vi "WVDIAL+HSRL_v5.8.vi"() -> ()   [LabVIEW 2012]
uses:
  C:/Users/eol-lidar/Desktop/20171016_WVDIALLabviewSlimmed/DLLs/PowerMeterCommands.dll
  DLLs/PowerMeterCommands.dll
  <vilib>/DAQmx/write.llb/DAQmx Write (Digital 1D Bool NChan 1Samp 1Line).vi
  <vilib>/DAQmx/miscellaneous.llb/DAQmx Fill In Error Info.vi
  <vilib>/Analysis/baseanly.llb/Mean (DBL).vi
  WVD-MCSupdate/WVDMCSupdate/Subroutines/AMCS_Data.vi
  Shared Telescope WV DIAL Code/Libraries and VIs/Scalar_Data.vi
  <vilib>/Analysis/NI_AALBase.lvlib
  Shared Telescope WV DIAL Code/Libraries and VIs/Scalar_Data_2.vi
  Shared Telescope WV DIAL Code/Libraries and VIs/Scalar_Data_4.vi
  Shared Telescope WV DIAL Code/Libraries and VIs/Scalar_Data_3.vi
  DLLs/CLDevIFace.dll
panel:
  out "WV_averaged_energy":dbl
  out "HSRL Pulse Energy":dbl=375.0
  out "sigma_off_total":dbl[](array[numeric])=[5.0680831413375535e-25, 5.050268932514758e-25, 5.0324923656148135e-25, 5.014753469706972e-25, 4.99705227357782e-25, 4.979388805746344e-25, 4.961763094386931e-25, 4.944175167376033e-25, 4.926625052240752e-25, 4.909112776197929e-25, 4.891638366076327e-25, 4.874201848358338e-25, 4.856803249148664e-25, 4.839442594150606e-25, 4.822119908686877e-25, 4.8048352176943855e-25, 4.78758854565523e-25, 4.770379916627166e-25, 4.753209354281222e-25, 4.736076881793376e-25, 4.718982521901608e-25, 4.7019262968902895e-25, 4.684908228544634e-25, 4.667928338234015e-25, 4.650986646753398e-25, 4.634083174466291e-25, 4.617217941209719e-25, 4.6003909663091255e-25, 4.583602268570049e-25, 4.566851866270442e-25, 4.55013977714655e-25, 4.533466018427296e-25, 4.516830606754478e-25, 4.500233558239396e-25, 4.483674888410031e-25, 4.467154612270298e-25, 4.450672744202499e-25, 4.434229298043165e-25, 4.417824287033527e-25, 4.401457723829736e-25, 4.385129620513669e-25, 4.368839988513398e-25, 4.352588838702857e-25, 4.336376181349563e-25, 4.320202026083546e-25, 4.304066381932244e-25, 4.287969257308179e-25, 4.271910659984005e-25, 4.255890597128637e-25, 4.239909075259594e-25, 4.22396610028079e-25, 4.208061677439288e-25, 4.192195811375286e-25, 4.176368506057362e-25, 4.160579764835863e-25, 4.144829590406775e-25, 4.129117984793732e-25, 4.113444949423985e-25, 4.097810485038377e-25, 4.082214591740086e-25, 4.0666572689665333e-25, 4.0511385155395965e-25, 4.0356583295814885e-25, 4.0202167085949603e-25, 4.004813649400491e-25, 3.989449148200182e-25, 3.974123200508076e-25, 3.958835801202973e-25, 3.943586944503348e-25, 3.928376623976787e-25, 3.9132048325413214e-25, 3.898071562459315e-25, 3.8829768053453936e-25, 3.8679205521584474e-25, 3.8529027932308287e-25, 3.837923518222313e-25, 3.822982716166859e-25, 3.8080803754419415e-25, 3.7932164837935613e-25, 3.7783910283248477e-25, 3.7636039955186373e-25, 3.748855371190181e-25, 3.7341451405484317e-25, 3.719473288177287e-25, 3.7048397980204027e-25, 3.6902446533968063e-25, 3.675687837026237e-25, 3.6611693309848415e-25, 3.6466891167654896e-25, 3.6322471752135777e-25, 3.617843486608717e-25, 3.6034780305936944e-25, 3.5891507862467635e-25, 3.5748617320063354e-25, 3.560610845767059e-25, 3.5463981047924663e-25, 3.532223485800512e-25, 3.5180869649136043e-25, 3.5039885176765912e-25, 3.48992811906682e-25, 3.475905743508301e-25, 3.4619213648441316e-25, 3.4479749563841165e-25, 3.434066490863645e-25, 3.4201959404908824e-25, 3.4063632769091302e-25, 3.3925684712700433e-25, 3.378811494142299e-25, 3.365092315592867e-25, 3.3514109051791915e-25, 3.3377672319122537e-25, 3.324161264322276e-25, 3.3105929704212585e-25, 3.2970623177234063e-25, 3.283569273235881e-25, 3.270113803501489e-25, 3.256695874559878e-25, 3.243315451986542e-25, 3.2299725008719377e-25, 3.2166669858496116e-25, 3.20339887109077e-25, 3.190168120304605e-25, 3.176974696765837e-25, 3.1638185632881056e-25, 3.150699682259159e-25, 3.1376180156208974e-25, 3.124573524912379e-25, 3.1115661712294625e-25, 3.098595915273405e-25, 3.0856627173057447e-25, 3.0727665372159963e-25, 3.0599073344858437e-25, 3.0470850681967553e-25, 3.0342996970621855e-25, 3.0215511793910874e-25, 3.0088394731451073e-25, 2.9961645359090424e-25, 2.9835263248846283e-25, 2.9709247969417565e-25, 2.958359908598783e-25, 2.9458316159962206e-25, 2.9333398749913824e-25, 2.9208846410508e-25, 2.9084658693549316e-25, 2.896083514735401e-25, 2.8837375317201307e-25, 2.8714278745019077e-25, 2.8591544970149368e-25, 2.846917352851204e-25, 2.8347163953255015e-25, 2.8225515774470685e-25, 2.810422851965737e-25, 2.798330171330179e-25, 2.786273487738203e-25, 2.77425275308972e-25, 2.7622679190446606e-25, 2.7503189370035713e-25, 2.738405758092023e-25, 2.7265283332265874e-25, 2.714686613054595e-25, 2.702880547978048e-25, 2.6911100881787775e-25, 2.679375183623213e-25, 2.667675784031e-25, 2.656011838920782e-25, 2.6443832975917595e-25, 2.632790109126673e-25, 2.621232222411873e-25, 2.609709586132485e-25, 2.5982221487819162e-25, 2.5867698586571715e-25, 2.5753526638740077e-25, 2.563970512352378e-25, 2.5526233518470714e-25, 2.54131112993464e-25, 2.530033794027293e-25, 2.5187912913630233e-25, 2.507583569015988e-25, 2.4964105739108755e-25, 2.485272252816323e-25, 2.474168552342947e-25, 2.4630994189670276e-25, 2.452064799004571e-25, 2.441064638654035e-25, 2.430098883964197e-25, 2.4191674808444842e-25, 2.408270375096492e-25, 2.3974075123655827e-25, 2.386578838207447e-25, 2.3757842980299015e-25, 2.365023837158599e-25, 2.3542974007604364e-25, 2.3436049339301653e-25, 2.332946381641563e-25, 2.322321688765572e-25, 2.3117308000577395e-25, 2.301173660203864e-25, 2.290650213761381e-25, 2.2801604052267496e-25, 2.2697041789820395e-25, 2.2592814793185174e-25, 2.2488922504726313e-25, 2.238536436557817e-25, 2.228213981633397e-25, 2.217924829675797e-25, 2.2076689245697116e-25, 2.197446210150236e-25, 2.187256630164115e-25, 2.1771001282917803e-25, 2.166976648140285e-25, 2.156886133275938e-25, 2.1468285271631183e-25, 2.1368037732345433e-25, 2.126811814852733e-25, 2.1168525953198595e-25, 2.106926057899171e-25, 2.0970321457635677e-25, 2.0871708020784106e-25, 2.0773419699265684e-25, 2.0675455923466506e-25, 2.0577816123512618e-25, 2.0480499728835437e-25, 2.0383506168412001e-25, 2.0286834871066825e-25, 2.0190485264964055e-25, 2.0094456777942608e-25, 1.9998748837535606e-25, 1.9903360870818826e-25, 1.9808292304539481e-25, 1.9713542565212467e-25, 1.9619111078898567e-25, 1.9524997271395504e-25, 1.9431200568252154e-25, 1.933772039471289e-25, 1.9244556175785046e-25, 1.9151707336173428e-25, 1.9059173300424462e-25, 1.896695349278346e-25, 1.887504733733578e-25, 1.87834542579272e-25, 1.8692173678369714e-25, 1.860120502207169e-25, 1.8510547712471297e-25, 1.842020117276254e-25, 1.8330164826123113e-25, 1.824043809547516e-25, 1.8151020403721158e-25, 1.8061911173670722e-25, 1.797310982803557e-25, 1.788461578952029e-25, 1.7796428480706259e-25, 1.77085473241696e-25, 1.7620971742526653e-25, 1.7533701158247174e-25, 1.7446734993880605e-25, 1.7360072672028068e-25, 1.7273713615348505e-25, 1.7187657246371322e-25, 1.7101902987927655e-25, 1.7016450262655736e-25, 1.693129849355724e-25, 1.6846447103521253e-25, 1.6761895515616383e-25, 1.6677643153115813e-25, 1.6593689439330508e-25, 1.651003379777635e-25, 1.6426675652102032e-25, 1.634361442624433e-25, 1.626084954418816e-25, 1.6178380430220918e-25, 1.6096206508892247e-25, 1.6014327204907626e-25, 1.5932741943263567e-25, 1.5851450149297006e-25, 1.5770451248486239e-25, 1.5689744666725117e-25, 1.5609329830216526e-25, 1.5529206165353868e-25, 1.544937309909236e-25, 1.5369830058589343e-25, 1.5290576471379584e-25, 1.5211611765445334e-25, 1.5132935369148861e-25, 1.505454671121801e-25, 1.4976445220855464e-25, 1.489863032772808e-25, 1.4821101461853077e-25, 1.4743858053839818e-25, 1.466689953463803e-25, 1.4590225335824177e-25, 1.4513834889370796e-25, 1.443772762787685e-25, 1.4361902984353226e-25, 1.4286360392430281e-25, 1.421109928625391e-25, 1.4136119100589185e-25, 1.406141927068145e-25, 1.3986999232379715e-25, 1.3912858422279377e-25, 1.383899627734513e-25, 1.376541223531611e-25, 1.3692105734515838e-25, 1.3619076213860454e-25, 1.3546323112982237e-25, 1.3473845872110886e-25, 1.3401643932080463e-25, 1.3329716734486295e-25, 1.3258063721594936e-25, 1.3186684336191663e-25, 1.311557802194871e-25, 1.3044744223048489e-25, 1.297418238447701e-25, 1.2903891951836824e-25, 1.2833872371460614e-25, 1.2764123090352544e-25, 1.2694643556285982e-25, 1.2625433217621673e-25, 1.2556491523516578e-25, 1.2487817923731893e-25, 1.2419411868814273e-25, 1.2351272809923693e-25, 1.2283400199027554e-25, 1.2215793488683331e-25, 1.214845213215785e-25, 1.208137558343977e-25, 1.201456329712131e-25, 1.194801472852171e-25, 1.1881729333666788e-25, 1.1815706569168798e-25, 1.1749945892296885e-25, 1.1684446760950514e-25, 1.1619208633760922e-25, 1.1554230969912116e-25, 1.1489513229158033e-25, 1.1425054871903887e-25, 1.1360855359210408e-25, 1.1296914152607023e-25, 1.1233230714222248e-25, 1.1169804506797123e-25, 1.110663499354571e-25, 1.1043721638205043e-25, 1.0981063905075512e-25, 1.0918661258885507e-25, 1.0856513164910038e-25, 1.0794619088778648e-25, 1.0732978496687776e-25, 1.0671590855166174e-25, 1.061045563121081e-25, 1.05495722921555e-25, 1.0488940305679622e-25, 1.042855913990988e-25, 1.0368428263208767e-25, 1.0308547144263727e-25, 1.0248915252079669e-25, 1.0189532055871608e-25, 1.0130397025147169e-25, 1.0071509629616662e-25, 1.001286933916925e-25, 9.954475623889804e-26, 9.896327954044623e-26, 9.838425799963646e-26, 9.780768632115727e-26, 9.723355921058893e-26, 9.666187137403877e-26, 9.609261751836239e-26, 9.552579234978825e-26, 9.496139057499041e-26, 9.439940690018152e-26, 9.383983603146422e-26, 9.328267267294007e-26, 9.272791152923559e-26, 9.217554730238317e-26, 9.162557469354778e-26, 9.107798840261185e-26, 9.053278312649423e-26, 8.998995356083224e-26, 8.9449494398041e-26, 8.891140032926042e-26, 8.837566604108784e-26, 8.784228621835966e-26, 8.731125554230762e-26, 8.678256869058159e-26, 8.625622033744771e-26, 8.573220515301755e-26, 8.521051780403056e-26, 8.469115295177399e-26, 8.417410525424378e-26, 8.365936936435877e-26, 8.31469399303781e-26, 8.263681159579713e-26, 8.212897899851394e-26, 8.162343677202723e-26, 8.112017954374161e-26, 8.061920193554679e-26, 8.012049856393303e-26, 7.962406403953712e-26, 7.912989296683604e-26, 7.863797994472096e-26, 7.814831956537151e-26, 7.766090641487171e-26, 7.717573507309588e-26, 7.669280011340041e-26, 7.621209610219873e-26, 7.573361759993122e-26, 7.525735915967917e-26, 7.478331532870406e-26, 7.431148064613669e-26, 7.384184964520994e-26, 7.337441685187794e-26, 7.29091767855353e-26, 7.244612395792056e-26, 7.198525287435714e-26, 7.152655803274832e-26, 7.107003392446656e-26, 7.061567503355338e-26, 7.016347583682272e-26, 6.971343080435626e-26, 6.926553439985115e-26, 6.88197810788442e-26, 6.837616529090031e-26, 6.79346814786059e-26, 6.749532407732893e-26, 6.705808751605971e-26, 6.662296621685533e-26, 6.618995459569764e-26, 6.575904706131978e-26, 6.533023801627712e-26, 6.490352185687561e-26, 6.447889297329119e-26, 6.405634574897022e-26, 6.363587456183544e-26, 6.321747378368162e-26, 6.280113778015749e-26, 6.238686091168659e-26, 6.197463753295892e-26, 6.156446199285288e-26, 6.115632863532144e-26, 6.075023179890269e-26, 6.034616581717167e-26, 5.994412501882668e-26, 5.954410372776347e-26, 5.914609626304142e-26, 5.875009693971481e-26, 5.835610006837895e-26, 5.796409995518303e-26, 5.75740909026125e-26, 5.718606720923057e-26, 5.680002316993107e-26, 5.641595307612728e-26, 5.603385121584446e-26, 5.565371187391746e-26, 5.527552933235658e-26, 5.489929786980034e-26, 5.452501176287165e-26, 5.415266528483136e-26, 5.378225270744512e-26, 5.341376829930272e-26, 5.304720632755439e-26, 5.268256105689871e-26, 5.231982675042429e-26, 5.195899766910684e-26, 5.16000680729164e-26, 5.1243032219653016e-26, 5.088788436603722e-26, 5.0534618767497824e-26, 5.018322967764659e-26, 4.983371134955952e-26, 4.948605803457036e-26, 4.914026398329114e-26, 4.879632344485452e-26, 4.8454230667505313e-26, 4.8113979898186e-26, 4.7775565382652193e-26, 4.7438981365517906e-26, 4.710422208969762e-26, 4.6771281796924836e-26, 4.644015472735411e-26, 4.611083511920767e-26, 4.57833172085292e-26, 4.545759522944633e-26, 4.5133663413310994e-26, 4.481151598877351e-26, 4.4491147181409444e-26, 4.4172551212861777e-26, 4.3855722300946404e-26, 4.354065465910907e-26, 4.322734249520448e-26, 4.291578001182216e-26, 4.260596140510642e-26, 4.229788086386439e-26, 4.199153256902903e-26, 4.168691069302124e-26, 4.1384009398048773e-26, 4.108282283613907e-26, 4.0783345146637817e-26, 4.048557045636684e-26, 4.0189492877570055e-26, 3.9895106506522613e-26, 3.9602405422291465e-26, 3.931138368487194e-26, 3.9022035333512423e-26, 3.873435438487378e-26, 3.8448334831007303e-26, 3.816397063734802e-26, 3.788125574018162e-26, 3.7600184044335007e-26, 3.732074942091133e-26, 3.7042945704012646e-26, 3.676676668819464e-26, 3.649220612529393e-26, 3.621925772117007e-26, 3.5947915132405926e-26, 3.5678171962714004e-26, 3.54100217587998e-26, 3.514345800680216e-26, 3.487847412793427e-26, 3.46150634740613e-26, 3.435321932324773e-26, 3.4092934874888365e-26, 3.383420324498672e-26, 3.3577017460758364e-26, 3.3321370455455056e-26, 3.306725506289838e-26, 3.2814664011948384e-26, 3.256358992044371e-26, 3.2314025289844984e-26, 3.2065962498566274e-26, 3.181939379657207e-26, 3.157431129885823e-26, 3.133070697945638e-26, 3.108857266564713e-26, 3.084790003140973e-26, 3.0608680592056025e-26, 3.0370905698406435e-26, 3.013456653126369e-26, 2.989965409648841e-26, 2.966615922014565e-26, 2.943407254448675e-26, 2.9203384524140105e-26, 2.897408542324931e-26, 2.874616531322669e-26, 2.8519614071813997e-26, 2.8294421382236213e-26, 2.8070576734672486e-26, 2.7848069428088064e-26, 2.7626888573875596e-26, 2.7407023100768283e-26, 2.7188461762097713e-26, 2.697119314370084e-26, 2.675520567481005e-26, 2.6540487640552044e-26, 2.632702719645332e-26, 2.611481238544639e-26, 2.590383115739343e-26, 2.5694071390316248e-26, 2.5485520914860395e-26, 2.5278167540887466e-26]
  out "sigma_on_total":dbl[](array[numeric])=[3.516762235495058e-23, 3.5170357724616793e-23, 3.517243654951452e-23, 3.5173857348664984e-23, 3.5174618696032314e-23, 3.5174719220915503e-23, 3.517415760753968e-23, 3.5172932596204093e-23, 3.517104298364396e-23, 3.51684876225809e-23, 3.5165265424458705e-23, 3.516137535496363e-23, 3.515681644076201e-23, 3.5151587762548456e-23, 3.514568846261864e-23, 3.5139117739475565e-23, 3.5131874852176734e-23, 3.512395911649246e-23, 3.511536990843376e-23, 3.5106106663674556e-23, 3.509616887861969e-23, 3.508555610727384e-23, 3.5074267963931806e-23, 3.506230412591386e-23, 3.504966432699066e-23, 3.5036348365157345e-23, 3.502235609771152e-23, 3.5007687440506677e-23, 3.499234237494354e-23, 3.4976320939504184e-23, 3.495962323760679e-23, 3.494224942903625e-23, 3.49241997404422e-23, 3.4905474456712165e-23, 3.488607392449504e-23, 3.486599855312831e-23, 3.4845248812021826e-23, 3.482382523331685e-23, 3.480172841011926e-23, 3.4778958997372714e-23, 3.475551771273733e-23, 3.473140533296108e-23, 3.470662269831449e-23, 3.468117070802047e-23, 3.465505032651236e-23, 3.4628262576097196e-23, 3.460080854138148e-23, 3.45726893673351e-23, 3.454390626099514e-23, 3.4514460488569266e-23, 3.4484353379891165e-23, 3.445358631993262e-23, 3.442216075973032e-23, 3.439007820599526e-23, 3.4357340227405154e-23, 3.432394845253444e-23, 3.4289904566802195e-23, 3.4255210316914945e-23, 3.4219867507798155e-23, 3.418387800421652e-23, 3.414724372765394e-23, 3.410996665790666e-23, 3.4072048831825184e-23, 3.4033492345861695e-23, 3.399429935096494e-23, 3.395447205798206e-23, 3.391401272962522e-23, 3.387292368778739e-23, 3.3831207310294633e-23, 3.3788866028578776e-23, 3.374590232920535e-23, 3.3702318753465245e-23, 3.3658117896955215e-23, 3.361330240816889e-23, 3.356787498902605e-23, 3.3521838393438606e-23, 3.3475195429790614e-23, 3.3427948954567696e-23, 3.338010187875212e-23, 3.333165716240765e-23, 3.328261781614206e-23, 3.3232986899599464e-23, 3.3182767522919066e-23, 3.3131962843222246e-23, 3.3080576067047674e-23, 3.302861044880871e-23, 3.2976069289233546e-23, 3.292295593378607e-23, 3.28692737770923e-23, 3.281502625634601e-23, 3.2760216853713696e-23, 3.270484909673951e-23, 3.2648926555724865e-23, 3.259245284310476e-23, 3.2535431613827763e-23, 3.247786656472462e-23, 3.2419761433868873e-23, 3.236111999891676e-23, 3.230194607644908e-23, 3.224224352334098e-23, 3.218201623304901e-23, 3.212126813900501e-23, 3.206000320987107e-23, 3.1998225450888635e-23, 3.193593890217053e-23, 3.187314763902574e-23, 3.180985577228577e-23, 3.1746067445558867e-23, 3.1681786832471166e-23, 3.161701814312117e-23, 3.1551765614147503e-23, 3.1486033518257166e-23, 3.141982615325147e-23, 3.135314784744979e-23, 3.128600295896494e-23, 3.12183958718897e-23, 3.1150330997616086e-23, 3.1081812775128245e-23, 3.1012845666149164e-23, 3.094343416057281e-23, 3.0873582768518243e-23, 3.080329602576102e-23, 3.073257848990092e-23, 3.0661434740644925e-23, 3.0589869378030693e-23, 3.0517887022709475e-23, 3.0445492314167926e-23, 3.037268991101071e-23, 3.0299484491244396e-23, 3.0225880747406617e-23, 3.015188339097293e-23, 3.007749714748848e-23, 3.000272675788408e-23, 2.9927576977732326e-23, 2.985205257650438e-23, 2.9776158335799395e-23, 2.96998990486058e-23, 2.9623279520622924e-23, 2.95463045674669e-23, 2.9468979013938806e-23, 2.9391307693296044e-23, 2.931329545063522e-23, 2.9234947134973156e-23, 2.9156267603665074e-23, 2.9077261721683166e-23, 2.899793435577354e-23, 2.8918290379901955e-23, 2.8838334673516254e-23, 2.875807211674682e-23, 2.867750759380563e-23, 2.859664598922285e-23, 2.8515492191245574e-23, 2.843405108706446e-23, 2.8352327564177137e-23, 2.827032650869429e-23, 2.818805280670558e-23, 2.810551134056049e-23, 2.8022706991261984e-23, 2.793964463577744e-23, 2.7856329147406625e-23, 2.7772765392102393e-23, 2.7688958234922345e-23, 2.7604912531299645e-23, 2.7520633132488165e-23, 2.743612487989655e-23, 2.735139261052668e-23, 2.7266441149317645e-23, 2.7181275314589267e-23, 2.709589991342852e-23, 2.701031974511761e-23, 2.6924539595546e-23, 2.683856424064811e-23, 2.6752398443838836e-23, 2.666604695645691e-23, 2.657951451622079e-23, 2.64928058466925e-23, 2.6405925660708546e-23, 2.6318878650933588e-23, 2.623166950023963e-23, 2.6144302873272845e-23, 2.605678341793869e-23, 2.596911576589419e-23, 2.5881304533037822e-23, 2.579335431608461e-23, 2.5705269695038145e-23, 2.561705522881775e-23, 2.5528715460663286e-23, 2.544025491086251e-23, 2.5351678083127844e-23, 2.526298945833359e-23, 2.5174193497978176e-23, 2.5085294640868702e-23, 2.499629730657495e-23, 2.4907205891173368e-23, 2.4818024768787626e-23, 2.4728758289295365e-23, 2.4639410781783132e-23, 2.4549986550355716e-23, 2.446048987569473e-23, 2.4370925014707235e-23, 2.4281296198294717e-23, 2.4191607635749923e-23, 2.410186350688018e-23, 2.4012067968306574e-23, 2.3922225152197037e-23, 2.383233916222184e-23, 2.3742414075155433e-23, 2.3652453944316237e-23, 2.356246279369929e-23, 2.3472444620513065e-23, 2.3382403394918925e-23, 2.3292343058859766e-23, 2.320226752582726e-23, 2.31121806824655e-23, 2.3022086386507255e-23, 2.2931988466565566e-23, 2.2841890722839565e-23, 2.2751796926910086e-23, 2.2661710820640453e-23, 2.25716361151011e-23, 2.2481576495791282e-23, 2.239153561347598e-23, 2.2301517092117286e-23, 2.221152452512235e-23, 2.2121561475204396e-23, 2.2031631476018805e-23, 2.1941738027609358e-23, 2.1851884603355635e-23, 2.1762074643670217e-23, 2.1672311557668873e-23, 2.1582598724815263e-23, 2.1492939493072072e-23, 2.1403337179684793e-23, 2.1313795069370378e-23, 2.122431641770026e-23, 2.1134904445861343e-23, 2.1045562347470948e-23, 2.0956293282506624e-23, 2.0867100378140534e-23, 2.0777986732100067e-23, 2.0688955410071003e-23, 2.060000944651547e-23, 2.0511151842133093e-23, 2.0422385568881732e-23, 2.0333713564102114e-23, 2.0245138737186396e-23, 2.0156663962089972e-23, 2.0068292082336044e-23, 1.998002591100643e-23, 1.9891868229105785e-23, 1.980382178477887e-23, 1.9715889294982612e-23, 1.9628073446320595e-23, 1.9540376892646818e-23, 1.9452802256735596e-23, 1.9365352129525438e-23, 1.9278029072567576e-23, 1.9190835612499812e-23, 1.91037742482846e-23, 1.9016847444917354e-23, 1.893005763903771e-23, 1.8843407232709448e-23, 1.875689860134706e-23, 1.8670534085198197e-23, 1.8584315997233446e-23, 1.8498246617024378e-23, 1.84123281962543e-23, 1.8326562953430182e-23, 1.8240953077839484e-23, 1.8155500729638188e-23, 1.8070208036927798e-23, 1.7985077098912548e-23, 1.7900109983755774e-23, 1.7815308732448307e-23, 1.773067535295308e-23, 1.764621182557202e-23, 1.756192010157153e-23, 1.7477802101116256e-23, 1.7393859717820795e-23, 1.731009481375805e-23, 1.72265092239957e-23, 1.7143104753107387e-23, 1.7059883179662526e-23, 1.6976846252044663e-23, 1.689399569006683e-23, 1.6811333187260572e-23, 1.672886040677187e-23, 1.6646578986487505e-23, 1.6564490535655085e-23, 1.6482596635768948e-23, 1.6400898840747094e-23, 1.6319398679177246e-23, 1.6238097651022214e-23, 1.615699723056421e-23, 1.6076098864519727e-23, 1.5995403974270677e-23, 1.5914913954000554e-23, 1.5834630172910538e-23, 1.5754553974044207e-23, 1.567468667381523e-23, 1.5595029564861017e-23, 1.5515583912900006e-23, 1.5436350960233774e-23, 1.5357331922636956e-23, 1.527852799218216e-23, 1.519994033676169e-23, 1.512157009770021e-23, 1.5043418395760004e-23, 1.4965486324245265e-23, 1.4887774955618395e-23, 1.4810285336580102e-23, 1.473301849145713e-23, 1.4655975421750792e-23, 1.4579157105704486e-23, 1.4502564497889548e-23, 1.4426198531888076e-23, 1.4350060117390143e-23, 1.4274150143477282e-23, 1.4198469475750628e-23, 1.412301895898126e-23, 1.4047799416085326e-23, 1.397281164833039e-23, 1.3898056436731065e-23, 1.3823534540450451e-23, 1.374924669819906e-23, 1.367519362784015e-23, 1.3601376026596058e-23, 1.3527794572993132e-23, 1.345444992356258e-23, 1.338134271653312e-23, 1.3308473570279063e-23, 1.3235843082957725e-23, 1.3163451834423065e-23, 1.3091300385276409e-23, 1.3019389277070232e-23, 1.2947719033067269e-23, 1.287629015842858e-23, 1.2805103139300586e-23, 1.2734158443578285e-23, 1.266345652328421e-23, 1.2592997810378082e-23, 1.2522782721323675e-23, 1.2452811654015202e-23, 1.2383084990135959e-23, 1.231360309373691e-23, 1.224436631302927e-23, 1.2175374978978468e-23, 1.2106629407078185e-23, 1.2038129895959912e-23, 1.1969876728632002e-23, 1.1901870172145144e-23, 1.1834110478803927e-23, 1.17665978842996e-23, 1.1699332610450954e-23, 1.1632314863343385e-23, 1.1565544833530395e-23, 1.1499022698715565e-23, 1.1432748620427733e-23, 1.1366722747191667e-23, 1.1300945212717786e-23, 1.123541613658381e-23, 1.1170135625863034e-23, 1.1105103771905268e-23, 1.1040320654863601e-23, 1.0975786340483784e-23, 1.0911500881251414e-23, 1.0847464317505074e-23, 1.0783676676651296e-23, 1.072013797333755e-23, 1.0656848209624235e-23, 1.0593807375613547e-23, 1.053101544960556e-23, 1.0468472397800419e-23, 1.0406178174014872e-23, 1.0344132721652046e-23, 1.0282335972046119e-23, 1.022078784463896e-23, 1.0159488248914287e-23, 1.009843708277041e-23, 1.0037634233561993e-23, 9.977079577813222e-24, 9.916772981374685e-24, 9.856714300432864e-24, 9.796903379941135e-24, 9.737340056329804e-24, 9.678024153832417e-24, 9.618955489701952e-24, 9.56013386888505e-24, 9.501559088775499e-24, 9.443230936842041e-24, 9.385149190786067e-24, 9.327313620315594e-24, 9.269723984839043e-24, 9.212380036839242e-24, 9.155281518378968e-24, 9.098428164050549e-24, 9.041819699508081e-24, 8.985455842395154e-24, 8.929336302854748e-24, 8.873460781329201e-24, 8.817828972565724e-24, 8.762440561873945e-24, 8.707295227569992e-24, 8.652392640705569e-24, 8.597732464436974e-24, 8.543314355275043e-24, 8.489137962449134e-24, 8.435202927298483e-24, 8.381508885599682e-24, 8.328055465472504e-24, 8.274842288958961e-24, 8.221868971047883e-24, 8.169135120158045e-24, 8.116640338958178e-24, 8.064384224108965e-24, 8.012366364973562e-24, 7.960586345836796e-24, 7.909043745295739e-24, 7.857738134993387e-24, 7.806669082471879e-24, 7.755836148193789e-24, 7.705238888368371e-24, 7.654876853018416e-24, 7.604749586765955e-24, 7.55485663024675e-24, 7.505197517235484e-24, 7.455771778360625e-24, 7.406578937601527e-24, 7.357618515634297e-24, 7.308890027653686e-24, 7.260392983805177e-24, 7.212126891168683e-24, 7.164091250688767e-24, 7.116285560408834e-24, 7.068709312748114e-24, 7.021361997071622e-24, 6.974243098223998e-24, 6.927352096928226e-24, 6.880688469872392e-24, 6.834251690388735e-24, 6.788041227928738e-24, 6.74205654756112e-24, 6.696297111818915e-24, 6.650762379008484e-24, 6.605451803883469e-24, 6.560364838293893e-24, 6.515500930679167e-24, 6.470859525864765e-24, 6.426440065985254e-24, 6.3822419899864224e-24, 6.338264733424697e-24, 6.2945077296430576e-24, 6.250970408187265e-24, 6.207652196791993e-24, 6.1645525192732555e-24, 6.1216707982928335e-24, 6.079006452468766e-24, 6.036558898585921e-24, 5.994327550854651e-24, 5.952311820977106e-24, 5.91051111846898e-24, 5.8689248504600775e-24, 5.827552422010919e-24, 5.786393235413015e-24, 5.745446691515252e-24, 5.70471218876791e-24, 5.6641891240289495e-24, 5.623876891385928e-24, 5.583774883936359e-24, 5.543882492367527e-24, 5.504199105985904e-24, 5.4647241118077035e-24, 5.425456895808213e-24, 5.3863968417823294e-24, 5.3475433323432925e-24, 5.3088957487283714e-24, 5.270453469928564e-24, 5.2322158743535506e-24, 5.194182338497658e-24, 5.156352237900821e-24, 5.118724946515789e-24, 5.081299837205395e-24, 5.044076281345124e-24, 5.00705364996358e-24, 4.970231311817872e-24, 4.933608635831867e-24, 4.8971849887587276e-24, 4.860959737161173e-24, 4.824932246587322e-24, 4.789101881198934e-24, 4.753468004653525e-24, 4.718029979926282e-24, 4.682787168937907e-24, 4.64773893320707e-24, 4.61288463287618e-24, 4.57822362796343e-24, 4.543755277985405e-24, 4.5094789415972385e-24, 4.475393976637923e-24, 4.441499740944134e-24, 4.4077955914103135e-24, 4.37428088498634e-24, 4.340954977751444e-24, 4.307817225523096e-24, 4.2748669836991026e-24, 4.242103607475026e-24, 4.2095264516881575e-24, 4.1771348710310574e-24, 4.1449282197180875e-24, 4.112905851880118e-24, 4.081067121412209e-24, 4.0494113821795354e-24, 4.0179379878670075e-24, 3.986646291836567e-24, 3.955535648018798e-24, 3.924605409556693e-24, 3.893854929871518e-24, 3.86328356267722e-24, 3.832890661331585e-24, 3.802675579205614e-24, 3.772637670199129e-24, 3.742776287938411e-24, 3.7130907862965146e-24, 3.683580519412032e-24, 3.654244841233783e-24, 3.625083106498119e-24, 3.596094669639684e-24, 3.567278885604821e-24, 3.538635109403695e-24, 3.510162696594244e-24, 3.481861002991539e-24, 3.4537293843915806e-24, 3.425767197493094e-24, 3.397973798720516e-24, 3.370348545724783e-24, 3.342890795635657e-24, 3.315599906549671e-24, 3.288475236958258e-24, 3.261516145767498e-24, 3.2347219923174537e-24, 3.2080921364011063e-24, 3.1816259384203983e-24, 3.155322759262521e-24, 3.1291819603180443e-24, 3.1032029037663484e-24, 3.0773849519178782e-24, 3.0517274680380555e-24, 3.0262298159556292e-24, 3.0008913599497758e-24, 2.9757114650285268e-24, 2.9506894969391785e-24, 2.925824821926189e-24, 2.9011168071272163e-24, 2.8765648200814337e-24, 2.852168229246826e-24, 2.82792640363848e-24, 2.803838713331491e-24]
  out "FileHour":i32=15
  out "L_Count":i32=3898
  out "background start":u32=534
  in  "Tab Control 2":enum32{"WV ND ", "Aerosol Backscatter"}(tab)=enum."Aerosol Backscatter"
  out "Absolute Humdity":dbl[][](graph)=[[-0.43911902357191485, 0.7674663952390105, 1.089198047561827, 2.6300411493201166, 3.4291765661964013, 2.1826370931198134, 1.507099326727282, 0.5927930846768686, -0.22988822366265907, 0.7025005460279994, 1.7544006141816164, 2.9545622050750473, 3.1900074073183284, 2.3324285712319845, 1.7514031153891634, 1.2541824635986243, 1.3509003729591222, 1.6519070588508906, 1.8026972975487114, 1.6903947914155135, 2.265494301508439, 2.146123298209767, 1.6391161390239504, 2.2166010853185822, 1.7640203753873043, 1.4599096312591482, 2.0214743075836146, 1.3455446471069752, 0.6906002473766166, 1.7187612553894822, 1.3245046931560058, 1.5373155298336214, 3.1175191270510267, 2.058600944624954, 1.992682744164231, 1.1161600614949756, -0.5551456593299476, 0.4070166162409883, 1.3515152707512752, 1.7177316023216946, 1.11631731679326, 1.111671097114888, 1.266626742515687, 1.46631192511657, 1.8073710736908608, 1.7019847089304116, 1.7250702973731098, 1.4125937608474792, 1.011178543723195, 1.3382268587214503, 1.3506200724082702, 1.9761660656741449, 2.1939556560739777, 1.5780195903776568, 2.045873256124458, 2.5293112999377176, 2.703490702778044, 1.6452879060216548, 1.0576075048490583, 1.0512130764071408, 0.7180371257359376, 2.211620844870098, 2.026119244247009, 0.4793695199345807, 0.9672725601626276, 0.6068382536487752, -0.512186851471919, -0.4011462028908473, 2.2986667235702, 2.3928225226358535, -0.8623343544274511, -4.546067296288631, -3.6671571300297594, 2.963508385146911, 2.477818336507603, -0.7730631068296039, 0.27484877099214655, 5.07228764603499, 2.7054981267383957, 7.484869038819736, 10.095384979146317, 8.159899319104877, 10.23621613915989, -0.15535901324366141, -0.7556744625625325, 2.0359146362496325, 3.2936174110066916, 0.26188560568521835, -1.5732608903042629, -2.7031331554811366, -6.26203848006013, -4.739911514124669, 7.8784445633844795, 4.34136334767541, -5.63169780872005, -5.188286488951439, -4.94422805003286, 1.8684667149638774, 8.76467512313612, 3.7715591123153467, 0.32819189377123303, -2.4505936350968844, -12.140776491859997, -6.038820259767352, 3.895123514841929, 9.862640663802816, 15.889993648854608, 14.678346101469582, -9.170494635908195, -8.428014213255375, 5.815078267516897, 10.848521904702222, -0.8857627679520638, 3.797778088570643, 11.036538008467865, -5.791907427244432, -8.201948155169413, -13.325468076271626, -7.10041117393044, -2.597492332767941, 11.13207815656458, -6.368634026394772, -10.006438999059894, -9.135296902391824, -13.617167814473344, -3.4845237505167916, -4.1454508598096504, 2.3435932133564874, 12.563732204982063, 11.288485674970199, 36.16868444595382, 14.799324316628024, 1.5769093431448964, -1.8854602956657383, 19.635491464201746, 16.80188672151142, 46.017922690101315, -3.3344957560978647, -1.7333040932192738, 16.563254978689933, -50.40049266193685, -1.478822874325444, 21.59077656916447, 16.283956730069626, 33.162981555324286, -18.016429544035276, -33.98559536088698, -6.453658300443035, -3.9250086558074146, -36.04460860293349, -11.207138038790982, -12.502937335249557, -18.70334107161657, 6.451952145173226, -39.77788600536842, -2.415211697000792, -12.042267091263861, 25.672126305642212, 27.582743378613074, 27.79818105218298, 18.14096003224789, 12.977436187270932, 8.300952165461291, -13.136037670393218, 12.4790266665156, 2.1400405652821046, -17.785069539595643, -45.96350671485605, -30.286726600015847, -6.691937135949138, -21.73091558346501, 3.876662572037105, -10.942380645889088, -20.11025690738919, 39.7950001868943, 13.302011241048865, 50.466041624007254, 86.92474022598945, 4.268838653895308, -15.510332019261929, -3.120771120488032, 82.70959529873473, 7.212016118863077, 33.79567740393959, -66.17164582139678, -14.266624478596933, -50.23105378528014, -89.36923945110037, -8.007399405059925, 20.873265942894925, 12.052826928469846, -123.2577053187001, -12.979203007957627, -37.916432497523004, -17.357255927214595, 2.424193931176986, 12.105455024944154, 9.39671603326679, -11.857119440235177, -36.45203460133756, -17.94219433082227, 25.151678741839277, 31.544730307661215, 27.524918592037537, 3.702470697348131, -11.067479447355169, -14.282810702638022, -6.623679239266069, 56.09246608240582, 36.66472983037535, 23.437555702735036, 27.67568468068117, -26.765705144177016, -7.161524719274879, 28.949544518736197, -8.993806007055584, 7.983236679121731, 31.466085561873314, -18.458534240183422, -73.61556182865067, -35.017148615525684, -23.833019550156873, -15.21702273040866, -7.142592181613441, -35.661949148037905, 60.69356326442661, 19.713397670224253, -17.883026013671092, -28.915412589844596, 56.08818489430987, 34.759673717673294, -1.7848152395586112, 30.039478435158447, 13.060054194604119, 24.45014848207904, -30.063842093382007, 3.00030230715792, 18.101208239831223, 14.799726748045284, 8.119813104816837, 8.792474244182555, -2.6819367152462514, -6.864471659793929, -8.464719896121629, -0.13458922431711476, 61.44658645984669, 9.567574008232688, -3.666034565863264, -5.046946350464024, -6.7482129347076265, -8.962278664595518, 11.267851385961015, 13.988036631351386, 8.653118740817341, 10.366790037010064, -61.808747733220905, -21.31075537221845, -8.2771015265964, -1.1438620239312303, 2.238097790183826, 3.8974548205482114, -3.4893073046384457, -8.821705986619776, -1.7859123029040789, -8.71772126672572, -3.0147944073719932, 2.3677584647460512, 3.650385333500165, 4.074997484857947, -0.40734405003237933, -6.067790871931436, -7.141221408743356, 14.609765340960015, 14.106004595440186, -31.931186108876847, -41.520029873391806, -19.794851211645675, -35.062557681914896, -42.40576415703153, -34.729201194765906, -40.105169588126046, 19.713817404511346, -49.31390778183477, 36.961376894599375, -38.62004628086643, -6.32287021310135, -4.3565484205215945, 24.534496672067952, 15.66396458255203, 97.66677999232155, 35.72375476017369, -73.65705456601637, 2.067566234273238, -76.29797616803506, 51.03788136001346, 18.90222470349584, -49.702263464726336, -162.57102303962967, 52.42583530551217, -95.06770127971939, -26.617125438135137, 21.60588778069863, 164.09841416001998, 24.224920521878957, 30.815023506316063, 34.87086766844997, 28.58143198840871, 146.67395537343643, -47.708963980019256, 21.9428530634823, 38.564811172828534, 49.41056852669724, -238.79484851802914, -66.052687314641, -96.10355014728687, -95.5871559144477, 40.83988650250965, 43.475983086813336, 0.3146611232194053, -57.92113263479661, -86.50607349880221, -46.66601322083931, 74.78750739157985, 33.58731971916481, 82.0189273383918, 66.17828900981743, 15.828750282461364, 128.98898461026386, 32.36477982878135, 41.292715954558744, 11.222439832481294, 20.882373165908316, -12.53860620252582, -11.025901192035857, -52.71470018331551, -37.75416667552049, 17.16686782465116, -148.0695548469285, -92.02220639264362, -9.621725955363358, 40.634897061935966, -54.19561553704295, 0.19256922982608626, 2.705738476726222, -67.92841173623351, 11.43063895755972, -101.05699470920753, -41.75593532364788, 77.82217107887442, -107.16183355638805, -6.644346212831696, 48.015602752530455, -2.826280188189698, 17.00937550041266, 45.378570522943164, -3.216248303794063, -47.535905897947366, -2.1416471893549414, -53.43411749158754, 100.056988279913, 4.5077035827966165, -3.4681683299170314, 78.94144920688721, -41.418068759228824, 63.41035478067363, 10.941650303541369, 72.09514961017665, 22.954807000569623, 37.58505741948733, 19.211356099163343, 8.36806288848049, -4.510582190291753, -84.203219500812, -127.20566074919812, -32.03321683489874, 71.13707478376679, -68.28675654099125, -5.070014078593644, 6.317676349883395, -76.13930765337595, -1.8097801311160377, -42.35186884877382, 136.40210547776994, 110.23560823152658, -78.14634172643382, -143.35537453766815, 90.5051179112309, 85.84572610130117, 0.6397803161787242, 26.074645575502156, -5.384544475919519, 90.41174545451459, -105.78459325272166, -99.77025958659856, 174.52912947182614, 216.81653820734786, -44.03123136198067, -110.06205393662276, -28.756543280269884, 74.44691147035503, -19.08819748364667, -57.62782727684459, -54.37021241945169, 141.53433389120698, -212.94365238427417, -127.8710282378702, 55.46889078541576, 60.18912046585632, 16.17632050754951, -124.17338839226964, -79.48214539666493, 2.264184105225891, 23.018973586716612, 59.67973610015452, 129.1402429611125, -2.5194785856018735, -20.116715560990293, -68.91417729611277, -127.14292619191158, 110.85548368430678, 118.84309886244603, -204.4337907222643, -220.97502702027364, -109.39265468176163, -99.83525030447593, 75.611129386354, 51.732838425089476, -16.26448504005327, 112.50382875161316, -65.30459777341832, -151.24297614131643, -106.8769085451633, 182.41586779612493, 14.682396841276315, 142.99334145918363, -61.413290273766606, 111.94019358125149, 154.59289487396987, -214.62582260199017, 54.89746663534102, 104.09764700780897, 153.46679671587947, 53.714970372805254, 114.30594447544635, -100.04777091083065, -83.78446042659188, 17.56692204963583, -233.31334718675464, 95.68415472865925, 13.813357318156969, 211.43682506862646, 331.10247078633154, 29.01033724066947, -66.1634157435356, 41.232661494877675, 22.766038523094117, 62.17321466458547, 167.67677281858678, -82.57240976208081, 31.87427363452741, -90.0984447176088, -185.8896799406589, -14.382218279554221, 22.947883635054612, 33.01337226979676, 185.61670504107, -278.10548234534053, 1.1761348198131083, 150.65272327367498, -156.21450261097485, -71.41734227420827, 193.7646422618191, 17.37553262297968, 5.478139913091408, 17.210869439202813, -72.81060297613503, 107.15506731119036, 51.13928453681435, 56.63733078666798, 147.76720023140442, 64.93260676843603, -273.7729915132311, 73.03962942057125, -10.352386123561907, 10.298394140344827, -146.47617580111626, -78.41364215229515, -310.5646190363324, -12.806151946359822, -239.14725235333947, -163.08909725538328, 40.796579558951386, -204.83372895132018, -200.7697824288599, -363.4414283726354, 98.61279360943745, 22.90101095800704, 377.0943507429146, 84.092404608979, 330.50906328556124, -31.316994886248807, 32.35325342771979, 255.03731059068778, 181.028718688296, 443.1982102564722, -23.76667509199042, 70.74003481964324, -134.11477765047925, -155.30804016381632, -233.72967769023967, -48.82622532292061, 159.41319054519667, -8.50455165762419, 7.252393694404157, -225.65864380952655, -65.80824706764862, -82.88698883069048, 125.39304515066029, -43.705535627238916, 311.43147238329783, 255.82741934799517, -124.18879604047645, -173.38468188675336, 96.52036098897344, -92.86986701240156, 171.2539866441557, -186.71904382508953, -276.6141098954611, 153.89123446188006, -166.57151009940048, 74.85347774357571, 338.7713134374434, -230.72249941522534, -230.30704775473677, 260.9121593060359, 379.3522477359284, 571.3157427938677, 660.755208257923, 168.97402576404386, 115.47244743761077, -346.3258112748618, -399.0683231386004, 601.2013788930942, 69.59615947630618, -13.239411448226178, -598.4806793666385, -7.939917205044425, -218.31030496983257, -152.1980061733255, -200.42173760532737, 101.05361795449112, -25.499221737363577, -407.7546192096181, -12.045156501862934, -118.44000763650338, 46.25216161070102, 0.0, 0.0, 0.0, 0.0]] caption="Water Vapor Number Density"
  out "Backscatter coef":dbl[][](graph)=[[-6.101781934239638, -5.55819207458303, -5.801044305154781, -6.2328196973688375, -6.123462348382745, -6.20454511151235, -6.230233735481989, -6.042460288349948, -6.183551699078807, -6.227583324579191, -6.14179490584266, -6.143598041595478, -6.243649871297107, -6.359221334791356, -6.397559978334611, -6.414721891492175, -6.583486632063202, -6.608356113735066, -6.479085289096807, -6.446078734050416, -6.408947595036615, -6.423946914503367, -6.529676985434499, -6.548874850127348, -6.53383478430665, -6.544013862553407, -6.470849612037488, -6.425986542998685, -6.490064242513089, -6.61442850716864, -6.6006100849411204, -6.564486600217162, -6.5912766529253695, -6.522963646056062, -6.433782002723005, -6.442100188316377, -6.357969926848167, -6.4294395107842925, -6.671873946585843, -6.5693667651223, -6.442154657110836, -6.627316417136742, -6.784281614219408, -6.82826455056865, -6.758622256468138, -6.572146777693813, -6.579011918997984, -6.726887737468162, -6.798353125161297, -6.632550076611347, -6.645257413804344, -6.409688215270268, -6.352622654680023, -6.469966713669638, -6.478787055077587, -6.609133823509786, -6.925203395437127, -6.912773007626432, -6.474892328385615, -6.3877190812993145, -6.30618894148784, -6.238046623511279, -6.369164948867766, -6.85060756875214, -6.877440858198632, -7.102948389995496, -7.879972331400623, -6.824995156110393, -6.601052025852254, -6.658935015227749, -6.581660399356896, -7.826827712774719, nan, -6.862363028311067, nan, -7.043271548959624, -6.554980851353428, -6.746756361648549, -6.471710007291128, -6.603143750008058, -6.969517781176899, -6.6533956488580746, -6.684513348055012, -6.855467344081217, -7.04806322155278, -7.058685532384198, -6.507047325108888, -6.697349668656321, -7.197998562647096, -6.14065622548063, nan, -6.657747296539549, nan, -6.872844777945468, -6.412116102542699, -6.4853258272712795, -5.701488005658509, -6.699194461112069, -6.799536069351966, -7.28248281187773, -6.721987992077037, nan, -5.8696467366998295, -6.191891614634519, -6.470695050609423, nan, -6.362405236333286, -7.383808298262869, -7.392369450178678, nan, nan, nan, -5.429004703299054, -7.141344338654054, -6.97010241908043, nan, nan, -7.847255547863111, nan, nan, nan, nan, nan, nan, -6.943106635634607, nan, -6.424595664976583, -7.763936251747335, -6.363978335247913, -6.437076520870096, -6.322176859254257, -6.463605971636375, nan, nan, -7.725945931706045, nan, nan, nan, nan, nan, nan, -7.029497900228135, nan, nan, nan, nan, -6.0770508341926055, -4.908384834473849, nan, -7.410668426290945, nan, -7.009087873143682, nan, nan, -6.452525855289771, -7.861147672479182, nan, nan, nan, nan, nan, -7.941553533165616, nan, nan, nan, nan, -6.688407630174046, nan, nan, nan, nan, nan, nan, -7.8954766416019835, nan, nan, nan, nan, nan, nan, nan, nan, nan, nan, -8.069425302907483, -7.337791663490015, -6.465528758424902, nan, -6.22762689299916, -6.903106438246555, nan, nan, nan, nan, nan, nan, nan, nan, nan, nan, nan, nan, nan, nan, nan, nan, nan, nan, nan, nan, nan, nan, nan, -6.757597584090068, nan, nan, nan, nan, nan, nan, nan, nan, nan, -5.28555309056839, nan, -7.938591488517235, nan, -7.201304983514285, nan, nan, -6.64156670249622, nan, nan, nan, nan, nan, nan, -5.311562799522255, -5.910909859318399, -5.908041686445022, -5.736617534218841, -6.150419939924439, -6.169203730474008, -5.556859074573575, -3.979132016620454, nan, -6.1914994657126154, -6.216072161385436, -5.849790050608194, nan, nan, -5.945987764217738, -6.183812829268557, -6.779842649130457, -6.971420158827712, -6.602903925356085, -5.456517847326549, -6.259957035764601, -6.0328808435207195, -6.196006111282781, nan, nan, -6.425628362757092, -5.754590483375731, nan, -5.577331674269346, nan, nan, -5.572791298424621, -6.241637765518725, -5.736282455012595, nan, -5.896948827281867, -6.7139486493262295, -6.705125028560182, -6.517084347716156, nan, nan, nan, -9.013260579632778, -5.717066396683533, nan, nan, nan, -7.762131335150803, nan, nan, nan, nan, nan, nan, nan, -6.545201890198715, -7.456125538818139, -6.65702933291991, -8.742000127950279, nan, -6.026770854720809, nan, nan, nan, nan, -6.567466491229605, nan, -7.031176856609699, nan, -8.005636414719262, nan, nan, nan, nan, nan, nan, nan, nan, -7.29486811785902, nan, nan, nan, nan, nan, nan, nan, nan, nan, nan, nan, nan, nan, -6.795427727652744, nan, nan, nan, nan, nan, nan, nan, -8.154571244295028, nan, nan, nan, -8.845266775441495, nan, nan, nan, nan, nan, nan, nan, nan, nan, nan, nan, nan, nan, -6.951811125727428, nan, nan, -7.393493398624159, nan, nan, nan, nan, nan, nan, nan, nan, nan, nan, nan, -7.223989215860527, nan, nan, nan, nan, nan, nan, nan, nan, nan, nan, nan, nan, nan, nan, -9.08674961116814, nan, nan, nan, nan, nan, nan, nan, nan, nan, nan, nan, nan, nan, -6.94748724512486, -6.786214691202737, nan, -7.638798822160836, nan, nan, nan, nan, nan, -7.736976289245345, nan, nan, nan, nan, nan, nan, nan, -7.324850728779775, nan, nan, nan, nan, nan, nan, nan, nan, nan, nan, nan, nan, nan, nan, nan, nan, nan, nan, nan, nan, nan, nan, nan, nan, nan, nan, nan, nan, -7.593816159626079, nan, nan, nan, nan, -9.114231695044417, nan, nan, nan, nan, -8.338836457430537, -7.736593899877906, nan, nan, nan, nan, nan, nan, nan, nan, nan, nan, nan, -7.263561345691878, nan, nan, nan, nan, nan, nan, -7.5785139208201135, nan, nan, nan, nan, nan, nan, nan, nan, nan, nan, -7.285866728754617, nan, nan, nan, nan, nan, -6.731074121270791, nan, nan, nan, -7.1857771374160375, -7.327150171084961, nan, nan, nan, -7.90494470790998, nan, nan, nan, nan, nan, -7.748141873196549, nan, -7.33723191679826, nan, nan, nan, nan, nan, -7.313697050657414, nan, -8.717279917923955, -8.509338006032813, nan, nan, nan, nan, -7.432594030618594, nan, -7.531314180693064, nan, nan, nan, nan, nan, nan, nan, nan, -7.6749074871488805, nan, nan, -6.850350129336467, nan, nan, nan, nan, nan, -6.625563065934155, nan, -7.915879745599926, nan, nan, nan, nan, nan, -8.976686657189024, -8.291181880961823, nan, nan, nan, -7.997335199255455, 0.0, 0.0, 0.0]] caption="Water Vapor Number Density"
  out "CH3 RingBuffer short":dbl[][](array[numeric])=[[58.56, 44.56, 19.560000000000002, 45.56, 45.56, 62.56, 77.56, 66.56, 77.56, 101.56, 167.56, 177.56, 186.56, 142.56, 149.56, 168.56, 157.56, 178.56, 202.56, 196.56, 231.56, 198.56, 199.56, 240.56, 195.56, 222.56, 197.56, 175.56, 169.56, 155.56, 163.56, 125.56, 152.56, 156.56, 149.56, 114.56, 117.56, 104.56, 111.56, 85.56, 115.56, 114.56, 81.56, 96.56, 91.56, 102.56, 90.56, 81.56, 95.56, 64.56, 82.56, 75.56, 62.56, 85.56, 67.56, 91.56, 73.56, 67.56, 66.56, 42.56, 35.56, 59.56, 61.56, 48.56, 50.56, 48.56, 32.56, 34.56, 51.56, 23.560000000000002, 38.56, 35.56, 28.560000000000002, 29.560000000000002, 14.560000000000002, 26.560000000000002, 17.560000000000002, 9.560000000000002, 20.560000000000002, 23.560000000000002, 10.560000000000002, 7.560000000000002, 35.56, 33.56, 12.560000000000002, 15.560000000000002, 19.560000000000002, 21.560000000000002, 27.560000000000002, 4.560000000000002, 20.560000000000002, 17.560000000000002, 19.560000000000002, 6.560000000000002, 5.560000000000002, 23.560000000000002, 5.560000000000002, 13.560000000000002, 17.560000000000002, 25.560000000000002, 15.560000000000002, 14.560000000000002, 25.560000000000002, 23.560000000000002, 16.560000000000002, 9.560000000000002, 14.560000000000002, 6.560000000000002, 11.560000000000002, -5.439999999999998, -1.4399999999999977, -4.439999999999998, 20.560000000000002, 11.560000000000002, 23.560000000000002, 14.560000000000002, 6.560000000000002, 20.560000000000002, 2.5600000000000023, 9.560000000000002, 0.5600000000000023, -4.439999999999998, 4.560000000000002, 14.560000000000002, 11.560000000000002, -9.439999999999998, -2.4399999999999977, 9.560000000000002, -5.439999999999998, 13.560000000000002, 7.560000000000002, 12.560000000000002, 19.560000000000002, -5.439999999999998, 17.560000000000002, 9.560000000000002, 10.560000000000002, 7.560000000000002, 8.560000000000002, -1.4399999999999977, -0.4399999999999977, 6.560000000000002, 20.560000000000002, 10.560000000000002, 28.560000000000002, 9.560000000000002, 9.560000000000002, -13.439999999999998, 0.5600000000000023, 4.560000000000002, 13.560000000000002, -8.439999999999998, 3.5600000000000023, -12.439999999999998, 21.560000000000002, 22.560000000000002, 0.5600000000000023, 24.560000000000002, -7.439999999999998, 11.560000000000002, -6.439999999999998, -3.4399999999999977, 2.5600000000000023, -0.4399999999999977, 9.560000000000002, -1.4399999999999977, 3.5600000000000023, 6.560000000000002, 3.5600000000000023, 1.5600000000000023, 4.560000000000002, 10.560000000000002, 6.560000000000002, 15.560000000000002, -2.4399999999999977, 10.560000000000002, -11.439999999999998, -8.439999999999998, -19.439999999999998, -11.439999999999998, -6.439999999999998, 9.560000000000002, -11.439999999999998, -2.4399999999999977, 15.560000000000002, 8.560000000000002, 9.560000000000002, -7.439999999999998, 5.560000000000002, 2.5600000000000023, -3.4399999999999977, 7.560000000000002, -12.439999999999998, -9.439999999999998, 0.5600000000000023, 7.560000000000002, 10.560000000000002, 7.560000000000002, 14.560000000000002, 11.560000000000002, 11.560000000000002, 9.560000000000002, 5.560000000000002, -1.4399999999999977, 15.560000000000002, 7.560000000000002, 5.560000000000002, -4.439999999999998, 3.5600000000000023, -1.4399999999999977, -5.439999999999998, -0.4399999999999977, 2.5600000000000023, -14.439999999999998, -4.439999999999998, -7.439999999999998, -0.4399999999999977, -0.4399999999999977, -12.439999999999998, -7.439999999999998, -1.4399999999999977, 3.5600000000000023, 1.5600000000000023, 7.560000000000002, -9.439999999999998, -6.439999999999998, -11.439999999999998, -9.439999999999998, 4.560000000000002, -6.439999999999998, 2.5600000000000023, -0.4399999999999977, 5.560000000000002, 8.560000000000002, -1.4399999999999977, 16.560000000000002, -9.439999999999998, 8.560000000000002, 24.560000000000002, 18.560000000000002, 57.56, 88.56, 110.56, 126.56, 101.56, 103.56, 74.56, 33.56, 28.560000000000002, 34.56, 26.560000000000002, -15.439999999999998, 33.56, 17.560000000000002, 14.560000000000002, 24.560000000000002, 31.560000000000002, 16.560000000000002, 20.560000000000002, 25.560000000000002, 17.560000000000002, 22.560000000000002, 42.56, 69.56, 45.56, 77.56, 101.56, 113.56, 111.56, 83.56, 86.56, 72.56, 49.56, 54.56, 2.5600000000000023, 27.560000000000002, -2.4399999999999977, -14.439999999999998, 4.560000000000002, -9.439999999999998, -3.4399999999999977, 9.560000000000002, -7.439999999999998, -12.439999999999998, -9.439999999999998, -3.4399999999999977, 15.560000000000002, 8.560000000000002, 15.560000000000002, 8.560000000000002, -6.439999999999998, 1.5600000000000023, 13.560000000000002, 17.560000000000002, -1.4399999999999977, -5.439999999999998, -1.4399999999999977, 4.560000000000002, -1.4399999999999977, -5.439999999999998, 11.560000000000002, 22.560000000000002, -2.4399999999999977, -1.4399999999999977, -19.439999999999998, -27.439999999999998, -3.4399999999999977, 1.5600000000000023, 0.5600000000000023, -2.4399999999999977, -14.439999999999998, 1.5600000000000023, 4.560000000000002, 13.560000000000002, 2.5600000000000023, -1.4399999999999977, 8.560000000000002, 8.560000000000002, 23.560000000000002, -6.439999999999998, -13.439999999999998, -13.439999999999998, -19.439999999999998, -5.439999999999998, 1.5600000000000023, -9.439999999999998, 0.5600000000000023, -14.439999999999998, 11.560000000000002, -0.4399999999999977, -3.4399999999999977, 9.560000000000002, 5.560000000000002, 5.560000000000002, -12.439999999999998, -13.439999999999998, 10.560000000000002, -13.439999999999998, -4.439999999999998, 1.5600000000000023, -3.4399999999999977, 5.560000000000002, -6.439999999999998, -9.439999999999998, -3.4399999999999977, 7.560000000000002, -10.439999999999998, 17.560000000000002, 4.560000000000002, 8.560000000000002, 0.5600000000000023, -9.439999999999998, 4.560000000000002, -18.439999999999998, 9.560000000000002, 0.5600000000000023, -1.4399999999999977, -1.4399999999999977, 1.5600000000000023, -7.439999999999998, -0.4399999999999977, 1.5600000000000023, 4.560000000000002, -8.439999999999998, 8.560000000000002, -9.439999999999998, -5.439999999999998, -6.439999999999998, -4.439999999999998, -20.439999999999998, -2.4399999999999977, -0.4399999999999977, 1.5600000000000023, -19.439999999999998, -1.4399999999999977, 8.560000000000002, -2.4399999999999977, -7.439999999999998, -2.4399999999999977, -3.4399999999999977, 8.560000000000002, -4.439999999999998, -2.4399999999999977, 7.560000000000002, -5.439999999999998, 1.5600000000000023, -5.439999999999998, -1.4399999999999977, -4.439999999999998, -6.439999999999998, -0.4399999999999977, -2.4399999999999977, 4.560000000000002, -12.439999999999998, -11.439999999999998, 12.560000000000002, -7.439999999999998, 7.560000000000002, -1.4399999999999977, 3.5600000000000023, 25.560000000000002, -15.439999999999998, 1.5600000000000023, -6.439999999999998, -5.439999999999998, -9.439999999999998, -5.439999999999998, 0.5600000000000023, -11.439999999999998, -9.439999999999998, 0.5600000000000023, -17.439999999999998, -7.439999999999998, 4.560000000000002, -5.439999999999998, -2.4399999999999977, -5.439999999999998, 4.560000000000002, -8.439999999999998, 1.5600000000000023, -17.439999999999998, 0.5600000000000023, 4.560000000000002, -2.4399999999999977, -17.439999999999998, 4.560000000000002, -4.439999999999998, -5.439999999999998, 2.5600000000000023, 18.560000000000002, 20.560000000000002, 5.560000000000002, -14.439999999999998, -1.4399999999999977, 3.5600000000000023, -0.4399999999999977, -7.439999999999998, 3.5600000000000023, 2.5600000000000023, 1.5600000000000023, -20.439999999999998, -7.439999999999998, -3.4399999999999977, 1.5600000000000023, 11.560000000000002, -12.439999999999998, -3.4399999999999977, 9.560000000000002, -5.439999999999998, -17.439999999999998, 7.560000000000002, -2.4399999999999977, 2.5600000000000023, -7.439999999999998, -8.439999999999998, 6.560000000000002, 12.560000000000002, 0.5600000000000023, -16.439999999999998, -10.439999999999998, -0.4399999999999977, -9.439999999999998, -10.439999999999998, 2.5600000000000023, 2.5600000000000023, -9.439999999999998, -12.439999999999998, -10.439999999999998, 22.560000000000002, 5.560000000000002, 3.5600000000000023, -17.439999999999998, -5.439999999999998, 1.5600000000000023, -16.439999999999998, -10.439999999999998, -4.439999999999998, -6.439999999999998, -10.439999999999998, -3.4399999999999977, -6.439999999999998, -13.439999999999998, -4.439999999999998, -1.4399999999999977, -20.439999999999998, -7.439999999999998, -6.439999999999998, -6.439999999999998, 0.5600000000000023, 4.560000000000002, 3.5600000000000023, -2.4399999999999977, -4.439999999999998, 12.560000000000002, -20.439999999999998, -2.4399999999999977, 0.5600000000000023, -20.439999999999998, 5.560000000000002, -8.439999999999998, -4.439999999999998, 10.560000000000002, -2.4399999999999977, -16.439999999999998, 5.560000000000002, 9.560000000000002, 0.5600000000000023, -5.439999999999998, -18.439999999999998, -8.439999999999998, -5.439999999999998, -4.439999999999998, -4.439999999999998, 7.560000000000002, -13.439999999999998, -5.439999999999998, 5.560000000000002, -1.4399999999999977, -3.4399999999999977, -11.439999999999998, -0.4399999999999977, -9.439999999999998, -13.439999999999998, -1.4399999999999977, -15.439999999999998, 3.5600000000000023, 4.560000000000002, 3.5600000000000023, -1.4399999999999977, 19.560000000000002, -17.439999999999998, -2.4399999999999977, -11.439999999999998, 0.5600000000000023, -12.439999999999998, -7.439999999999998, -13.439999999999998, 5.560000000000002, 0.5600000000000023, -3.4399999999999977, -4.439999999999998, 4.560000000000002, 10.560000000000002, -26.439999999999998, 18.560000000000002, 8.560000000000002, -0.4399999999999977, -3.4399999999999977, -10.439999999999998, -5.439999999999998, -2.4399999999999977, 13.560000000000002, 0.5600000000000023, 2.5600000000000023, 9.560000000000002, 7.560000000000002, -11.439999999999998, 2.5600000000000023, 16.560000000000002], [121.76, 61.760000000000005, 55.760000000000005, 58.760000000000005, 27.760000000000005, 56.760000000000005, 69.76, 80.76, 95.76, 109.76, 129.76, 166.76, 167.76, 186.76, 206.76, 188.76, 167.76, 189.76, 204.76, 215.76, 243.76, 213.76, 221.76, 203.76, 180.76, 187.76, 183.76, 188.76, 160.76, 189.76, 168.76, 155.76, 147.76, 128.76, 143.76, 142.76, 149.76, 140.76, 110.76, 130.76, 126.76, 100.76, 108.76, 101.76, 117.76, 99.76, 113.76, 77.76, 67.76, 94.76, 98.76, 72.76, 58.760000000000005, 58.760000000000005, 89.76, 68.76, 43.760000000000005, 68.76, 58.760000000000005, 57.760000000000005, 64.76, 38.760000000000005, 62.760000000000005, 36.760000000000005, 47.760000000000005, 50.760000000000005, 39.760000000000005, 45.760000000000005, 59.760000000000005, 52.760000000000005, 47.760000000000005, 26.760000000000005, 17.760000000000005, 5.760000000000005, 30.760000000000005, 29.760000000000005, 45.760000000000005, 27.760000000000005, 31.760000000000005, 25.760000000000005, 23.760000000000005, 21.760000000000005, 28.760000000000005, 9.760000000000005, 10.760000000000005, 14.760000000000005, 27.760000000000005, 18.760000000000005, 9.760000000000005, 26.760000000000005, 27.760000000000005, 13.760000000000005, 23.760000000000005, 18.760000000000005, 18.760000000000005, 27.760000000000005, 15.760000000000005, 31.760000000000005, 30.760000000000005, 17.760000000000005, 24.760000000000005, 13.760000000000005, 2.760000000000005, 23.760000000000005, 31.760000000000005, 6.760000000000005, 23.760000000000005, 4.760000000000005, 15.760000000000005, 9.760000000000005, -6.239999999999995, 8.760000000000005, 22.760000000000005, 7.760000000000005, 23.760000000000005, 13.760000000000005, 3.760000000000005, 4.760000000000005, 1.7600000000000051, 16.760000000000005, 5.760000000000005, 1.7600000000000051, 12.760000000000005, -2.239999999999995, -0.23999999999999488, 10.760000000000005, 16.760000000000005, 12.760000000000005, 14.760000000000005, 10.760000000000005, 15.760000000000005, 19.760000000000005, 2.760000000000005, -2.239999999999995, 14.760000000000005, 10.760000000000005, 4.760000000000005, 23.760000000000005, 17.760000000000005, -2.239999999999995, 7.760000000000005, 13.760000000000005, -1.2399999999999949, 17.760000000000005, 8.760000000000005, 10.760000000000005, 7.760000000000005, 5.760000000000005, 22.760000000000005, 24.760000000000005, -0.23999999999999488, 4.760000000000005, 6.760000000000005, -1.2399999999999949, 20.760000000000005, -3.239999999999995, 10.760000000000005, 6.760000000000005, 12.760000000000005, 9.760000000000005, 5.760000000000005, 4.760000000000005, 10.760000000000005, -6.239999999999995, 2.760000000000005, 7.760000000000005, 9.760000000000005, -8.239999999999995, -6.239999999999995, 30.760000000000005, 3.760000000000005, -5.239999999999995, 7.760000000000005, 0.7600000000000051, 13.760000000000005, 16.760000000000005, 13.760000000000005, -4.239999999999995, -8.239999999999995, 2.760000000000005, -2.239999999999995, -1.2399999999999949, 12.760000000000005, -4.239999999999995, 1.7600000000000051, 4.760000000000005, 23.760000000000005, 0.7600000000000051, 7.760000000000005, 16.760000000000005, 0.7600000000000051, -11.239999999999995, -6.239999999999995, 13.760000000000005, -8.239999999999995, -14.239999999999995, -1.2399999999999949, 13.760000000000005, 14.760000000000005, -2.239999999999995, 2.760000000000005, -6.239999999999995, 0.7600000000000051, -5.239999999999995, -1.2399999999999949, 4.760000000000005, -2.239999999999995, 1.7600000000000051, 9.760000000000005, 0.7600000000000051, 5.760000000000005, -5.239999999999995, -2.239999999999995, -5.239999999999995, 19.760000000000005, -6.239999999999995, -0.23999999999999488, -17.239999999999995, -2.239999999999995, 15.760000000000005, 0.7600000000000051, -6.239999999999995, -1.2399999999999949, 17.760000000000005, -1.2399999999999949, -2.239999999999995, 2.760000000000005, -1.2399999999999949, 23.760000000000005, 17.760000000000005, 14.760000000000005, -0.23999999999999488, 10.760000000000005, 12.760000000000005, -1.2399999999999949, 2.760000000000005, -12.239999999999995, 9.760000000000005, 21.760000000000005, 9.760000000000005, 60.760000000000005, 80.76, 116.76, 135.76, 123.76, 87.76, 61.760000000000005, 38.760000000000005, 16.760000000000005, 34.760000000000005, 24.760000000000005, 28.760000000000005, 12.760000000000005, 31.760000000000005, 15.760000000000005, 34.760000000000005, 20.760000000000005, 27.760000000000005, 29.760000000000005, 33.760000000000005, 12.760000000000005, 29.760000000000005, 41.760000000000005, 44.760000000000005, 63.760000000000005, 66.76, 92.76, 114.76, 103.76, 108.76, 65.76, 54.760000000000005, 74.76, 49.760000000000005, 41.760000000000005, 25.760000000000005, 0.7600000000000051, 9.760000000000005, 5.760000000000005, -1.2399999999999949, 9.760000000000005, 12.760000000000005, -9.239999999999995, -6.239999999999995, -7.239999999999995, 4.760000000000005, -4.239999999999995, 8.760000000000005, -3.239999999999995, 1.7600000000000051, 10.760000000000005, 5.760000000000005, 3.760000000000005, 7.760000000000005, 6.760000000000005, -2.239999999999995, -4.239999999999995, -10.239999999999995, 7.760000000000005, 12.760000000000005, 11.760000000000005, -2.239999999999995, 16.760000000000005, -4.239999999999995, 2.760000000000005, 3.760000000000005, 19.760000000000005, 9.760000000000005, -5.239999999999995, -16.239999999999995, -12.239999999999995, 25.760000000000005, -0.23999999999999488, 3.760000000000005, -1.2399999999999949, 17.760000000000005, 4.760000000000005, -13.239999999999995, 2.760000000000005, 4.760000000000005, 1.7600000000000051, -16.239999999999995, -1.2399999999999949, 6.760000000000005, 11.760000000000005, 5.760000000000005, 6.760000000000005, 2.760000000000005, -2.239999999999995, 14.760000000000005, 26.760000000000005, -6.239999999999995, -13.239999999999995, 3.760000000000005, -7.239999999999995, 7.760000000000005, -9.239999999999995, 15.760000000000005, -13.239999999999995, 6.760000000000005, 3.760000000000005, 6.760000000000005, -1.2399999999999949, 14.760000000000005, 12.760000000000005, -12.239999999999995, 2.760000000000005, -4.239999999999995, 3.760000000000005, 3.760000000000005, -7.239999999999995, 6.760000000000005, 0.7600000000000051, 0.7600000000000051, -3.239999999999995, -2.239999999999995, 3.760000000000005, -3.239999999999995, -16.239999999999995, 17.760000000000005, 12.760000000000005, 8.760000000000005, -3.239999999999995, 3.760000000000005, -6.239999999999995, 5.760000000000005, 8.760000000000005, 10.760000000000005, -5.239999999999995, -1.2399999999999949, 18.760000000000005, 6.760000000000005, -1.2399999999999949, 9.760000000000005, -7.239999999999995, -15.239999999999995, -6.239999999999995, -1.2399999999999949, 5.760000000000005, -8.239999999999995, -5.239999999999995, -0.23999999999999488, 9.760000000000005, -19.239999999999995, 0.7600000000000051, -15.239999999999995, -3.239999999999995, 12.760000000000005, 10.760000000000005, -11.239999999999995, -10.239999999999995, 2.760000000000005, 10.760000000000005, -21.239999999999995, 7.760000000000005, -16.239999999999995, -15.239999999999995, 7.760000000000005, -6.239999999999995, 4.760000000000005, 8.760000000000005, 3.760000000000005, -2.239999999999995, 15.760000000000005, 8.760000000000005, 14.760000000000005, 14.760000000000005, 9.760000000000005, -5.239999999999995, 9.760000000000005, 16.760000000000005, 1.7600000000000051, -6.239999999999995, -9.239999999999995, -9.239999999999995, 10.760000000000005, -4.239999999999995, -4.239999999999995, 9.760000000000005, -0.23999999999999488, -0.23999999999999488, -11.239999999999995, -0.23999999999999488, -3.239999999999995, 21.760000000000005, 8.760000000000005, 0.7600000000000051, 12.760000000000005, -8.239999999999995, 6.760000000000005, -5.239999999999995, 11.760000000000005, -2.239999999999995, -0.23999999999999488, -6.239999999999995, -0.23999999999999488, 13.760000000000005, -2.239999999999995, 4.760000000000005, 2.760000000000005, 18.760000000000005, -2.239999999999995, 11.760000000000005, -9.239999999999995, -7.239999999999995, 15.760000000000005, 12.760000000000005, -5.239999999999995, -11.239999999999995, -1.2399999999999949, 6.760000000000005, 7.760000000000005, -0.23999999999999488, 0.7600000000000051, -4.239999999999995, 16.760000000000005, 2.760000000000005, 3.760000000000005, 7.760000000000005, 16.760000000000005, -3.239999999999995, 22.760000000000005, -12.239999999999995, 8.760000000000005, -17.239999999999995, -10.239999999999995, -1.2399999999999949, 6.760000000000005, 12.760000000000005, 10.760000000000005, 2.760000000000005, 3.760000000000005, 6.760000000000005, -2.239999999999995, 4.760000000000005, -1.2399999999999949, 11.760000000000005, -6.239999999999995, 0.7600000000000051, -12.239999999999995, -14.239999999999995, -3.239999999999995, 7.760000000000005, 0.7600000000000051, -9.239999999999995, 10.760000000000005, 12.760000000000005, 14.760000000000005, 7.760000000000005, -0.23999999999999488, -10.239999999999995, -9.239999999999995, 11.760000000000005, 5.760000000000005, 13.760000000000005, 16.760000000000005, -1.2399999999999949, 11.760000000000005, 8.760000000000005, -10.239999999999995, -0.23999999999999488, 5.760000000000005, 15.760000000000005, -0.23999999999999488, 1.7600000000000051, -14.239999999999995, -9.239999999999995, 19.760000000000005, 5.760000000000005, 0.7600000000000051, 6.760000000000005, 12.760000000000005, 1.7600000000000051, -1.2399999999999949, -2.239999999999995, 2.760000000000005, -8.239999999999995, -1.2399999999999949, -4.239999999999995, 14.760000000000005, -3.239999999999995, 2.760000000000005, -10.239999999999995, -0.23999999999999488, -13.239999999999995, 21.760000000000005, -8.239999999999995, -11.239999999999995, 10.760000000000005, 9.760000000000005, 0.7600000000000051, 12.760000000000005, 20.760000000000005, -3.239999999999995, 0.7600000000000051, -9.239999999999995, -13.239999999999995, 8.760000000000005, 4.760000000000005, 8.760000000000005, 0.7600000000000051, 7.760000000000005, -7.239999999999995, -6.239999999999995, -14.239999999999995, -7.239999999999995, 12.760000000000005, 7.760000000000005, 9.760000000000005, -18.239999999999995, -2.239999999999995, -1.2399999999999949, 14.760000000000005, 7.760000000000005, -7.239999999999995, -3.239999999999995, 3.760000000000005, -0.23999999999999488, 1.7600000000000051], [121.76, 61.760000000000005, 55.760000000000005, 58.760000000000005, 27.760000000000005, 56.760000000000005, 69.76, 80.76, 95.76, 109.76, 129.76, 166.76, 167.76, 186.76, 206.76, 188.76, 167.76, 189.76, 204.76, 215.76, 243.76, 213.76, 221.76, 203.76, 180.76, 187.76, 183.76, 188.76, 160.76, 189.76, 168.76, 155.76, 147.76, 128.76, 143.76, 142.76, 149.76, 140.76, 110.76, 130.76, 126.76, 100.76, 108.76, 101.76, 117.76, 99.76, 113.76, 77.76, 67.76, 94.76, 98.76, 72.76, 58.760000000000005, 58.760000000000005, 89.76, 68.76, 43.760000000000005, 68.76, 58.760000000000005, 57.760000000000005, 64.76, 38.760000000000005, 62.760000000000005, 36.760000000000005, 47.760000000000005, 50.760000000000005, 39.760000000000005, 45.760000000000005, 59.760000000000005, 52.760000000000005, 47.760000000000005, 26.760000000000005, 17.760000000000005, 5.760000000000005, 30.760000000000005, 29.760000000000005, 45.760000000000005, 27.760000000000005, 31.760000000000005, 25.760000000000005, 23.760000000000005, 21.760000000000005, 28.760000000000005, 9.760000000000005, 10.760000000000005, 14.760000000000005, 27.760000000000005, 18.760000000000005, 9.760000000000005, 26.760000000000005, 27.760000000000005, 13.760000000000005, 23.760000000000005, 18.760000000000005, 18.760000000000005, 27.760000000000005, 15.760000000000005, 31.760000000000005, 30.760000000000005, 17.760000000000005, 24.760000000000005, 13.760000000000005, 2.760000000000005, 23.760000000000005, 31.760000000000005, 6.760000000000005, 23.760000000000005, 4.760000000000005, 15.760000000000005, 9.760000000000005, -6.239999999999995, 8.760000000000005, 22.760000000000005, 7.760000000000005, 23.760000000000005, 13.760000000000005, 3.760000000000005, 4.760000000000005, 1.7600000000000051, 16.760000000000005, 5.760000000000005, 1.7600000000000051, 12.760000000000005, -2.239999999999995, -0.23999999999999488, 10.760000000000005, 16.760000000000005, 12.760000000000005, 14.760000000000005, 10.760000000000005, 15.760000000000005, 19.760000000000005, 2.760000000000005, -2.239999999999995, 14.760000000000005, 10.760000000000005, 4.760000000000005, 23.760000000000005, 17.760000000000005, -2.239999999999995, 7.760000000000005, 13.760000000000005, -1.2399999999999949, 17.760000000000005, 8.760000000000005, 10.760000000000005, 7.760000000000005, 5.760000000000005, 22.760000000000005, 24.760000000000005, -0.23999999999999488, 4.760000000000005, 6.760000000000005, -1.2399999999999949, 20.760000000000005, -3.239999999999995, 10.760000000000005, 6.760000000000005, 12.760000000000005, 9.760000000000005, 5.760000000000005, 4.760000000000005, 10.760000000000005, -6.239999999999995, 2.760000000000005, 7.760000000000005, 9.760000000000005, -8.239999999999995, -6.239999999999995, 30.760000000000005, 3.760000000000005, -5.239999999999995, 7.760000000000005, 0.7600000000000051, 13.760000000000005, 16.760000000000005, 13.760000000000005, -4.239999999999995, -8.239999999999995, 2.760000000000005, -2.239999999999995, -1.2399999999999949, 12.760000000000005, -4.239999999999995, 1.7600000000000051, 4.760000000000005, 23.760000000000005, 0.7600000000000051, 7.760000000000005, 16.760000000000005, 0.7600000000000051, -11.239999999999995, -6.239999999999995, 13.760000000000005, -8.239999999999995, -14.239999999999995, -1.2399999999999949, 13.760000000000005, 14.760000000000005, -2.239999999999995, 2.760000000000005, -6.239999999999995, 0.7600000000000051, -5.239999999999995, -1.2399999999999949, 4.760000000000005, -2.239999999999995, 1.7600000000000051, 9.760000000000005, 0.7600000000000051, 5.760000000000005, -5.239999999999995, -2.239999999999995, -5.239999999999995, 19.760000000000005, -6.239999999999995, -0.23999999999999488, -17.239999999999995, -2.239999999999995, 15.760000000000005, 0.7600000000000051, -6.239999999999995, -1.2399999999999949, 17.760000000000005, -1.2399999999999949, -2.239999999999995, 2.760000000000005, -1.2399999999999949, 23.760000000000005, 17.760000000000005, 14.760000000000005, -0.23999999999999488, 10.760000000000005, 12.760000000000005, -1.2399999999999949, 2.760000000000005, -12.239999999999995, 9.760000000000005, 21.760000000000005, 9.760000000000005, 60.760000000000005, 80.76, 116.76, 135.76, 123.76, 87.76, 61.760000000000005, 38.760000000000005, 16.760000000000005, 34.760000000000005, 24.760000000000005, 28.760000000000005, 12.760000000000005, 31.760000000000005, 15.760000000000005, 34.760000000000005, 20.760000000000005, 27.760000000000005, 29.760000000000005, 33.760000000000005, 12.760000000000005, 29.760000000000005, 41.760000000000005, 44.760000000000005, 63.760000000000005, 66.76, 92.76, 114.76, 103.76, 108.76, 65.76, 54.760000000000005, 74.76, 49.760000000000005, 41.760000000000005, 25.760000000000005, 0.7600000000000051, 9.760000000000005, 5.760000000000005, -1.2399999999999949, 9.760000000000005, 12.760000000000005, -9.239999999999995, -6.239999999999995, -7.239999999999995, 4.760000000000005, -4.239999999999995, 8.760000000000005, -3.239999999999995, 1.7600000000000051, 10.760000000000005, 5.760000000000005, 3.760000000000005, 7.760000000000005, 6.760000000000005, -2.239999999999995, -4.239999999999995, -10.239999999999995, 7.760000000000005, 12.760000000000005, 11.760000000000005, -2.239999999999995, 16.760000000000005, -4.239999999999995, 2.760000000000005, 3.760000000000005, 19.760000000000005, 9.760000000000005, -5.239999999999995, -16.239999999999995, -12.239999999999995, 25.760000000000005, -0.23999999999999488, 3.760000000000005, -1.2399999999999949, 17.760000000000005, 4.760000000000005, -13.239999999999995, 2.760000000000005, 4.760000000000005, 1.7600000000000051, -16.239999999999995, -1.2399999999999949, 6.760000000000005, 11.760000000000005, 5.760000000000005, 6.760000000000005, 2.760000000000005, -2.239999999999995, 14.760000000000005, 26.760000000000005, -6.239999999999995, -13.239999999999995, 3.760000000000005, -7.239999999999995, 7.760000000000005, -9.239999999999995, 15.760000000000005, -13.239999999999995, 6.760000000000005, 3.760000000000005, 6.760000000000005, -1.2399999999999949, 14.760000000000005, 12.760000000000005, -12.239999999999995, 2.760000000000005, -4.239999999999995, 3.760000000000005, 3.760000000000005, -7.239999999999995, 6.760000000000005, 0.7600000000000051, 0.7600000000000051, -3.239999999999995, -2.239999999999995, 3.760000000000005, -3.239999999999995, -16.239999999999995, 17.760000000000005, 12.760000000000005, 8.760000000000005, -3.239999999999995, 3.760000000000005, -6.239999999999995, 5.760000000000005, 8.760000000000005, 10.760000000000005, -5.239999999999995, -1.2399999999999949, 18.760000000000005, 6.760000000000005, -1.2399999999999949, 9.760000000000005, -7.239999999999995, -15.239999999999995, -6.239999999999995, -1.2399999999999949, 5.760000000000005, -8.239999999999995, -5.239999999999995, -0.23999999999999488, 9.760000000000005, -19.239999999999995, 0.7600000000000051, -15.239999999999995, -3.239999999999995, 12.760000000000005, 10.760000000000005, -11.239999999999995, -10.239999999999995, 2.760000000000005, 10.760000000000005, -21.239999999999995, 7.760000000000005, -16.239999999999995, -15.239999999999995, 7.760000000000005, -6.239999999999995, 4.760000000000005, 8.760000000000005, 3.760000000000005, -2.239999999999995, 15.760000000000005, 8.760000000000005, 14.760000000000005, 14.760000000000005, 9.760000000000005, -5.239999999999995, 9.760000000000005, 16.760000000000005, 1.7600000000000051, -6.239999999999995, -9.239999999999995, -9.239999999999995, 10.760000000000005, -4.239999999999995, -4.239999999999995, 9.760000000000005, -0.23999999999999488, -0.23999999999999488, -11.239999999999995, -0.23999999999999488, -3.239999999999995, 21.760000000000005, 8.760000000000005, 0.7600000000000051, 12.760000000000005, -8.239999999999995, 6.760000000000005, -5.239999999999995, 11.760000000000005, -2.239999999999995, -0.23999999999999488, -6.239999999999995, -0.23999999999999488, 13.760000000000005, -2.239999999999995, 4.760000000000005, 2.760000000000005, 18.760000000000005, -2.239999999999995, 11.760000000000005, -9.239999999999995, -7.239999999999995, 15.760000000000005, 12.760000000000005, -5.239999999999995, -11.239999999999995, -1.2399999999999949, 6.760000000000005, 7.760000000000005, -0.23999999999999488, 0.7600000000000051, -4.239999999999995, 16.760000000000005, 2.760000000000005, 3.760000000000005, 7.760000000000005, 16.760000000000005, -3.239999999999995, 22.760000000000005, -12.239999999999995, 8.760000000000005, -17.239999999999995, -10.239999999999995, -1.2399999999999949, 6.760000000000005, 12.760000000000005, 10.760000000000005, 2.760000000000005, 3.760000000000005, 6.760000000000005, -2.239999999999995, 4.760000000000005, -1.2399999999999949, 11.760000000000005, -6.239999999999995, 0.7600000000000051, -12.239999999999995, -14.239999999999995, -3.239999999999995, 7.760000000000005, 0.7600000000000051, -9.239999999999995, 10.760000000000005, 12.760000000000005, 14.760000000000005, 7.760000000000005, -0.23999999999999488, -10.239999999999995, -9.239999999999995, 11.760000000000005, 5.760000000000005, 13.760000000000005, 16.760000000000005, -1.2399999999999949, 11.760000000000005, 8.760000000000005, -10.239999999999995, -0.23999999999999488, 5.760000000000005, 15.760000000000005, -0.23999999999999488, 1.7600000000000051, -14.239999999999995, -9.239999999999995, 19.760000000000005, 5.760000000000005, 0.7600000000000051, 6.760000000000005, 12.760000000000005, 1.7600000000000051, -1.2399999999999949, -2.239999999999995, 2.760000000000005, -8.239999999999995, -1.2399999999999949, -4.239999999999995, 14.760000000000005, -3.239999999999995, 2.760000000000005, -10.239999999999995, -0.23999999999999488, -13.239999999999995, 21.760000000000005, -8.239999999999995, -11.239999999999995, 10.760000000000005, 9.760000000000005, 0.7600000000000051, 12.760000000000005, 20.760000000000005, -3.239999999999995, 0.7600000000000051, -9.239999999999995, -13.239999999999995, 8.760000000000005, 4.760000000000005, 8.760000000000005, 0.7600000000000051, 7.760000000000005, -7.239999999999995, -6.239999999999995, -14.239999999999995, -7.239999999999995, 12.760000000000005, 7.760000000000005, 9.760000000000005, -18.239999999999995, -2.239999999999995, -1.2399999999999949, 14.760000000000005, 7.760000000000005, -7.239999999999995, -3.239999999999995, 3.760000000000005, -0.23999999999999488, 1.7600000000000051], [114.44, 50.44, 47.44, 54.44, 50.44, 62.44, 69.44, 57.44, 99.44, 114.44, 153.44, 139.44, 157.44, 179.44, 176.44, 171.44, 158.44, 209.44, 226.44, 209.44, 226.44, 195.44, 205.44, 204.44, 203.44, 197.44, 178.44, 194.44, 187.44, 146.44, 150.44, 178.44, 145.44, 150.44, 160.44, 127.44, 107.44, 132.44, 144.44, 124.44, 155.44, 115.44, 112.44, 132.44, 91.44, 120.44, 100.44, 89.44, 71.44, 72.44, 77.44, 70.44, 86.44, 65.44, 67.44, 84.44, 77.44, 54.44, 76.44, 47.44, 47.44, 48.44, 51.44, 40.44, 62.44, 36.44, 48.44, 45.44, 53.44, 47.44, 44.44, 45.44, 21.439999999999998, 44.44, 29.439999999999998, 17.439999999999998, 44.44, 25.439999999999998, 30.439999999999998, 26.439999999999998, 28.439999999999998, 32.44, 18.439999999999998, 35.44, 22.439999999999998, 13.439999999999998, 10.439999999999998, 37.44, 17.439999999999998, 32.44, 23.439999999999998, 11.439999999999998, 15.439999999999998, 29.439999999999998, 21.439999999999998, 15.439999999999998, 14.439999999999998, 6.439999999999998, 11.439999999999998, -2.5600000000000023, 33.44, 23.439999999999998, -13.560000000000002, 35.44, 16.439999999999998, 21.439999999999998, 25.439999999999998, 19.439999999999998, 5.439999999999998, 3.4399999999999977, 17.439999999999998, 14.439999999999998, 10.439999999999998, 24.439999999999998, 11.439999999999998, 20.439999999999998, -0.5600000000000023, 7.439999999999998, 15.439999999999998, 6.439999999999998, 28.439999999999998, 13.439999999999998, 11.439999999999998, 7.439999999999998, 15.439999999999998, 31.439999999999998, 9.439999999999998, -4.560000000000002, 1.4399999999999977, 11.439999999999998, 1.4399999999999977, 6.439999999999998, 26.439999999999998, 8.439999999999998, 12.439999999999998, 0.4399999999999977, -5.560000000000002, 18.439999999999998, 26.439999999999998, -11.560000000000002, 10.439999999999998, -4.560000000000002, 14.439999999999998, 15.439999999999998, 1.4399999999999977, 7.439999999999998, -11.560000000000002, 5.439999999999998, 11.439999999999998, 19.439999999999998, 16.439999999999998, 22.439999999999998, 13.439999999999998, 6.439999999999998, 1.4399999999999977, 15.439999999999998, 5.439999999999998, 4.439999999999998, 14.439999999999998, -1.5600000000000023, 3.4399999999999977, 12.439999999999998, 7.439999999999998, -1.5600000000000023, 10.439999999999998, 8.439999999999998, 22.439999999999998, 12.439999999999998, 6.439999999999998, -5.560000000000002, -1.5600000000000023, 3.4399999999999977, 4.439999999999998, 6.439999999999998, -4.560000000000002, 11.439999999999998, 10.439999999999998, -0.5600000000000023, 5.439999999999998, 4.439999999999998, 4.439999999999998, 4.439999999999998, 17.439999999999998, 14.439999999999998, 19.439999999999998, 1.4399999999999977, 2.4399999999999977, 13.439999999999998, 0.4399999999999977, -10.560000000000002, 5.439999999999998, 2.4399999999999977, 8.439999999999998, 28.439999999999998, -6.560000000000002, 5.439999999999998, 2.4399999999999977, 14.439999999999998, -4.560000000000002, 4.439999999999998, -4.560000000000002, 21.439999999999998, 5.439999999999998, 20.439999999999998, 11.439999999999998, 5.439999999999998, 6.439999999999998, 7.439999999999998, 4.439999999999998, -8.560000000000002, 10.439999999999998, -0.5600000000000023, -14.560000000000002, 21.439999999999998, 13.439999999999998, 8.439999999999998, -6.560000000000002, -7.560000000000002, -5.560000000000002, 2.4399999999999977, 12.439999999999998, -6.560000000000002, -11.560000000000002, 12.439999999999998, 5.439999999999998, 6.439999999999998, -1.5600000000000023, 18.439999999999998, 7.439999999999998, 6.439999999999998, -5.560000000000002, 4.439999999999998, 6.439999999999998, -13.560000000000002, 6.439999999999998, 6.439999999999998, 4.439999999999998, 18.439999999999998, 24.439999999999998, 46.44, 45.44, 62.44, 112.44, 147.44, 128.44, 131.44, 78.44, 56.44, 52.44, 58.44, 26.439999999999998, 41.44, 25.439999999999998, 25.439999999999998, 29.439999999999998, 48.44, 21.439999999999998, 5.439999999999998, 25.439999999999998, 14.439999999999998, 37.44, 9.439999999999998, 28.439999999999998, 26.439999999999998, 35.44, 77.44, 109.44, 127.44, 107.44, 113.44, 95.44, 113.44, 109.44, 68.44, 71.44, 37.44, 18.439999999999998, 7.439999999999998, 1.4399999999999977, 12.439999999999998, 10.439999999999998, -4.560000000000002, 12.439999999999998, 1.4399999999999977, 0.4399999999999977, 0.4399999999999977, 1.4399999999999977, 12.439999999999998, 2.4399999999999977, 4.439999999999998, -17.560000000000002, 12.439999999999998, -13.560000000000002, -2.5600000000000023, 13.439999999999998, 10.439999999999998, -6.560000000000002, 3.4399999999999977, -3.5600000000000023, -0.5600000000000023, -0.5600000000000023, -5.560000000000002, -14.560000000000002, 32.44, 6.439999999999998, -6.560000000000002, -13.560000000000002, 5.439999999999998, -8.560000000000002, -7.560000000000002, 14.439999999999998, 8.439999999999998, 10.439999999999998, 4.439999999999998, 5.439999999999998, 4.439999999999998, 6.439999999999998, 18.439999999999998, 13.439999999999998, 6.439999999999998, 8.439999999999998, 7.439999999999998, -1.5600000000000023, 18.439999999999998, -12.560000000000002, 13.439999999999998, 2.4399999999999977, -11.560000000000002, 8.439999999999998, -4.560000000000002, 1.4399999999999977, -2.5600000000000023, 4.439999999999998, 5.439999999999998, -5.560000000000002, 13.439999999999998, -2.5600000000000023, -8.560000000000002, 3.4399999999999977, -0.5600000000000023, -14.560000000000002, 8.439999999999998, 26.439999999999998, -3.5600000000000023, -8.560000000000002, 3.4399999999999977, -5.560000000000002, 6.439999999999998, -6.560000000000002, 5.439999999999998, -4.560000000000002, -5.560000000000002, -2.5600000000000023, -4.560000000000002, -1.5600000000000023, 6.439999999999998, 7.439999999999998, 18.439999999999998, 6.439999999999998, -0.5600000000000023, -14.560000000000002, 0.4399999999999977, 12.439999999999998, -6.560000000000002, 1.4399999999999977, 12.439999999999998, -5.560000000000002, -6.560000000000002, 21.439999999999998, 3.4399999999999977, 1.4399999999999977, 9.439999999999998, 13.439999999999998, 8.439999999999998, 9.439999999999998, -15.560000000000002, -12.560000000000002, -18.560000000000002, 7.439999999999998, -0.5600000000000023, 16.439999999999998, -1.5600000000000023, 3.4399999999999977, 5.439999999999998, 19.439999999999998, 18.439999999999998, -15.560000000000002, -6.560000000000002, 7.439999999999998, 19.439999999999998, -6.560000000000002, 20.439999999999998, 1.4399999999999977, -8.560000000000002, 22.439999999999998, -3.5600000000000023, -1.5600000000000023, 6.439999999999998, 1.4399999999999977, 22.439999999999998, 0.4399999999999977, 10.439999999999998, -8.560000000000002, 4.439999999999998, 18.439999999999998, 13.439999999999998, 6.439999999999998, 1.4399999999999977, 6.439999999999998, 19.439999999999998, 14.439999999999998, 8.439999999999998, 8.439999999999998, -4.560000000000002, 10.439999999999998, -1.5600000000000023, 13.439999999999998, 1.4399999999999977, 2.4399999999999977, 3.4399999999999977, -5.560000000000002, -14.560000000000002, 1.4399999999999977, 14.439999999999998, 5.439999999999998, 11.439999999999998, -6.560000000000002, -3.5600000000000023, 8.439999999999998, -7.560000000000002, 13.439999999999998, 0.4399999999999977, -8.560000000000002, -6.560000000000002, -7.560000000000002, 12.439999999999998, -8.560000000000002, 0.4399999999999977, -5.560000000000002, -1.5600000000000023, 14.439999999999998, 7.439999999999998, -20.560000000000002, -12.560000000000002, -4.560000000000002, 1.4399999999999977, -1.5600000000000023, 14.439999999999998, -8.560000000000002, -2.5600000000000023, 1.4399999999999977, 4.439999999999998, 8.439999999999998, 6.439999999999998, 15.439999999999998, -8.560000000000002, 1.4399999999999977, 6.439999999999998, 8.439999999999998, -5.560000000000002, 7.439999999999998, -5.560000000000002, 15.439999999999998, 5.439999999999998, -4.560000000000002, 0.4399999999999977, 0.4399999999999977, 6.439999999999998, 8.439999999999998, -2.5600000000000023, 11.439999999999998, 11.439999999999998, 1.4399999999999977, 18.439999999999998, -0.5600000000000023, 15.439999999999998, 26.439999999999998, 5.439999999999998, 2.4399999999999977, -4.560000000000002, 13.439999999999998, 15.439999999999998, 6.439999999999998, 4.439999999999998, 6.439999999999998, 6.439999999999998, -2.5600000000000023, 5.439999999999998, -10.560000000000002, -4.560000000000002, -3.5600000000000023, -1.5600000000000023, 10.439999999999998, 1.4399999999999977, 3.4399999999999977, 9.439999999999998, 19.439999999999998, 24.439999999999998, 4.439999999999998, -11.560000000000002, 2.4399999999999977, 15.439999999999998, -3.5600000000000023, 3.4399999999999977, -1.5600000000000023, 8.439999999999998, 15.439999999999998, 13.439999999999998, 6.439999999999998, 8.439999999999998, 2.4399999999999977, -1.5600000000000023, 4.439999999999998, 8.439999999999998, -16.560000000000002, -8.560000000000002, 5.439999999999998, 5.439999999999998, 11.439999999999998, 3.4399999999999977, 1.4399999999999977, -0.5600000000000023, 12.439999999999998, 1.4399999999999977, 8.439999999999998, 2.4399999999999977, 19.439999999999998, 0.4399999999999977, 0.4399999999999977, 2.4399999999999977, -15.560000000000002, -8.560000000000002, 5.439999999999998, -5.560000000000002, 9.439999999999998, 1.4399999999999977, -4.560000000000002, -7.560000000000002, -13.560000000000002, 6.439999999999998, 11.439999999999998, -13.560000000000002, -3.5600000000000023, 4.439999999999998, 7.439999999999998, 13.439999999999998, 7.439999999999998, -3.5600000000000023, -1.5600000000000023, -17.560000000000002, -22.560000000000002, 4.439999999999998, 11.439999999999998, -3.5600000000000023, -2.5600000000000023, 4.439999999999998, -7.560000000000002, 12.439999999999998, 7.439999999999998], [94.48, 44.480000000000004, 38.480000000000004, 34.480000000000004, 68.48, 47.480000000000004, 60.480000000000004, 92.48, 105.48, 107.48, 123.48, 163.48000000000002, 163.48000000000002, 146.48000000000002, 180.48000000000002, 158.48000000000002, 179.48000000000002, 176.48000000000002, 184.48000000000002, 207.48000000000002, 225.48000000000002, 243.48000000000002, 198.48000000000002, 171.48000000000002, 182.48000000000002, 189.48000000000002, 210.48000000000002, 170.48000000000002, 199.48000000000002, 169.48000000000002, 132.48000000000002, 190.48000000000002, 143.48000000000002, 124.48, 171.48000000000002, 181.48000000000002, 130.48000000000002, 153.48000000000002, 138.48000000000002, 117.48, 122.48, 120.48, 128.48000000000002, 112.48, 87.48, 106.48, 94.48, 95.48, 87.48, 91.48, 89.48, 71.48, 65.48, 72.48, 74.48, 62.480000000000004, 76.48, 48.480000000000004, 61.480000000000004, 68.48, 74.48, 50.480000000000004, 49.480000000000004, 57.480000000000004, 39.480000000000004, 25.480000000000004, 29.480000000000004, 36.480000000000004, 20.480000000000004, 33.480000000000004, 34.480000000000004, 41.480000000000004, 34.480000000000004, 67.48, 37.480000000000004, 5.480000000000004, 21.480000000000004, 16.480000000000004, 28.480000000000004, 17.480000000000004, 29.480000000000004, 7.480000000000004, 41.480000000000004, 23.480000000000004, 20.480000000000004, 26.480000000000004, 9.480000000000004, 12.480000000000004, 29.480000000000004, 7.480000000000004, 14.480000000000004, 5.480000000000004, 8.480000000000004, 15.480000000000004, 15.480000000000004, 13.480000000000004, -4.519999999999996, 14.480000000000004, 7.480000000000004, 2.480000000000004, 2.480000000000004, 4.480000000000004, -2.519999999999996, 15.480000000000004, 24.480000000000004, 22.480000000000004, 20.480000000000004, 9.480000000000004, 13.480000000000004, 4.480000000000004, 8.480000000000004, 21.480000000000004, 9.480000000000004, 26.480000000000004, 17.480000000000004, 10.480000000000004, -1.519999999999996, 2.480000000000004, 1.480000000000004, 19.480000000000004, -0.519999999999996, 14.480000000000004, 2.480000000000004, 15.480000000000004, 23.480000000000004, 20.480000000000004, 1.480000000000004, 19.480000000000004, 19.480000000000004, -3.519999999999996, 7.480000000000004, -6.519999999999996, 8.480000000000004, 7.480000000000004, 0.480000000000004, 10.480000000000004, 4.480000000000004, -6.519999999999996, -6.519999999999996, 0.480000000000004, -1.519999999999996, 2.480000000000004, 8.480000000000004, 12.480000000000004, 26.480000000000004, 7.480000000000004, 3.480000000000004, 19.480000000000004, 3.480000000000004, 12.480000000000004, 10.480000000000004, 0.480000000000004, 14.480000000000004, 9.480000000000004, -6.519999999999996, 10.480000000000004, -1.519999999999996, 11.480000000000004, 14.480000000000004, -9.519999999999996, 13.480000000000004, 6.480000000000004, 3.480000000000004, 5.480000000000004, 12.480000000000004, 0.480000000000004, 7.480000000000004, 1.480000000000004, -2.519999999999996, 7.480000000000004, 8.480000000000004, -5.519999999999996, -9.519999999999996, 6.480000000000004, 17.480000000000004, 6.480000000000004, 6.480000000000004, 7.480000000000004, 6.480000000000004, 9.480000000000004, 21.480000000000004, 11.480000000000004, -4.519999999999996, -4.519999999999996, -6.519999999999996, 3.480000000000004, -9.519999999999996, -1.519999999999996, 20.480000000000004, 18.480000000000004, 6.480000000000004, -5.519999999999996, 3.480000000000004, 5.480000000000004, -0.519999999999996, 1.480000000000004, 1.480000000000004, 4.480000000000004, 2.480000000000004, -2.519999999999996, -3.519999999999996, -12.519999999999996, 9.480000000000004, 6.480000000000004, 0.480000000000004, -6.519999999999996, 6.480000000000004, 0.480000000000004, -11.519999999999996, 6.480000000000004, 3.480000000000004, 5.480000000000004, -5.519999999999996, 3.480000000000004, 23.480000000000004, 16.480000000000004, -4.519999999999996, 13.480000000000004, -2.519999999999996, -5.519999999999996, 2.480000000000004, -6.519999999999996, 2.480000000000004, 7.480000000000004, -6.519999999999996, -0.519999999999996, -2.519999999999996, 8.480000000000004, 4.480000000000004, 7.480000000000004, -9.519999999999996, 7.480000000000004, 1.480000000000004, -6.519999999999996, 1.480000000000004, 17.480000000000004, 9.480000000000004, 13.480000000000004, 23.480000000000004, 32.480000000000004, 47.480000000000004, 104.48, 93.48, 81.48, 119.48, 87.48, 49.480000000000004, 43.480000000000004, 47.480000000000004, 53.480000000000004, 51.480000000000004, 15.480000000000004, 45.480000000000004, 16.480000000000004, 23.480000000000004, 34.480000000000004, 27.480000000000004, 38.480000000000004, 27.480000000000004, 27.480000000000004, 28.480000000000004, 23.480000000000004, 30.480000000000004, 41.480000000000004, 35.480000000000004, 67.48, 108.48, 95.48, 119.48, 83.48, 94.48, 87.48, 46.480000000000004, 66.48, 26.480000000000004, 21.480000000000004, 15.480000000000004, 2.480000000000004, -1.519999999999996, -2.519999999999996, -0.519999999999996, -0.519999999999996, 9.480000000000004, 4.480000000000004, -0.519999999999996, -0.519999999999996, 4.480000000000004, -7.519999999999996, -1.519999999999996, 12.480000000000004, 6.480000000000004, 12.480000000000004, 6.480000000000004, -3.519999999999996, 4.480000000000004, 13.480000000000004, -0.519999999999996, 9.480000000000004, 23.480000000000004, -3.519999999999996, 4.480000000000004, 5.480000000000004, 8.480000000000004, -0.519999999999996, -3.519999999999996, -10.519999999999996, 3.480000000000004, 4.480000000000004, 16.480000000000004, -10.519999999999996, 0.480000000000004, -8.519999999999996, -4.519999999999996, -2.519999999999996, -18.519999999999996, 3.480000000000004, 3.480000000000004, -3.519999999999996, -6.519999999999996, 13.480000000000004, 2.480000000000004, 6.480000000000004, 5.480000000000004, 0.480000000000004, 8.480000000000004, -21.519999999999996, 6.480000000000004, -5.519999999999996, 0.480000000000004, -14.519999999999996, 14.480000000000004, 2.480000000000004, 12.480000000000004, -4.519999999999996, -0.519999999999996, 2.480000000000004, -6.519999999999996, -1.519999999999996, -1.519999999999996, 9.480000000000004, 1.480000000000004, -10.519999999999996, -7.519999999999996, 2.480000000000004, -7.519999999999996, 6.480000000000004, -9.519999999999996, 7.480000000000004, -2.519999999999996, 10.480000000000004, -2.519999999999996, -8.519999999999996, 10.480000000000004, -18.519999999999996, 18.480000000000004, -12.519999999999996, 3.480000000000004, 7.480000000000004, 12.480000000000004, 4.480000000000004, -1.519999999999996, 5.480000000000004, -9.519999999999996, -17.519999999999996, -8.519999999999996, 0.480000000000004, -4.519999999999996, 2.480000000000004, 2.480000000000004, 11.480000000000004, 13.480000000000004, -5.519999999999996, 10.480000000000004, -3.519999999999996, 10.480000000000004, 0.480000000000004, -8.519999999999996, -0.519999999999996, 2.480000000000004, 3.480000000000004, 2.480000000000004, 8.480000000000004, 5.480000000000004, 10.480000000000004, -1.519999999999996, -12.519999999999996, 5.480000000000004, -13.519999999999996, -11.519999999999996, 4.480000000000004, 7.480000000000004, -14.519999999999996, 2.480000000000004, 13.480000000000004, -7.519999999999996, 4.480000000000004, 1.480000000000004, -2.519999999999996, 5.480000000000004, 4.480000000000004, 3.480000000000004, 4.480000000000004, 20.480000000000004, 13.480000000000004, 1.480000000000004, 5.480000000000004, -10.519999999999996, -2.519999999999996, -5.519999999999996, 2.480000000000004, -5.519999999999996, 2.480000000000004, -22.519999999999996, -0.519999999999996, -4.519999999999996, -3.519999999999996, 6.480000000000004, 4.480000000000004, 4.480000000000004, 1.480000000000004, 0.480000000000004, 2.480000000000004, 13.480000000000004, 6.480000000000004, 10.480000000000004, 21.480000000000004, -5.519999999999996, -2.519999999999996, 20.480000000000004, -3.519999999999996, 4.480000000000004, -8.519999999999996, 1.480000000000004, 7.480000000000004, -4.519999999999996, -7.519999999999996, 3.480000000000004, -6.519999999999996, 12.480000000000004, -6.519999999999996, -3.519999999999996, 3.480000000000004, 2.480000000000004, 3.480000000000004, -7.519999999999996, 1.480000000000004, 5.480000000000004, 2.480000000000004, 9.480000000000004, -2.519999999999996, -9.519999999999996, -3.519999999999996, 0.480000000000004, -14.519999999999996, -4.519999999999996, 1.480000000000004, 9.480000000000004, 16.480000000000004, 11.480000000000004, 9.480000000000004, 3.480000000000004, -4.519999999999996, 8.480000000000004, 13.480000000000004, 2.480000000000004, -2.519999999999996, -0.519999999999996, -1.519999999999996, -13.519999999999996, -8.519999999999996, -0.519999999999996, 12.480000000000004, -4.519999999999996, -3.519999999999996, -10.519999999999996, 9.480000000000004, -4.519999999999996, 8.480000000000004, 4.480000000000004, -0.519999999999996, -9.519999999999996, 16.480000000000004, -7.519999999999996, 14.480000000000004, 2.480000000000004, 1.480000000000004, 1.480000000000004, -4.519999999999996, -8.519999999999996, 10.480000000000004, 4.480000000000004, 3.480000000000004, 5.480000000000004, 2.480000000000004, 6.480000000000004, 5.480000000000004, 17.480000000000004, -1.519999999999996, -4.519999999999996, -2.519999999999996, 14.480000000000004, -1.519999999999996, 16.480000000000004, -12.519999999999996, -8.519999999999996, -2.519999999999996, -9.519999999999996, -0.519999999999996, -16.519999999999996, 9.480000000000004, 5.480000000000004, 5.480000000000004, -13.519999999999996, 1.480000000000004, 20.480000000000004, 5.480000000000004, -13.519999999999996, 23.480000000000004, -4.519999999999996, 4.480000000000004, 5.480000000000004, -1.519999999999996, 4.480000000000004, 10.480000000000004, -6.519999999999996, 9.480000000000004, 3.480000000000004, 6.480000000000004, -0.519999999999996, -4.519999999999996, 10.480000000000004, 18.480000000000004, 7.480000000000004, 12.480000000000004, 4.480000000000004, -9.519999999999996, 9.480000000000004, -4.519999999999996, 12.480000000000004, 9.480000000000004, 4.480000000000004, -5.519999999999996, -2.519999999999996, -22.519999999999996, 0.480000000000004, -9.519999999999996, -6.519999999999996, 3.480000000000004, -7.519999999999996, -4.519999999999996, -1.519999999999996, -1.519999999999996, 13.480000000000004, -2.519999999999996, 1.480000000000004, -5.519999999999996, 19.480000000000004, 0.480000000000004, 4.480000000000004]]
  in  "?":T1(tab)=enum."Raw Counts combined"
  out "NRB WV Offline":dbl[][](graph)=[[8.417004443952767e-06, 3.777846374018435e-05, 0.00010495950595860812, 0.00023051318603964705, 0.00044311255965762743, 0.0007715798096324077, 0.0012664936261046194, 0.00194342800799893, 0.0028080258441383773, 0.00393639016463193, 0.005251684977648643, 0.006469469970496937, 0.007602102157360491, 0.008773828116546797, 0.010144850443098923, 0.011862644220783139, 0.013831515592834076, 0.016124460726861467, 0.018779564681224586, 0.021146579464015436, 0.023176578510579457, 0.025255732903990732, 0.026818020699673924, 0.028284386818955926, 0.02978277271959251, 0.031007947886778683, 0.03235641935567802, 0.033499995336881284, 0.03412386741170296, 0.03502064141409781, 0.03541512954841668, 0.03562593200238588, 0.036640155271657135, 0.037093809094988134, 0.03729784916702316, 0.037408577556670174, 0.03744840561340627, 0.037851639152133805, 0.038415738147179204, 0.03858655185308906, 0.03887759435899143, 0.03890195615209426, 0.038563023079122766, 0.0388240276853941, 0.03939906192425048, 0.040028441764994094, 0.04037612721820537, 0.03970846802266822, 0.038743507298406255, 0.03890259876638325, 0.03958207168229139, 0.04066058471091726, 0.040173960668825656, 0.03911917658545836, 0.039185947326161014, 0.03851741559329875, 0.038000738759134414, 0.03839483522450416, 0.038505908438785715, 0.037589779982924454, 0.03683522288024606, 0.036877849361392614, 0.03710303169891088, 0.036508773166941774, 0.03566829954710531, 0.03439779293683489, 0.03342202497800318, 0.03487796054696994, 0.03377822791274589, 0.030824665795632977, 0.030916522055162484, 0.030714649945591067, 0.029822620432927004, 0.028641930264031053, 0.029482878779960767, 0.02941391878542321, 0.02767986790416879, 0.02629110834172519, 0.024508779659559155, 0.026836521067004137, 0.02760504548271547, 0.026110972405088452, 0.026381997591239863, 0.025900980032971192, 0.02492291450890634, 0.027294849183595347, 0.026026658615171203, 0.02324438384188751, 0.024513045669805444, 0.024375050592058946, 0.025590857006541772, 0.02600806770297486, 0.02672809108194418, 0.026764058409616032, 0.02533006869809887, 0.027067234223134822, 0.02602655604677008, 0.02173820696568368, 0.022420245963781685, 0.023510656867348732, 0.022139902524148318, 0.022888122040569486, 0.023525003354831514, 0.027383593967650596, 0.026693242301129152, 0.026244301793987165, 0.024046068456391963, 0.020895466913336037, 0.022884589641448204, 0.02333291868960292, 0.02467661519731887, 0.024628696604455068, 0.024189483203616875, 0.021858459638980195, 0.023329844730351018, 0.028556048397219966, 0.025362657414347692, 0.019744456945177482, 0.02282540983495217, 0.02414105147275147, 0.023823567652962424, 0.02728332788387843, 0.030416482269541325, 0.026838106498144176, 0.02364515999601601, 0.02593745325609509, 0.027746180330489804, 0.022891876102645273, 0.015378475911787747, 0.017968190268610976, 0.021722353163242714, 0.023619895334405082, 0.0203954771022273, 0.018304406123161372, 0.021452562095269835, 0.02185257390986505, 0.02096245008521529, 0.021957796706134715, 0.024752692227707717, 0.024637923060094123, 0.019069340137890325, 0.019318705309746262, 0.02167433028265778, 0.01702830188619889, 0.02117969068365927, 0.028685784932340745, 0.024370985173724227, 0.02292867598538887, 0.017161644178891895, 0.011750492185372474, 0.01869910116842371, 0.0207692264419869, 0.01712133812897434, 0.017527671357886118, 0.01741402723555863, 0.01731965623385488, 0.019701792409329243, 0.020008244409837617, 0.020013155569406377, 0.02026568500363132, 0.018958614449192352, 0.012987312260112256, 0.01640672125329408, 0.016461385181502104, 0.015857798721756806, 0.017227434763329726, 0.017496699433834972, 0.020673935243190868, 0.01982612464396358, 0.03167610481222818, 0.0298403938553557, 0.02147575038570657, 0.021070712627150937, 0.014949465806679859, 0.024277153698263356, 0.02387698493058203, 0.01529787474847502, 0.02355532709600905, 0.023890910956699186, 0.01734646435630372, 0.019620489374965827, 0.021034885683519137, 0.01723272770096553, 0.024317379014202025, 0.02521955099360469, 0.015377773310666686, 0.026686824428998227, 0.028946912001445804, 0.01681661857797192, 0.013990678369410339, 0.017693738519428844, 0.021472245806385414, 0.012070205831947572, 0.008981012770316018, 0.02339767912661407, 0.030831874072932468, 0.026769962870599143, 0.018713915623162714, 0.0056772213155333465, 0.009895540819703548, 0.012737658120027376, 0.006564588898914189, 0.016467070514012108, 0.02688331827020619, 0.02696344710720438, 0.018119110292434213, 0.014870183943209252, 0.02283124988058921, 0.03209177529349085, 0.028053317313822004, 0.019691888111602412, 0.01677839848063801, 0.01574471692033561, 0.012081627815981, 0.014523235149612243, 0.02630726762864449, 0.03557532467785083, 0.034238627356240406, 0.038545010903432785, 0.022520596446559352, 0.004916066514773927, 0.007335218457959199, 0.006965813049054886, 0.02477554486444605, 0.016848069939622876, 0.003071638703181543, 0.01748748007834838, 0.009957111914174813, 0.01142283599332012, 0.013028925425540745, 0.015596618631394943, 0.04785434824101969, 0.06628137908079844, 0.08975756732778602, 0.13020048236839285, 0.18907552664033977, 0.2259926927451923, 0.22765566977104562, 0.23582896617213436, 0.24670184141392165, 0.26816447145128625, 0.27097181895471084, 0.24003780125309626, 0.23667052020643484, 0.25478714399183167, 0.25103856783487527, 0.23076579543218403, 0.22253394348904998, 0.1922134400581615, 0.1403022441095343, 0.1229362550535619, 0.1109824238242298, 0.1074488448991332, 0.12787083370046198, 0.12581759916737337, 0.1458256758838165, 0.17828793543320653, 0.19243552481529635, 0.23220663371788738, 0.25932404346771054, 0.27960199286818516, 0.31016804412683735, 0.3492841025592465, 0.43202711929699117, 0.5441565393533199, 0.6935342671473717, 0.8641130637222598, 1.0169857206026816, 1.1538475357164268, 1.2550424574293555, 1.3720590455319228, 1.5603775971679725, 1.7213116881943318, 1.809754338746903, 1.7527602242596538, 1.4557195023077085, 1.0036188298089705, 0.5676997248922993, 0.2683450081152654, 0.09709215380652389, 0.016248378679083707, -0.006102579840166127, 0.012797099743613134, 0.014654112871425332, 0.026853903116074985, 0.016473480377300915, -0.00469738497654194, 0.010346856223849675, 0.021393803612758357, 0.028817431526672547, 0.004258047178326554, -0.0024349777701002328, 0.01907588389717869, 0.011445014558171433, 0.006567683264719156, 0.03078975678147716, 0.026168533943751144, 0.014675849524508995, 0.0175156211030623, 0.006792203318870715, 0.018643626052148053, 0.03854233643154035, 0.006828193521364587, 9.310157824924474e-05, 0.03330176843835326, 0.04110812119969961, 0.03704255532083559, 0.011729938969007788, 0.018915936123218312, 0.03861192026796571, 0.02435131635817891, 0.021523509643420452, 0.006428109506754996, -0.024192548771537287, -0.01587201543071082, 0.014534101811432469, 0.04334644864749878, 0.040076832445805975, 0.0033339982441486704, -0.006736761400308365, 0.0025861100497806024, 0.004532364326174926, 0.01072966940096525, 0.03332681887219371, 0.031566580339381534, -0.00617714060962698, -0.003639134973681453, 0.012831538165906958, 0.023814393008452832, 0.04005806636380571, 0.02026568141213431, -0.006889400856808962, -0.006688115222464689, 0.03981347272117299, 0.05639678907967182, 0.015566711708443107, 0.006083715540361812, 0.026261037628781025, 0.04101441516897273, 0.04707974024612761, 0.020872034864120582, 0.017664576236715596, 0.04611059459141952, 0.02849747627936288, -0.009915846136059723, 0.02030877188291695, 0.05009309865042654, 0.030755417667643194, 0.029732040430369974, 0.010586348575603597, -0.0010900527871446576, 0.007994123244684244, -0.005605332362874124, -0.021280528677063256, -0.0271968640806867, -0.002647891373067867, -0.03266779707371711, -0.05628777453025922, 0.01720629694979472, 0.0287974764187627, 0.013688214784742461, 0.00386290982825141, 0.003307121778219752, 0.007968122829053589, -0.019268289977972617, -0.03272216667170967, -0.015202929643909973, 0.030684760174124023, 0.024589526111395404, -0.010955270604883065, 0.013552745395778143, 0.023930238563095816, 0.03000074169924868, 0.04272168642882764, 0.023855800778803147, 0.02150622770925634, 0.044810539613904854, 0.0409805305009384, 0.030659092709244124, 0.0006198339305055077, -0.016702856030091584, -0.005445627397475567, 0.00544848617225571, -0.028592477196475057, -0.06931821748693649, -0.011270627878797122, 0.02491499588422349, 0.02421967138511268, 0.019705053950862823, 0.017474744953750357, -0.0035289531654773697, -0.007753647713326499, 0.038716290465695136, 0.04231334779457208, 0.03330236450567607, 0.016814541868918276, 0.029670960421857344, -0.010074281042131436, -0.048825468782231936, -0.0014156414797213098, 0.02745456452058817, 0.07908780557856951, 0.014568777077058887, -0.027537791612550447, 0.0644665209869607, 0.07832297974851667, 0.01340830062649336, 0.00800580936178661, 0.017203939720143665, -0.021183034025484757, -0.00019976961048384867, 0.0511006288158511, 0.041823254790017715, 0.021568491647962217, 0.016015086126594292, -0.009869133466479413, -0.010678283584609562, -0.0047984593382851964, -0.030197362341271107, -0.026285316807730493, 0.05025219853060314, 0.03723066158089971, -0.0435120396782839, -0.029150654032817386, -0.005553882012494226, 0.061786527055640666, 0.06427317800245642, -0.0012195878196824847, -0.0004191793987496896, -0.022287737893836663, -0.0020503923998730954, 0.06272180683222722, 0.0601382132081228, 0.009883685214301361, -0.027989163092767864, -0.02541195096853322, -0.005244597086679473, 0.0004033402014085832, -0.0255518279678898, -0.030332243325829372, 0.07771439104650905, 0.10053016257790409, 0.045326260594520607, 0.0332265276801594, 0.0010668594866753156, -0.01417550320325517, -0.04115071126384698, -0.010127213339855017, 0.06709309131650192, 0.07182719083405392, 0.0224777908270675, 0.02817054163904619, 0.06649614401911809, 0.009461403000921041, -0.005232151925861605, 0.026394384885833677, 0.055554692647936846, 0.03880039791289731, 0.009670951530386045, 0.03566438021021902, 0.034190593995347095, -0.01801551699678214, -0.06551024768564083, -0.050705530965727066, 0.003532620238483738, 0.07750129515435333, 0.056818495050015363, 0.03451729024317206, 0.057306205217578295, 0.020783232516593444, -0.04641695993547782, -0.04490661675263582, -0.019618571473253715, -0.031018682180952453, -0.042514541577875806, 0.02305400092900598, 0.043830478584196836, 0.040511689138460524, 0.06480094082269071, 0.07945270638086656, 0.07395706927402887, -0.06972524191788461, -0.09811449791507533, 0.009470543750346908, 0.04608574819037628, 0.07472669881365222, 0.0625685122606428, 0.022666396749745903, -0.019920916142833294, -0.05838763267416668, -0.07736909859385267, -0.01990103058403915, 0.061990561696228436, 0.007728132960977308, -0.0067291413850605695, 0.005096907580987854, 0.031083639953508265, 0.01735874361302521, -0.032195709145069, -0.009055806470244468, -0.001121392380449164, -0.06900893147940347, -0.06374321983457303, 0.05393965183812454, 0.04884796217898643, -0.014601362889605222, 0.023621337291489915, 0.04180018565247476, -0.030094683860411052, -0.03847261894796629, 0.006839515088484497, 0.06599964304958028, 0.06712224337905011, 0.028328325576476455, 0.010432136779510848, -0.062124293425105934, -0.031926174840129384, 0.06696792533008394, 0.09790262305492584, 0.039652980887419684, -0.032719339435591764, 0.05756290594325096, 0.09192940404777669, 0.025532636308873594, -0.015718495236792644, -0.06607035421728576, -0.05050780854997524, 0.07690519575535266, 0.08118044775633655, -0.06707904733202577, -0.009596032286042095, 0.10038922893144334, 0.0021526956646553057, -0.005645504410892656, -0.029800090603445455, -0.10100918181022817, -0.14527744936701384, -0.10303215224956892, 0.003155813747558175, 0.018175031003382854, 0.07144443251862566, 0.056589782888370285, -0.05394411496953414, -0.059651880455095736, 0.05494121102800441, 0.04698186727542864, 0.014062318822590857, 0.009181188781742096, -0.03336035738054375, -0.016257409908556703, 0.010279337062240717, -0.02071338721927162, 0.06493776371947058, 0.1596128925861705, 0.055626712351279486, -0.00781280771768218, -0.019051963055981294, 0.0, 0.0, 0.0]] caption="Water Vapor Number Density"
  out "NRB HSRL Combined":dbl[][](graph)=[[3.0526048681727356e-05, 7.570043679600625e-05, 0.00016642077996791477, 0.0002977525803457301, 0.0004987689347039542, 0.0008986121856749108, 0.0014010112943981723, 0.0021507223773845063, 0.0032497139060569543, 0.004920500743995497, 0.0072497360904537995, 0.009419172516841354, 0.01124157056497073, 0.013634433307862617, 0.015954356992209477, 0.017251378017404326, 0.020252431938952827, 0.025166161394300023, 0.0294829488900197, 0.035011419874103146, 0.038949276237536024, 0.040371261022968, 0.04326635486521748, 0.04473984247875559, 0.04758138254385749, 0.05175823740835707, 0.05388378765575019, 0.055592070586187696, 0.057405197922313, 0.05808688583425708, 0.06031398749511843, 0.06236518481409098, 0.06128736782293099, 0.06652017049604439, 0.07145909934565435, 0.06976136617006387, 0.07168912698534612, 0.07339126801822282, 0.07231696186019938, 0.07803264751287756, 0.07952581030172191, 0.07599660401956698, 0.07914736492481837, 0.08027171703287062, 0.08268231892736376, 0.08698288518865252, 0.0814722145943729, 0.07378791883369316, 0.0765153334960119, 0.08529562588382966, 0.08309429875247386, 0.07411148622221483, 0.07455056179121475, 0.08394989993059328, 0.09126670888625463, 0.08545674163534979, 0.07981772493688463, 0.08357209274784853, 0.08180874003464668, 0.07963408840695574, 0.07673224215360953, 0.0794203225113666, 0.07949770345119792, 0.07557837525849832, 0.07662538881320807, 0.06903605104770574, 0.07043570932811788, 0.08258497089772611, 0.08540739423447115, 0.0817161552467189, 0.07730764780877092, 0.060488243257866794, 0.0573472074997017, 0.0638953742438423, 0.055874997447816696, 0.06466278224089704, 0.06590805875957421, 0.059954634804601774, 0.06445467558832121, 0.05928360813392631, 0.05353213487623129, 0.06467082131565363, 0.07196185716510328, 0.05256376312171658, 0.046132477518666955, 0.05247246025654599, 0.060861338831640695, 0.06196318897690433, 0.05994440673197211, 0.06768576037662911, 0.05744545459774019, 0.0510407379632796, 0.06136212936166391, 0.05885718368455689, 0.06687606059932355, 0.0563021428598936, 0.05377219033401227, 0.07419547997896661, 0.06142145147083539, 0.06385117995663246, 0.0687538186339989, 0.034852866622299, 0.05728457166194854, 0.10360085681025274, 0.08169624023352268, 0.07750139986096041, 0.06904128177476229, 0.04918814350015792, 0.03933245610507787, 0.01621289445845234, 0.02961994307687374, 0.0667438979572068, 0.08253830549013912, 0.09117816002585252, 0.09017801073298974, 0.04507691015663736, 0.028053008360580604, 0.03457115519322223, 0.051345706927613546, 0.061861298731281884, 0.03865953912286229, 0.041647692131857234, 0.04591098182087288, 0.05029673537363817, 0.07020324266880186, 0.06632475400061216, 0.05848138599219539, 0.0613433208600233, 0.05771419983201786, 0.06061080248036521, 0.06763454637539305, 0.07691256224279172, 0.04601059993768552, 0.04670508974396977, 0.07326467032187475, 0.04446477292020588, 0.06361496183431771, 0.09832623722014784, 0.035787353305666236, 0.005406774055472356, 0.043876545539470006, 0.058011404457538766, 0.09268355018755366, 0.12095791918476882, 0.0994379695717806, 0.05292435680111497, 0.03406384209936981, 0.07251393977995332, 0.128628447756633, 0.11173539348061423, 0.05751003693899362, 0.06282728552457002, 0.04243677434409648, 0.05514434462682587, 0.09468678845456666, 0.06521833222067604, 0.07771525478723534, 0.09937153267459368, 0.06675444358753377, 0.04237299155382973, 0.048012213914195655, 0.06205678270689621, 0.02722332841825998, 0.030738290495124627, 0.06544947246716075, 0.08253629130857941, 0.06264904045316583, -0.001112241436863234, 0.06753558035709736, 0.09567443661617292, 0.019589788853794414, 0.017487827676064955, 0.055436038356466245, 0.08113700798459846, 0.12069855968454125, 0.11597721600098154, 0.02839655681584141, -0.042450671972602536, -0.020202252621259218, 0.029367309548126705, 0.04906127335322257, 0.06527039691312218, 0.034313750814825864, 0.04136111683753395, 0.07418427749440712, 0.099531965315067, 0.07717513812030215, 0.06685894334575841, 0.12107145035343717, 0.0768256487649162, -0.011500959569596975, -0.045033028003552356, 0.05725029710885216, 0.04301257811847524, -0.055441534689112, -0.003027765216539939, 0.10094552394039444, 0.14832890901272766, 0.07959398568147207, 0.028374065020611863, 0.023882021563706744, 0.04502506376510203, 0.06008850778768674, 0.0656023348052836, 0.06790331851558086, 0.05017070021887288, 0.035460952741518025, 0.03921442223117759, 0.024099490989039685, 0.03128240668522458, 0.0245629321289127, -0.0495904560889453, -0.03933262565885625, 0.12994914421438275, 0.1402759689781115, -0.012870142273710286, -0.07607917948047452, -0.10112613034957327, -0.007560097168741431, 0.06866651893007791, -0.01347287848916075, -0.06214733005679232, 0.10387006898233568, 0.09887113378555785, -0.035909585620949494, -0.030191336629760923, 0.010153246448661672, 0.16185022903396568, 0.22114844249758073, 0.12508778407235216, 0.058881051553024435, 0.0975743065614357, 0.10483612141280815, 0.03884125760671558, 0.10882012044219211, 0.05706765401721584, 0.08854328968853264, 0.3929405060058441, 0.5246112671509436, 0.8833407089437023, 1.5781367526752912, 2.2339519351044332, 2.7422073940287985, 2.8753687508735433, 2.593108012045748, 1.9667519593470757, 1.2917873570633058, 0.9044012344843874, 0.9239355963326424, 0.9116525330266309, 0.6282939290094607, 0.5732191002400866, 0.6383464723094329, 0.5645486120602279, 0.7074482911708136, 0.7724435265966526, 0.6196284451647848, 0.653328880252162, 0.708656830855235, 0.6501706604607652, 0.6014657061609615, 0.8117829150177469, 1.1235055832367231, 1.2942609943105707, 1.661476571056178, 2.402897613450557, 3.0121423573707773, 3.151057718849362, 2.9802753234545043, 2.605222675465024, 2.2911438556960335, 2.1533150613481276, 1.892701868362403, 1.400091017759244, 0.9599469623270284, 0.5134193596964512, 0.14514542394682822, 0.09441613166564193, 0.042946097343875785, 0.07415135123658961, 0.174263664420406, 0.08148247841972624, -0.0725890826291684, -0.13666796593451183, -0.057614935151834516, 0.06124564048502901, 0.14282927817358315, 0.1340195800346541, 0.12836860223974986, 0.10937189920942665, 0.14016356631913496, 0.17473239132562968, 0.13871343227231653, 0.19416732262217512, 0.15090286312879936, -0.010358199792571366, -0.06952081359813872, 0.10848985762170263, 0.17616346921960013, 0.19507918113941972, 0.20352345778254066, 0.1545548587632463, 0.17005336781946645, 0.04006136689834487, -0.17595445196193457, -0.040589298215212496, 0.21171821914268799, 0.10841601686234019, -0.20693589993208722, -0.2915817905671659, 0.11053830290671283, 0.2416902133818604, 0.12740850884242952, 0.03885480706984042, 0.11340001763752008, 0.2754765816396892, 0.09900354566151075, 0.13151158068554178, 0.23661425424061505, 0.09685074447228031, -0.12587478945621847, -0.20428674602408303, 0.03700262756382799, 0.1985792337218293, 0.062437526983652014, 0.07119880989794658, -0.012641434733608743, -0.04239592762356885, 0.11090670673796073, 0.3261794935224379, 0.2720231495349483, -0.030405490440188667, 0.04369924440309479, -0.08352547162738486, -0.06633688529397212, 0.004448974973372547, -0.040279049737101974, -0.09454187184396115, -0.022643737252537068, 0.06833399402897204, 0.03665922716204027, 0.12445406668489324, 0.13445602091243744, 0.11658672670044021, -0.00469049521763912, -0.12737516552937406, 0.014235165243865254, 0.12408649044995887, 0.1680024506418345, 0.05310246542857563, -0.15050222664566118, 0.019531161770199094, -0.12767092610281205, -0.09876622880731394, 0.04966405392690004, 0.03496086309665025, 0.1757928451478326, 0.030304070184182838, 0.10158015159499918, 0.20940559380414706, 0.17461823295206344, 0.13427128793866763, -0.12462197863554235, -0.1879619816774497, 0.021000444108622594, 0.08974281849796126, 0.0690020974966942, 0.10673714860686347, 0.005365795788596408, 0.22659619311403476, 0.3634408595321281, 0.21814478805493964, 0.15352151986508383, 0.04961017102740371, -0.18287004562969705, -0.40667421477286975, -0.3640388602818237, -0.05630669730225693, 0.011321142941510775, 1.6425996602670817e-16, 0.10869087019471978, 0.16101944429121523, 0.06358814327552924, -0.005810894037489554, -0.052570350599916695, -0.2642091279488442, -0.10623491810101697, 0.10085582480782557, 0.04770608193416893, -0.14984384997996736, -0.06627079862915869, 0.2361757269976284, -0.12172703623687978, -0.1896361527549765, 1.774838033193708e-16, -0.35222527646954144, -0.06832029029861833, 0.12484929767191635, 0.20704061505398264, 0.5486045067987753, 0.3422061259569886, 0.10189673099277607, 0.3328264325249132, 0.4824349083877748, 0.45896685715720786, 0.3832759820757069, 0.25459621642954855, -0.01311989559053793, 0.07251455934169437, 0.49687106717469454, 0.26628248744817645, -0.2474915940636062, -0.35623211157401147, -0.24990025718803524, -0.02714784376652889, 0.1363975660836289, 0.054820962599049027, 0.13771223382255443, 0.166047007327129, -0.11817369219544674, -0.39810198083574383, -0.10526654382438609, 0.21859355135347092, 0.38258747458065306, 0.6905167750606441, 0.2860738492676771, -0.0071851569211251656, 0.20935317541860904, 0.2611044382316212, 0.3570557359543963, 0.358718391382502, -0.03677191132184263, -0.199484132529794, -0.16329511425421606, -0.12676540195965652, 0.14233643788989778, 0.06020567377222131, 0.09072267108608476, 0.13670695462093344, 0.20599763440199836, 0.20693505132301163, 0.007698851568682283, -0.18560464665624346, -0.3185020944607622, 0.05462634858851601, 0.3762820726167067, 0.3307228542726236, -0.08700109476041275, -0.4130984526084606, -0.09575949071322877, 0.21642626464359957, 0.20128392553243926, -0.02426036136360685, -0.16244773226761397, 0.22028233606443032, 0.5080778385129116, 0.49384609859596734, 0.41333714340309624, 0.38193096909686824, 0.2585069802345871, 0.2512566542844539, 0.12617198115501652, 0.23654489496767855, 0.042421808057813315, -0.5623427236453304, -0.4021883489105745, -0.06016024644914274, 0.4402159824221292, 0.5114524029541763, 0.31339739734822747, 0.2972466710378121, 0.16681193175481326, 0.14988556719915774, -0.0531234399556614, -0.05334782593599719, 0.47325433348230783, 0.32280215672813417, -0.06302772606452377, -0.31644939413869444, -0.58105144823879, -0.17322722794993897, 0.2014223329036116, 0.26661604146776946, -0.10154520315586761, -0.07415677242286256, 0.37233297461718495, 0.39256093882149384, 0.19708308547868256, 0.0659629193325819, -0.056770362358927115, -0.33250350368221304, 0.1526294540421979, 0.6034533681813754, 0.43278044922135794, 0.6083594729401951, 0.785354624799143, 0.5938148299225311, 0.47891428198828623, -0.19624700548413587, -0.30539976673416047, 0.4748093492170867, 0.7746724650067299, 0.15953064287858765, -0.2702673831994844, -0.1406971969892753, -0.252238132632945, 0.3545526057670537, 0.3051006593760772, -0.06125831841030068, 0.27675611935929634, 0.4219151084855917, 0.15495974507552635, 0.05185467823260385, 0.01041136437132523, -0.17767923759941814, -0.23083046964721357, 0.06319984251006557, 0.21148495586297875, 0.22291763381661264, 0.277059279773326, -0.06418077438179731, -0.24696729377475457, -0.07545347106450837, -0.32460206436564243, 0.20637720253662922, 0.7632767054733083, -0.010944646471747069, 0.0878905924883879, 0.6286267033401833, 0.17711685190880672, 0.13333883291686757, 0.8477192376005002, 0.4926152655374603, 0.044949541304097465, -0.34965219293394023, -0.7811394255593083, -0.27272814817713353, 0.22813110852851037, 0.4465197338548912, 0.4941471516091687, 0.16147668602282741, -0.10418806863642388, -0.7784401905857949, -0.6880249725191443, -0.04682008009727534, 0.28196051307713205, 0.44808078321004774, 0.14201320352909438, -0.7601106230495639, -1.1323668978915202, -0.20338804492193782, 0.828589214355894, 0.8074882179921723, 0.07256955154839627, -0.0728308657459747, 0.09745948906497609, 0.2812092104937272, 0.0, 0.0, 0.0]] caption="Water Vapor Number Density"
  out "CH 1 (WV off) counts display":dbl[][](graph)=[[15.879999999999995, 14.879999999999995, 30.879999999999995, 9.879999999999995, 66.88, 41.879999999999995, 63.879999999999995, 73.88, 59.879999999999995, 96.88, 126.88, 132.88, 165.88, 146.88, 167.88, 144.88, 157.88, 133.88, 131.88, 139.88, 162.88, 145.88, 152.88, 148.88, 156.88, 128.88, 135.88, 108.88, 110.88, 119.88, 122.88, 121.88, 84.88, 83.88, 78.88, 81.88, 74.88, 99.88, 67.88, 97.88, 57.879999999999995, 45.879999999999995, 59.879999999999995, 67.88, 60.879999999999995, 60.879999999999995, 56.879999999999995, 54.879999999999995, 15.879999999999995, 36.879999999999995, 54.879999999999995, 33.879999999999995, 51.879999999999995, 36.879999999999995, 35.879999999999995, 33.879999999999995, 36.879999999999995, 22.879999999999995, 26.879999999999995, 29.879999999999995, 16.879999999999995, 32.879999999999995, 45.879999999999995, 11.879999999999995, 18.879999999999995, 32.879999999999995, 12.879999999999995, 20.879999999999995, 21.879999999999995, 10.879999999999995, 15.879999999999995, 6.8799999999999955, 15.879999999999995, 19.879999999999995, 18.879999999999995, 21.879999999999995, 17.879999999999995, 10.879999999999995, 0.8799999999999955, 14.879999999999995, 14.879999999999995, -1.1200000000000045, -1.1200000000000045, 21.879999999999995, 2.8799999999999955, -0.12000000000000455, 20.879999999999995, -8.120000000000005, 9.879999999999995, -16.120000000000005, -9.120000000000005, -6.1200000000000045, 21.879999999999995, 21.879999999999995, 6.8799999999999955, 4.8799999999999955, 24.879999999999995, -2.1200000000000045, -25.120000000000005, 11.879999999999995, -11.120000000000005, 13.879999999999995, 5.8799999999999955, -0.12000000000000455, 11.879999999999995, 6.8799999999999955, 4.8799999999999955, -5.1200000000000045, 1.8799999999999955, 2.8799999999999955, -4.1200000000000045, -4.1200000000000045, 0.8799999999999955, -13.120000000000005, 3.8799999999999955, -11.120000000000005, 4.8799999999999955, 7.8799999999999955, 12.879999999999995, -9.120000000000005, -10.120000000000005, 8.879999999999995, 5.8799999999999955, -1.1200000000000045, -13.120000000000005, 10.879999999999995, 13.879999999999995, -0.12000000000000455, -5.1200000000000045, 0.8799999999999955, 4.8799999999999955, -12.120000000000005, 8.879999999999995, -1.1200000000000045, 3.8799999999999955, 4.8799999999999955, 13.879999999999995, 7.8799999999999955, -4.1200000000000045, 12.879999999999995, 14.879999999999995, -7.1200000000000045, -13.120000000000005, -3.1200000000000045, -2.1200000000000045, -5.1200000000000045, 6.8799999999999955, -8.120000000000005, -7.1200000000000045, -6.1200000000000045, -3.1200000000000045, 1.8799999999999955, -3.1200000000000045, -8.120000000000005, 13.879999999999995, -10.120000000000005, 16.879999999999995, -2.1200000000000045, 2.8799999999999955, -10.120000000000005, -4.1200000000000045, 8.879999999999995, 13.879999999999995, 2.8799999999999955, 6.8799999999999955, -5.1200000000000045, -2.1200000000000045, 3.8799999999999955, -5.1200000000000045, 9.879999999999995, -26.120000000000005, -1.1200000000000045, 14.879999999999995, 5.8799999999999955, 3.8799999999999955, -8.120000000000005, 0.8799999999999955, -4.1200000000000045, -10.120000000000005, -1.1200000000000045, -4.1200000000000045, -4.1200000000000045, -10.120000000000005, 3.8799999999999955, -2.1200000000000045, 13.879999999999995, -2.1200000000000045, 6.8799999999999955, -13.120000000000005, -4.1200000000000045, -4.1200000000000045, 3.8799999999999955, -2.1200000000000045, 0.8799999999999955, 6.8799999999999955, -5.1200000000000045, 17.879999999999995, -7.1200000000000045, -5.1200000000000045, -7.1200000000000045, 12.879999999999995, 0.8799999999999955, -11.120000000000005, 14.879999999999995, 6.8799999999999955, -10.120000000000005, 4.8799999999999955, 2.8799999999999955, -8.120000000000005, 16.879999999999995, -25.120000000000005, -9.120000000000005, -14.120000000000005, 7.8799999999999955, -15.120000000000005, -3.1200000000000045, 1.8799999999999955, 13.879999999999995, 8.879999999999995, 24.879999999999995, 8.879999999999995, 7.8799999999999955, 3.8799999999999955, 8.879999999999995, -9.120000000000005, 0.8799999999999955, -4.1200000000000045, 5.8799999999999955, -0.12000000000000455, 2.8799999999999955, 4.8799999999999955, -18.120000000000005, -9.120000000000005, -8.120000000000005, 7.8799999999999955, 0.8799999999999955, -2.1200000000000045, 6.8799999999999955, 16.879999999999995, 24.879999999999995, 56.879999999999995, 71.88, 126.88, 124.88, 123.88, 107.88, 61.879999999999995, 8.879999999999995, 21.879999999999995, 14.879999999999995, 13.879999999999995, 34.879999999999995, 32.879999999999995, 16.879999999999995, 15.879999999999995, 19.879999999999995, 37.879999999999995, 25.879999999999995, 16.879999999999995, 20.879999999999995, 28.879999999999995, 41.879999999999995, 15.879999999999995, 45.879999999999995, 65.88, 74.88, 115.88, 130.88, 106.88, 69.88, 81.88, 49.879999999999995, 65.88, 52.879999999999995, 35.879999999999995, 1.8799999999999955, 0.8799999999999955, 7.8799999999999955, 18.879999999999995, 3.8799999999999955, -2.1200000000000045, -6.1200000000000045, -23.120000000000005, 1.8799999999999955, 14.879999999999995, 15.879999999999995, -12.120000000000005, -8.120000000000005, 0.8799999999999955, -5.1200000000000045, -11.120000000000005, -2.1200000000000045, -7.1200000000000045, -10.120000000000005, 1.8799999999999955, -3.1200000000000045, 5.8799999999999955, -3.1200000000000045, 12.879999999999995, 1.8799999999999955, -1.1200000000000045, -12.120000000000005, -11.120000000000005, 4.8799999999999955, -3.1200000000000045, 11.879999999999995, -6.1200000000000045, 6.8799999999999955, -10.120000000000005, -12.120000000000005, -4.1200000000000045, -11.120000000000005, 2.8799999999999955, 13.879999999999995, -4.1200000000000045, -0.12000000000000455, 18.879999999999995, 5.8799999999999955, -2.1200000000000045, -10.120000000000005, -6.1200000000000045, 1.8799999999999955, -10.120000000000005, 1.8799999999999955, -4.1200000000000045, -1.1200000000000045, -11.120000000000005, 14.879999999999995, -1.1200000000000045, -2.1200000000000045, -0.12000000000000455, 14.879999999999995, -20.120000000000005, -1.1200000000000045, 1.8799999999999955, -1.1200000000000045, -17.120000000000005, -2.1200000000000045, -1.1200000000000045, -8.120000000000005, -7.1200000000000045, 5.8799999999999955, 17.879999999999995, 11.879999999999995, -3.1200000000000045, -14.120000000000005, 2.8799999999999955, 0.8799999999999955, 2.8799999999999955, 1.8799999999999955, 4.8799999999999955, 3.8799999999999955, -7.1200000000000045, -0.12000000000000455, 3.8799999999999955, 13.879999999999995, -7.1200000000000045, -1.1200000000000045, 6.8799999999999955, -22.120000000000005, -18.120000000000005, -2.1200000000000045, -4.1200000000000045, -6.1200000000000045, -8.120000000000005, -24.120000000000005, 1.8799999999999955, 4.8799999999999955, -7.1200000000000045, 21.879999999999995, -3.1200000000000045, -21.120000000000005, 2.8799999999999955, 2.8799999999999955, 7.8799999999999955, -5.1200000000000045, -2.1200000000000045, -3.1200000000000045, -2.1200000000000045, 12.879999999999995, -5.1200000000000045, 4.8799999999999955, -9.120000000000005, 12.879999999999995, -14.120000000000005, -3.1200000000000045, -0.12000000000000455, -6.1200000000000045, 1.8799999999999955, -3.1200000000000045, -5.1200000000000045, 4.8799999999999955, -8.120000000000005, -3.1200000000000045, -20.120000000000005, 13.879999999999995, -3.1200000000000045, 8.879999999999995, -0.12000000000000455, 11.879999999999995, -2.1200000000000045, 12.879999999999995, 27.879999999999995, -6.1200000000000045, -0.12000000000000455, -3.1200000000000045, -3.1200000000000045, 9.879999999999995, -14.120000000000005, 7.8799999999999955, 4.8799999999999955, -4.1200000000000045, 10.879999999999995, -11.120000000000005, -4.1200000000000045, 0.8799999999999955, 2.8799999999999955, 6.8799999999999955, -5.1200000000000045, -12.120000000000005, 17.879999999999995, -4.1200000000000045, -6.1200000000000045, 5.8799999999999955, -2.1200000000000045, 7.8799999999999955, 5.8799999999999955, -10.120000000000005, -2.1200000000000045, -12.120000000000005, -2.1200000000000045, -4.1200000000000045, 17.879999999999995, 16.879999999999995, -10.120000000000005, -14.120000000000005, 0.8799999999999955, 1.8799999999999955, -1.1200000000000045, -9.120000000000005, 3.8799999999999955, -4.1200000000000045, 4.8799999999999955, -5.1200000000000045, 10.879999999999995, -3.1200000000000045, 8.879999999999995, -8.120000000000005, 2.8799999999999955, -16.120000000000005, 12.879999999999995, -4.1200000000000045, -9.120000000000005, 18.879999999999995, -3.1200000000000045, 5.8799999999999955, -3.1200000000000045, 5.8799999999999955, 0.8799999999999955, -5.1200000000000045, 2.8799999999999955, -14.120000000000005, -1.1200000000000045, -11.120000000000005, -0.12000000000000455, 13.879999999999995, -4.1200000000000045, 6.8799999999999955, 37.879999999999995, -8.120000000000005, -0.12000000000000455, 1.8799999999999955, -17.120000000000005, 10.879999999999995, 9.879999999999995, 1.8799999999999955, 8.879999999999995, 6.8799999999999955, 5.8799999999999955, -23.120000000000005, -5.1200000000000045, 3.8799999999999955, 7.8799999999999955, -3.1200000000000045, -10.120000000000005, -2.1200000000000045, 6.8799999999999955, -14.120000000000005, 16.879999999999995, 8.879999999999995, 4.8799999999999955, 6.8799999999999955, -2.1200000000000045, -0.12000000000000455, 11.879999999999995, -0.12000000000000455, 10.879999999999995, -15.120000000000005, -7.1200000000000045, 4.8799999999999955, -17.120000000000005, 9.879999999999995, -9.120000000000005, -4.1200000000000045, 15.879999999999995, -12.120000000000005, 4.8799999999999955, -10.120000000000005, -7.1200000000000045, 10.879999999999995, -9.120000000000005, 5.8799999999999955, -14.120000000000005, -14.120000000000005, 4.8799999999999955, 3.8799999999999955, -6.1200000000000045, 6.8799999999999955, -2.1200000000000045, -3.1200000000000045, 7.8799999999999955, -4.1200000000000045, 5.8799999999999955, 7.8799999999999955, -15.120000000000005, -8.120000000000005, 11.879999999999995, 6.8799999999999955, 10.879999999999995, -1.1200000000000045, 10.879999999999995, 3.8799999999999955, 2.8799999999999955, -17.120000000000005, -16.120000000000005, -0.12000000000000455, -4.1200000000000045, -8.120000000000005, -9.120000000000005, 0.8799999999999955, -2.1200000000000045, -3.1200000000000045, -3.1200000000000045, 7.8799999999999955, -7.1200000000000045, 18.879999999999995, -0.12000000000000455, 23.879999999999995, 3.8799999999999955, -8.120000000000005, -6.1200000000000045, 1.8799999999999955, -0.12000000000000455, 4.8799999999999955, -8.120000000000005, -1.1200000000000045, -2.1200000000000045, 0.8799999999999955, 15.879999999999995, 0.0]] caption="Water Vapor Number Density"
  out "CH 3 (HSRL comb) counts display":dbl[][](graph)=[[121.76, 61.760000000000005, 55.760000000000005, 58.760000000000005, 27.760000000000005, 56.760000000000005, 69.76, 80.76, 95.76, 109.76, 129.76, 166.76, 167.76, 186.76, 206.76, 188.76, 167.76, 189.76, 204.76, 215.76, 243.76, 213.76, 221.76, 203.76, 180.76, 187.76, 183.76, 188.76, 160.76, 189.76, 168.76, 155.76, 147.76, 128.76, 143.76, 142.76, 149.76, 140.76, 110.76, 130.76, 126.76, 100.76, 108.76, 101.76, 117.76, 99.76, 113.76, 77.76, 67.76, 94.76, 98.76, 72.76, 58.760000000000005, 58.760000000000005, 89.76, 68.76, 43.760000000000005, 68.76, 58.760000000000005, 57.760000000000005, 64.76, 38.760000000000005, 62.760000000000005, 36.760000000000005, 47.760000000000005, 50.760000000000005, 39.760000000000005, 45.760000000000005, 59.760000000000005, 52.760000000000005, 47.760000000000005, 26.760000000000005, 17.760000000000005, 5.760000000000005, 30.760000000000005, 29.760000000000005, 45.760000000000005, 27.760000000000005, 31.760000000000005, 25.760000000000005, 23.760000000000005, 21.760000000000005, 28.760000000000005, 9.760000000000005, 10.760000000000005, 14.760000000000005, 27.760000000000005, 18.760000000000005, 9.760000000000005, 26.760000000000005, 27.760000000000005, 13.760000000000005, 23.760000000000005, 18.760000000000005, 18.760000000000005, 27.760000000000005, 15.760000000000005, 31.760000000000005, 30.760000000000005, 17.760000000000005, 24.760000000000005, 13.760000000000005, 2.760000000000005, 23.760000000000005, 31.760000000000005, 6.760000000000005, 23.760000000000005, 4.760000000000005, 15.760000000000005, 9.760000000000005, -6.239999999999995, 8.760000000000005, 22.760000000000005, 7.760000000000005, 23.760000000000005, 13.760000000000005, 3.760000000000005, 4.760000000000005, 1.7600000000000051, 16.760000000000005, 5.760000000000005, 1.7600000000000051, 12.760000000000005, -2.239999999999995, -0.23999999999999488, 10.760000000000005, 16.760000000000005, 12.760000000000005, 14.760000000000005, 10.760000000000005, 15.760000000000005, 19.760000000000005, 2.760000000000005, -2.239999999999995, 14.760000000000005, 10.760000000000005, 4.760000000000005, 23.760000000000005, 17.760000000000005, -2.239999999999995, 7.760000000000005, 13.760000000000005, -1.2399999999999949, 17.760000000000005, 8.760000000000005, 10.760000000000005, 7.760000000000005, 5.760000000000005, 22.760000000000005, 24.760000000000005, -0.23999999999999488, 4.760000000000005, 6.760000000000005, -1.2399999999999949, 20.760000000000005, -3.239999999999995, 10.760000000000005, 6.760000000000005, 12.760000000000005, 9.760000000000005, 5.760000000000005, 4.760000000000005, 10.760000000000005, -6.239999999999995, 2.760000000000005, 7.760000000000005, 9.760000000000005, -8.239999999999995, -6.239999999999995, 30.760000000000005, 3.760000000000005, -5.239999999999995, 7.760000000000005, 0.7600000000000051, 13.760000000000005, 16.760000000000005, 13.760000000000005, -4.239999999999995, -8.239999999999995, 2.760000000000005, -2.239999999999995, -1.2399999999999949, 12.760000000000005, -4.239999999999995, 1.7600000000000051, 4.760000000000005, 23.760000000000005, 0.7600000000000051, 7.760000000000005, 16.760000000000005, 0.7600000000000051, -11.239999999999995, -6.239999999999995, 13.760000000000005, -8.239999999999995, -14.239999999999995, -1.2399999999999949, 13.760000000000005, 14.760000000000005, -2.239999999999995, 2.760000000000005, -6.239999999999995, 0.7600000000000051, -5.239999999999995, -1.2399999999999949, 4.760000000000005, -2.239999999999995, 1.7600000000000051, 9.760000000000005, 0.7600000000000051, 5.760000000000005, -5.239999999999995, -2.239999999999995, -5.239999999999995, 19.760000000000005, -6.239999999999995, -0.23999999999999488, -17.239999999999995, -2.239999999999995, 15.760000000000005, 0.7600000000000051, -6.239999999999995, -1.2399999999999949, 17.760000000000005, -1.2399999999999949, -2.239999999999995, 2.760000000000005, -1.2399999999999949, 23.760000000000005, 17.760000000000005, 14.760000000000005, -0.23999999999999488, 10.760000000000005, 12.760000000000005, -1.2399999999999949, 2.760000000000005, -12.239999999999995, 9.760000000000005, 21.760000000000005, 9.760000000000005, 60.760000000000005, 80.76, 116.76, 135.76, 123.76, 87.76, 61.760000000000005, 38.760000000000005, 16.760000000000005, 34.760000000000005, 24.760000000000005, 28.760000000000005, 12.760000000000005, 31.760000000000005, 15.760000000000005, 34.760000000000005, 20.760000000000005, 27.760000000000005, 29.760000000000005, 33.760000000000005, 12.760000000000005, 29.760000000000005, 41.760000000000005, 44.760000000000005, 63.760000000000005, 66.76, 92.76, 114.76, 103.76, 108.76, 65.76, 54.760000000000005, 74.76, 49.760000000000005, 41.760000000000005, 25.760000000000005, 0.7600000000000051, 9.760000000000005, 5.760000000000005, -1.2399999999999949, 9.760000000000005, 12.760000000000005, -9.239999999999995, -6.239999999999995, -7.239999999999995, 4.760000000000005, -4.239999999999995, 8.760000000000005, -3.239999999999995, 1.7600000000000051, 10.760000000000005, 5.760000000000005, 3.760000000000005, 7.760000000000005, 6.760000000000005, -2.239999999999995, -4.239999999999995, -10.239999999999995, 7.760000000000005, 12.760000000000005, 11.760000000000005, -2.239999999999995, 16.760000000000005, -4.239999999999995, 2.760000000000005, 3.760000000000005, 19.760000000000005, 9.760000000000005, -5.239999999999995, -16.239999999999995, -12.239999999999995, 25.760000000000005, -0.23999999999999488, 3.760000000000005, -1.2399999999999949, 17.760000000000005, 4.760000000000005, -13.239999999999995, 2.760000000000005, 4.760000000000005, 1.7600000000000051, -16.239999999999995, -1.2399999999999949, 6.760000000000005, 11.760000000000005, 5.760000000000005, 6.760000000000005, 2.760000000000005, -2.239999999999995, 14.760000000000005, 26.760000000000005, -6.239999999999995, -13.239999999999995, 3.760000000000005, -7.239999999999995, 7.760000000000005, -9.239999999999995, 15.760000000000005, -13.239999999999995, 6.760000000000005, 3.760000000000005, 6.760000000000005, -1.2399999999999949, 14.760000000000005, 12.760000000000005, -12.239999999999995, 2.760000000000005, -4.239999999999995, 3.760000000000005, 3.760000000000005, -7.239999999999995, 6.760000000000005, 0.7600000000000051, 0.7600000000000051, -3.239999999999995, -2.239999999999995, 3.760000000000005, -3.239999999999995, -16.239999999999995, 17.760000000000005, 12.760000000000005, 8.760000000000005, -3.239999999999995, 3.760000000000005, -6.239999999999995, 5.760000000000005, 8.760000000000005, 10.760000000000005, -5.239999999999995, -1.2399999999999949, 18.760000000000005, 6.760000000000005, -1.2399999999999949, 9.760000000000005, -7.239999999999995, -15.239999999999995, -6.239999999999995, -1.2399999999999949, 5.760000000000005, -8.239999999999995, -5.239999999999995, -0.23999999999999488, 9.760000000000005, -19.239999999999995, 0.7600000000000051, -15.239999999999995, -3.239999999999995, 12.760000000000005, 10.760000000000005, -11.239999999999995, -10.239999999999995, 2.760000000000005, 10.760000000000005, -21.239999999999995, 7.760000000000005, -16.239999999999995, -15.239999999999995, 7.760000000000005, -6.239999999999995, 4.760000000000005, 8.760000000000005, 3.760000000000005, -2.239999999999995, 15.760000000000005, 8.760000000000005, 14.760000000000005, 14.760000000000005, 9.760000000000005, -5.239999999999995, 9.760000000000005, 16.760000000000005, 1.7600000000000051, -6.239999999999995, -9.239999999999995, -9.239999999999995, 10.760000000000005, -4.239999999999995, -4.239999999999995, 9.760000000000005, -0.23999999999999488, -0.23999999999999488, -11.239999999999995, -0.23999999999999488, -3.239999999999995, 21.760000000000005, 8.760000000000005, 0.7600000000000051, 12.760000000000005, -8.239999999999995, 6.760000000000005, -5.239999999999995, 11.760000000000005, -2.239999999999995, -0.23999999999999488, -6.239999999999995, -0.23999999999999488, 13.760000000000005, -2.239999999999995, 4.760000000000005, 2.760000000000005, 18.760000000000005, -2.239999999999995, 11.760000000000005, -9.239999999999995, -7.239999999999995, 15.760000000000005, 12.760000000000005, -5.239999999999995, -11.239999999999995, -1.2399999999999949, 6.760000000000005, 7.760000000000005, -0.23999999999999488, 0.7600000000000051, -4.239999999999995, 16.760000000000005, 2.760000000000005, 3.760000000000005, 7.760000000000005, 16.760000000000005, -3.239999999999995, 22.760000000000005, -12.239999999999995, 8.760000000000005, -17.239999999999995, -10.239999999999995, -1.2399999999999949, 6.760000000000005, 12.760000000000005, 10.760000000000005, 2.760000000000005, 3.760000000000005, 6.760000000000005, -2.239999999999995, 4.760000000000005, -1.2399999999999949, 11.760000000000005, -6.239999999999995, 0.7600000000000051, -12.239999999999995, -14.239999999999995, -3.239999999999995, 7.760000000000005, 0.7600000000000051, -9.239999999999995, 10.760000000000005, 12.760000000000005, 14.760000000000005, 7.760000000000005, -0.23999999999999488, -10.239999999999995, -9.239999999999995, 11.760000000000005, 5.760000000000005, 13.760000000000005, 16.760000000000005, -1.2399999999999949, 11.760000000000005, 8.760000000000005, -10.239999999999995, -0.23999999999999488, 5.760000000000005, 15.760000000000005, -0.23999999999999488, 1.7600000000000051, -14.239999999999995, -9.239999999999995, 19.760000000000005, 5.760000000000005, 0.7600000000000051, 6.760000000000005, 12.760000000000005, 1.7600000000000051, -1.2399999999999949, -2.239999999999995, 2.760000000000005, -8.239999999999995, -1.2399999999999949, -4.239999999999995, 14.760000000000005, -3.239999999999995, 2.760000000000005, -10.239999999999995, -0.23999999999999488, -13.239999999999995, 21.760000000000005, -8.239999999999995, -11.239999999999995, 10.760000000000005, 9.760000000000005, 0.7600000000000051, 12.760000000000005, 20.760000000000005, -3.239999999999995, 0.7600000000000051, -9.239999999999995, -13.239999999999995, 8.760000000000005, 4.760000000000005, 8.760000000000005, 0.7600000000000051, 7.760000000000005, -7.239999999999995, -6.239999999999995, -14.239999999999995, -7.239999999999995, 12.760000000000005, 7.760000000000005, 9.760000000000005, -18.239999999999995, -2.239999999999995, -1.2399999999999949, 14.760000000000005, 7.760000000000005, -7.239999999999995, -3.239999999999995, 3.760000000000005, -0.23999999999999488, 1.7600000000000051, 0.0]] caption="Water Vapor Number Density"
  out "CH3 (HSRL combined) smooth":dbl[](array[numeric])=[77.4, 48.0, 46.9, 47.2, 50.6, 63.300000000000004, 72.5, 85.19999999999999, 101.69999999999999, 124.7, 151.8, 165.7, 168.5, 176.2, 179.6, 170.7, 177.5, 196.7, 206.8, 221.6, 223.6, 211.2, 207.10000000000002, 196.7, 192.8, 193.9, 187.2, 179.6, 172.89999999999998, 163.5, 159.0, 154.3, 142.60000000000002, 145.8, 147.8, 136.4, 132.7, 128.8, 120.5, 123.6, 119.9, 109.2, 108.5, 105.1, 103.5, 104.19999999999999, 93.5, 81.2, 80.8, 86.5, 81.0, 69.5, 67.30000000000001, 73.0, 76.5, 69.1, 62.3, 63.0, 59.6, 56.099999999999994, 52.3, 52.400000000000006, 50.8, 46.8, 46.0, 40.2, 39.8, 45.3, 45.5, 42.3, 38.900000000000006, 29.6, 27.300000000000004, 29.6, 25.200000000000003, 28.400000000000002, 28.200000000000003, 25.0, 26.200000000000003, 23.500000000000004, 20.700000000000003, 24.400000000000002, 26.5, 18.900000000000002, 16.200000000000003, 18.000000000000004, 20.400000000000006, 20.300000000000004, 19.200000000000003, 21.200000000000003, 17.6, 15.300000000000002, 18.000000000000004, 16.900000000000006, 18.800000000000004, 15.500000000000002, 14.500000000000002, 19.6, 15.900000000000002, 16.200000000000003, 17.1, 8.500000000000004, 13.700000000000003, 24.300000000000004, 18.800000000000004, 17.5, 15.300000000000002, 10.700000000000003, 8.400000000000002, 3.400000000000003, 6.100000000000003, 13.500000000000004, 16.400000000000002, 17.800000000000004, 17.300000000000004, 8.500000000000004, 5.200000000000003, 6.300000000000003, 9.200000000000003, 10.900000000000002, 6.700000000000003, 7.100000000000003, 7.700000000000003, 8.300000000000004, 11.400000000000002, 10.600000000000001, 9.200000000000003, 9.500000000000004, 8.800000000000004, 9.100000000000003, 10.000000000000004, 11.200000000000003, 6.600000000000003, 6.600000000000003, 10.200000000000003, 6.100000000000002, 8.600000000000003, 13.100000000000001, 4.700000000000003, 0.7000000000000026, 5.600000000000003, 7.3000000000000025, 11.500000000000004, 14.800000000000002, 12.000000000000004, 6.3000000000000025, 4.0000000000000036, 8.400000000000002, 14.700000000000003, 12.600000000000003, 6.400000000000003, 6.900000000000003, 4.600000000000003, 5.900000000000003, 10.000000000000004, 6.8000000000000025, 8.000000000000004, 10.100000000000001, 6.700000000000003, 4.200000000000003, 4.700000000000003, 6.000000000000003, 2.6000000000000028, 2.900000000000003, 6.100000000000003, 7.600000000000003, 5.700000000000003, -0.09999999999999715, 6.0000000000000036, 8.400000000000004, 1.7000000000000028, 1.5000000000000029, 4.700000000000003, 6.8000000000000025, 10.000000000000004, 9.500000000000004, 2.300000000000003, -3.3999999999999972, -1.5999999999999972, 2.3000000000000025, 3.800000000000003, 5.0000000000000036, 2.6000000000000028, 3.1000000000000028, 5.5000000000000036, 7.300000000000003, 5.600000000000003, 4.8000000000000025, 8.600000000000001, 5.400000000000002, -0.7999999999999972, -3.099999999999997, 3.9000000000000026, 2.9000000000000026, -3.699999999999997, -0.19999999999999707, 6.600000000000003, 9.600000000000001, 5.100000000000002, 1.800000000000003, 1.5000000000000029, 2.800000000000003, 3.700000000000003, 4.000000000000003, 4.100000000000003, 3.0000000000000027, 2.1000000000000028, 2.300000000000003, 1.4000000000000028, 1.8000000000000027, 1.4000000000000028, -2.799999999999997, -2.199999999999997, 7.200000000000003, 7.700000000000003, -0.6999999999999972, -4.099999999999997, -5.399999999999997, -0.39999999999999725, 3.6000000000000028, -0.6999999999999971, -3.199999999999997, 5.300000000000003, 5.0000000000000036, -1.7999999999999972, -1.4999999999999971, 0.5000000000000028, 7.900000000000002, 10.700000000000003, 6.0000000000000036, 2.800000000000003, 4.600000000000003, 4.900000000000003, 1.800000000000003, 5.000000000000003, 2.6000000000000028, 4.0000000000000036, 17.6, 23.300000000000004, 38.9, 68.9, 96.7, 117.7, 122.4, 109.5, 82.4, 53.7, 37.3, 37.8, 37.0, 25.300000000000004, 22.900000000000002, 25.3, 22.200000000000003, 27.6, 29.9, 23.800000000000004, 24.900000000000002, 26.8, 24.400000000000002, 22.400000000000006, 30.0, 41.2, 47.099999999999994, 60.0, 86.1, 107.1, 111.2, 104.4, 90.6, 79.1, 73.8, 64.4, 47.3, 32.2, 17.1, 4.8000000000000025, 3.1000000000000028, 1.4000000000000028, 2.400000000000003, 5.600000000000003, 2.6000000000000028, -2.299999999999997, -4.299999999999997, -1.7999999999999972, 1.9000000000000028, 4.400000000000003, 4.100000000000003, 3.9000000000000026, 3.3000000000000025, 4.200000000000003, 5.200000000000003, 4.100000000000003, 5.700000000000003, 4.400000000000003, -0.29999999999999716, -1.9999999999999973, 3.1000000000000028, 5.000000000000003, 5.500000000000003, 5.700000000000003, 4.3000000000000025, 4.700000000000003, 1.100000000000003, -4.799999999999997, -1.099999999999997, 5.700000000000003, 2.900000000000003, -5.499999999999997, -7.6999999999999975, 2.900000000000003, 6.3000000000000025, 3.300000000000003, 1.000000000000003, 2.9000000000000026, 7.000000000000003, 2.500000000000003, 3.300000000000003, 5.900000000000003, 2.400000000000003, -3.099999999999997, -4.9999999999999964, 0.900000000000003, 4.8000000000000025, 1.5000000000000029, 1.700000000000003, -0.29999999999999716, -0.9999999999999973, 2.6000000000000028, 7.600000000000003, 6.3000000000000025, -0.6999999999999972, 1.0000000000000029, -1.899999999999997, -1.4999999999999971, 0.10000000000000275, -0.8999999999999972, -2.099999999999997, -0.49999999999999734, 1.5000000000000027, 0.8000000000000029, 2.700000000000003, 2.900000000000003, 2.5000000000000027, -0.0999999999999972, -2.6999999999999975, 0.30000000000000293, 2.600000000000003, 3.500000000000003, 1.1000000000000028, -3.0999999999999974, 0.4000000000000029, -2.599999999999997, -1.9999999999999973, 1.0000000000000027, 0.700000000000003, 3.5000000000000027, 0.6000000000000028, 2.0000000000000027, 4.100000000000003, 3.400000000000003, 2.6000000000000028, -2.3999999999999972, -3.599999999999997, 0.4000000000000028, 1.7000000000000028, 1.300000000000003, 2.0000000000000027, 0.10000000000000286, 4.200000000000003, 6.700000000000003, 4.0000000000000036, 2.800000000000003, 0.9000000000000028, -3.299999999999997, -7.299999999999997, -6.499999999999997, -0.9999999999999971, 0.20000000000000284, 2.886579864025407e-15, 1.900000000000003, 2.800000000000003, 1.1000000000000028, -0.0999999999999972, -0.899999999999997, -4.4999999999999964, -1.799999999999997, 1.7000000000000028, 0.8000000000000028, -2.4999999999999973, -1.0999999999999972, 3.900000000000003, -1.999999999999997, -3.099999999999997, 2.886579864025407e-15, -5.6999999999999975, -1.099999999999997, 2.0000000000000027, 3.3000000000000034, 8.700000000000003, 5.400000000000002, 1.6000000000000028, 5.200000000000003, 7.5000000000000036, 7.100000000000003, 5.900000000000002, 3.900000000000003, -0.1999999999999973, 1.1000000000000028, 7.5000000000000036, 4.000000000000003, -3.699999999999997, -5.299999999999997, -3.699999999999997, -0.399999999999997, 2.0000000000000027, 0.8000000000000028, 2.0000000000000027, 2.400000000000003, -1.699999999999997, -5.6999999999999975, -1.4999999999999971, 3.100000000000003, 5.400000000000002, 9.700000000000003, 4.0000000000000036, -0.0999999999999972, 2.900000000000003, 3.6000000000000028, 4.900000000000003, 4.900000000000003, -0.49999999999999734, -2.6999999999999975, -2.1999999999999975, -1.6999999999999973, 1.9000000000000028, 0.8000000000000027, 1.2000000000000028, 1.800000000000003, 2.700000000000003, 2.700000000000003, 0.10000000000000285, -2.3999999999999972, -4.099999999999998, 0.7000000000000028, 4.8000000000000025, 4.200000000000003, -1.099999999999997, -5.1999999999999975, -1.1999999999999973, 2.700000000000003, 2.5000000000000027, -0.29999999999999716, -1.9999999999999971, 2.700000000000003, 6.200000000000003, 6.000000000000003, 5.000000000000003, 4.600000000000003, 3.1000000000000028, 3.0000000000000027, 1.5000000000000029, 2.8000000000000025, 0.5000000000000027, -6.599999999999997, -4.6999999999999975, -0.6999999999999973, 5.100000000000003, 5.900000000000003, 3.6000000000000028, 3.400000000000003, 1.900000000000003, 1.7000000000000028, -0.599999999999997, -0.599999999999997, 5.3000000000000025, 3.6000000000000028, -0.6999999999999971, -3.499999999999997, -6.399999999999997, -1.8999999999999972, 2.200000000000003, 2.900000000000003, -1.0999999999999972, -0.7999999999999972, 4.000000000000003, 4.200000000000003, 2.1000000000000028, 0.7000000000000027, -0.5999999999999972, -3.4999999999999973, 1.6000000000000028, 6.3000000000000025, 4.5000000000000036, 6.3000000000000025, 8.100000000000003, 6.100000000000003, 4.900000000000003, -1.9999999999999973, -3.0999999999999974, 4.8000000000000025, 7.8000000000000025, 1.6000000000000023, -2.6999999999999975, -1.399999999999997, -2.4999999999999973, 3.5000000000000027, 3.0000000000000027, -0.5999999999999972, 2.700000000000003, 4.100000000000003, 1.5000000000000027, 0.5000000000000028, 0.10000000000000275, -1.699999999999997, -2.199999999999997, 0.6000000000000028, 2.0000000000000027, 2.1000000000000028, 2.6000000000000028, -0.5999999999999971, -2.299999999999997, -0.6999999999999973, -2.9999999999999973, 1.9000000000000026, 7.000000000000003, -0.0999999999999972, 0.8000000000000027, 5.700000000000003, 1.6000000000000028, 1.2000000000000028, 7.600000000000003, 4.400000000000003, 0.40000000000000285, -3.099999999999997, -6.899999999999997, -2.3999999999999972, 2.0000000000000027, 3.900000000000003, 4.3000000000000025, 1.4000000000000028, -0.8999999999999971, -6.699999999999997, -5.899999999999997, -0.39999999999999714, 2.400000000000003, 3.800000000000003, 1.2000000000000028, -6.399999999999997, -9.499999999999996, -1.6999999999999973, 6.900000000000003, 6.700000000000003, 0.600000000000003, -0.5999999999999971, 0.8000000000000028, 2.3000000000000025]
  out "CH3 Bin Readings":dbl[](array[numeric])=[197.0, 137.0, 131.0, 134.0, 103.0, 132.0, 145.0, 156.0, 171.0, 185.0, 205.0, 242.0, 243.0, 262.0, 282.0, 264.0, 243.0, 265.0, 280.0, 291.0, 319.0, 289.0, 297.0, 279.0, 256.0, 263.0, 259.0, 264.0, 236.0, 265.0, 244.0, 231.0, 223.0, 204.0, 219.0, 218.0, 225.0, 216.0, 186.0, 206.0, 202.0, 176.0, 184.0, 177.0, 193.0, 175.0, 189.0, 153.0, 143.0, 170.0, 174.0, 148.0, 134.0, 134.0, 165.0, 144.0, 119.0, 144.0, 134.0, 133.0, 140.0, 114.0, 138.0, 112.0, 123.0, 126.0, 115.0, 121.0, 135.0, 128.0, 123.0, 102.0, 93.0, 81.0, 106.0, 105.0, 121.0, 103.0, 107.0, 101.0, 99.0, 97.0, 104.0, 85.0, 86.0, 90.0, 103.0, 94.0, 85.0, 102.0, 103.0, 89.0, 99.0, 94.0, 94.0, 103.0, 91.0, 107.0, 106.0, 93.0, 100.0, 89.0, 78.0, 99.0, 107.0, 82.0, 99.0, 80.0, 91.0, 85.0, 69.0, 84.0, 98.0, 83.0, 99.0, 89.0, 79.0, 80.0, 77.0, 92.0, 81.0, 77.0, 88.0, 73.0, 75.0, 86.0, 92.0, 88.0, 90.0, 86.0, 91.0, 95.0, 78.0, 73.0, 90.0, 86.0, 80.0, 99.0, 93.0, 73.0, 83.0, 89.0, 74.0, 93.0, 84.0, 86.0, 83.0, 81.0, 98.0, 100.0, 75.0, 80.0, 82.0, 74.0, 96.0, 72.0, 86.0, 82.0, 88.0, 85.0, 81.0, 80.0, 86.0, 69.0, 78.0, 83.0, 85.0, 67.0, 69.0, 106.0, 79.0, 70.0, 83.0, 76.0, 89.0, 92.0, 89.0, 71.0, 67.0, 78.0, 73.0, 74.0, 88.0, 71.0, 77.0, 80.0, 99.0, 76.0, 83.0, 92.0, 76.0, 64.0, 69.0, 89.0, 67.0, 61.0, 74.0, 89.0, 90.0, 73.0, 78.0, 69.0, 76.0, 70.0, 74.0, 80.0, 73.0, 77.0, 85.0, 76.0, 81.0, 70.0, 73.0, 70.0, 95.0, 69.0, 75.0, 58.0, 73.0, 91.0, 76.0, 69.0, 74.0, 93.0, 74.0, 73.0, 78.0, 74.0, 99.0, 93.0, 90.0, 75.0, 86.0, 88.0, 74.0, 78.0, 63.0, 85.0, 97.0, 85.0, 136.0, 156.0, 192.0, 211.0, 199.0, 163.0, 137.0, 114.0, 92.0, 110.0, 100.0, 104.0, 88.0, 107.0, 91.0, 110.0, 96.0, 103.0, 105.0, 109.0, 88.0, 105.0, 117.0, 120.0, 139.0, 142.0, 168.0, 190.0, 179.0, 184.0, 141.0, 130.0, 150.0, 125.0, 117.0, 101.0, 76.0, 85.0, 81.0, 74.0, 85.0, 88.0, 66.0, 69.0, 68.0, 80.0, 71.0, 84.0, 72.0, 77.0, 86.0, 81.0, 79.0, 83.0, 82.0, 73.0, 71.0, 65.0, 83.0, 88.0, 87.0, 73.0, 92.0, 71.0, 78.0, 79.0, 95.0, 85.0, 70.0, 59.0, 63.0, 101.0, 75.0, 79.0, 74.0, 93.0, 80.0, 62.0, 78.0, 80.0, 77.0, 59.0, 74.0, 82.0, 87.0, 81.0, 82.0, 78.0, 73.0, 90.0, 102.0, 69.0, 62.0, 79.0, 68.0, 83.0, 66.0, 91.0, 62.0, 82.0, 79.0, 82.0, 74.0, 90.0, 88.0, 63.0, 78.0, 71.0, 79.0, 79.0, 68.0, 82.0, 76.0, 76.0, 72.0, 73.0, 79.0, 72.0, 59.0, 93.0, 88.0, 84.0, 72.0, 79.0, 69.0, 81.0, 84.0, 86.0, 70.0, 74.0, 94.0, 82.0, 74.0, 85.0, 68.0, 60.0, 69.0, 74.0, 81.0, 67.0, 70.0, 75.0, 85.0, 56.0, 76.0, 60.0, 72.0, 88.0, 86.0, 64.0, 65.0, 78.0, 86.0, 54.0, 83.0, 59.0, 60.0, 83.0, 69.0, 80.0, 84.0, 79.0, 73.0, 91.0, 84.0, 90.0, 90.0, 85.0, 70.0, 85.0, 92.0, 77.0, 69.0, 66.0, 66.0, 86.0, 71.0, 71.0, 85.0, 75.0, 75.0, 64.0, 75.0, 72.0, 97.0, 84.0, 76.0, 88.0, 67.0, 82.0, 70.0, 87.0, 73.0, 75.0, 69.0, 75.0, 89.0, 73.0, 80.0, 78.0, 94.0, 73.0, 87.0, 66.0, 68.0, 91.0, 88.0, 70.0, 64.0, 74.0, 82.0, 83.0, 75.0, 76.0, 71.0, 92.0, 78.0, 79.0, 83.0, 92.0, 72.0, 98.0, 63.0, 84.0, 58.0, 65.0, 74.0, 82.0, 88.0, 86.0, 78.0, 79.0, 82.0, 73.0, 80.0, 74.0, 87.0, 69.0, 76.0, 63.0, 61.0, 72.0, 83.0, 76.0, 66.0, 86.0, 88.0, 90.0, 83.0, 75.0, 65.0, 66.0, 87.0, 81.0, 89.0, 92.0, 74.0, 87.0, 84.0, 65.0, 75.0, 81.0, 91.0, 75.0, 77.0, 61.0, 66.0, 95.0, 81.0, 76.0, 82.0, 88.0, 77.0, 74.0, 73.0, 78.0, 67.0, 74.0, 71.0, 90.0, 72.0, 78.0, 65.0, 75.0, 62.0, 97.0, 67.0, 64.0, 86.0, 85.0, 76.0, 88.0, 96.0, 72.0, 76.0, 66.0, 62.0, 84.0, 80.0, 84.0, 76.0, 83.0, 68.0, 69.0, 61.0, 68.0, 88.0, 83.0, 85.0, 57.0, 73.0, 74.0, 90.0, 83.0, 68.0, 72.0, 79.0, 75.0, 77.0]
  out "CH2 (molecular) smoothed":dbl[](array[numeric])=[15.479999999999997, 3.3799999999999955, 5.3799999999999955, 11.579999999999995, 10.379999999999995, 14.779999999999996, 17.58, 15.079999999999997, 22.779999999999994, 29.879999999999995, 31.58, 34.48, 41.08, 50.879999999999995, 54.58, 52.98, 67.78, 77.07999999999998, 69.38, 71.08, 68.08, 65.47999999999999, 73.38, 71.18, 68.38, 69.47999999999999, 61.07999999999999, 55.08, 57.58, 63.07999999999999, 60.279999999999994, 55.98, 53.279999999999994, 50.08, 45.08, 41.97999999999999, 36.17999999999999, 38.779999999999994, 48.67999999999999, 44.379999999999995, 36.48, 41.779999999999994, 48.67999999999999, 48.98, 45.17999999999999, 37.08, 33.48, 34.17999999999999, 36.379999999999995, 32.78, 31.08, 19.679999999999996, 17.479999999999997, 22.379999999999995, 23.679999999999993, 25.179999999999993, 30.879999999999995, 30.879999999999995, 18.179999999999996, 15.079999999999995, 12.379999999999995, 11.079999999999995, 13.179999999999996, 21.579999999999995, 21.679999999999996, 22.279999999999994, 28.179999999999993, 20.279999999999994, 15.979999999999997, 15.879999999999995, 13.279999999999996, 20.779999999999994, 21.179999999999993, 13.579999999999995, 19.379999999999995, 14.979999999999997, 9.179999999999996, 10.179999999999996, 7.579999999999996, 8.079999999999995, 10.279999999999996, 8.879999999999995, 9.979999999999995, 8.479999999999995, 8.479999999999995, 9.479999999999995, 6.079999999999995, 7.679999999999996, 10.979999999999997, 3.4799999999999955, -5.020000000000005, 5.479999999999996, 15.179999999999996, 7.579999999999996, 4.779999999999995, 4.3799999999999955, 0.9799999999999954, 7.279999999999996, 6.579999999999996, 9.579999999999995, 6.479999999999995, -0.4200000000000046, 1.2799999999999954, 4.179999999999995, 5.079999999999996, -2.6200000000000045, 3.479999999999995, 6.579999999999995, 5.179999999999995, 10.079999999999995, 5.679999999999995, -4.1200000000000045, 0.5799999999999956, 9.579999999999995, 8.179999999999996, 9.079999999999995, 6.079999999999995, 4.3799999999999955, 7.279999999999996, 14.679999999999996, 13.779999999999996, 10.379999999999995, 8.779999999999996, 8.679999999999996, 5.179999999999995, -5.020000000000005, 2.1799999999999957, 6.479999999999995, 1.8799999999999955, 2.1799999999999953, 1.9799999999999955, 2.7799999999999954, 6.8799999999999955, 8.279999999999996, 6.8799999999999955, 7.579999999999995, 12.079999999999995, 13.479999999999995, -1.7200000000000042, -2.720000000000004, 7.179999999999995, 3.479999999999995, -0.7200000000000044, -0.7200000000000044, -0.7200000000000044, -4.020000000000005, 0.47999999999999554, 0.07999999999999563, -2.0200000000000045, 7.579999999999996, 6.479999999999996, 3.1799999999999953, 12.379999999999995, 10.479999999999995, 2.2799999999999954, 4.679999999999996, 8.379999999999995, 7.679999999999995, 10.179999999999996, 5.579999999999995, 3.7799999999999954, 4.179999999999995, 6.679999999999995, 7.479999999999995, 4.979999999999995, 7.3799999999999955, 1.7799999999999956, 7.079999999999996, 7.3799999999999955, -0.5200000000000046, -0.8200000000000046, -0.4200000000000046, 3.5799999999999956, 4.679999999999996, -2.1200000000000045, -1.9200000000000046, 4.3799999999999955, 6.679999999999995, 2.1799999999999953, -2.1200000000000045, -2.2200000000000046, -3.6200000000000045, -0.5200000000000047, 3.1799999999999953, 3.8799999999999955, 4.079999999999995, 1.1799999999999953, -4.6200000000000045, 1.1799999999999953, 2.079999999999995, -5.720000000000004, -3.5200000000000045, 4.779999999999995, 5.3799999999999955, -4.820000000000005, -4.420000000000005, 7.979999999999995, 7.779999999999996, 4.779999999999996, 4.579999999999996, 3.779999999999996, 3.779999999999996, 4.979999999999996, 4.8799999999999955, 4.179999999999995, 4.279999999999996, 3.8799999999999955, 2.979999999999995, -5.220000000000005, -2.420000000000005, 5.179999999999996, 2.6799999999999957, 1.0799999999999956, 2.1799999999999953, -4.720000000000004, -3.0200000000000045, 2.579999999999995, 4.479999999999995, 3.579999999999995, 3.7799999999999954, 5.279999999999996, 1.3799999999999955, -1.1200000000000045, 0.07999999999999541, -3.8200000000000047, -1.020000000000005, 7.479999999999995, 3.7799999999999954, -0.6200000000000044, -1.2200000000000044, 0.6799999999999955, 3.9799999999999955, 9.179999999999996, 4.8799999999999955, -7.720000000000005, -2.8200000000000047, 3.779999999999996, 0.2799999999999954, 1.3799999999999955, 2.279999999999996, 2.779999999999996, 9.279999999999996, 11.679999999999996, 3.279999999999996, 0.07999999999999546, -0.02000000000000457, 5.479999999999995, 3.9799999999999955, 1.8799999999999955, -0.5200000000000045, -3.4200000000000044, 1.3799999999999955, 2.4799999999999955, 6.179999999999996, 9.879999999999995, 6.279999999999995, 0.47999999999999543, 2.7799999999999954, 1.8799999999999955, 2.3799999999999955, -1.120000000000005, -1.720000000000005, 6.179999999999995, 1.7799999999999954, -1.5200000000000047, 2.1799999999999957, -1.8200000000000043, -6.020000000000005, 2.579999999999995, 9.279999999999994, 2.779999999999995, -5.020000000000005, 3.1799999999999953, 11.179999999999996, 7.479999999999995, 2.8799999999999955, -0.9200000000000046, 4.479999999999995, 4.8799999999999955, 1.7799999999999954, 0.17999999999999527, -1.8200000000000047, 5.079999999999996, 6.279999999999996, -1.1200000000000048, -0.3200000000000047, 8.479999999999995, 7.179999999999995, 6.979999999999996, 2.779999999999996, -4.320000000000005, -1.4200000000000046, 0.6799999999999955, 2.9799999999999955, 0.8799999999999957, -0.22000000000000441, 3.9799999999999955, 0.17999999999999527, -4.820000000000005, -4.520000000000005, -2.8200000000000043, -1.1200000000000045, 0.7799999999999956, -2.7200000000000046, -1.6200000000000045, 4.8799999999999955, 3.7799999999999954, 5.079999999999996, 3.1799999999999957, 1.2799999999999954, -1.6200000000000048, -7.520000000000005, -4.920000000000004, -2.7200000000000046, -2.3200000000000047, 3.079999999999995, 4.779999999999996, 9.879999999999995, 7.079999999999996, 1.8799999999999952, 6.3799999999999955, 0.17999999999999572, 2.6799999999999957, 3.779999999999996, -1.8200000000000045, -4.220000000000005, 1.979999999999995, 8.179999999999996, 3.8799999999999955, 1.6799999999999955, -0.32000000000000456, 0.07999999999999546, 3.4799999999999955, 0.5799999999999952, 0.07999999999999519, -0.22000000000000464, -3.2200000000000046, -1.4200000000000046, -9.120000000000005, -11.420000000000005, -3.6200000000000045, 1.9799999999999955, 3.9799999999999955, 4.8799999999999955, -0.5200000000000045, -4.420000000000004, 3.879999999999996, 5.579999999999996, 6.279999999999995, 10.579999999999995, 9.479999999999995, 7.979999999999995, 5.479999999999995, 3.5799999999999956, -0.12000000000000455, 0.1799999999999955, 5.779999999999996, 2.7799999999999954, 0.8799999999999955, -0.6200000000000045, -1.8200000000000045, -2.520000000000005, 0.4799999999999951, 4.979999999999995, -0.12000000000000455, -2.7200000000000046, -2.6200000000000045, -3.220000000000004, -3.720000000000004, -3.8200000000000047, 2.3799999999999955, 11.979999999999995, 10.479999999999995, 6.979999999999995, 5.8799999999999955, 3.9799999999999955, 6.779999999999996, 1.5799999999999956, 1.0799999999999956, 5.579999999999996, 5.579999999999996, 8.079999999999995, -0.12000000000000455, -1.2200000000000046, 2.0799999999999956, -3.3200000000000047, 3.3799999999999955, 6.3799999999999955, 4.8799999999999955, 9.679999999999996, 10.579999999999995, 11.479999999999997, 9.079999999999995, 5.779999999999996, 0.9799999999999953, 7.379999999999996, 5.779999999999996, -10.920000000000005, -7.320000000000005, 1.8799999999999955, 0.8799999999999955, -3.8200000000000047, 2.579999999999995, 12.479999999999995, 8.579999999999995, 6.579999999999996, 15.579999999999995, 9.879999999999995, 0.5799999999999954, -2.8200000000000043, -1.4200000000000044, 4.979999999999995, 8.879999999999995, 3.8799999999999955, -4.1200000000000045, -1.8200000000000047, 0.2799999999999955, -1.6200000000000043, -4.1200000000000045, 0.4799999999999953, 8.179999999999996, 14.679999999999996, 11.179999999999996, 5.179999999999995, -0.9200000000000048, -1.2200000000000046, 4.8799999999999955, 3.3799999999999955, -1.3200000000000047, -4.520000000000005, -4.220000000000004, -6.020000000000005, 2.779999999999996, 4.679999999999996, -3.6200000000000045, -1.4200000000000044, -0.02000000000000455, 1.6799999999999955, -2.020000000000005, 4.379999999999995, 12.579999999999995, -0.8200000000000047, -6.1200000000000045, 4.179999999999995, 5.779999999999995, 2.0799999999999956, -1.5200000000000045, -3.1200000000000045, 3.6799999999999953, 6.079999999999996, 1.9799999999999955, -0.5200000000000046, 1.2799999999999954, 4.679999999999995, 3.4799999999999955, 4.079999999999996, 2.8799999999999955, -4.020000000000005, -9.720000000000006, -1.020000000000005, 11.279999999999996, 7.979999999999996, 7.779999999999996, 10.079999999999995, 7.279999999999996, 7.579999999999995, 3.1799999999999953, 4.079999999999996, 1.5799999999999956, -0.9200000000000044, 5.079999999999996, 6.079999999999996, 7.979999999999995, 5.779999999999996, 4.979999999999995, 2.0799999999999956, -2.8200000000000047, -0.9200000000000046, 0.9799999999999954, 3.4799999999999955, 7.779999999999996, 4.079999999999996, -0.8200000000000045, -2.9200000000000044, -0.6200000000000043, 4.979999999999995, 1.0799999999999952, 1.6799999999999953, 1.7799999999999954, 6.479999999999995, 12.679999999999996, 5.979999999999995, 0.5799999999999954, -1.7200000000000046, 6.079999999999995, 7.479999999999995, 1.2799999999999954, 1.2799999999999954, 2.3799999999999955, 3.1799999999999953, 3.779999999999996, 3.8799999999999955, 5.079999999999995, 6.8799999999999955, 2.5799999999999956, -2.4200000000000044, 3.3799999999999955, 1.2799999999999954, -1.5200000000000045, 0.6799999999999955, -6.520000000000005, -8.720000000000004, -3.1200000000000045, -0.22000000000000453, -4.520000000000005, -0.5200000000000045, 6.579999999999996, 1.3799999999999957, 1.3799999999999957, -0.7200000000000042, -1.5200000000000045, 0.5799999999999954, -1.0200000000000045, -0.8200000000000045, -0.5200000000000045, 2.1799999999999953, 2.8799999999999955, 1.2799999999999954, -2.3200000000000047, -5.420000000000004, 2.979999999999995, 12.779999999999994, 8.779999999999996, -2.120000000000004, -1.120000000000004, 9.479999999999995, 8.679999999999996, 0.17999999999999527, -3.9200000000000044, -4.720000000000004, -7.320000000000004, -5.520000000000005, 1.7799999999999954, -0.3200000000000047, -1.9200000000000046, 1.0799999999999956, -3.6200000000000045, -2.1200000000000045, 3.8799999999999955, 5.3799999999999955, 4.279999999999996, 4.8799999999999955, 3.8799999999999955, 3.8799999999999955, 3.7799999999999954, 1.4799999999999955, 1.0799999999999954]
  out "CH 2 Bin Readings":dbl[](array[numeric])=[163.0, 137.0, 127.0, 150.0, 154.0, 152.0, 171.0, 154.0, 150.0, 168.0, 162.0, 168.0, 175.0, 169.0, 207.0, 196.0, 188.0, 228.0, 204.0, 194.0, 214.0, 206.0, 207.0, 241.0, 201.0, 208.0, 230.0, 202.0, 196.0, 189.0, 211.0, 195.0, 200.0, 186.0, 196.0, 168.0, 180.0, 171.0, 200.0, 187.0, 201.0, 163.0, 195.0, 192.0, 188.0, 186.0, 167.0, 169.0, 202.0, 188.0, 180.0, 168.0, 148.0, 161.0, 168.0, 175.0, 156.0, 181.0, 165.0, 150.0, 150.0, 148.0, 154.0, 154.0, 172.0, 149.0, 168.0, 168.0, 143.0, 148.0, 158.0, 167.0, 192.0, 155.0, 140.0, 185.0, 150.0, 164.0, 157.0, 139.0, 146.0, 156.0, 137.0, 167.0, 159.0, 156.0, 158.0, 144.0, 149.0, 157.0, 135.0, 142.0, 147.0, 150.0, 127.0, 143.0, 152.0, 143.0, 162.0, 138.0, 161.0, 121.0, 127.0, 129.0, 155.0, 148.0, 136.0, 150.0, 139.0, 142.0, 163.0, 139.0, 130.0, 155.0, 153.0, 153.0, 147.0, 151.0, 156.0, 153.0, 177.0, 151.0, 171.0, 146.0, 148.0, 124.0, 128.0, 158.0, 134.0, 140.0, 145.0, 148.0, 137.0, 163.0, 157.0, 161.0, 150.0, 165.0, 155.0, 115.0, 174.0, 137.0, 143.0, 135.0, 155.0, 131.0, 134.0, 149.0, 136.0, 146.0, 150.0, 155.0, 150.0, 173.0, 140.0, 134.0, 145.0, 143.0, 155.0, 143.0, 149.0, 162.0, 137.0, 164.0, 129.0, 153.0, 152.0, 132.0, 161.0, 127.0, 132.0, 137.0, 138.0, 157.0, 131.0, 131.0, 165.0, 134.0, 161.0, 139.0, 143.0, 141.0, 128.0, 162.0, 137.0, 142.0, 141.0, 156.0, 122.0, 168.0, 134.0, 131.0, 136.0, 157.0, 138.0, 131.0, 149.0, 168.0, 146.0, 157.0, 134.0, 155.0, 140.0, 170.0, 135.0, 150.0, 141.0, 157.0, 140.0, 136.0, 150.0, 145.0, 127.0, 147.0, 142.0, 108.0, 131.0, 147.0, 140.0, 130.0, 147.0, 152.0, 130.0, 129.0, 159.0, 119.0, 158.0, 162.0, 135.0, 116.0, 138.0, 135.0, 160.0, 165.0, 143.0, 113.0, 157.0, 130.0, 146.0, 148.0, 140.0, 137.0, 174.0, 150.0, 146.0, 152.0, 148.0, 158.0, 128.0, 142.0, 126.0, 156.0, 141.0, 153.0, 149.0, 162.0, 148.0, 133.0, 141.0, 141.0, 165.0, 120.0, 152.0, 151.0, 138.0, 141.0, 145.0, 127.0, 127.0, 160.0, 155.0, 141.0, 134.0, 166.0, 167.0, 142.0, 137.0, 136.0, 162.0, 143.0, 137.0, 135.0, 127.0, 172.0, 146.0, 142.0, 157.0, 150.0, 158.0, 144.0, 135.0, 133.0, 135.0, 147.0, 140.0, 142.0, 154.0, 160.0, 130.0, 143.0, 135.0, 122.0, 133.0, 145.0, 127.0, 160.0, 141.0, 158.0, 152.0, 121.0, 155.0, 138.0, 134.0, 129.0, 144.0, 140.0, 150.0, 135.0, 173.0, 147.0, 153.0, 155.0, 145.0, 165.0, 143.0, 149.0, 130.0, 158.0, 147.0, 149.0, 131.0, 146.0, 129.0, 144.0, 126.0, 149.0, 122.0, 128.0, 139.0, 121.0, 126.0, 129.0, 149.0, 134.0, 144.0, 130.0, 140.0, 164.0, 139.0, 167.0, 150.0, 157.0, 139.0, 143.0, 163.0, 125.0, 129.0, 146.0, 135.0, 136.0, 138.0, 120.0, 147.0, 150.0, 150.0, 146.0, 134.0, 130.0, 152.0, 145.0, 132.0, 155.0, 167.0, 142.0, 146.0, 148.0, 142.0, 151.0, 128.0, 147.0, 139.0, 158.0, 159.0, 127.0, 152.0, 137.0, 139.0, 176.0, 124.0, 161.0, 164.0, 154.0, 151.0, 147.0, 155.0, 122.0, 160.0, 114.0, 115.0, 135.0, 149.0, 156.0, 132.0, 157.0, 172.0, 153.0, 163.0, 169.0, 136.0, 138.0, 141.0, 156.0, 154.0, 154.0, 135.0, 143.0, 143.0, 140.0, 129.0, 149.0, 135.0, 154.0, 161.0, 159.0, 161.0, 130.0, 142.0, 137.0, 142.0, 132.0, 143.0, 141.0, 126.0, 166.0, 139.0, 143.0, 151.0, 140.0, 141.0, 134.0, 149.0, 150.0, 143.0, 147.0, 155.0, 149.0, 145.0, 132.0, 146.0, 154.0, 144.0, 140.0, 143.0, 140.0, 147.0, 143.0, 171.0, 137.0, 136.0, 132.0, 139.0, 159.0, 140.0, 163.0, 153.0, 163.0, 158.0, 164.0, 148.0, 146.0, 144.0, 160.0, 145.0, 152.0, 161.0, 159.0, 143.0, 138.0, 160.0, 135.0, 148.0, 163.0, 130.0, 120.0, 130.0, 148.0, 155.0, 135.0, 141.0, 117.0, 148.0, 167.0, 148.0, 131.0, 145.0, 152.0, 142.0, 142.0, 149.0, 145.0, 156.0, 143.0, 155.0, 151.0, 138.0, 141.0, 135.0, 156.0, 132.0, 166.0, 143.0, 121.0, 141.0, 140.0, 148.0, 124.0, 149.0, 148.0, 135.0, 135.0, 110.0, 145.0, 123.0, 145.0, 149.0, 139.0, 141.0, 146.0, 143.0, 131.0, 140.0, 181.0, 165.0, 154.0, 131.0, 154.0, 150.0, 154.0, 128.0, 131.0, 144.0, 142.0, 147.0, 153.0, 129.0, 145.0, 138.0, 131.0, 133.0, 144.0, 136.0, 132.0, 161.0, 155.0, 152.0, 138.0, 140.0, 141.0, 104.0]
  in  "stop":bool
  in  "Reset Average":bool=TRUE
  in  "Save Data?":bool=TRUE
  in  "Collect Data?":bool=TRUE
  in  "ILX Address":i32=6 min=0 step=1
  in  "Lambda On DBR Current":dbl=171.13999999999868
  in  "Lambda Off DBR Current":dbl=172.9499999999997
  in  "Tab Control":T2(tab)=enum."OD"
  out "Water Vapor Number Density":cluster{"Y":dbl[], "Y":dbl[]}[](graph)
  out "Absolute Humidity":cluster{"Y":dbl[], "Y":dbl[]}[](graph)
  out "NRB plot":cluster{"Y":dbl[], "Y":dbl[]}[](graph)
  in  "background length":i32=25
  out "Correction":cluster{"Y":dbl[], "Y":dbl[]}[](graph)
  in  "dead time":dbl=3.7e-08
  out "Optical Depth":cluster{"Y":dbl[], "Y":dbl[]}[](graph) caption="XY Graph"
  out "aerosol profile":cluster{"Y":dbl[], "Y":dbl[]}[](graph)
  out "CH1 RingBuffer long":dbl[][](array[numeric])
  in  "Weather":T3(tab)=enum."Pulse Energy (Micro Joule)"
  out "Temperature (C)":dbl(graph)=16.758852258852258
  out "Pressure (mb)":dbl(graph)=847.1703296703296
  out "Relative Humdity (%)":dbl(graph)=22.21001221001221
  out "Pulse Energy (Micro Joule)":T4(graph)={"WV Online Pulse Energy"=1272.0, "WV_averaged_energy"=1341.0, "HSRL"=374.0, "WV_averaged_energy"=0.0}
  out "?":cluster{"mean":dbl, "mean":dbl}(graph)={"mean"=29995.09975498775, "mean"=21068.253412670634}
  out "Index":i32=837
  out "CH1  Bin Readings":dbl[](array[numeric])=[123.0, 122.0, 138.0, 117.0, 174.0, 149.0, 171.0, 181.0, 167.0, 204.0, 234.0, 240.0, 273.0, 254.0, 275.0, 252.0, 265.0, 241.0, 239.0, 247.0, 270.0, 253.0, 260.0, 256.0, 264.0, 236.0, 243.0, 216.0, 218.0, 227.0, 230.0, 229.0, 192.0, 191.0, 186.0, 189.0, 182.0, 207.0, 175.0, 205.0, 165.0, 153.0, 167.0, 175.0, 168.0, 168.0, 164.0, 162.0, 123.0, 144.0, 162.0, 141.0, 159.0, 144.0, 143.0, 141.0, 144.0, 130.0, 134.0, 137.0, 124.0, 140.0, 153.0, 119.0, 126.0, 140.0, 120.0, 128.0, 129.0, 118.0, 123.0, 114.0, 123.0, 127.0, 126.0, 129.0, 125.0, 118.0, 108.0, 122.0, 122.0, 106.0, 106.0, 129.0, 110.0, 107.0, 128.0, 99.0, 117.0, 91.0, 98.0, 101.0, 129.0, 129.0, 114.0, 112.0, 132.0, 105.0, 82.0, 119.0, 96.0, 121.0, 113.0, 107.0, 119.0, 114.0, 112.0, 102.0, 109.0, 110.0, 103.0, 103.0, 108.0, 94.0, 111.0, 96.0, 112.0, 115.0, 120.0, 98.0, 97.0, 116.0, 113.0, 106.0, 94.0, 118.0, 121.0, 107.0, 102.0, 108.0, 112.0, 95.0, 116.0, 106.0, 111.0, 112.0, 121.0, 115.0, 103.0, 120.0, 122.0, 100.0, 94.0, 104.0, 105.0, 102.0, 114.0, 99.0, 100.0, 101.0, 104.0, 109.0, 104.0, 99.0, 121.0, 97.0, 124.0, 105.0, 110.0, 97.0, 103.0, 116.0, 121.0, 110.0, 114.0, 102.0, 105.0, 111.0, 102.0, 117.0, 81.0, 106.0, 122.0, 113.0, 111.0, 99.0, 108.0, 103.0, 97.0, 106.0, 103.0, 103.0, 97.0, 111.0, 105.0, 121.0, 105.0, 114.0, 94.0, 103.0, 103.0, 111.0, 105.0, 108.0, 114.0, 102.0, 125.0, 100.0, 102.0, 100.0, 120.0, 108.0, 96.0, 122.0, 114.0, 97.0, 112.0, 110.0, 99.0, 124.0, 82.0, 98.0, 93.0, 115.0, 92.0, 104.0, 109.0, 121.0, 116.0, 132.0, 116.0, 115.0, 111.0, 116.0, 98.0, 108.0, 103.0, 113.0, 107.0, 110.0, 112.0, 89.0, 98.0, 99.0, 115.0, 108.0, 105.0, 114.0, 124.0, 132.0, 164.0, 179.0, 234.0, 232.0, 231.0, 215.0, 169.0, 116.0, 129.0, 122.0, 121.0, 142.0, 140.0, 124.0, 123.0, 127.0, 145.0, 133.0, 124.0, 128.0, 136.0, 149.0, 123.0, 153.0, 173.0, 182.0, 223.0, 238.0, 214.0, 177.0, 189.0, 157.0, 173.0, 160.0, 143.0, 109.0, 108.0, 115.0, 126.0, 111.0, 105.0, 101.0, 84.0, 109.0, 122.0, 123.0, 95.0, 99.0, 108.0, 102.0, 96.0, 105.0, 100.0, 97.0, 109.0, 104.0, 113.0, 104.0, 120.0, 109.0, 106.0, 95.0, 96.0, 112.0, 104.0, 119.0, 101.0, 114.0, 97.0, 95.0, 103.0, 96.0, 110.0, 121.0, 103.0, 107.0, 126.0, 113.0, 105.0, 97.0, 101.0, 109.0, 97.0, 109.0, 103.0, 106.0, 96.0, 122.0, 106.0, 105.0, 107.0, 122.0, 87.0, 106.0, 109.0, 106.0, 90.0, 105.0, 106.0, 99.0, 100.0, 113.0, 125.0, 119.0, 104.0, 93.0, 110.0, 108.0, 110.0, 109.0, 112.0, 111.0, 100.0, 107.0, 111.0, 121.0, 100.0, 106.0, 114.0, 85.0, 89.0, 105.0, 103.0, 101.0, 99.0, 83.0, 109.0, 112.0, 100.0, 129.0, 104.0, 86.0, 110.0, 110.0, 115.0, 102.0, 105.0, 104.0, 105.0, 120.0, 102.0, 112.0, 98.0, 120.0, 93.0, 104.0, 107.0, 101.0, 109.0, 104.0, 102.0, 112.0, 99.0, 104.0, 87.0, 121.0, 104.0, 116.0, 107.0, 119.0, 105.0, 120.0, 135.0, 101.0, 107.0, 104.0, 104.0, 117.0, 93.0, 115.0, 112.0, 103.0, 118.0, 96.0, 103.0, 108.0, 110.0, 114.0, 102.0, 95.0, 125.0, 103.0, 101.0, 113.0, 105.0, 115.0, 113.0, 97.0, 105.0, 95.0, 105.0, 103.0, 125.0, 124.0, 97.0, 93.0, 108.0, 109.0, 106.0, 98.0, 111.0, 103.0, 112.0, 102.0, 118.0, 104.0, 116.0, 99.0, 110.0, 91.0, 120.0, 103.0, 98.0, 126.0, 104.0, 113.0, 104.0, 113.0, 108.0, 102.0, 110.0, 93.0, 106.0, 96.0, 107.0, 121.0, 103.0, 114.0, 145.0, 99.0, 107.0, 109.0, 90.0, 118.0, 117.0, 109.0, 116.0, 114.0, 113.0, 84.0, 102.0, 111.0, 115.0, 104.0, 97.0, 105.0, 114.0, 93.0, 124.0, 116.0, 112.0, 114.0, 105.0, 107.0, 119.0, 107.0, 118.0, 92.0, 100.0, 112.0, 90.0, 117.0, 98.0, 103.0, 123.0, 95.0, 112.0, 97.0, 100.0, 118.0, 98.0, 113.0, 93.0, 93.0, 112.0, 111.0, 101.0, 114.0, 105.0, 104.0, 115.0, 103.0, 113.0, 115.0, 92.0, 99.0, 119.0, 114.0, 118.0, 106.0, 118.0, 111.0, 110.0, 90.0, 91.0, 107.0, 103.0, 99.0, 98.0, 108.0, 105.0, 104.0, 104.0, 115.0, 100.0, 126.0, 107.0, 131.0, 111.0, 99.0, 101.0, 109.0, 107.0, 112.0, 99.0, 106.0, 105.0, 108.0, 123.0]
  out "CH1 (WV off) smooth":dbl[](array[numeric])=[21.34699999999998, 23.952555555555556, 29.574777777777797, 36.53311111111114, 44.94144444444446, 54.338666666666654, 65.52199999999996, 76.96922222222216, 87.86088888888884, 99.75255555555553, 109.97477777777779, 113.83311111111112, 113.9747777777778, 113.42200000000003, 114.24144444444445, 117.40533333333335, 121.25533333333335, 126.08033333333336, 131.7831111111111, 133.92200000000003, 133.13311111111113, 132.18866666666668, 128.43033333333332, 124.40533333333332, 120.73033333333333, 116.21922222222223, 112.46088888888892, 108.27200000000002, 102.81922222222224, 98.6081111111111, 93.39422222222217, 88.1747777777777, 85.2747777777777, 81.33033333333327, 77.17477777777773, 73.16644444444441, 69.34144444444439, 66.44977777777774, 64.02755555555552, 61.13866666666663, 58.63311111111108, 55.91088888888886, 52.87755555555553, 50.84422222222221, 49.33033333333332, 47.96366666666667, 46.34422222222225, 43.69977777777781, 40.91644444444447, 39.45811111111114, 38.58866666666669, 38.130333333333354, 36.266444444444474, 34.01922222222225, 32.8497777777778, 31.147000000000027, 29.660888888888913, 28.944222222222244, 28.05255555555558, 26.48033333333335, 25.105333333333345, 24.330333333333336, 23.7081111111111, 22.60533333333332, 21.41088888888887, 20.027555555555537, 18.8831111111111, 19.13033333333332, 17.994222222222206, 15.955333333333318, 15.55533333333332, 15.027555555555546, 14.194222222222216, 13.266444444444438, 13.294222222222214, 12.91644444444444, 11.841444444444452, 10.9608888888889, 9.9608888888889, 10.6358888888889, 10.672000000000011, 9.849777777777788, 9.713666666666676, 9.310888888888897, 8.749777777777787, 9.360888888888901, 8.722000000000008, 7.613666666666673, 7.849777777777785, 7.63311111111112, 7.8386666666666756, 7.794222222222231, 7.838666666666675, 7.683111111111117, 7.119222222222227, 7.4497777777777845, 7.016444444444451, 5.741444444444445, 5.802555555555557, 5.963666666666667, 5.505333333333329, 5.58033333333333, 5.6247777777777745, 6.422000000000002, 6.1414444444444465, 5.924777777777778, 5.3275555555555565, 4.544222222222218, 4.885888888888884, 4.89144444444444, 5.08033333333333, 4.98033333333333, 4.80533333333333, 4.266444444444441, 4.474777777777775, 5.383111111111107, 4.699777777777774, 3.5969999999999964, 4.088666666666663, 4.252555555555551, 4.127555555555551, 4.649777777777773, 5.099777777777773, 4.427555555555551, 3.8386666666666622, 4.1442222222222185, 4.363666666666663, 3.5442222222222215, 2.344222222222224, 2.697, 3.2108888888888876, 3.4386666666666645, 2.924777777777776, 2.58588888888889, 2.985888888888888, 2.996999999999999, 2.833111111111112, 2.924777777777778, 3.2497777777777754, 3.1886666666666637, 2.433111111111111, 2.430333333333335, 2.688666666666668, 2.083111111111112, 2.555333333333332, 3.413666666666664, 2.860888888888889, 2.655333333333335, 1.9608888888888898, 1.3247777777777785, 2.0803333333333347, 2.2803333333333344, 1.855333333333335, 1.8747777777777799, 1.8386666666666684, 1.8053333333333348, 2.027555555555556, 2.0331111111111113, 2.008111111111112, 2.0081111111111123, 1.8553333333333346, 1.255333333333334, 1.5664444444444454, 1.5525555555555564, 1.4775555555555564, 1.5858888888888898, 1.5914444444444453, 1.8581111111111122, 1.76088888888889, 2.780333333333332, 2.5886666666666653, 1.8414444444444455, 1.78588888888889, 1.2525555555555559, 2.0108888888888896, 1.9553333333333343, 1.238666666666667, 1.88588888888889, 1.8914444444444456, 1.3581111111111115, 1.519222222222223, 1.6108888888888897, 1.305333333333334, 1.822000000000001, 1.869222222222223, 1.127555555555556, 1.9358888888888899, 2.077555555555557, 1.1942222222222227, 0.9831111111111113, 1.2303333333333337, 1.4775555555555562, 0.8220000000000005, 0.6053333333333335, 1.5608888888888899, 2.0358888888888904, 1.749777777777779, 1.2108888888888896, 0.3636666666666669, 0.6275555555555561, 0.7997777777777784, 0.4081111111111113, 1.013666666666667, 1.6386666666666674, 1.6275555555555563, 1.0831111111111116, 0.8803333333333341, 1.3386666666666678, 1.8636666666666681, 1.613666666666668, 1.1220000000000003, 0.9470000000000004, 0.8803333333333339, 0.6692222222222225, 0.7970000000000003, 1.430333333333334, 1.9164444444444455, 1.8275555555555565, 2.0386666666666677, 1.1803333333333341, 0.25533333333333363, 0.3775555555555558, 0.3553333333333336, 1.2525555555555559, 0.8442222222222229, 0.15255555555555617, 0.8608888888888895, 0.48588888888888937, 0.5525555555555561, 0.6247777777777783, 0.7414444444444448, 2.2553333333333345, 3.0969999999999986, 4.158111111111108, 5.980333333333334, 8.610888888888896, 10.205333333333343, 10.19422222222223, 10.472000000000007, 10.863666666666674, 11.710888888888888, 11.73588888888889, 10.310888888888897, 10.08311111111112, 10.766444444444453, 10.52200000000001, 9.594222222222232, 9.177555555555564, 7.863666666666675, 5.6942222222222245, 4.949777777777774, 4.433111111111108, 4.258111111111108, 5.027555555555551, 4.908111111111107, 5.644222222222226, 6.847000000000009, 7.333111111111121, 8.780333333333344, 9.730333333333343, 10.410888888888898, 11.460888888888897, 12.808111111111106, 15.721999999999984, 19.652555555555537, 24.858111111111114, 30.738666666666692, 35.90533333333336, 40.43311111111114, 43.652555555555594, 47.36922222222225, 53.471999999999994, 58.55255555555552, 61.110888888888844, 58.75811111111106, 48.45255555555555, 33.169222222222245, 18.63033333333334, 8.744222222222216, 3.1414444444444443, 0.5220000000000005, -0.19466666666666643, 0.4053333333333335, 0.46088888888888907, 0.8386666666666677, 0.5108888888888898, -0.14466666666666633, 0.31644444444444464, 0.6497777777777782, 0.8692222222222228, 0.12755555555555576, -0.07244444444444417, 0.5636666666666669, 0.33588888888888907, 0.1914444444444447, 0.8914444444444449, 0.7525555555555562, 0.41922222222222266, 0.49700000000000033, 0.19144444444444467, 0.5220000000000004, 1.0720000000000005, 0.18866666666666704, 0.0025555555555559217, 0.9081111111111114, 1.113666666666667, 0.9970000000000006, 0.313666666666667, 0.5025555555555559, 1.0192222222222225, 0.6386666666666669, 0.5608888888888892, 0.16644444444444476, -0.6224444444444439, -0.405777777777777, 0.3692222222222226, 1.0942222222222229, 1.0053333333333343, 0.08311111111111186, -0.1668888888888884, 0.0636666666666669, 0.11088888888888913, 0.26088888888888917, 0.8053333333333339, 0.7581111111111116, -0.14744444444444416, -0.08633333333333304, 0.302555555555556, 0.5581111111111117, 0.9331111111111118, 0.46922222222222276, -0.15855555555555534, -0.15299999999999975, 0.9053333333333341, 1.2747777777777787, 0.3497777777777782, 0.13588888888888928, 0.5831111111111116, 0.9053333333333342, 1.033111111111112, 0.4553333333333338, 0.3831111111111114, 0.9942222222222228, 0.6108888888888893, -0.21133333333333332, 0.4303333333333336, 1.0553333333333337, 0.6442222222222225, 0.6192222222222223, 0.21922222222222246, -0.02244444444444421, 0.1636666666666669, -0.11411111111111086, -0.43077777777777726, -0.5474444444444437, -0.0529999999999996, -0.6502222222222216, -1.1141111111111104, 0.338666666666667, 0.5636666666666671, 0.26644444444444493, 0.07477777777777828, 0.06366666666666712, 0.1525555555555559, -0.36688888888888865, -0.6196666666666663, -0.28633333333333294, 0.5747777777777783, 0.45811111111111164, -0.20299999999999974, 0.24977777777777788, 0.43866666666666687, 0.5470000000000007, 0.7747777777777782, 0.43033333333333373, 0.3858888888888893, 0.7997777777777781, 0.727555555555556, 0.5414444444444446, 0.010888888888889225, -0.2918888888888885, -0.09466666666666634, 0.09422222222222254, -0.49188888888888876, -1.1863333333333332, -0.19188888888888858, 0.42200000000000015, 0.4081111111111113, 0.3303333333333338, 0.29144444444444484, -0.05855555555555539, -0.12799999999999967, 0.6358888888888895, 0.6914444444444449, 0.5414444444444448, 0.27200000000000035, 0.47755555555555596, -0.16133333333333288, -0.7779999999999997, -0.022444444444444194, 0.4331111111111115, 1.2414444444444457, 0.22755555555555673, -0.4279999999999996, 0.9970000000000007, 1.205333333333334, 0.20533333333333356, 0.12200000000000036, 0.2608888888888892, -0.3196666666666663, -0.0029999999999995586, 0.7636666666666669, 0.6220000000000001, 0.3192222222222223, 0.23588888888888898, -0.1446666666666665, -0.15577777777777757, -0.06966666666666649, -0.43633333333333324, -0.3779999999999999, 0.7192222222222227, 0.5303333333333338, -0.6168888888888884, -0.4113333333333328, -0.07799999999999957, 0.8636666666666676, 0.894222222222223, -0.01688888888888853, -0.005777777777777349, -0.30577777777777754, -0.02799999999999986, 0.8525555555555562, 0.8136666666666672, 0.13311111111111149, -0.3752222222222218, -0.3391111111111107, -0.0696666666666664, 0.005333333333333575, -0.3363333333333331, -0.3974444444444442, 1.0136666666666676, 1.3053333333333341, 0.5858888888888891, 0.4275555555555558, 0.013666666666666924, -0.1807777777777775, -0.522444444444444, -0.12799999999999961, 0.8442222222222224, 0.899777777777778, 0.28033333333333366, 0.3497777777777781, 0.8220000000000004, 0.1164444444444448, -0.0641111111111109, 0.3220000000000003, 0.6747777777777781, 0.46922222222222265, 0.11644444444444504, 0.42755555555555613, 0.40811111111111137, -0.2141111111111107, -0.7752222222222216, -0.5974444444444438, 0.04144444444444495, 0.9053333333333338, 0.6608888888888891, 0.39977777777777795, 0.6608888888888893, 0.23866666666666717, -0.5307777777777771, -0.5113333333333329, -0.22244444444444436, -0.350222222222222, -0.47799999999999965, 0.25811111111111146, 0.48866666666666697, 0.44977777777777833, 0.716444444444445, 0.8747777777777784, 0.8108888888888895, -0.7613333333333326, -1.066888888888888, 0.1025555555555559, 0.49700000000000033, 0.8025555555555559, 0.6692222222222226, 0.2414444444444448, -0.211333333333333, -0.6168888888888887, -0.8141111111111108, -0.20855555555555533, 0.6470000000000001, 0.08033333333333378, -0.06966666666666607, 0.052555555555555925, 0.3192222222222226, 0.1775555555555559, -0.32799999999999985, -0.09188888888888869, -0.011333333333333091, -0.694666666666666, -0.6391111111111104, 0.5386666666666668, 0.48588888888888915, -0.14466666666666633, 0.23311111111111124, 0.41088888888888897, -0.29466666666666624, -0.3752222222222218, 0.06644444444444467, 0.638666666666667, 0.6470000000000005, 0.27200000000000024, 0.09977777777777777, -0.5918888888888889, -0.3029999999999996, 0.6331111111111116, 0.9220000000000006, 0.37200000000000044, -0.3057777777777775, 0.5358888888888893, 0.8525555555555561, 0.23588888888888904, -0.14466666666666644, -0.6057777777777774, -0.46133333333333304, 0.6997777777777783, 0.7358888888888893, -0.6057777777777773, -0.08633333333333293, 0.899777777777778, 0.019222222222222585, -0.050222222222221835, -0.2641111111111105, -0.8918888888888884, -1.2779999999999994, -0.9029999999999994, 0.027555555555555736, 0.15811111111111148, 0.6192222222222228, 0.4886666666666671, -0.46411111111111103, -0.5113333333333333, 0.4692222222222225, 0.399777777777778, 0.11922222222222248, 0.07755555555555575, -0.28077777777777757, -0.136333333333333, 0.08588888888888926, -0.1724444444444441, 0.5386666666666671, 1.3192222222222227, 0.45811111111111147, -0.0641111111111109, -0.15577777777777752]
  out "CH0 (WV on) smoothed":dbl[](array[numeric])=[14.809111111111108, 16.411888888888882, 20.817444444444437, 25.73411111111111, 30.35633333333334, 35.84800000000001, 42.0896666666667, 48.12300000000005, 55.00911111111117, 62.44800000000005, 69.2035555555556, 71.74244444444449, 69.63688888888893, 66.8035555555556, 64.87022222222227, 66.22577777777782, 68.31466666666671, 69.87300000000005, 71.6396666666667, 72.07855555555558, 70.82300000000004, 68.81188888888894, 65.83688888888894, 61.89244444444449, 59.61466666666672, 57.15355555555562, 53.38411111111117, 50.670222222222264, 48.2646666666667, 45.21188888888892, 42.3146666666667, 40.289666666666704, 37.71744444444447, 35.62022222222224, 33.15633333333334, 30.017444444444443, 28.564666666666664, 27.167444444444442, 26.467444444444446, 25.56744444444444, 23.817444444444433, 21.82022222222221, 20.603555555555545, 20.2591111111111, 19.322999999999993, 18.109111111111105, 17.345222222222215, 16.23966666666666, 15.170222222222218, 14.547999999999995, 13.425777777777773, 12.864666666666665, 12.192444444444446, 12.00911111111111, 11.797999999999996, 10.489666666666666, 9.892444444444445, 9.089666666666666, 8.628555555555554, 8.53411111111111, 7.342444444444447, 6.625777777777781, 6.33966666666667, 6.936888888888891, 7.023000000000002, 6.167444444444445, 5.923000000000002, 4.986888888888889, 4.667444444444443, 4.93411111111111, 4.19522222222222, 3.8924444444444424, 3.964666666666665, 4.2063333333333315, 3.5952222222222217, 3.256333333333333, 3.9841111111111096, 4.17022222222222, 3.5063333333333317, 2.5729999999999995, 2.3480000000000008, 2.723, 2.653555555555556, 1.9424444444444462, 1.895222222222223, 1.2785555555555557, 1.2785555555555552, 1.475777777777778, 1.1896666666666673, 1.8646666666666676, 1.8313333333333341, 1.8174444444444449, 1.631333333333334, 1.5674444444444446, 1.7480000000000007, 1.2730000000000008, 1.7118888888888892, 1.6313333333333335, 0.4702222222222219, 1.025777777777778, 2.0118888888888895, 1.9646666666666674, 1.7368888888888891, 1.131333333333333, 0.7507777777777778, 0.7535555555555556, 1.261888888888889, 1.5563333333333342, 1.048000000000001, 1.359111111111112, 1.356333333333334, 0.8035555555555558, 0.42577777777777776, 0.23966666666666636, 1.1230000000000004, 1.3257777777777786, 0.7063333333333335, 0.5257777777777777, 0.9341111111111116, 0.8730000000000006, 0.46744444444444444, 1.167444444444445, 0.8563333333333336, 0.7035555555555558, 1.642444444444445, 1.236888888888889, 0.2841111111111107, 0.8424444444444449, 1.1341111111111115, 1.100777777777778, 1.0257777777777781, 1.1202222222222225, 0.675777777777778, -0.3492222222222223, -0.4964444444444448, -0.3853333333333335, -0.013111111111111186, 0.23133333333333303, 1.3591111111111112, 1.4563333333333337, 0.18133333333333335, -0.22700000000000026, -0.021444444444444696, 0.3535555555555553, 0.47299999999999975, 0.13133333333333297, -0.5353333333333332, -0.2353333333333331, -0.16866666666666677, 0.18133333333333368, 0.014666666666667383, -0.7575555555555554, -0.17422222222222264, -0.4936666666666663, -0.44088888888888855, 0.8952222222222221, 0.823, 0.436888888888889, 0.6452222222222224, -0.17700000000000046, -0.2242222222222227, 0.48688888888888904, 0.3452222222222224, 0.07022222222222185, 0.053555555555555225, 0.11466666666666636, -0.18255555555555597, -0.1631111111111115, -0.313111111111111, -0.5964444444444442, -0.13533333333333356, 0.5952222222222227, 1.2591111111111117, 1.2368888888888891, 0.5674444444444443, -0.22700000000000034, -0.6047777777777779, -0.13255555555555576, -0.6936666666666665, -1.085333333333333, 0.006333333333333219, 0.21744444444444416, 0.03411111111111075, 0.006333333333332983, -0.38533333333333336, 0.3480000000000003, 1.089666666666667, 0.0007777777777776551, -0.2603333333333336, -0.08533333333333365, -0.35200000000000037, -0.4742222222222227, -0.5075555555555559, -0.604777777777778, -0.5242222222222224, 0.17022222222222233, -0.449222222222222, -1.0520000000000003, -0.17700000000000035, -0.5714444444444441, -0.6631111111111108, 0.1146666666666664, -0.29922222222222195, -0.9047777777777775, -1.1158888888888887, -0.8381111111111109, -0.6714444444444445, -0.2603333333333335, 0.14244444444444404, -0.28533333333333355, -0.727, -0.5103333333333334, -0.5992222222222221, -0.5353333333333331, -0.02144444444444458, 0.13133333333333314, -0.3686666666666664, -0.07422222222222163, 0.7313333333333334, 0.31466666666666643, 0.031333333333333095, 0.32299999999999973, 0.14799999999999952, -0.1658888888888894, 0.0674444444444441, -0.8214444444444443, -1.1408888888888884, 0.07855555555555532, 0.45355555555555493, -0.24922222222222268, -0.6520000000000001, 0.07299999999999979, 0.4479999999999997, 1.478555555555555, 2.348, 2.173000000000001, 2.0563333333333347, 1.8452222222222232, 1.717444444444445, 2.150777777777777, 2.7479999999999993, 1.9146666666666672, 1.3007777777777785, 1.3952222222222226, 1.9368888888888893, 1.7368888888888896, 1.2341111111111118, 1.8924444444444455, 1.8174444444444453, 1.7063333333333341, 1.1563333333333339, -0.03533333333333376, 0.3368888888888887, 0.8285555555555555, 1.1118888888888885, 1.2785555555555557, 1.359111111111112, 0.8674444444444449, 1.0174444444444444, 1.8618888888888891, 1.4480000000000004, 1.8813333333333344, 2.8313333333333333, 3.8174444444444444, 4.645222222222223, 5.025777777777778, 5.075777777777778, 5.070222222222223, 7.136888888888889, 9.042444444444442, 9.892444444444441, 10.125777777777776, 11.58133333333333, 12.486888888888886, 11.484111111111108, 9.939666666666666, 7.189666666666669, 3.645222222222224, 0.8229999999999997, -0.3519999999999999, -0.42699999999999966, -0.218666666666667, -0.18811111111111162, -0.42144444444444473, -1.0019999999999998, -0.4631111111111109, 0.1729999999999997, 0.028555555555555195, -0.5075555555555559, 0.023000000000000076, 0.4952222222222223, -0.10200000000000033, -0.3158888888888893, 0.11188888888888852, 0.11744444444444394, -0.01588888888888955, -0.20477777777777828, -0.7381111111111113, -0.34644444444444455, 0.11466666666666632, -0.2520000000000004, -0.685333333333333, -0.7075555555555553, -0.4436666666666671, -0.07700000000000039, 0.8841111111111115, 0.7952222222222227, -0.2408888888888891, 0.0007777777777776274, 0.2479999999999998, -0.09922222222222249, 0.09799999999999953, -0.19644444444444462, -0.3797777777777777, 0.20355555555555532, 0.12577777777777752, 0.20633333333333298, -0.12422222222222204, -0.7825555555555548, -0.4297777777777775, -0.30755555555555586, -0.5881111111111116, -0.07422222222222255, 0.11188888888888852, -0.38533333333333386, -0.37977777777777816, -0.3353333333333336, -0.20477777777777806, 0.3868888888888892, 0.7507777777777781, 0.13688888888888856, -0.08533333333333362, -0.027000000000000274, -0.001999999999999974, 0.22299999999999967, -0.2131111111111117, -0.32144444444444475, -0.19366666666666701, -0.8908888888888886, -1.1158888888888887, -0.6992222222222226, -0.6575555555555559, -0.10755555555555546, -0.1742222222222224, -0.671444444444445, -0.3575555555555559, -0.6853333333333329, -1.1519999999999988, -0.6019999999999996, -0.21588888888888919, -0.2520000000000003, 0.19522222222222219, 0.27299999999999996, -0.45477777777777806, -0.17422222222222256, 0.9980000000000001, 0.5396666666666668, -0.504777777777778, -0.36588888888888915, -0.3520000000000002, -0.7464444444444449, 0.09799999999999981, 0.5507777777777777, -0.17422222222222242, -0.5519999999999999, -0.665888888888889, -0.21588888888888913, 0.3035555555555553, -0.06033333333333374, -0.39366666666666705, -0.12422222222222248, -0.4242222222222225, -0.6325555555555559, -0.4770000000000003, -0.23533333333333353, -0.24644444444444474, -0.48255555555555585, -0.4353333333333338, -0.6547777777777781, -0.4881111111111112, -0.33811111111111136, -0.01588888888888934, 0.581333333333333, 0.35633333333333317, -0.5825555555555558, -0.8020000000000003, -0.279777777777778, -0.7075555555555553, -0.015888888888888175, 0.7785555555555557, 0.4174444444444441, 0.6785555555555557, 0.4424444444444443, -0.071444444444445, 0.2729999999999997, 0.5757777777777775, 0.3646666666666661, -0.03533333333333381, -0.4686666666666669, -0.5158888888888888, 0.05911111111111106, 0.05077777777777717, -0.4047777777777784, -0.5297777777777779, -0.9519999999999995, -0.48811111111111094, -0.23255555555555577, -0.0964444444444445, 0.4979999999999999, 0.31466666666666643, 0.03688888888888846, -0.5270000000000001, -0.34922222222222216, -0.11588888888888929, -0.16311111111111154, 0.7452222222222223, 0.8646666666666667, -0.054777777777778175, -0.5214444444444448, -0.11866666666666717, 0.6257777777777775, 0.39244444444444415, -0.527, -0.5908888888888887, -0.615888888888889, -0.5131111111111113, -0.49088888888888893, -0.5936666666666666, -0.40755555555555595, -0.802, -0.16033333333333327, -0.17699999999999988, -0.29644444444444434, 0.2646666666666663, -0.3769999999999998, -0.6881111111111113, -0.5881111111111119, -1.0214444444444444, -0.8492222222222221, -0.8131111111111109, 0.48688888888888915, 0.8868888888888886, 0.036888888888888416, 0.0646666666666662, -0.48811111111111144, -0.1492222222222226, -0.7325555555555552, -1.4908888888888878, -0.8575555555555552, -0.28533333333333355, -0.6881111111111108, -0.9186666666666659, 0.04800000000000043, 0.7591111111111113, 0.4285555555555555, -0.22422222222222238, -0.03811111111111137, 0.031333333333332936, -0.0742222222222225, -0.37977777777777777, -0.49922222222222223, -0.3658888888888888, -0.021444444444444377, -0.2908888888888887, -0.7547777777777777, -0.3908888888888893, -0.15477777777777804, -0.4214444444444444, -0.5186666666666667, -0.15200000000000036, -0.39644444444444493, 0.06466666666666634, 0.32855555555555527, 0.17299999999999974, -0.9297777777777776, -0.9103333333333332, -0.318666666666667, 0.036888888888888804, 0.4424444444444443, -0.5186666666666665, -0.4797777777777776, -0.27144444444444477, -0.38533333333333364, -0.02700000000000026, 0.4368888888888887, 0.39799999999999974, -0.19088888888888939, -0.6186666666666673, 0.053555555555555745, 0.4091111111111115, -0.42144444444444434, -0.4297777777777776, -0.6075555555555552, -0.838111111111111, -0.07144444444444498, -0.424222222222222, -0.6492222222222219, -0.27700000000000036, -0.9381111111111109, -0.6131111111111108, 0.3618888888888886, 0.506333333333333, 0.5118888888888884, -0.08811111111111175, -0.2131111111111116, 0.03133333333333299, -0.6381111111111109, -0.45199999999999974, 0.056333333333332986, 0.33688888888888846, 0.01744444444444404, -0.5770000000000003, -0.2464444444444448, 0.1841111111111107, -0.20755555555555577, -1.385333333333333, -1.2214444444444439, -0.1464444444444442, 0.2118888888888888, -0.3075555555555557, -0.7325555555555558, -0.8992222222222219, -0.7547777777777775, -0.052000000000000365, 0.42299999999999977, 0.07855555555555516, -0.16311111111111165, -0.5270000000000001, -0.8520000000000001, -0.21311111111111156, 0.42299999999999965, 0.32299999999999973, -0.08255555555555609, 0.12855555555555506, -0.19366666666666646, -0.5408888888888888, -0.2631111111111114, 0.0424444444444441, -0.20200000000000046, -0.38533333333333364, -0.3297777777777779, 0.009111111111111181, -0.01866666666666683, 0.006333333333332969, 0.08411111111111089, -0.09088888888888917, 0.34244444444444394, -0.08533333333333348, 0.017444444444444485, 0.16188888888888855, -0.04644444444444473, 0.3118888888888886, -0.027000000000000385, -0.1020000000000003, -0.2575555555555557, -0.06311111111111128, 0.18966666666666643]
  out "CH 0 Bin Readings":dbl[](array[numeric])=[117.0, 123.0, 123.0, 136.0, 156.0, 123.0, 134.0, 149.0, 155.0, 137.0, 188.0, 188.0, 209.0, 207.0, 200.0, 179.0, 160.0, 162.0, 180.0, 203.0, 192.0, 161.0, 179.0, 182.0, 172.0, 186.0, 162.0, 138.0, 178.0, 163.0, 148.0, 140.0, 147.0, 140.0, 141.0, 154.0, 134.0, 123.0, 130.0, 135.0, 123.0, 132.0, 133.0, 129.0, 126.0, 127.0, 148.0, 138.0, 87.0, 118.0, 97.0, 117.0, 112.0, 138.0, 130.0, 117.0, 102.0, 119.0, 114.0, 121.0, 100.0, 112.0, 123.0, 119.0, 118.0, 127.0, 115.0, 129.0, 103.0, 107.0, 100.0, 121.0, 111.0, 122.0, 96.0, 116.0, 103.0, 105.0, 93.0, 90.0, 127.0, 103.0, 106.0, 96.0, 104.0, 115.0, 87.0, 112.0, 107.0, 92.0, 128.0, 116.0, 124.0, 108.0, 103.0, 105.0, 123.0, 101.0, 93.0, 127.0, 122.0, 85.0, 109.0, 110.0, 104.0, 108.0, 102.0, 125.0, 97.0, 112.0, 93.0, 108.0, 99.0, 125.0, 103.0, 102.0, 106.0, 99.0, 106.0, 122.0, 99.0, 113.0, 103.0, 89.0, 127.0, 119.0, 110.0, 90.0, 105.0, 128.0, 102.0, 102.0, 121.0, 114.0, 111.0, 108.0, 124.0, 108.0, 127.0, 124.0, 116.0, 116.0, 98.0, 120.0, 115.0, 87.0, 107.0, 94.0, 109.0, 115.0, 109.0, 102.0, 103.0, 106.0, 105.0, 106.0, 126.0, 88.0, 110.0, 118.0, 108.0, 102.0, 109.0, 111.0, 101.0, 100.0, 79.0, 106.0, 107.0, 107.0, 87.0, 116.0, 107.0, 93.0, 108.0, 102.0, 101.0, 103.0, 90.0, 103.0, 109.0, 104.0, 106.0, 79.0, 99.0, 109.0, 105.0, 117.0, 111.0, 101.0, 108.0, 104.0, 119.0, 113.0, 103.0, 85.0, 124.0, 98.0, 108.0, 103.0, 94.0, 101.0, 111.0, 96.0, 106.0, 113.0, 100.0, 103.0, 110.0, 102.0, 103.0, 103.0, 99.0, 98.0, 101.0, 98.0, 105.0, 98.0, 122.0, 101.0, 110.0, 107.0, 115.0, 100.0, 105.0, 83.0, 97.0, 96.0, 93.0, 109.0, 109.0, 76.0, 128.0, 118.0, 120.0, 111.0, 89.0, 113.0, 114.0, 98.0, 93.0, 114.0, 110.0, 126.0, 137.0, 127.0, 108.0, 102.0, 116.0, 114.0, 125.0, 114.0, 106.0, 107.0, 102.0, 116.0, 123.0, 116.0, 119.0, 129.0, 111.0, 118.0, 104.0, 103.0, 125.0, 124.0, 128.0, 147.0, 117.0, 142.0, 120.0, 139.0, 123.0, 116.0, 115.0, 114.0, 104.0, 95.0, 109.0, 110.0, 96.0, 116.0, 96.0, 99.0, 105.0, 104.0, 102.0, 100.0, 81.0, 116.0, 119.0, 102.0, 98.0, 110.0, 115.0, 99.0, 106.0, 105.0, 104.0, 91.0, 111.0, 127.0, 111.0, 98.0, 120.0, 99.0, 112.0, 109.0, 121.0, 110.0, 112.0, 104.0, 100.0, 108.0, 100.0, 97.0, 87.0, 106.0, 97.0, 95.0, 101.0, 127.0, 107.0, 103.0, 100.0, 95.0, 94.0, 92.0, 111.0, 109.0, 105.0, 111.0, 118.0, 97.0, 106.0, 105.0, 121.0, 124.0, 91.0, 131.0, 109.0, 102.0, 94.0, 104.0, 93.0, 89.0, 113.0, 112.0, 81.0, 115.0, 113.0, 108.0, 106.0, 118.0, 105.0, 112.0, 129.0, 113.0, 115.0, 94.0, 101.0, 88.0, 123.0, 103.0, 128.0, 93.0, 99.0, 100.0, 102.0, 109.0, 111.0, 110.0, 107.0, 112.0, 117.0, 102.0, 121.0, 105.0, 91.0, 108.0, 96.0, 118.0, 125.0, 90.0, 102.0, 106.0, 101.0, 100.0, 116.0, 123.0, 116.0, 102.0, 104.0, 115.0, 100.0, 124.0, 110.0, 112.0, 128.0, 96.0, 98.0, 112.0, 105.0, 104.0, 125.0, 113.0, 108.0, 112.0, 105.0, 108.0, 101.0, 99.0, 120.0, 103.0, 117.0, 103.0, 83.0, 121.0, 121.0, 93.0, 137.0, 100.0, 116.0, 102.0, 119.0, 115.0, 110.0, 111.0, 94.0, 101.0, 98.0, 106.0, 100.0, 98.0, 101.0, 94.0, 107.0, 84.0, 113.0, 108.0, 105.0, 101.0, 114.0, 94.0, 107.0, 102.0, 95.0, 93.0, 116.0, 107.0, 107.0, 112.0, 109.0, 118.0, 112.0, 109.0, 93.0, 110.0, 90.0, 107.0, 94.0, 85.0, 90.0, 106.0, 84.0, 114.0, 97.0, 95.0, 83.0, 108.0, 101.0, 109.0, 109.0, 112.0, 128.0, 95.0, 103.0, 108.0, 107.0, 94.0, 110.0, 109.0, 110.0, 99.0, 98.0, 93.0, 106.0, 89.0, 113.0, 120.0, 113.0, 102.0, 119.0, 97.0, 93.0, 109.0, 97.0, 106.0, 99.0, 93.0, 96.0, 103.0, 103.0, 103.0, 118.0, 110.0, 103.0, 110.0, 115.0, 108.0, 95.0, 98.0, 112.0, 97.0, 117.0, 117.0, 113.0, 108.0, 119.0, 104.0, 101.0, 100.0, 117.0, 99.0, 107.0, 106.0, 116.0, 125.0, 106.0, 128.0, 119.0, 123.0, 101.0, 99.0, 122.0, 90.0, 94.0, 111.0, 99.0, 90.0, 109.0, 111.0, 128.0, 124.0, 106.0, 98.0, 110.0, 101.0, 100.0, 106.0, 90.0, 109.0, 137.0, 91.0, 125.0, 102.0, 107.0, 97.0, 104.0]
  out "Range Corrected Altitude Array":dbl[](array[numeric])=[1406.25, 5625.0, 12656.25, 22500.0, 35156.25, 50625.0, 68906.25, 90000.0, 113906.25, 140625.0, 170156.25, 202500.0, 237656.25, 275625.0, 316406.25, 360000.0, 406406.25, 455625.0, 507656.25, 562500.0, 620156.25, 680625.0, 743906.25, 810000.0, 878906.25, 950625.0, 1025156.25, 1102500.0, 1182656.25, 1265625.0, 1351406.25, 1440000.0, 1531406.25, 1625625.0, 1722656.25, 1822500.0, 1925156.25, 2030625.0, 2138906.25, 2250000.0, 2363906.25, 2480625.0, 2600156.25, 2722500.0, 2847656.25, 2975625.0, 3106406.25, 3240000.0, 3376406.25, 3515625.0, 3657656.25, 3802500.0, 3950156.25, 4100625.0, 4253906.25, 4410000.0, 4568906.25, 4730625.0, 4895156.25, 5062500.0, 5232656.25, 5405625.0, 5581406.25, 5760000.0, 5941406.25, 6125625.0, 6312656.25, 6502500.0, 6695156.25, 6890625.0, 7088906.25, 7290000.0, 7493906.25, 7700625.0, 7910156.25, 8122500.0, 8337656.25, 8555625.0, 8776406.25, 9000000.0, 9226406.25, 9455625.0, 9687656.25, 9922500.0, 10160156.25, 10400625.0, 10643906.25, 10890000.0, 11138906.25, 11390625.0, 11645156.25, 11902500.0, 12162656.25, 12425625.0, 12691406.25, 12960000.0, 13231406.25, 13505625.0, 13782656.25, 14062500.0, 14345156.25, 14630625.0, 14918906.25, 15210000.0, 15503906.25, 15800625.0, 16100156.25, 16402500.0, 16707656.25, 17015625.0, 17326406.25, 17640000.0, 17956406.25, 18275625.0, 18597656.25, 18922500.0, 19250156.25, 19580625.0, 19913906.25, 20250000.0, 20588906.25, 20930625.0, 21275156.25, 21622500.0, 21972656.25, 22325625.0, 22681406.25, 23040000.0, 23401406.25, 23765625.0, 24132656.25, 24502500.0, 24875156.25, 25250625.0, 25628906.25, 26010000.0, 26393906.25, 26780625.0, 27170156.25, 27562500.0, 27957656.25, 28355625.0, 28756406.25, 29160000.0, 29566406.25, 29975625.0, 30387656.25, 30802500.0, 31220156.25, 31640625.0, 32063906.25, 32490000.0, 32918906.25, 33350625.0, 33785156.25, 34222500.0, 34662656.25, 35105625.0, 35551406.25, 36000000.0, 36451406.25, 36905625.0, 37362656.25, 37822500.0, 38285156.25, 38750625.0, 39218906.25, 39690000.0, 40163906.25, 40640625.0, 41120156.25, 41602500.0, 42087656.25, 42575625.0, 43066406.25, 43560000.0, 44056406.25, 44555625.0, 45057656.25, 45562500.0, 46070156.25, 46580625.0, 47093906.25, 47610000.0, 48128906.25, 48650625.0, 49175156.25, 49702500.0, 50232656.25, 50765625.0, 51301406.25, 51840000.0, 52381406.25, 52925625.0, 53472656.25, 54022500.0, 54575156.25, 55130625.0, 55688906.25, 56250000.0, 56813906.25, 57380625.0, 57950156.25, 58522500.0, 59097656.25, 59675625.0, 60256406.25, 60840000.0, 61426406.25, 62015625.0, 62607656.25, 63202500.0, 63800156.25, 64400625.0, 65003906.25, 65610000.0, 66218906.25, 66830625.0, 67445156.25, 68062500.0, 68682656.25, 69305625.0, 69931406.25, 70560000.0, 71191406.25, 71825625.0, 72462656.25, 73102500.0, 73745156.25, 74390625.0, 75038906.25, 75690000.0, 76343906.25, 77000625.0, 77660156.25, 78322500.0, 78987656.25, 79655625.0, 80326406.25, 81000000.0, 81676406.25, 82355625.0, 83037656.25, 83722500.0, 84410156.25, 85100625.0, 85793906.25, 86490000.0, 87188906.25, 87890625.0, 88595156.25, 89302500.0, 90012656.25, 90725625.0, 91441406.25, 92160000.0, 92881406.25, 93605625.0, 94332656.25, 95062500.0, 95795156.25, 96530625.0, 97268906.25, 98010000.0, 98753906.25, 99500625.0, 100250156.25, 101002500.0, 101757656.25, 102515625.0, 103276406.25, 104040000.0, 104806406.25, 105575625.0, 106347656.25, 107122500.0, 107900156.25, 108680625.0, 109463906.25, 110250000.0, 111038906.25, 111830625.0, 112625156.25, 113422500.0, 114222656.25, 115025625.0, 115831406.25, 116640000.0, 117451406.25, 118265625.0, 119082656.25, 119902500.0, 120725156.25, 121550625.0, 122378906.25, 123210000.0, 124043906.25, 124880625.0, 125720156.25, 126562500.0, 127407656.25, 128255625.0, 129106406.25, 129960000.0, 130816406.25, 131675625.0, 132537656.25, 133402500.0, 134270156.25, 135140625.0, 136013906.25, 136890000.0, 137768906.25, 138650625.0, 139535156.25, 140422500.0, 141312656.25, 142205625.0, 143101406.25, 144000000.0, 144901406.25, 145805625.0, 146712656.25, 147622500.0, 148535156.25, 149450625.0, 150368906.25, 151290000.0, 152213906.25, 153140625.0, 154070156.25, 155002500.0, 155937656.25, 156875625.0, 157816406.25, 158760000.0, 159706406.25, 160655625.0, 161607656.25, 162562500.0, 163520156.25, 164480625.0, 165443906.25, 166410000.0, 167378906.25, 168350625.0, 169325156.25, 170302500.0, 171282656.25, 172265625.0, 173251406.25, 174240000.0, 175231406.25, 176225625.0, 177222656.25, 178222500.0, 179225156.25, 180230625.0, 181238906.25, 182250000.0, 183263906.25, 184280625.0, 185300156.25, 186322500.0, 187347656.25, 188375625.0, 189406406.25, 190440000.0, 191476406.25, 192515625.0, 193557656.25, 194602500.0, 195650156.25, 196700625.0, 197753906.25, 198810000.0, 199868906.25, 200930625.0, 201995156.25, 203062500.0, 204132656.25, 205205625.0, 206281406.25, 207360000.0, 208441406.25, 209525625.0, 210612656.25, 211702500.0, 212795156.25, 213890625.0, 214988906.25, 216090000.0, 217193906.25, 218300625.0, 219410156.25, 220522500.0, 221637656.25, 222755625.0, 223876406.25, 225000000.0, 226126406.25, 227255625.0, 228387656.25, 229522500.0, 230660156.25, 231800625.0, 232943906.25, 234090000.0, 235238906.25, 236390625.0, 237545156.25, 238702500.0, 239862656.25, 241025625.0, 242191406.25, 243360000.0, 244531406.25, 245705625.0, 246882656.25, 248062500.0, 249245156.25, 250430625.0, 251618906.25, 252810000.0, 254003906.25, 255200625.0, 256400156.25, 257602500.0, 258807656.25, 260015625.0, 261226406.25, 262440000.0, 263656406.25, 264875625.0, 266097656.25, 267322500.0, 268550156.25, 269780625.0, 271013906.25, 272250000.0, 273488906.25, 274730625.0, 275975156.25, 277222500.0, 278472656.25, 279725625.0, 280981406.25, 282240000.0, 283501406.25, 284765625.0, 286032656.25, 287302500.0, 288575156.25, 289850625.0, 291128906.25, 292410000.0, 293693906.25, 294980625.0, 296270156.25, 297562500.0, 298857656.25, 300155625.0, 301456406.25, 302760000.0, 304066406.25, 305375625.0, 306687656.25, 308002500.0, 309320156.25, 310640625.0, 311963906.25, 313290000.0, 314618906.25, 315950625.0, 317285156.25, 318622500.0, 319962656.25, 321305625.0, 322651406.25, 324000000.0, 325351406.25, 326705625.0, 328062656.25, 329422500.0, 330785156.25, 332150625.0, 333518906.25, 334890000.0, 336263906.25, 337640625.0, 339020156.25, 340402500.0, 341787656.25, 343175625.0, 344566406.25, 345960000.0, 347356406.25, 348755625.0, 350157656.25, 351562500.0, 352970156.25, 354380625.0, 355793906.25, 357210000.0, 358628906.25, 360050625.0, 361475156.25, 362902500.0, 364332656.25, 365765625.0, 367201406.25, 368640000.0, 370081406.25, 371525625.0, 372972656.25, 374422500.0, 375875156.25, 377330625.0, 378788906.25, 380250000.0, 381713906.25, 383180625.0, 384650156.25, 386122500.0, 387597656.25, 389075625.0, 390556406.25, 392040000.0, 393526406.25, 395015625.0, 396507656.25, 398002500.0, 399500156.25, 401000625.0, 402503906.25, 404010000.0, 405518906.25, 407030625.0, 408545156.25, 410062500.0, 411582656.25, 413105625.0, 414631406.25, 416160000.0, 417691406.25, 419225625.0, 420762656.25, 422302500.0, 423845156.25, 425390625.0, 426938906.25, 428490000.0, 430043906.25, 431600625.0, 433160156.25, 434722500.0, 436287656.25, 437855625.0, 439426406.25, 441000000.0]
  out "Altitude Array (km)":dbl[](array[numeric])=[0.0375, 0.075, 0.11249999999999999, 0.15, 0.1875, 0.225, 0.26249999999999996, 0.3, 0.33749999999999997, 0.37499999999999994, 0.4125, 0.44999999999999996, 0.48749999999999993, 0.525, 0.5625, 0.6, 0.6375, 0.6749999999999999, 0.7124999999999999, 0.75, 0.7875, 0.825, 0.8624999999999999, 0.8999999999999999, 0.9374999999999999, 0.975, 1.0125, 1.05, 1.0875000000000001, 1.125, 1.1625, 1.2, 1.2375, 1.2750000000000001, 1.3125, 1.35, 1.3875, 1.425, 1.4625000000000001, 1.5, 1.5375, 1.575, 1.6125, 1.6500000000000001, 1.6875, 1.725, 1.7625, 1.8, 1.8375, 1.875, 1.9125, 1.95, 1.9875, 2.025, 2.0625, 2.1, 2.1375, 2.175, 2.2125, 2.25, 2.2875, 2.325, 2.3625, 2.4, 2.4375, 2.475, 2.5125, 2.55, 2.5875, 2.625, 2.6625, 2.7, 2.7375, 2.775, 2.8125, 2.85, 2.8875, 2.925, 2.9625, 3.0, 3.0375, 3.075, 3.1125, 3.15, 3.1875, 3.225, 3.2625, 3.3, 3.3375, 3.375, 3.4125, 3.45, 3.4875, 3.525, 3.5625, 3.6, 3.6374999999999997, 3.675, 3.7125, 3.75, 3.7875, 3.8249999999999997, 3.8625, 3.9, 3.9375, 3.975, 4.012499999999999, 4.05, 4.0874999999999995, 4.124999999999999, 4.1625, 4.199999999999999, 4.2375, 4.2749999999999995, 4.312499999999999, 4.35, 4.387499999999999, 4.425, 4.4624999999999995, 4.499999999999999, 4.5375, 4.574999999999999, 4.6125, 4.6499999999999995, 4.687499999999999, 4.725, 4.762499999999999, 4.8, 4.8374999999999995, 4.874999999999999, 4.9125, 4.949999999999999, 4.9875, 5.0249999999999995, 5.062499999999999, 5.1, 5.137499999999999, 5.175, 5.2124999999999995, 5.249999999999999, 5.2875, 5.324999999999999, 5.3625, 5.3999999999999995, 5.437499999999999, 5.475, 5.512499999999999, 5.55, 5.5874999999999995, 5.624999999999999, 5.6625, 5.699999999999999, 5.7375, 5.7749999999999995, 5.812499999999999, 5.85, 5.887499999999999, 5.925, 5.9624999999999995, 5.999999999999999, 6.0375, 6.074999999999999, 6.1125, 6.1499999999999995, 6.187499999999999, 6.225, 6.262499999999999, 6.3, 6.3374999999999995, 6.374999999999999, 6.4125, 6.449999999999999, 6.4875, 6.5249999999999995, 6.562499999999999, 6.6, 6.637499999999999, 6.675, 6.7124999999999995, 6.749999999999999, 6.7875, 6.824999999999999, 6.8625, 6.8999999999999995, 6.937499999999999, 6.975, 7.012499999999999, 7.05, 7.0874999999999995, 7.124999999999999, 7.1625, 7.199999999999999, 7.237499999999999, 7.2749999999999995, 7.312499999999999, 7.35, 7.387499999999999, 7.424999999999999, 7.4624999999999995, 7.499999999999999, 7.5375, 7.574999999999999, 7.612499999999999, 7.6499999999999995, 7.687499999999999, 7.725, 7.762499999999999, 7.799999999999999, 7.8374999999999995, 7.874999999999999, 7.9125, 7.949999999999999, 7.987499999999999, 8.025, 8.0625, 8.1, 8.1375, 8.174999999999999, 8.212499999999999, 8.25, 8.2875, 8.325, 8.362499999999999, 8.399999999999999, 8.4375, 8.475, 8.5125, 8.549999999999999, 8.587499999999999, 8.625, 8.6625, 8.7, 8.737499999999999, 8.774999999999999, 8.8125, 8.85, 8.8875, 8.924999999999999, 8.962499999999999, 9.0, 9.0375, 9.075, 9.112499999999999, 9.149999999999999, 9.1875, 9.225, 9.2625, 9.299999999999999, 9.337499999999999, 9.375, 9.4125, 9.45, 9.487499999999999, 9.524999999999999, 9.5625, 9.6, 9.6375, 9.674999999999999, 9.712499999999999, 9.75, 9.7875, 9.825, 9.862499999999999, 9.899999999999999, 9.9375, 9.975, 10.0125, 10.049999999999999, 10.087499999999999, 10.125, 10.1625, 10.2, 10.237499999999999, 10.274999999999999, 10.3125, 10.35, 10.3875, 10.424999999999999, 10.462499999999999, 10.5, 10.5375, 10.575, 10.612499999999999, 10.649999999999999, 10.6875, 10.725, 10.7625, 10.799999999999999, 10.837499999999999, 10.875, 10.9125, 10.95, 10.987499999999999, 11.024999999999999, 11.0625, 11.1, 11.1375, 11.174999999999999, 11.212499999999999, 11.25, 11.2875, 11.325, 11.362499999999999, 11.399999999999999, 11.4375, 11.475, 11.5125, 11.549999999999999, 11.587499999999999, 11.625, 11.6625, 11.7, 11.737499999999999, 11.774999999999999, 11.8125, 11.85, 11.8875, 11.924999999999999, 11.962499999999999, 12.0, 12.0375, 12.075, 12.112499999999999, 12.149999999999999, 12.1875, 12.225, 12.2625, 12.299999999999999, 12.337499999999999, 12.375, 12.4125, 12.45, 12.487499999999999, 12.524999999999999, 12.5625, 12.6, 12.6375, 12.674999999999999, 12.712499999999999, 12.75, 12.7875, 12.825, 12.862499999999999, 12.899999999999999, 12.9375, 12.975, 13.0125, 13.049999999999999, 13.087499999999999, 13.125, 13.1625, 13.2, 13.237499999999999, 13.274999999999999, 13.3125, 13.35, 13.3875, 13.424999999999999, 13.462499999999999, 13.5, 13.5375, 13.575, 13.612499999999999, 13.649999999999999, 13.6875, 13.725, 13.7625, 13.799999999999999, 13.837499999999999, 13.875, 13.9125, 13.95, 13.987499999999999, 14.024999999999999, 14.0625, 14.1, 14.1375, 14.174999999999999, 14.212499999999999, 14.25, 14.2875, 14.325, 14.362499999999999, 14.399999999999999, 14.437499999999998, 14.475, 14.5125, 14.549999999999999, 14.587499999999999, 14.624999999999998, 14.6625, 14.7, 14.737499999999999, 14.774999999999999, 14.812499999999998, 14.85, 14.8875, 14.924999999999999, 14.962499999999999, 14.999999999999998, 15.0375, 15.075, 15.112499999999999, 15.149999999999999, 15.187499999999998, 15.225, 15.2625, 15.299999999999999, 15.337499999999999, 15.374999999999998, 15.4125, 15.45, 15.487499999999999, 15.524999999999999, 15.562499999999998, 15.6, 15.6375, 15.674999999999999, 15.712499999999999, 15.749999999999998, 15.7875, 15.825, 15.862499999999999, 15.899999999999999, 15.937499999999998, 15.975, 16.0125, 16.05, 16.087500000000002, 16.125, 16.1625, 16.2, 16.2375, 16.275000000000002, 16.3125, 16.35, 16.3875, 16.425, 16.462500000000002, 16.5, 16.5375, 16.575, 16.6125, 16.650000000000002, 16.6875, 16.725, 16.7625, 16.8, 16.837500000000002, 16.875, 16.9125, 16.95, 16.9875, 17.025000000000002, 17.0625, 17.1, 17.1375, 17.175, 17.212500000000002, 17.25, 17.2875, 17.325, 17.3625, 17.400000000000002, 17.4375, 17.475, 17.5125, 17.55, 17.587500000000002, 17.625, 17.6625, 17.7, 17.7375, 17.775000000000002, 17.8125, 17.85, 17.8875, 17.925, 17.962500000000002, 18.0, 18.0375, 18.075, 18.1125, 18.150000000000002, 18.1875, 18.225, 18.2625, 18.3, 18.337500000000002, 18.375, 18.4125, 18.45, 18.4875, 18.525000000000002, 18.5625, 18.6, 18.6375, 18.675, 18.712500000000002, 18.75, 18.7875, 18.825, 18.8625, 18.900000000000002, 18.9375, 18.975, 19.0125, 19.05, 19.087500000000002, 19.125, 19.1625, 19.2, 19.2375, 19.275000000000002, 19.3125, 19.35, 19.3875, 19.425, 19.462500000000002, 19.5, 19.5375, 19.575, 19.6125, 19.650000000000002, 19.6875, 19.725, 19.7625, 19.8, 19.837500000000002, 19.875, 19.9125, 19.95, 19.9875, 20.025000000000002, 20.0625, 20.1, 20.1375, 20.175, 20.212500000000002, 20.25, 20.2875, 20.325, 20.3625, 20.400000000000002, 20.4375, 20.475, 20.5125, 20.55, 20.587500000000002, 20.625, 20.6625, 20.7, 20.7375, 20.775000000000002, 20.8125, 20.85, 20.8875, 20.925, 20.962500000000002, 21.0]
  out "WV Offline Pulse Energy":dbl=1323.0
  out "WV Online Pulse Energy":dbl=1272.0
  in  "Instrument Control":T5(tab)=enum."Wavemeter"
  in  "Device In":refnum<visa-resource-name>="GPIB0::10::INSTR"
  in  "Settings":T6={"Module"=enum."WV Online TEC", "WV Online TEC"=23.122500000001626, "WV Online LD"=0.175, "WV Offline TEC"=29.534450000000476, "WV Offline LD"=0.17, "WV Etalon TEC"=27.3, "HSRL Etalon TEC"=26.0, "HSRL TEC"=18.63300000000109, "HSRL LD"=0.16} {"HSRL LD" min=0.0 max=0.18 step=0.001 format="%.3p"; "HSRL TEC" min=14.0 max=28.0 step=0.1 format="%.3g"; "WV Offline LD" min=0.0 max=0.18 step=0.001 format="%.3p"; "WV Online LD" min=0.0 max=0.18 step=0.001 format="%.3p"; "HSRL Etalon TEC" format="%.2g"; "WV Etalon TEC" format="%.2g"; "WV Offline TEC" min=16.0 max=30.0 step=0.1 format="%.3g"; "WV Online TEC" min=14.0 max=28.0 step=0.1 format="%.3g"}
  out "Readings":T7={"Pro8000"=TRUE, "WV OnLine TEC"=23.1282902, "WV Online TEC"=TRUE, "WV Online LD"=0.175111338, "WV Online LD"=TRUE, "WV Offline TEC"=29.5466862, "WV Offline TEC"=TRUE, "WV Offline LD"=0.170369148, "WV Offline LD"=TRUE, "WV EtalonTEC"=26.9207764, "WV Etalon TEC"=TRUE, "HSRL Etalon TEC"=25.9994164, "HSRL Etalon TEC"=TRUE, "HSRL TEC"=18.6453495, "HSRL TEC "=TRUE, "HSRL LD"=0.1602754, "HSRL LD"=TRUE} {"HSRL LD" format="%.3p"; "HSRL TEC" format="%.3g"; "WV Offline LD" format="%.3p"; "WV Online LD" format="%.3p"; "HSRL Etalon TEC" format="%.3g"; "WV EtalonTEC" format="%.3g"; "WV Offline TEC" format="%.3g"; "WV OnLine TEC" format="%.3g"}
  in  "Pulse B Polarity":enum32{"Low", "High"}(ring)=enum."High"
  in  "Pulse A Delay(ns)":u32=1040 min=80 max=327600
  in  "Pulse B Delay(ns)":u32=170000 min=80 max=327600 step=1
  in  "Accumulation Delay(ns)":u32=10 min=10 max=1270 step=1
  in  "Sync Pulse Polarity":enum32{"Low", "High"}(ring)=enum."High"
  in  "Pulse A Polarity":enum32{"Low", "High"}(ring)=enum."High"
  in  "Number of Bins":u32=560 min=2 max=4095 step=1
  in  "Number of Accumulates":u32=14285 min=1 max=32767 step=1
  in  "Time Resolution Per Bin(ns)":u32=250 min=5 max=1063 step=1
  out "AMCS_Profile":i32=247
  in  "WV Online Set (nm)":dbl=828.195 format="%.5f"
  out "WV Online Read (nm)":dbl=828.1949970058118 format="%.5f"
  out "WV Offline Read (nm)":dbl=828.2946901675556 format="%.5f"
  in  "WV Offline Set (nm)":dbl=828.29465 format="%.5f"
  in  "Bristol In":i32=3
  out "Bristol Out":i32
  out "Online_Diff":dbl=-2.9941882075945614e-06 format="%#_3e"
  out "Oflline_Diff":dbl=4.0167555539483146e-05 format="%#_3e"
  out "WV Online Locked":bool=TRUE
  out "WV Oflline Locked":bool=TRUE
  in  "calculate absorption cross sections":bool
  in  "Online_Tol":dbl=5e-05 format="%#_15g"
  in  "Cancel online":bool
  in  "Offline_Tol":dbl=5e-05 format="%#_15g"
  in  "Cancel Offline":bool
  in  "temp step size":dbl=0.0005 format="%#_6p"
  in  "HSRL_Tol":dbl=7.5e-05 format="%#_15g"
  out "HSRL_Diff":dbl=-7.440016486270906e-05 format="%#_3e"
  in  "Cancel HSRL":bool
  out "HSRL Locked":bool=TRUE
  out "HSRL Read (nm)":dbl=780.2460455998352 format="%.5f"
  in  "HSRL Set (nm)":dbl=780.24612 format="%#.5f"
  in  "Smoothing Range":dbl=75.0
  in  "Total DIAL Integration Time (Minutes)":i32=3
  in  "Data Reads (number of loops)":i32=1
  in  "Total Aerosol Integration Time (Minutes)":dbl=0.08
  in  "Scalar Wait Time":u32
  out "Smoothed Bins":dbl=2.0
  out "gate size":dbl=37.5
  in  "Receiver Scale Factor":dbl=0.75
  in  "NewportIn":string
  in  "logging":bool
  out "Newport Device Key":string
  in  "SampleSize":i32=2
  out "NewportRef":refnum<k24>
  in  "Switch Comm Port":refnum<visa-resource-name>="COM3"
  out "FF_On_Ref":refnum<file>
  out "FF_On_Ptr":i64=5986016 format="%.2p"
  out "FF_Off_Ref":refnum<file>
  out "FF_Off_Ptr":i64=5986016 format="%.2p"
  out "NF_On_Ref":refnum<file>
  out "NF_On_Ptr":i64=5986016 format="%.2p"
  out "NF_Off_Ref":refnum<file>
  out "NF_Off_Ptr":i64=5986016 format="%.2p"
  out "DataOpen":bool=TRUE
  out "File Path_Far Field (out)":string="C:\\SharedTeleWVData\\171024FF\\15"
  out "File Path_Near Field (out)":string="C:\\SharedTeleWVData\\171024NF\\15"
  in  "Data File DIR (in)":string="C:\\SharedTeleWVData\\"
  out "TRHP":T8={"Temp C"=16.758852258852258, "RelH %"=22.21001221001221, "Press hPa"=847.1703296703296, "AbH g/m^3"=3.0677655677655675}
  in  "WS visa":refnum<visa-resource-name>="COM2"
  in  "WS_On/Off":bool=TRUE
  out "NetCDFFilePath":string="C:\\SharedTeleWVData\\171024NF\\15"
  in  "OfflineIndex":i32=1
  in  "WVDialNumber":dbl=2.0
  out "NetCDFFileName":string="TestingNCARWVDIAL002_20171024_150001.cdf"
  out "NetCDFEntry":i32=1323
  out "H2ODIAL":T9(array[cluster])=[{"DIALCounts"=array[559 elements], "DIALEnergy"=1272.0, "DIALTEC"=23.1282902, "DIALWavelength"=828.1949970058118}, {"DIALCounts"=array[559 elements], "DIALEnergy"=1323.0, "DIALTEC"=29.5466862, "DIALWavelength"=828.2946901675556}]
  in  "OnlinIndex":i32
  out "HSRL":T10={"HSRLCombinedCounts"=array[559 elements], "HSRLMolecularCounts"=[197.0, 137.0, 131.0, 134.0, 103.0, 132.0, 145.0, 156.0, 171.0, 185.0, 205.0, 242.0, 243.0, 262.0, 282.0, 264.0, 243.0, 265.0, 280.0, 291.0, 319.0, 289.0, 297.0, 279.0, 256.0, 263.0, 259.0, 264.0, 236.0, 265.0, 244.0, 231.0, 223.0, 204.0, 219.0, 218.0, 225.0, 216.0, 186.0, 206.0, 202.0, 176.0, 184.0, 177.0, 193.0, 175.0, 189.0, 153.0, 143.0, 170.0, 174.0, 148.0, 134.0, 134.0, 165.0, 144.0, 119.0, 144.0, 134.0, 133.0, 140.0, 114.0, 138.0, 112.0, 123.0, 126.0, 115.0, 121.0, 135.0, 128.0, 123.0, 102.0, 93.0, 81.0, 106.0, 105.0, 121.0, 103.0, 107.0, 101.0, 99.0, 97.0, 104.0, 85.0, 86.0, 90.0, 103.0, 94.0, 85.0, 102.0, 103.0, 89.0, 99.0, 94.0, 94.0, 103.0, 91.0, 107.0, 106.0, 93.0, 100.0, 89.0, 78.0, 99.0, 107.0, 82.0, 99.0, 80.0, 91.0, 85.0, 69.0, 84.0, 98.0, 83.0, 99.0, 89.0, 79.0, 80.0, 77.0, 92.0, 81.0, 77.0, 88.0, 73.0, 75.0, 86.0, 92.0, 88.0, 90.0, 86.0, 91.0, 95.0, 78.0, 73.0, 90.0, 86.0, 80.0, 99.0, 93.0, 73.0, 83.0, 89.0, 74.0, 93.0, 84.0, 86.0, 83.0, 81.0, 98.0, 100.0, 75.0, 80.0, 82.0, 74.0, 96.0, 72.0, 86.0, 82.0, 88.0, 85.0, 81.0, 80.0, 86.0, 69.0, 78.0, 83.0, 85.0, 67.0, 69.0, 106.0, 79.0, 70.0, 83.0, 76.0, 89.0, 92.0, 89.0, 71.0, 67.0, 78.0, 73.0, 74.0, 88.0, 71.0, 77.0, 80.0, 99.0, 76.0, 83.0, 92.0, 76.0, 64.0, 69.0, 89.0, 67.0, 61.0, 74.0, 89.0, 90.0, 73.0, 78.0, 69.0, 76.0, 70.0, 74.0, 80.0, 73.0, 77.0, 85.0, 76.0, 81.0, 70.0, 73.0, 70.0, 95.0, 69.0, 75.0, 58.0, 73.0, 91.0, 76.0, 69.0, 74.0, 93.0, 74.0, 73.0, 78.0, 74.0, 99.0, 93.0, 90.0, 75.0, 86.0, 88.0, 74.0, 78.0, 63.0, 85.0, 97.0, 85.0, 136.0, 156.0, 192.0, 211.0, 199.0, 163.0, 137.0, 114.0, 92.0, 110.0, 100.0, 104.0, 88.0, 107.0, 91.0, 110.0, 96.0, 103.0, 105.0, 109.0, 88.0, 105.0, 117.0, 120.0, 139.0, 142.0, 168.0, 190.0, 179.0, 184.0, 141.0, 130.0, 150.0, 125.0, 117.0, 101.0, 76.0, 85.0, 81.0, 74.0, 85.0, 88.0, 66.0, 69.0, 68.0, 80.0, 71.0, 84.0, 72.0, 77.0, 86.0, 81.0, 79.0, 83.0, 82.0, 73.0, 71.0, 65.0, 83.0, 88.0, 87.0, 73.0, 92.0, 71.0, 78.0, 79.0, 95.0, 85.0, 70.0, 59.0, 63.0, 101.0, 75.0, 79.0, 74.0, 93.0, 80.0, 62.0, 78.0, 80.0, 77.0, 59.0, 74.0, 82.0, 87.0, 81.0, 82.0, 78.0, 73.0, 90.0, 102.0, 69.0, 62.0, 79.0, 68.0, 83.0, 66.0, 91.0, 62.0, 82.0, 79.0, 82.0, 74.0, 90.0, 88.0, 63.0, 78.0, 71.0, 79.0, 79.0, 68.0, 82.0, 76.0, 76.0, 72.0, 73.0, 79.0, 72.0, 59.0, 93.0, 88.0, 84.0, 72.0, 79.0, 69.0, 81.0, 84.0, 86.0, 70.0, 74.0, 94.0, 82.0, 74.0, 85.0, 68.0, 60.0, 69.0, 74.0, 81.0, 67.0, 70.0, 75.0, 85.0, 56.0, 76.0, 60.0, 72.0, 88.0, 86.0, 64.0, 65.0, 78.0, 86.0, 54.0, 83.0, 59.0, 60.0, 83.0, 69.0, 80.0, 84.0, 79.0, 73.0, 91.0, 84.0, 90.0, 90.0, 85.0, 70.0, 85.0, 92.0, 77.0, 69.0, 66.0, 66.0, 86.0, 71.0, 71.0, 85.0, 75.0, 75.0, 64.0, 75.0, 72.0, 97.0, 84.0, 76.0, 88.0, 67.0, 82.0, 70.0, 87.0, 73.0, 75.0, 69.0, 75.0, 89.0, 73.0, 80.0, 78.0, 94.0, 73.0, 87.0, 66.0, 68.0, 91.0, 88.0, 70.0, 64.0, 74.0, 82.0, 83.0, 75.0, 76.0, 71.0, 92.0, 78.0, 79.0, 83.0, 92.0, 72.0, 98.0, 63.0, 84.0, 58.0, 65.0, 74.0, 82.0, 88.0, 86.0, 78.0, 79.0, 82.0, 73.0, 80.0, 74.0, 87.0, 69.0, 76.0, 63.0, 61.0, 72.0, 83.0, 76.0, 66.0, 86.0, 88.0, 90.0, 83.0, 75.0, 65.0, 66.0, 87.0, 81.0, 89.0, 92.0, 74.0, 87.0, 84.0, 65.0, 75.0, 81.0, 91.0, 75.0, 77.0, 61.0, 66.0, 95.0, 81.0, 76.0, 82.0, 88.0, 77.0, 74.0, 73.0, 78.0, 67.0, 74.0, 71.0, 90.0, 72.0, 78.0, 65.0, 75.0, 62.0, 97.0, 67.0, 64.0, 86.0, 85.0, 76.0, 88.0, 96.0, 72.0, 76.0, 66.0, 62.0, 84.0, 80.0, 84.0, 76.0, 83.0, 68.0, 69.0, 61.0, 68.0, 88.0, 83.0, 85.0, 57.0, 73.0, 74.0, 90.0, 83.0, 68.0, 72.0, 79.0, 75.0, 77.0], "HSRLLaserEnergy"=0.0, "HSRLTEC"=18.6453495, "HSRLWavelength"=780.2460455998352}
  out "WeatherStation":T11={"Pressure"=847.1703296703296, "RelativeHumidity"=22.21001221001221, "Temperature"=16.758852258852258, "AbsoluteHumidity"=16.758852258852258}
  out "size(s)":i32=559
  in  "bins":u32=560 min=2 max=4095 step=1
  out "y offset":u32=10
  in  "ns scale":u32=250
  # "NetCDFStuff"
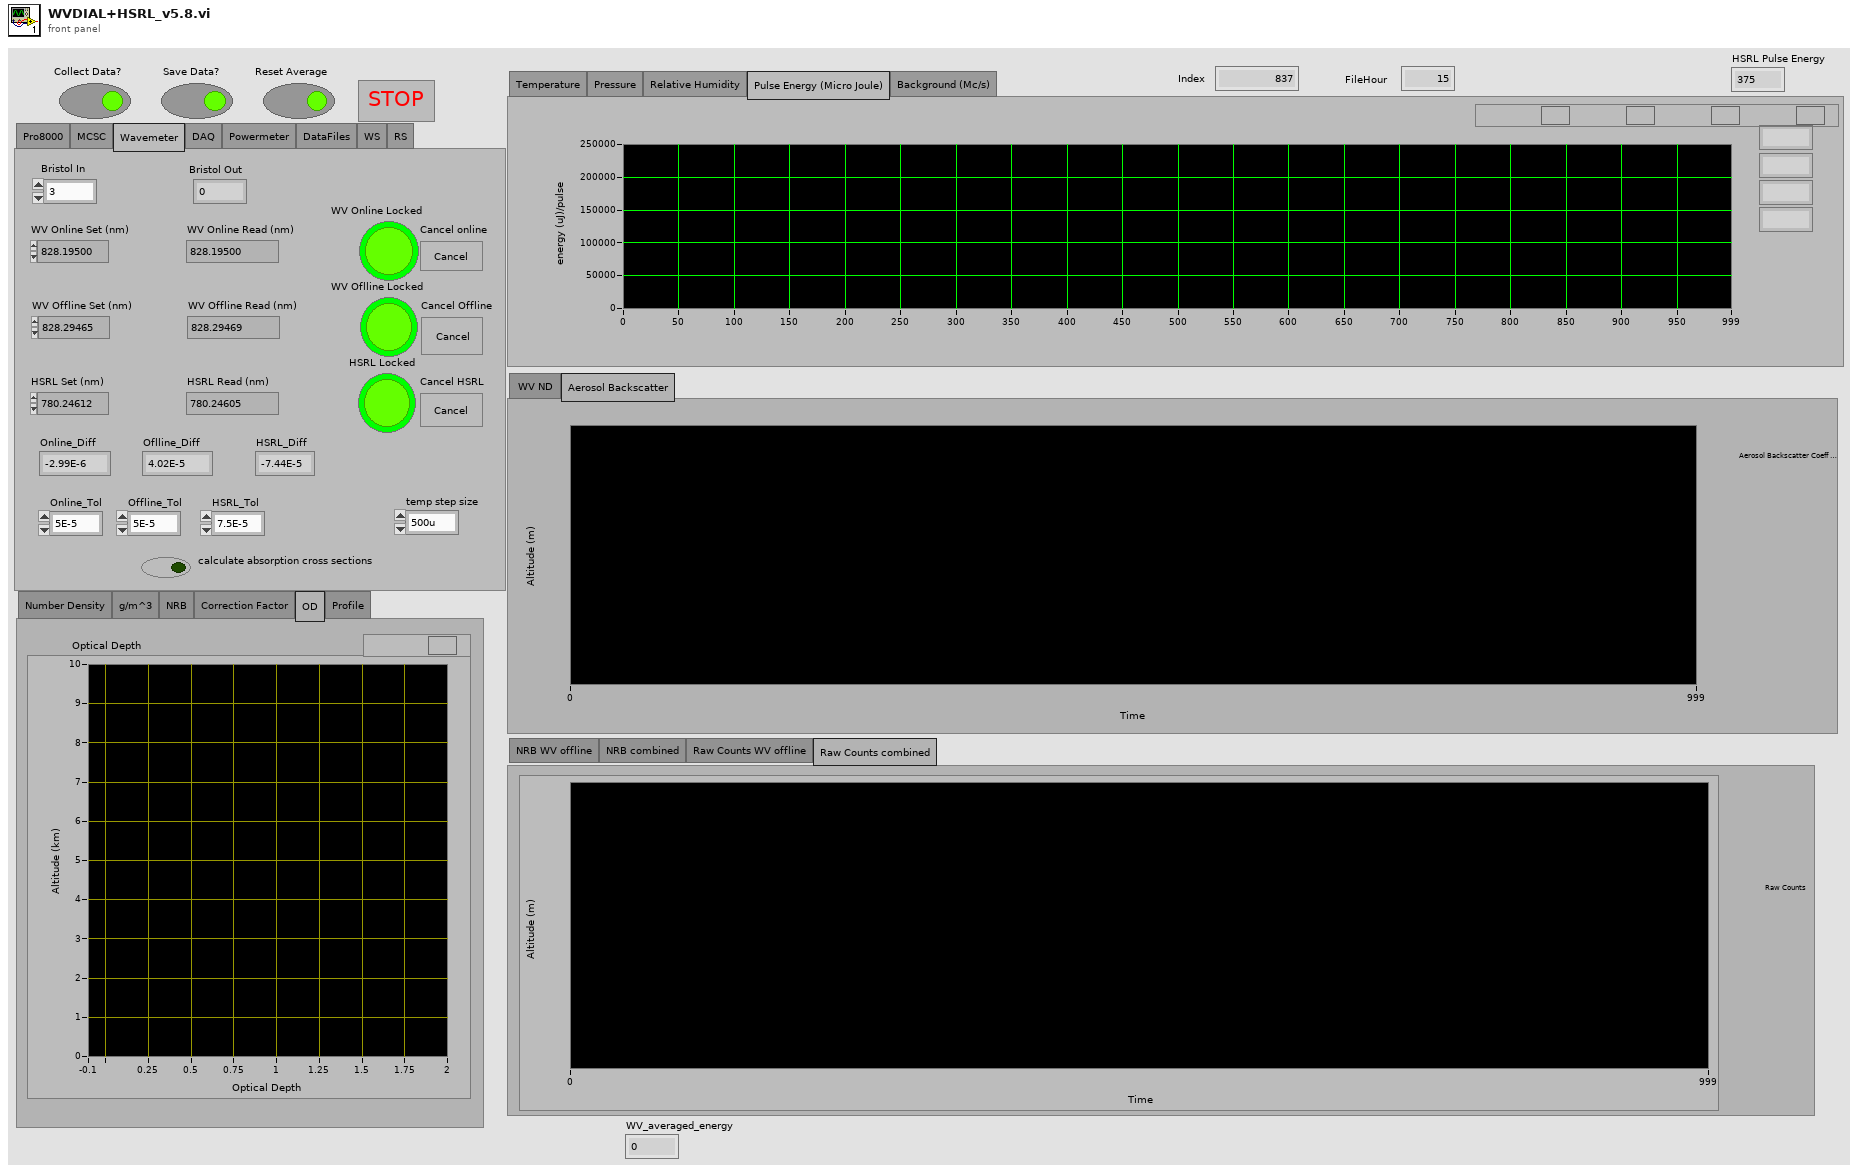
[diagram p1: front panel]
types:
  T1 = enum32{"NRB WV offline", "NRB combined", "Raw Counts WV offline", "Raw Counts combined"}
  T2 = enum32{"Number Density", "g/m^3", "NRB", "Correction Factor", "OD", "Profile"}
  T3 = enum32{"Temperature", "Pressure", "Relative Humidity", "Pulse Energy (Micro Joule)", "Background (Mc/s)"}
  T4 = cluster{"WV Online Pulse Energy":dbl, "WV_averaged_energy":dbl, "HSRL":dbl, "WV_averaged_energy":dbl}
  T5 = enum32{"Pro8000", "MCSC", "Wavemeter", "DAQ", "Powermeter", "DataFiles", "WS", "RS"}
  T6 = cluster{"Module":enum16{"WV Online TEC", "WV Online LD", "WV Offline TEC", "WV Offline LD", "WV Etalon TEC", "HSRL Etalon TEC", "HSRL TEC", "HSRL LD"}, "WV Online TEC":dbl, "WV Online LD":dbl, "WV Offline TEC":dbl, "WV Offline LD":dbl, "WV Etalon TEC":dbl, "HSRL Etalon TEC":dbl, "HSRL TEC":dbl, "HSRL LD":dbl}
  T7 = cluster{"Pro8000":bool, "WV OnLine TEC":dbl, "WV Online TEC":bool, "WV Online LD":dbl, "WV Online LD":bool, "WV Offline TEC":dbl, "WV Offline TEC":bool, "WV Offline LD":dbl, "WV Offline LD":bool, "WV EtalonTEC":dbl, "WV Etalon TEC":bool, "HSRL Etalon TEC":dbl, "HSRL Etalon TEC":bool, "HSRL TEC":dbl, "HSRL TEC ":bool, "HSRL LD":dbl, "HSRL LD":bool}
  T8 = cluster{"Temp C":dbl, "RelH %":dbl, "Press hPa":dbl, "AbH g/m^3":dbl}
  T9 = cluster{"DIALCounts":dbl[], "DIALEnergy":dbl, "DIALTEC":dbl, "DIALWavelength":dbl}[]
  T10 = cluster{"HSRLCombinedCounts":dbl[], "HSRLMolecularCounts":dbl[], "HSRLLaserEnergy":dbl, "HSRLTEC":dbl, "HSRLWavelength":dbl}
  T11 = cluster{"Pressure":dbl, "RelativeHumidity":dbl, "Temperature":dbl, "AbsoluteHumidity":dbl}
  T12 = enum16{"Open_TL", "Close_TL", "Verify_ID", "TEC_Sensor", "SET", "READ", "ON", "OFF", "Set_Limits", "Read_Limits", "Enable_Status", "Read_Status"}
  T13 = enum16{"Initialize ILX", "Set ON T", "Set Off T", "Set ON I", "Set Off I", "Set On Lim", "Set Off Lim", "Read ILX", "TEC ON/OFF", "LASER ON/OFF", "Status?", "ILX OFF"}
  T14 = enum16{"open", "replace", "create", "open or create", "replace or create", "replace or create with confirmation"}
  T15 = enum16{"WV Online TEC", "WV Online LD", "WV Offline TEC", "WV Offline LD", "WV Etalon TEC", "HSRL Etalon TEC", "HSRL TEC", "HSRL LD"}
  T16 = cluster{"Temp":dbl, "RelH":dbl, "Press":dbl, "AbH":dbl}
  T17 = typedef "LVDateTimeRec.ctl" = cluster{"fractional second":dbl, "second":i32, "minute":i32, "hour":i32, "day of month":i32, "month":i32, "year":i32, "day of week":i32, "day of year":i32, "DST":i32}
  T18 = cluster{"WV Online Pulse Energy":dbl, "WV Offline Pulse Energy":dbl, "HSRL Pulse Energy":dbl, "WV_averaged_energy":dbl}
  T19 = cluster{"DIALCounts":dbl[], "DIALEnergy":dbl, "DIALTEC":dbl, "DIALWavelength":dbl}
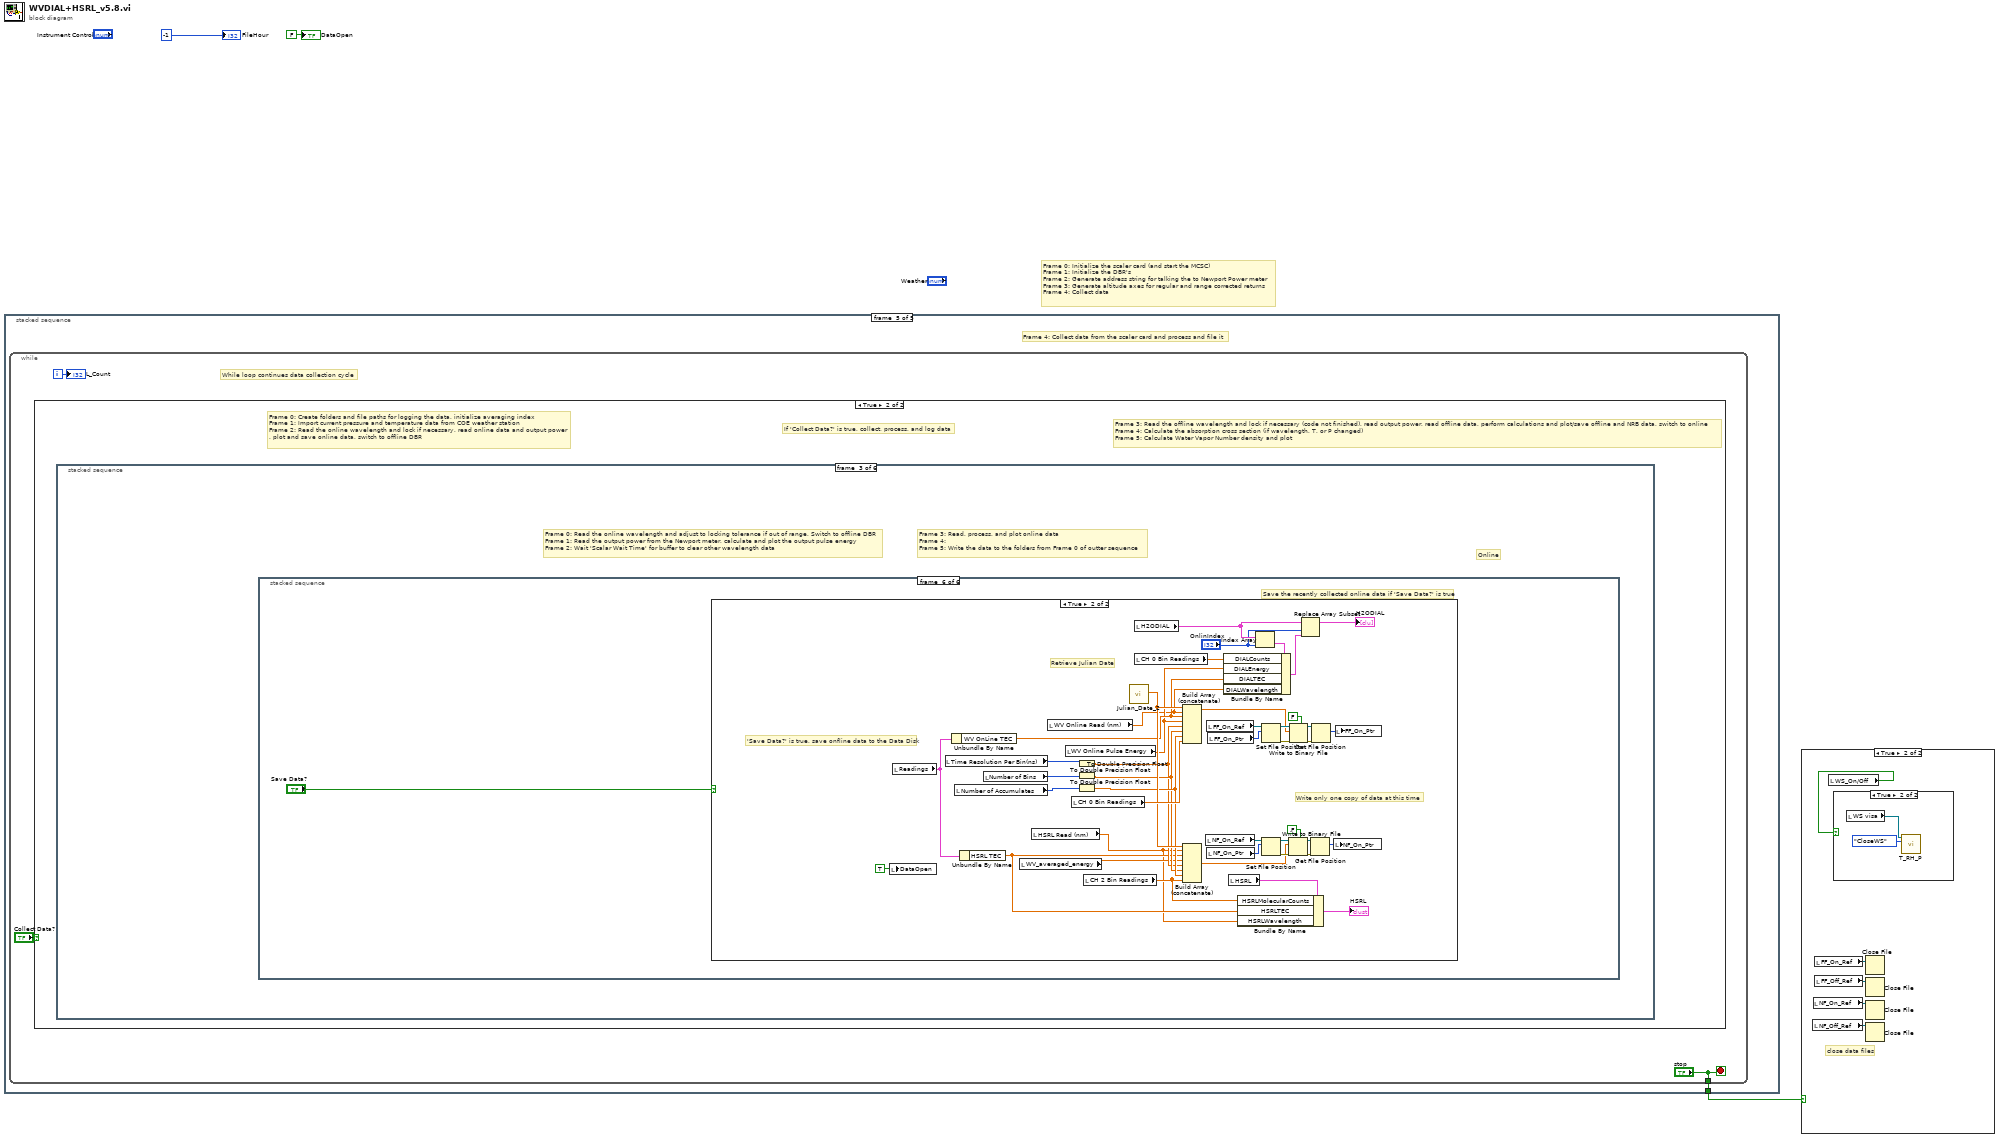
[diagram p0: block diagram]
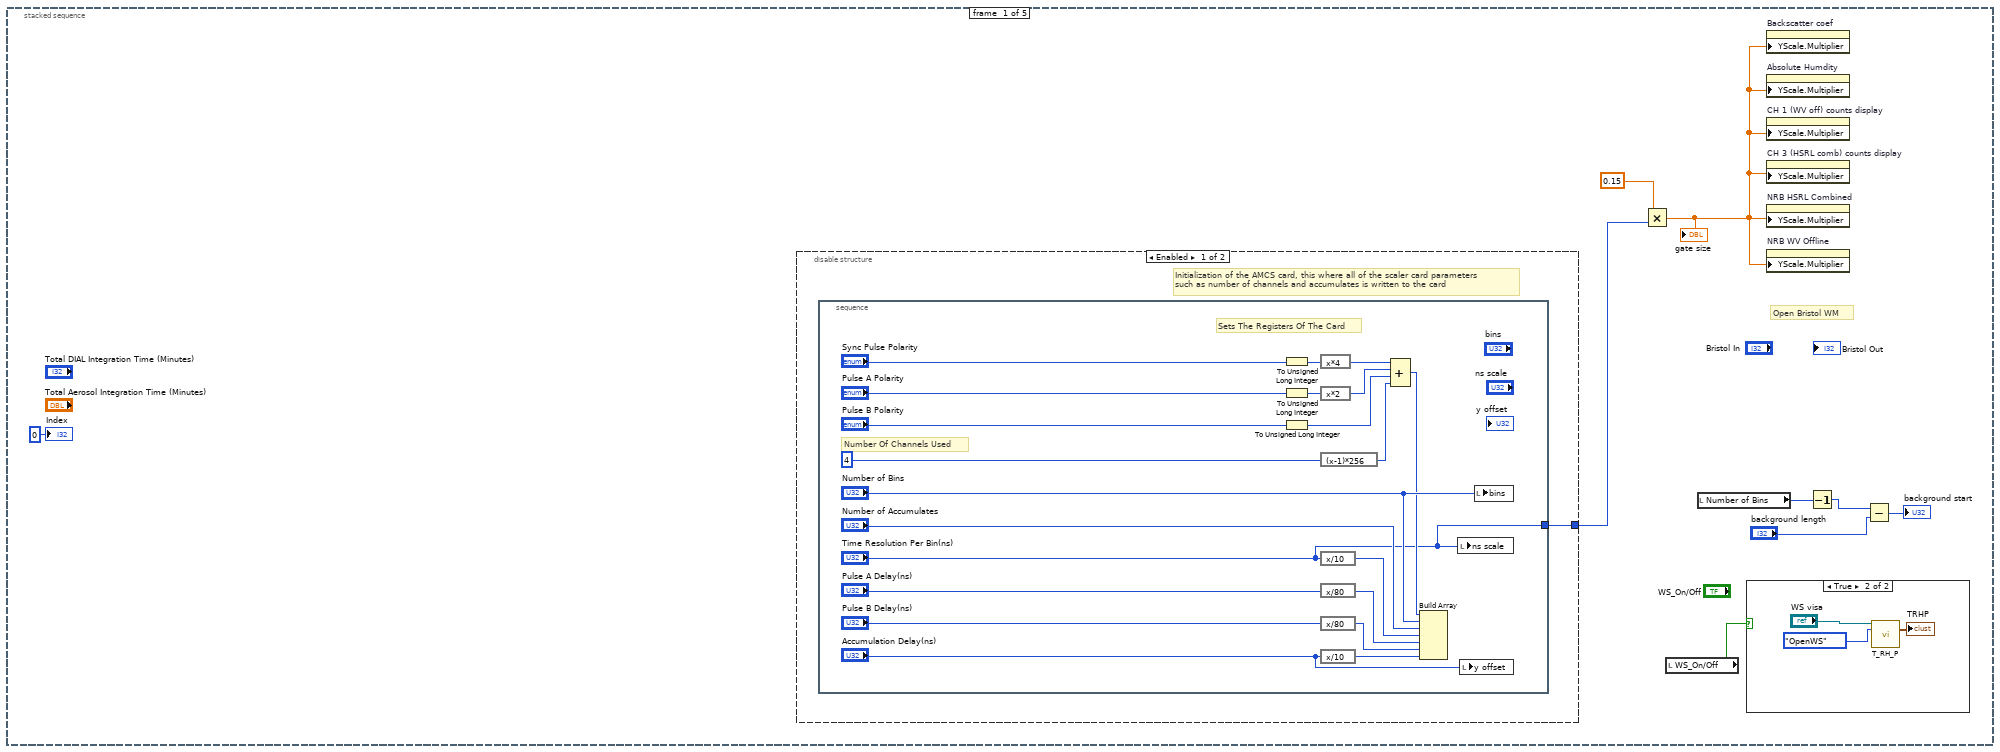
[diagram p4: hidden frame]
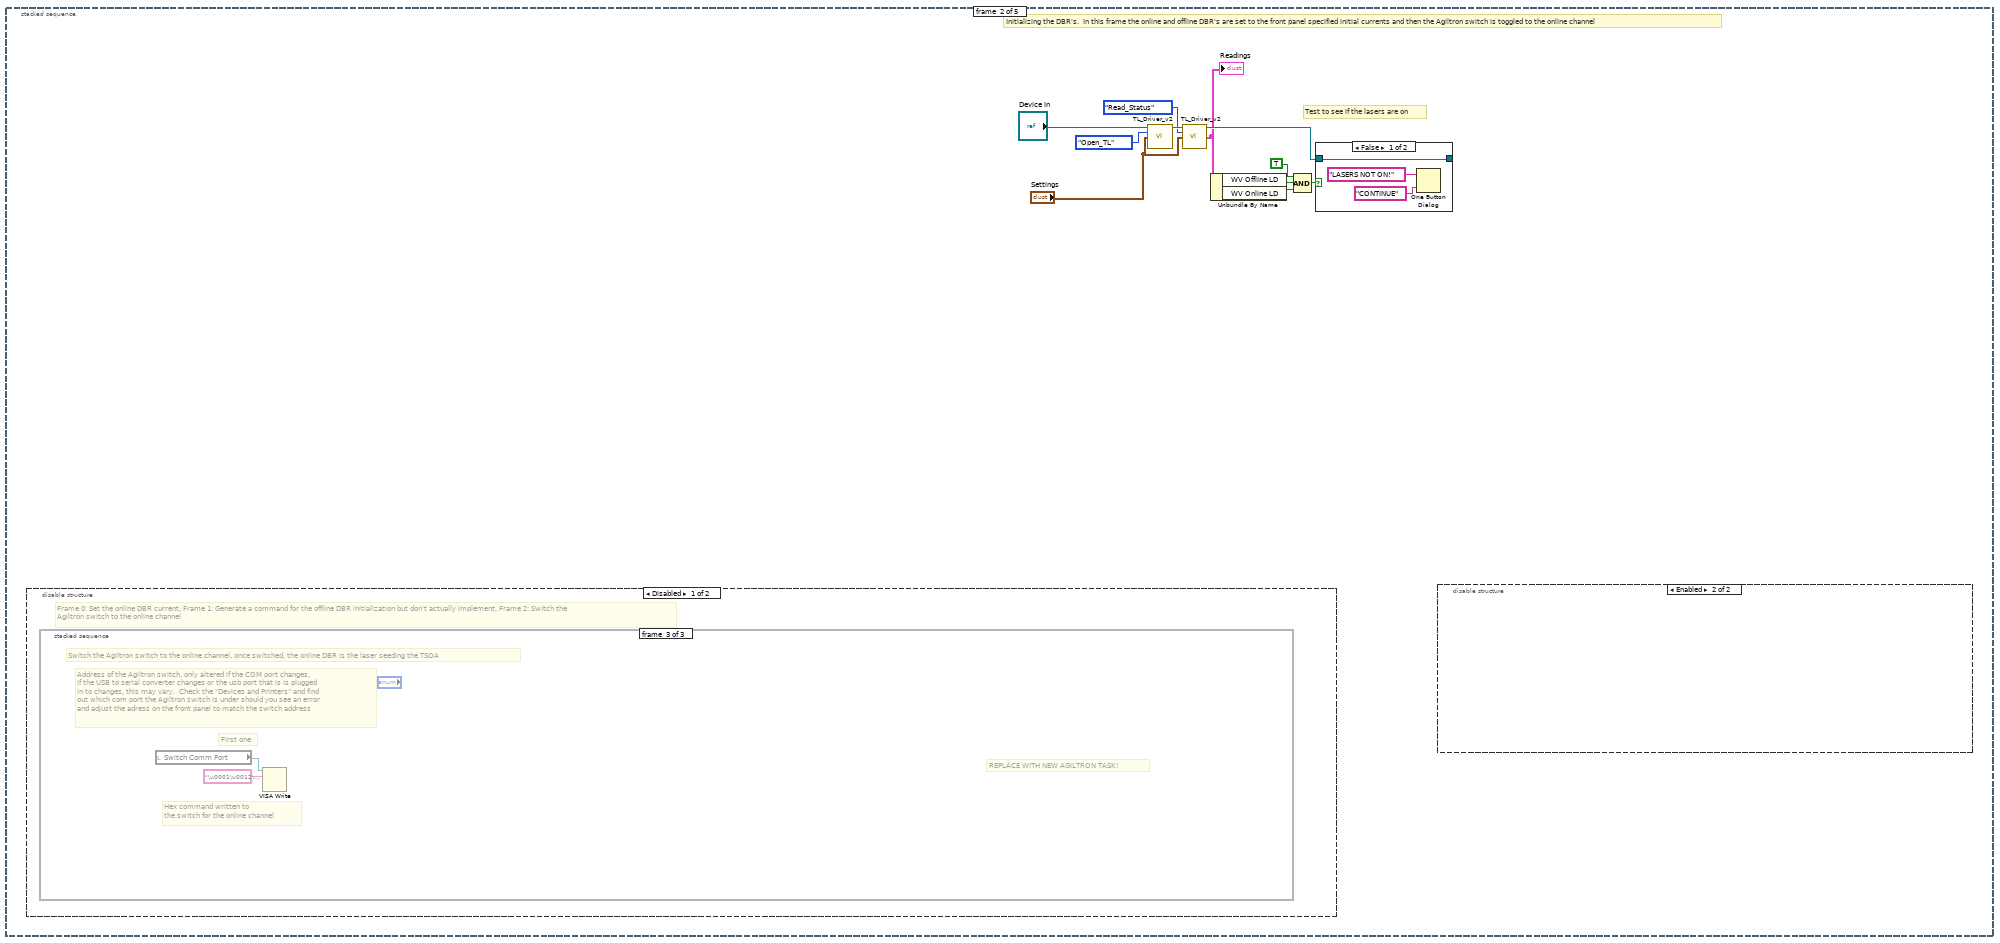
[diagram p7: hidden frame]
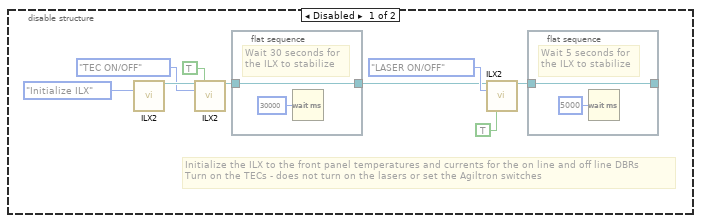
[diagram p9: hidden frame]
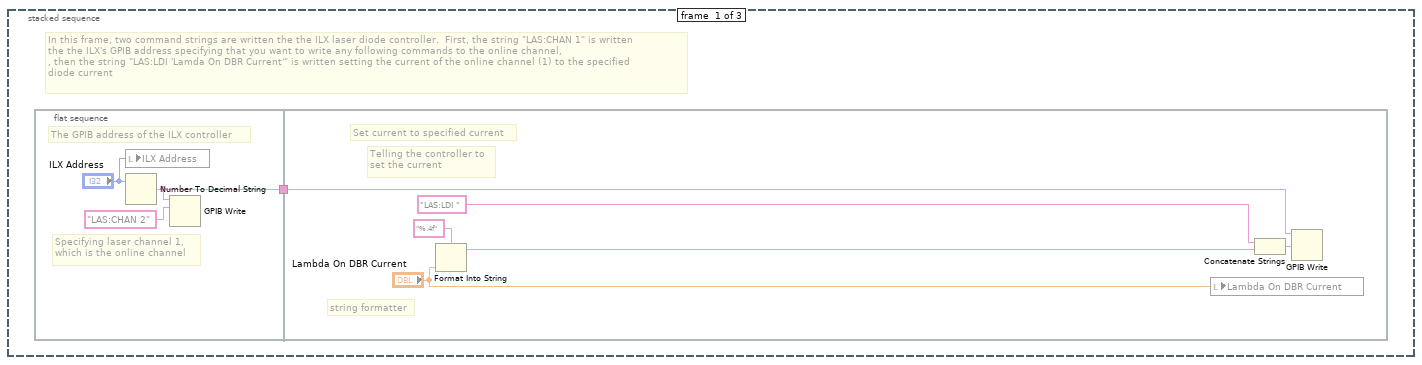
[diagram p10: hidden frame]
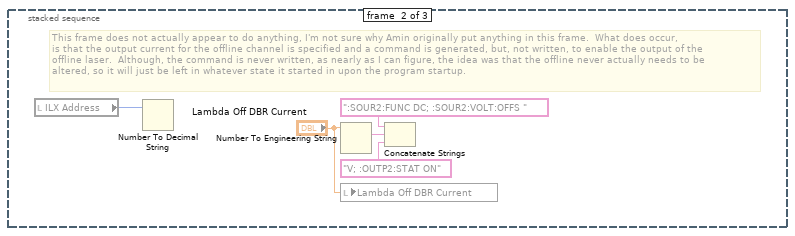
[diagram p11: hidden frame]
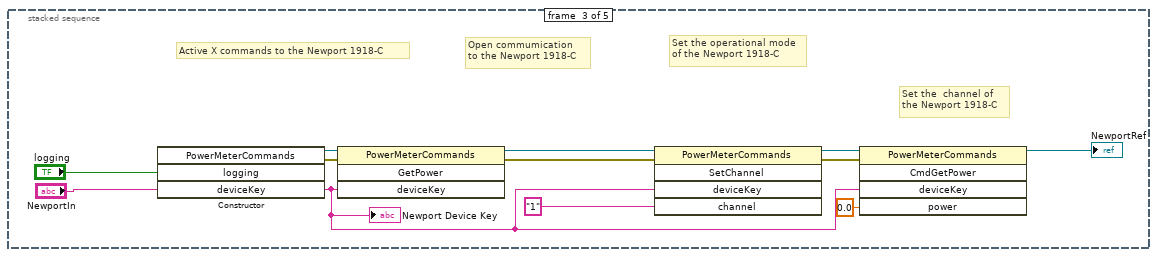
[diagram p13: hidden frame]
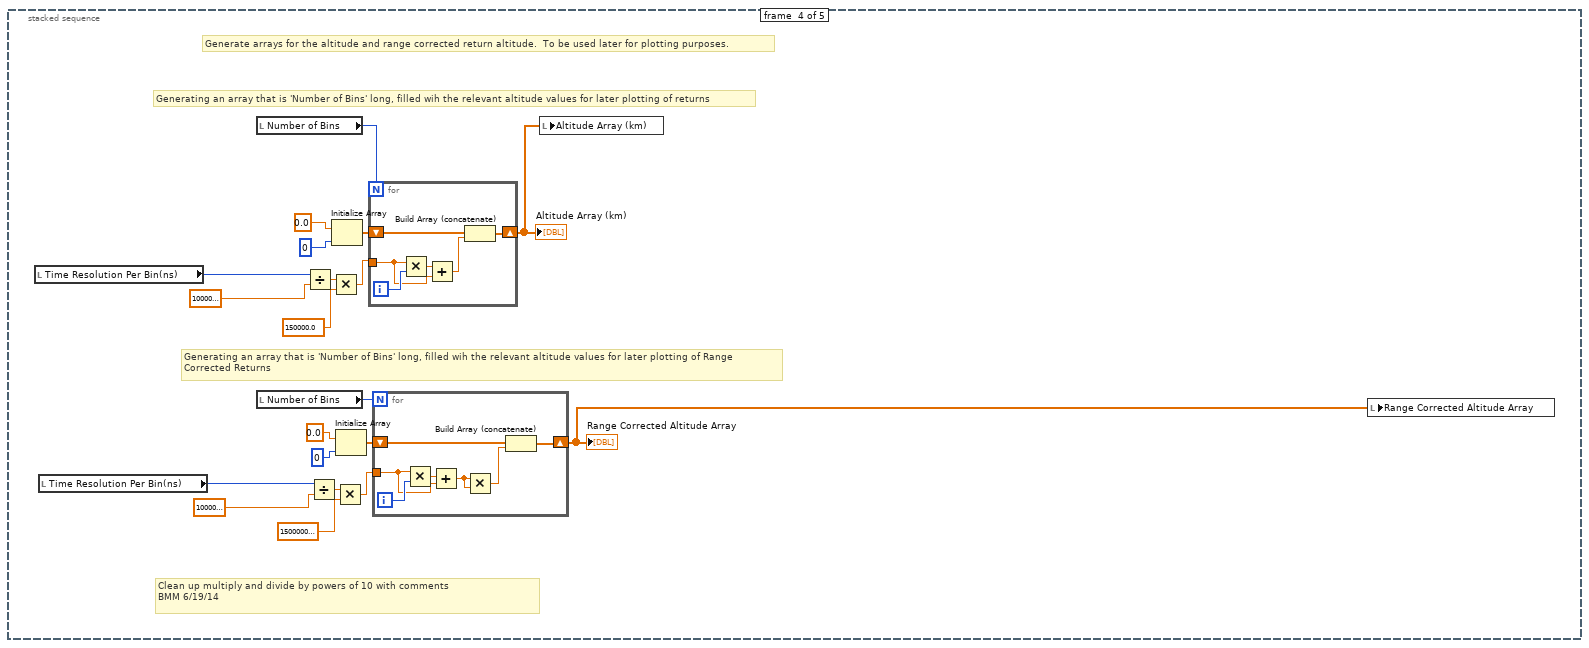
[diagram p14: hidden frame]
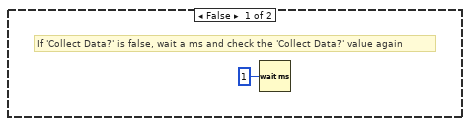
[diagram p15: hidden frame]
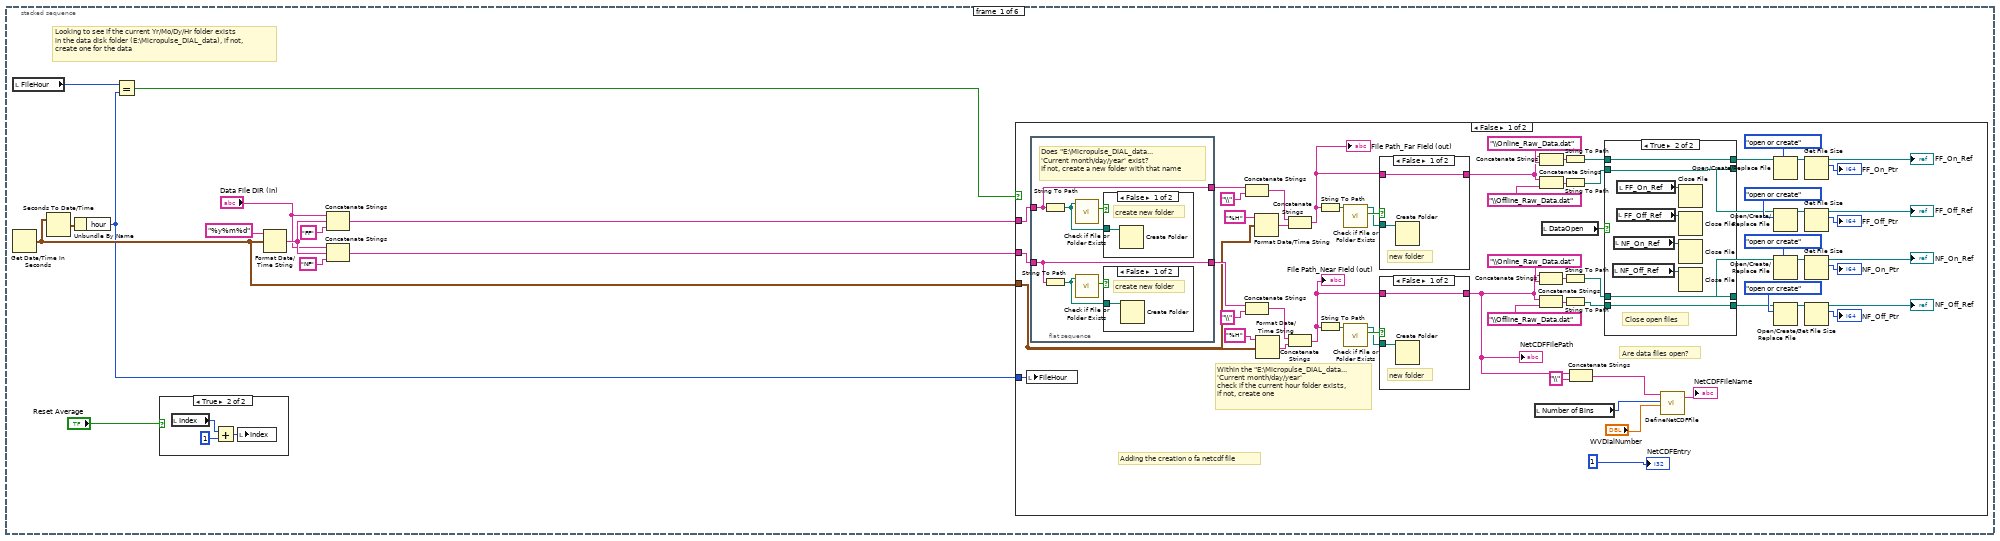
[diagram p16: hidden frame]
diagram:
  # "Frame 0: Initialize the scaler card (and start the MCSC)\nFrame 1: Initialize the DBR's\nFrame 2: Generate address string for talking the to Newport Power meter\nFrame 3: Generate altitude axes for regular and range corrected returns\nFrame 4: Collect data"
  n1 = stacked-sequence {
    tunnel: [_ _ _ _ w128] -> w3
    frame #0 {
      # "Open Bristol WM"
      n2 = disable-structure shown="Enabled" {
        disable-tunnel: [w16 _] -> w5
        frame Enabled {
          # "Initialization of the AMCS card, this where all of the scaler card parameters\nsuch as number of channels and accumulates is written to the card"
          n3 = stacked-sequence {
            tunnel: ["Time Resolution Per Bin(ns)"] -> w16
            frame #0 {
              # "Sets The Registers Of The Card"
              # "Number Of Channels Used"
              n4 = To Unsigned Long Integer(number="Sync Pulse Polarity") -> (unsigned 32bit integer=w18:u32)
              n5 = To Unsigned Long Integer(number="Pulse A Polarity") -> (unsigned 32bit integer=w22:u32)
              n6 = To Unsigned Long Integer(number="Pulse B Polarity") -> (unsigned 32bit integer=w20:u32)
              n7 = expression code="x*4"(w18) -> (w27:u32)
              n8 = expression code="x*2"(w22) -> (w26:u32)
              n9 = expression code="(x-1)*256"(u32 4 ("Number of Channels Used")) -> (w25:u32)
              n10 = expression code="x/10"("Time Resolution Per Bin(ns)") -> (w28:u32)
              n11 = expression code="x/80"("Pulse A Delay(ns)") -> (w35:u32)
              n12 = expression code="x/80"("Pulse B Delay(ns)") -> (w37:u32)
              n13 = expression code="x/10"("Accumulation Delay(ns)") -> (w36:u32)
              n14 = Compound Arithmetic op=ADD(w27, w26, w20, w25) -> (w24:u32)
              n15 = Build Array(w24, "Number of Bins", "Number of Accumulates", w28, w35, w37, w36) -> ()  [unwired: 1 out]
              n16 = local write "ns scale"("Time Resolution Per Bin(ns)") -> ()
              n17 = local write "y offset"("Accumulation Delay(ns)") -> ()
              n18 = local write "bins"("Number of Bins") -> ()
            }
          }
        }
        frame Disabled {
        }
      }
      n19 = Multiply(x=0.15, y=w5) -> (x*y=w4:dbl)
      "gate size" <- w4
      n20 = local read "WS_On/Off"() -> (w7:bool)
      n21 = local read "Number of Bins"() -> (w11:u32)
      n22 = case shown="True" w7 {
        frame False {
        }
        frame True {
          n23 = call "T_RH_P.vi"("VISA in"="WS visa", "WS_Commands"=enum16{"OpenWS", "ReadTRHP", "CloseWS"}."OpenWS") -> ("TRHP"=→"TRHP":T16)  [unwired: 11 in, 2 out]
        }
      }
      n24 = property on="Backscatter coef" class="IntChart (strict)"("YScale.Multiplier"=w4) -> ()  [unwired: 2 in, 2 out]
      n25 = property on="Absolute Humdity" class="IntChart (strict)"("YScale.Multiplier"=w4) -> ()  [unwired: 2 in, 2 out]
      n26 = property on="CH 1 (WV off) counts display" class="IntChart (strict)"("YScale.Multiplier"=w4) -> ()  [unwired: 2 in, 2 out]
      n27 = property on="CH 3 (HSRL comb) counts display" class="IntChart (strict)"("YScale.Multiplier"=w4) -> ()  [unwired: 2 in, 2 out]
      n28 = property on="NRB HSRL Combined" class="IntChart (strict)"("YScale.Multiplier"=w4) -> ()  [unwired: 2 in, 2 out]
      n29 = property on="NRB WV Offline" class="IntChart (strict)"("YScale.Multiplier"=w4) -> ()  [unwired: 2 in, 2 out]
      n30 = Decrement(x=w11) -> (x-1=w10:u32)
      n31 = Subtract(x=w10, y="background length") -> (x-y=→"background start":u32)
      "Index" <- 0 ("Index")
    }
    frame #1 {
      # "Test to see if the lasers are on"
      # "Initializing the DBR's.  In this frame the online and offline DBR's are set to the front panel specified initial currents and then the Agiltron switch is toggled to the online channel"
      n32 = disable-structure shown="Disabled" {
        frame Disabled {
          # "Frame 0: Set the online DBR current, Frame 1: Generate a command for the offline DBR initialization but don't actually implement, Frame 2: Switch the \nAgiltron switch to the online channel"
          n33 = stacked-sequence {
            frame #0 {
              # "In this frame, two command strings are written the the ILX laser diode controller.  First, the string \"LAS:CHAN 1\" is written\nthe the ILX's GPIB address specifying that you want to write any following commands to the online channel,\n, then the string \"LAS:LDI 'Lamda On DBR Current'\" is written setting the current of the online channel (1) to the specified \ndiode current"
              n34 = flat-sequence {
                tunnel: [w68] -> w66
                tunnel: w66 -> [w70]
                frame #0 {
                  # "The GPIB address of the ILX controller"
                  # "Specifying laser channel 1,\nwhich is the online channel"
                  n35 = local write "ILX Address"("ILX Address") -> ()
                  n36 = Number To Decimal String(number="ILX Address") -> (decimal integer string=w68:string)  [unwired: 1 in]
                  n37 = GPIB Write(0:w68, 1:"LAS:CHAN 2") -> ()  [unwired: 3 in, 2 out]
                }
                frame #1 {
                  # "Telling the controller to\nset the current"
                  # "string formatter"
                  # "Set current to specified current"
                  n38 = Format Into String(format string="%.4f" ("Format String"), "Lambda On DBR Current") -> (resulting string=w73:string)  [unwired: 2 in, 1 out]
                  n39 = local write "Lambda On DBR Current"("Lambda On DBR Current") -> ()
                  n40 = Concatenate Strings("LAS:LDI ", w73) -> (w74:string)
                  n41 = GPIB Write(0:w70, 1:w74) -> ()  [unwired: 3 in, 2 out]
                }
              }
            }
            frame #1 {
              # "This frame does not actually appear to do anything, I'm not sure why Amin originally put anything in this frame.  What does occur, \nis that the output current for the offline channel is specified and a command is generated, but, not written, to enable the output of the\noffline laser.  Although, the command is never written, as nearly as I can figure, the idea was that the offline never actually needs to be \naltered, so it will just be left in whatever state it started in upon the program startup."
              n42 = local read "ILX Address"() -> (w76:i32)
              n43 = Number To Decimal String(number=w76) -> ()  [unwired: 1 in, 1 out]
              n44 = Number To Engineering String(4:"Lambda Off DBR Current") -> (0:w80:string)  [unwired: 3 in]
              n45 = local write "Lambda Off DBR Current"("Lambda Off DBR Current") -> ()
              n46 = Concatenate Strings(":SOUR2:FUNC DC; :SOUR2:VOLT:OFFS ", w80, "V; :OUTP2:STAT ON") -> ()  [unwired: 1 out]
            }
            frame #2 {
              # "REPLACE WITH NEW AGILTRON TASK!"
              # "First one"
              # "Address of the Agiltron switch, only altered if the COM port changes,\nif the USB to serial converter changes or the usb port that is is plugged\nin to changes, this may vary.  Check the \"Devices and Printers\" and find \nout which com port the Agiltron switch is under should you see an error \nand adjust the adress on the front panel to match the switch address"
              # "Hex command written to \nthe switch for the online channel"
              # "Switch the Agiltron switch to the online channel, once switched, the online DBR is the laser seeding the TSOA"
              n47 = local read "Switch Comm Port"() -> (w81:refnum<visa-resource-name>)
              n48 = VISA Write(VISA resource name=w81, write buffer="\u0001\u0012\u0000\u0002") -> ()  [unwired: 1 in, 3 out]
            }
          }
        }
        frame Enabled {
        }
      }
      n49 = call "TL_Driver_v2.vi"("Device In"="Device In", "Commands"=T12."Open_TL", "Settings"="Settings") -> ("Device Out"=w46:refnum<visa-resource-name>)  [unwired: 9 in, 3 out]
      n50 = call "TL_Driver_v2.vi"("Device In"=w46, "Commands"=T12."Read_Status", "Settings"="Settings") -> ("Device Out"=w44:refnum<visa-resource-name>, "Readings"=w38:T7)  [unwired: 9 in, 2 out]
      "Readings" <- w38
      n51 = Unbundle By Name(w38) -> ("WV Offline LD"=w41:bool, "WV Online LD"=w42:bool)
      n52 = Compound Arithmetic op=AND(TRUE, w41, w42) -> (w40:bool)
      n53 = case shown="False" w40 {
        tunnel: w44 -> [w49 w52]
        tunnel: [w49 w52] -> _
        frame False {
          n54 = One Button Dialog(message="LASERS NOT ON!", button name ("OK")="CONTINUE") -> ()  [unwired: 1 out]
        }
        frame True {
        }
      }
      n55 = disable-structure shown="Enabled" {
        frame Disabled {
          # "Initialize the ILX to the front panel temperatures and currents for the on line and off line DBRs\nTurn on the TECs - does not turn on the lasers or set the Agiltron switches"
          n56 = call "ILX2.vi"("ILX Command"=T13."Initialize ILX") -> ("Device Out"=w60:refnum<visa-resource-name>)  [unwired: 10 in, 4 out]
          n57 = call "ILX2.vi"("Device In"=w60, "TEC Control"=TRUE, "ILX Command"=T13."TEC ON/OFF") -> ("Device Out"=w57:refnum<visa-resource-name>)  [unwired: 8 in, 4 out]
          n58 = flat-sequence {
            tunnel: w57 -> [w64]
            tunnel: [w64] -> w54
            frame #0 {
              # "Wait 30 seconds for\nthe ILX to stabilize"
              n59 = Wait (ms)(milliseconds to wait=u32 30000) -> ()  [unwired: 1 out]
            }
          }
          n60 = call "ILX2.vi"("Device In"=w54, "ILX Command"=T13."LASER ON/OFF", "Laser Control"=TRUE ("TEC Control")) -> ("Device Out"=w53:refnum<visa-resource-name>)  [unwired: 8 in, 4 out]
          n61 = flat-sequence {
            tunnel: w53 -> [w62]
            tunnel: [w62] -> _
            frame #0 {
              # "Wait 5 seconds for\nthe ILX to stabilize"
              n62 = Wait (ms)(milliseconds to wait=u32 5000) -> ()  [unwired: 1 out]
            }
          }
        }
        frame Enabled {
        }
      }
    }
    frame #2 {
      # "Active X commands to the Newport 1918-C"
      # "Set the  channel of\nthe Newport 1918-C"
      # "Set the operational mode\nof the Newport 1918-C"
      # "Open commumication\nto the Newport 1918-C"
      n63 = constructor class="PowerMeterCommands"("logging"="logging", "deviceKey"="NewportIn") -> (reference out=w94:refnum<k24>, error out=w91:errorcluster, "deviceKey"=w86:string)  [unwired: 3 in, 2 out]
      "Newport Device Key" <- w86
      n64 = invoke class="PowerMeterCommands" method="GetPower"(reference=w94, error in=w91, "deviceKey"=w86) -> (reference out=w93:refnum<k24>, error out=w90:errorcluster)  [unwired: 1 in, 2 out]
      n65 = invoke class="PowerMeterCommands" method="SetChannel"(reference=w93, error in=w90, "deviceKey"=w86, "channel"="1") -> (reference out=w87:refnum<k24>, error out=w89:errorcluster)  [unwired: 1 in, 3 out]
      n66 = invoke class="PowerMeterCommands" method="CmdGetPower"(reference=w87, error in=w89, "deviceKey"=w86, "power"=sgl 0.0) -> (reference out=→"NewportRef":refnum<k24>)  [unwired: 1 in, 4 out]
    }
    frame #3 {
      # "Clean up multiply and divide by powers of 10 with comments\nBMM 6/19/14"
      # "Generating an array that is 'Number of Bins' long, filled wih the relevant altitude values for later plotting of Range \nCorrected Returns"
      # "Generating an array that is 'Number of Bins' long, filled wih the relevant altitude values for later plotting of returns"
      # "Generate arrays for the altitude and range corrected return altitude.  To be used later for plotting purposes."
      n67 = local read "Time Resolution Per Bin(ns)"() -> (w107:u32)
      n68 = local read "Time Resolution Per Bin(ns)"() -> (w97:u32)
      n69 = local read "Number of Bins"() -> (w110:u32)
      n70 = local read "Number of Bins"() -> (w100:u32)
      n71 = Divide(x=w107, y=1000000000.0) -> (x/y=w105:dbl)
      n72 = Divide(x=w97, y=1000000000.0) -> (x/y=w95:dbl)
      n73 = Multiply(x=w105, y=150000.0) -> (x*y=w108:dbl)
      n74 = Initialize Array(0.0, 0) -> (w113:dbl[])
      n75 = Multiply(x=w95, y=150000000.0) -> (x*y=w98:dbl)
      n76 = Initialize Array(0.0, 0) -> (w103:dbl[])
      n77 = for {
        N: w110 -> [_]
        shift-right: [w126] -> w111
        shift-left: w113 -> [w127]
        tunnel: w108 -> [w123]
        i -> [w125]
        n78 = Multiply(x=w123, y=w125) -> (x*y=w124:dbl)
        n79 = Add(x=w124, y=w123) -> (x+y=w122:dbl)
        n80 = Build Array (concatenate)(w127, w122) -> (w126:dbl[])
      }
      "Altitude Array (km)" <- w111
      n81 = for {
        N: w100 -> [_]
        shift-right: [w120] -> w101
        shift-left: w103 -> [w121]
        tunnel: w98 -> [w116]
        i -> [w119]
        n82 = Multiply(x=w116, y=w119) -> (x*y=w117:dbl)
        n83 = Add(x=w117, y=w116) -> (x+y=w115:dbl)
        n84 = Multiply(x=w115, y=w115) -> (x*y=w118:dbl)
        n85 = Build Array (concatenate)(w121, w118) -> (w120:dbl[])
      }
      "Range Corrected Altitude Array" <- w101
      n86 = local write "Altitude Array (km)"(w111) -> ()
      n87 = local write "Range Corrected Altitude Array"(w101) -> ()
    }
    frame #4 {
      # "Frame 4: Collect data from the scaler card and process and file it"
      n88 = while {
        tunnel: ["stop"] -> w128
        i -> [w129]
        stop <- "stop" stop-if-true
        # "While loop continues data collection cycle"
        n89 = case shown="True" "Collect Data?" {
          frame False {
            # "If 'Collect Data?' is false, wait a ms and check the 'Collect Data?' value again"
            n90 = Wait (ms)(milliseconds to wait=u32 1) -> ()  [unwired: 1 out]
          }
          frame True {
            # "Frame 3: Read the offline wavelength and lock if necessary (code not finished), read output power, read offline data, perform calculations and plot/save offline and NRB data, switch to online\nFrame 4: Calculate the absorption cross section (if wavelength, T, or P changed)\nFrame 5: Calculate Water Vapor Number density and plot"
            # "Frame 0: Create folders and file paths for logging the data, initialize averaging index\nFrame 1: Import current pressure and temperature data from COE weather station\nFrame 2: Read the online wavelength and lock if necessary, read online data and output power\n, plot and save online data, switch to offline DBR"
            # "If 'Collect Data?' is true, collect, process, and log data"
            n91 = stacked-sequence {
              frame #0 {
                # "Looking to see if the current Yr/Mo/Dy/Hr folder exists\nin the data disk folder (E:\\Micropulse_DIAL_data), if not,\ncreate one for the data"
                n92 = local read "FileHour"() -> (w142:i32)
                n93 = Get Date/Time In Seconds() -> (seconds since 1Jan1904=w134:timestamp)
                n94 = Seconds To Date/Time(time stamp (now)=w134) -> (date time rec=w144:T17)  [unwired: 1 in]
                n95 = Unbundle By Name(w144) -> ("hour"=w133:i32)
                n96 = Equal?(x=w142, y=w133) -> (x = y?=w143:bool)
                n97 = case shown="True" "Reset Average" {
                  frame False {
                    n98 = local write "Index"(0 ("Index")) -> ()
                  }
                  frame True {
                    n99 = local read "Index"() -> (w238:i32)
                    n100 = Add(x=w238, y=1) -> (x+y=w237:i32)
                    n101 = local write "Index"(w237) -> ()
                  }
                }
                n102 = Format Date/Time String(time format string (%c)="%y%m%d", seconds (now)=w134) -> (date/time string=w138:string)  [unwired: 1 in]
                n103 = Concatenate Strings("Data File DIR (in)", w138, "FF" ("string")) -> (w140:string)
                n104 = Concatenate Strings("Data File DIR (in)", w138, "NF" ("string")) -> (w135:string)
                n105 = case shown="False" w143 {
                  tunnel: w140 -> [w208 _]
                  tunnel: w135 -> [w207 _]
                  tunnel: w134 -> [w194 _]
                  tunnel: w133 -> [w170 _]
                  frame False {
                    # "Adding the creation o fa netcdf file"
                    # "Are data files open?"
                    # "Within the \"E:\\Micropulse_DIAL_data...\n'Current month/day/year' \ncheck if the current hour folder exists,\nif not, create one"
                    n106 = local write "FileHour"(w170) -> ()
                    n107 = flat-sequence {
                      tunnel: [w228] -> w195
                      tunnel: w208 -> [w227]
                      tunnel: w207 -> [w228]
                      tunnel: [w227] -> w196
                      frame #0 {
                        # "Does \"E:\\Micropulse_DIAL_data...\n'Current month/day/year' exist?\nIf not, create a new folder with that name"
                        n108 = String To Path(string=w227) -> (path=w232:path)
                        n109 = String To Path(string=w228) -> (path=w230:path)
                        n110 = call <vilib>:"Check if File or Folder Exists.vi"("path"=w232) -> ("file or folder exists?"=w231:bool)  [unwired: 8 in, 2 out]
                        n111 = call <vilib>:"Check if File or Folder Exists.vi"("path"=w230) -> ("file or folder exists?"=w229:bool)  [unwired: 8 in, 2 out]
                        n112 = case shown="False" w231 {
                          tunnel: w232 -> [w234 _]
                          frame False {
                            # "create new folder"
                            n113 = Create Folder(path (use dialog)=w234) -> ()  [unwired: 2 in, 3 out]
                          }
                          frame True {
                            # "Folder exists\ndo nothing"
                          }
                        }
                        n114 = case shown="False" w229 {
                          tunnel: w230 -> [w233 _]
                          frame False {
                            # "create new folder"
                            n115 = Create Folder(path (use dialog)=w233) -> ()  [unwired: 2 in, 3 out]
                          }
                          frame True {
                            # "Folder exists\ndo nothing"
                          }
                        }
                      }
                    }
                    n116 = Concatenate Strings(w196, "\\" ("string")) -> (w203:string)
                    n117 = Concatenate Strings(w195, "\\" ("string")) -> (w198:string)
                    n118 = Format Date/Time String(time format string (%c)="%H", seconds (now)=w194) -> (date/time string=w206:string)  [unwired: 1 in]
                    n119 = Format Date/Time String(time format string (%c)="%H", seconds (now)=w194) -> (date/time string=w201:string)  [unwired: 1 in]
                    n120 = Concatenate Strings(w203, w206) -> (w166:string)
                    "File Path_Far Field (out)" <- w166
                    n121 = Concatenate Strings(w198, w201) -> (w167:string)
                    "File Path_Near Field (out)" <- w167
                    n122 = String To Path(string=w166) -> (path=w204:path)
                    n123 = String To Path(string=w167) -> (path=w199:path)
                    n124 = call <vilib>:"Check if File or Folder Exists.vi"("path"=w204) -> ("file or folder exists?"=w193:bool, "dup path"=w191:path)  [unwired: 8 in, 1 out]
                    n125 = call <vilib>:"Check if File or Folder Exists.vi"("path"=w199) -> ("file or folder exists?"=w192:bool, "dup path"=w190:path)  [unwired: 8 in, 1 out]
                    n126 = case shown="False" w193 {
                      tunnel: w191 -> [w225 _]
                      tunnel: w166 -> [w224 w226]
                      tunnel: [w224 w226] -> w165
                      frame False {
                        # "new folder"
                        n127 = Create Folder(path (use dialog)=w225) -> ()  [unwired: 2 in, 3 out]
                      }
                      frame True {
                        # "Folder exists\ndo nothing"
                      }
                    }
                    n128 = case shown="False" w192 {
                      tunnel: w190 -> [w222 _]
                      tunnel: w167 -> [w221 w223]
                      tunnel: [w221 w223] -> w147
                      frame False {
                        # "new folder"
                        n129 = Create Folder(path (use dialog)=w222) -> ()  [unwired: 2 in, 3 out]
                      }
                      frame True {
                        # "Folder exists\ndo nothing"
                      }
                    }
                    "NetCDFFilePath" <- w147
                    n130 = local read "Number of Bins"() -> (w151:u32)
                    n131 = Concatenate Strings(w147, "\\Online_Raw_Data.dat" ("string")) -> (w184:string)
                    n132 = Concatenate Strings(w147, "\\Offline_Raw_Data.dat" ("string")) -> (w183:string)
                    n133 = Concatenate Strings(w165, "\\Online_Raw_Data.dat" ("string")) -> (w189:string)
                    n134 = Concatenate Strings(w165, "\\Offline_Raw_Data.dat" ("string")) -> (w188:string)
                    n135 = local read "DataOpen"() -> (w181:bool)
                    n136 = String To Path(string=w189) -> (path=w180:path)
                    n137 = String To Path(string=w188) -> (path=w179:path)
                    n138 = String To Path(string=w184) -> (path=w178:path)
                    n139 = String To Path(string=w183) -> (path=w177:path)
                    n140 = Concatenate Strings(w147, "\\" ("string")) -> (w149:string)
                    n141 = case shown="True" w181 {
                      tunnel: w180 -> [w212 w216]
                      tunnel: [w212 w216] -> w174
                      tunnel: w179 -> [w211 w215]
                      tunnel: [w211 w215] -> w173
                      tunnel: w178 -> [w210 w214]
                      tunnel: [w210 w214] -> w172
                      tunnel: [w209 w213] -> w171
                      tunnel: w177 -> [w209 w213]
                      frame False {
                        # "No files open\ndo nothing"
                      }
                      frame True {
                        # "Close open files"
                        n142 = local read "NF_Off_Ref"() -> (w218:refnum<file>)
                        n143 = local read "NF_On_Ref"() -> (w217:refnum<file>)
                        n144 = local read "FF_Off_Ref"() -> (w220:refnum<file>)
                        n145 = local read "FF_On_Ref"() -> (w219:refnum<file>)
                        n146 = Close File(refnum=w219) -> ()  [unwired: 1 in, 2 out]
                        n147 = Close File(refnum=w220) -> ()  [unwired: 1 in, 2 out]
                        n148 = Close File(refnum=w217) -> ()  [unwired: 1 in, 2 out]
                        n149 = Close File(refnum=w218) -> ()  [unwired: 1 in, 2 out]
                      }
                    }
                    n150 = call "DefineNetCDFFile.vi"("BaseFilePath"=w149, "AltitudeBins"=w151, "WVDialNumber"="WVDialNumber") -> ("BaseName"=→"NetCDFFileName":string)  [unwired: 14 in, 2 out]
                    n151 = Open/Create/Replace File(file path (use dialog)=w174, operation (0:open)=T14."open or create") -> (refnum out=w161:refnum<file>)  [unwired: 4 in, 2 out]
                    n152 = Open/Create/Replace File(file path (use dialog)=w173, operation (0:open)=T14."open or create") -> (refnum out=w162:refnum<file>)  [unwired: 4 in, 2 out]
                    n153 = Open/Create/Replace File(file path (use dialog)=w172, operation (0:open)=T14."open or create") -> (refnum out=w163:refnum<file>)  [unwired: 4 in, 2 out]
                    n154 = Open/Create/Replace File(file path (use dialog)=w171, operation (0:open)=T14."open or create") -> (refnum out=w164:refnum<file>)  [unwired: 4 in, 2 out]
                    n155 = Get File Size(file=w161) -> (refnum out=→"FF_On_Ref":refnum<file>, size (in bytes)=→"FF_On_Ptr":i64)  [unwired: 1 in, 1 out]
                    n156 = Get File Size(file=w162) -> (refnum out=→"FF_Off_Ref":refnum<file>, size (in bytes)=→"FF_Off_Ptr":i64)  [unwired: 1 in, 1 out]
                    n157 = Get File Size(file=w163) -> (refnum out=→"NF_On_Ref":refnum<file>, size (in bytes)=→"NF_On_Ptr":i64)  [unwired: 1 in, 1 out]
                    n158 = Get File Size(file=w164) -> (refnum out=→"NF_Off_Ref":refnum<file>, size (in bytes)=→"NF_Off_Ptr":i64)  [unwired: 1 in, 1 out]
                    "NetCDFEntry" <- 1
                  }
                  frame True {
                    # "Don't need to do anything!"
                  }
                }
              }
              frame #1 {
                # "Writing and plotting retrieved\nweather parameters"
                # "Matlab script goes online and retrieves most recent press, temp, and relative humidity data \nfrom the weather station on the roof of Cobleigh"
                # "Importing the current weather conditions from the COE weather station"
                n159 = disable-structure shown="Disabled" {
                  frame Disabled {
                    n160 = script code="%try\n%s=urlread('http://www.coe.montana.edu/ee/weather/mostCurrentCSV.php');\n%amin=textscan(s,'%s %s %s %s %s %s %s %s %s %s %s %s %s');\n%data=amin{1}{2};\n%[test remain]=strtok(data,',');\n%remain=str2num(remain);\n%press=remain(3)./1000;\n%temp=remain(5);\n%RH=remain(7);\n%catch\npress=.850;\ntemp=20;\nRH=40;\n%end"() -> ()  [unwired: 1 in, 4 out]
                  }
                  frame Enabled {
                  }
                }
                n161 = local read "WS_On/Off"() -> (w239:bool)
                n162 = case shown="True" w239 {
                  frame False {
                  }
                  frame True {
                    n163 = local read "WS visa"() -> (w247:refnum<visa-resource-name>)
                    n164 = local read "WeatherStation"() -> (w244:T11)
                    n165 = call "T_RH_P.vi"("VISA in"=w247, "WS_Commands"=enum16{"OpenWS", "ReadTRHP", "CloseWS"}."ReadTRHP") -> ("TRHP"=w246:T16)  [unwired: 11 in, 2 out]
                    n166 = local write "TRHP"(w246) -> ()
                    n167 = Unbundle By Name(w246) -> ("Temp"=w241:dbl, "RelH"=w242:dbl, "Press"=w243:dbl, "AbH"=w240:dbl)
                    "Temperature (C)" <- w241
                    "Pressure (mb)" <- w243
                    "Relative Humdity (%)" <- w242
                    n168 = Bundle By Name(cluster=w244, "Pressure"=w243, "RelativeHumidity"=w242, "Temperature"=w241, "AbsoluteHumidity"=w240) -> (→"WeatherStation":T11)
                  }
                }
              }
              frame #2 {
                # "Frame 3: Read, process, and plot online data\nFrame 4:\nFrame 5: Write the data to the folders from Frame 0 of outter sequence"
                # "Frame 0: Read the online wavelength and adjust to locking tolerance if out of range, Switch to offline DBR\nFrame 1: Read the output power from the Newport meter, calculate and plot the output pulse energy\nFrame 2: Wait 'Scalar Wait Time' for buffer to clear other wavelength data"
                # "Online"
                n169 = stacked-sequence {
                  frame #0 {
                    # "Read the online wavelength and continue adjusting the online DBR if outside the wavelength tolerance\nuntil it is within tolerance"
                    n170 = while {
                      i -> [w250]
                      stop <- w249 stop-if-true
                      # "Frame 2: Decrement DBR current if above tolerance\nFrame 3: Increment DBR current if below tolerance"
                      # "Frame 0: Read the current wavelength from the wavemeter\nFrame 1: Calculate the difference between desired and actual wavelength"
                      # "Continue reading and adjusting online DBR current until within locking tolerance"
                      n171 = stacked-sequence {
                        tunnel: w250 -> [w252 _ _ _ _]
                        tunnel: [_ _ w268 _ _] -> w249
                        frame #0 {
                          n172 = Equal To 0?(x=w252) -> (x = 0?=w251:bool)
                          n173 = case shown="True" w251 {
                            frame False {
                            }
                            frame True {
                              # "Set the wavemeter switch to WV Online"
                              n174 = flat-sequence {
                                frame #0 {
                                n175 = Build Array(FALSE ("Boolean")) -> (w255:bool[])
                                n176 = call-poly <vilib>:"DAQmx Write.vi"("task/channels in"=refnum<k21> "BristolWM", "data"=w255) -> ()  [unwired: 11 in, 3 out]
                                }
                                frame #1 {
                                n177 = Build Array(FALSE ("Boolean")) -> (w258:bool[])
                                n178 = call-poly <vilib>:"DAQmx Write.vi"("task/channels in"=refnum<k21> "HSRL_WV_switch", "data"=w258) -> ()  [unwired: 11 in, 3 out]
                                }
                              }
                            }
                          }
                        }
                        frame #1 {
                          # "Reading the wavelength from the wavemeter"
                          n179 = flat-sequence {
                            tunnel: [w261] -> w260
                            tunnel: w260 -> [w264]
                            tunnel: [w263] -> w259
                            tunnel: w259 -> [w267]
                            frame #0 {
                              n180 = local read "Bristol In"() -> (w262:i32)
                              n181 = dll-call lib="C:/Users/eol-lidar/Desktop/20171016_WVDIALLabviewSlimmed/DLLs/CLDevIface.dll" fn="CLOpenUSBSerialDevice"("commPort"=w262) -> ("return type"=w261:i32)  [unwired: 4 in, 2 out]
                            }
                            frame #1 {
                              n182 = dll-call lib="C:/Users/eol-lidar/Desktop/20171016_WVDIALLabviewSlimmed/DLLs/CLDevIface.dll" fn="CLGetLambdaReading"("devHandle"=w264) -> ("return type"=→"WV Online Read (nm)":dbl, "devHandle"=w263:i32)  [unwired: 3 in, 2 out]
                            }
                            frame #2 {
                              n183 = dll-call lib="C:/Users/eol-lidar/Desktop/20171016_WVDIALLabviewSlimmed/DLLs/CLDevIface.dll" fn="CLCloseDevice"("commPort"=w267) -> ("return type"=w266:i32)  [unwired: 4 in, 2 out]
                              n184 = local write "Bristol Out"(w266) -> ()
                            }
                          }
                        }
                        frame #2 {
                          # "If WL difference is within tolerance, stop looping, and illuminate 'Wavelength Lock Online' indicator"
                          # "Calculating the difference between the actual and desired online wavelength"
                          n185 = local read "WV Online Read (nm)"() -> (w271:dbl)
                          n186 = local read "Online_Tol"() -> (w276:dbl)
                          n187 = Multiply(x=-1.0, y=w276) -> (x*y=w277:dbl)
                          n188 = Subtract(x=w271, y="WV Online Set (nm)") -> (x-y=w272:dbl)
                          "Online_Diff" <- w272
                          n189 = Greater?(x=w272, y=w277) -> (0:w273:bool)
                          n190 = Less?(x=w272, y=w276) -> (x < y?=w274:bool)
                          n191 = And(x=w273, y=w274) -> (x .and. y?=w270:bool)
                          "WV Online Locked" <- w270
                          n192 = Or(x=w270, y="Cancel online") -> (x .or. y?=w268:bool)
                        }
                        frame #3 {
                          # "If the wavelength difference is greater that 0.0002 nm, decrement the \nDBR current by 0.01 mA"
                          n193 = local read "Online_Diff"() -> (w281:dbl)
                          n194 = Greater Or Equal?(x=w281, y="Online_Tol") -> (x >= y?=w280:bool)
                          n195 = case shown="True" w280 {
                            frame False {
                              # "Wavelength difference is not greater than 0.0002 nm, do nothing"
                            }
                            frame True {
                              # "Generating a command string\nto decrement the current"
                              # "WL difference is greater than 0.0002 nm,\ndecrement the DBR current by 0.01 mA"
                              n196 = local read "Settings"() -> (w288:T6)
                              n197 = local read "temp step size"() -> (w283:dbl)
                              n198 = Unbundle By Name(w288) -> ("WV Online TEC"=w287:dbl)
                              n199 = local read "Device In"() -> (w284:refnum<visa-resource-name>)
                              n200 = Subtract(x=w287, y=w283) -> (x-y=w286:dbl)
                              n201 = Bundle By Name(cluster=w288, "WV Online TEC"=w286, "Module"=T15."WV Online TEC") -> (w290:T6)
                              n202 = call "TL_Driver_v2.vi"("Device In"=w284, "Commands"=T12."SET", "Settings"=w290) -> ("Readings"=w289:T7)  [unwired: 9 in, 3 out]
                              n203 = local write "Settings"(w290) -> ()
                              n204 = local write "Readings"(w289) -> ()
                            }
                          }
                        }
                        frame #4 {
                          # "If WL difference is < 0.0002 nm, increment the DBR current"
                          n205 = local read "Online_Tol"() -> (w292:dbl)
                          n206 = local read "Online_Diff"() -> (w295:dbl)
                          n207 = Multiply(x=-1.0, y=w292) -> (x*y=w291:dbl)
                          n208 = Less Or Equal?(x=w295, y=w291) -> (x <= y?=w294:bool)
                          n209 = case shown="True" w294 {
                            frame False {
                              # "WL difference is no <= to -0.0002 nm, do nothing"
                            }
                            frame True {
                              # "WL difference is < -0.0002,\nincrement the DBR current by 0.01 mA"
                              # "Generating a command string\nto decrement the current"
                              n210 = local read "Settings"() -> (w304:T6)
                              n211 = local read "temp step size"() -> (w297:dbl)
                              n212 = Unbundle By Name(w304) -> ("WV Online TEC"=w301:dbl)
                              n213 = local read "Device In"() -> (w298:refnum<visa-resource-name>)
                              n214 = Add(x=w301, y=w297) -> (x+y=w300:dbl)
                              n215 = Bundle By Name(cluster=w304, "WV Online TEC"=w300, "Module"=T15."WV Online TEC") -> (w303:T6)
                              n216 = call "TL_Driver_v2.vi"("Device In"=w298, "Commands"=T12."SET", "Settings"=w303) -> ("Readings"=w302:T7)  [unwired: 9 in, 3 out]
                              n217 = local write "Settings"(w303) -> ()
                              n218 = local write "Readings"(w302) -> ()
                            }
                          }
                        }
                      }
                    }
                  }
                  frame #1 {
                    # "Converting to pulse energy, assumes 5 percent pickoff"
                    # "Reading the Newport Power meter"
                    # "Reading the output power of the laser transmitter from the Newport power meter, once read, convert to corresponding pulse energy and plot"
                    n219 = local read "Newport Device Key"() -> (w313:string)
                    n220 = local read "NewportRef"() -> (w309:refnum<k24>)
                    n221 = disable-structure shown="Enabled" {
                      frame Enabled {
                        # "Plotting the online and offling pulse energies"
                        n222 = local read "WV Online Pulse Energy"() -> (w325:dbl)
                        n223 = local read "WV Offline Pulse Energy"() -> (w321:dbl)
                        n224 = local read "HSRL Pulse Energy"() -> (w324:dbl)
                        n225 = local read "WV_averaged_energy"() -> (w322:dbl)
                        n226 = Bundle("WV Online Pulse Energy"=w325, "WV Offline Pulse Energy"=w321, "HSRL Pulse Energy"=w324, "WV_averaged_energy"=w322) -> (→"Pulse Energy (Micro Joule)":T18)  [unwired: 1 in]
                      }
                      frame Disabled {
                      }
                    }
                    n227 = Number To Decimal String(number="SampleSize") -> (decimal integer string=w311:string)  [unwired: 1 in]
                    n228 = invoke class="PowerMeterCommands" method="PerformDAQ"(reference=w309, "deviceKey"=w313, "interval"="1", "sampleSize"=w311) -> ("PerformDAQ"=w314:dbl[])  [unwired: 2 in, 5 out]
                    n229 = call-poly <vilib>:"Mean.vi"("X"=w314) -> ("mean"=w312:dbl)  [unwired: 1 out]
                    n230 = Multiply(x=w312, y=1000.0) -> (x*y=w319:dbl)
                    n231 = Divide(x=w319, y=0.05) -> (x/y=w317:dbl)
                    n232 = global read "AMCS_Data.vi" "AMCS_PowerMon"() -> (w307:u32[])
                    n233 = Divide(x=w317, y=7.0) -> (x/y=→"WV_averaged_energy":dbl)
                    n234 = Index Array(array=w307, index=1) -> (element=→"WV Online Pulse Energy":u32)
                  }
                  frame #2 {
                    # "Wait 'Scalar Wait Time' for the next available batch of scalar card data"
                    n235 = local read "AMCS_Profile"() -> (w326:i32)
                    n236 = disable-structure shown="Disabled" {
                      frame Disabled {
                        # "Waiting 'Scalar Wait Time'"
                        n237 = Wait (ms)(milliseconds to wait="Scalar Wait Time") -> ()  [unwired: 1 out]
                      }
                      frame Enabled {
                      }
                    }
                    n238 = while {
                      tunnel: [w333] -> w327
                      tunnel: [w329] -> _
                      tunnel: w326 -> [w329]
                      stop <- w331 stop-if-true
                      n239 = global read "AMCS_Data.vi" "AMCS_Profile"() -> (w333:i32)
                      n240 = Wait (ms)(milliseconds to wait=u32 10) -> ()  [unwired: 1 out]
                      n241 = Equal?(x=w333, y=w329) -> (x = y?=w332:bool)
                      n242 = case shown="False" w332 {
                        tunnel: [TRUE FALSE] -> w331
                        frame False {
                        }
                        frame True {
                        }
                      }
                    }
                    "AMCS_Profile" <- w327
                  }
                  frame #3 {
                    # "convert time per range bin to meters\nand calculate smoothed bins using\nsmoothing range"
                    # "Plotting online cross section and smoothed online data"
                    # "Calculate the bin by bin mean of the data"
                    # "Collect 'Integration Period (Seconds)' number\nof scalar data"
                    # "Reading, processing, and plotting the online data"
                    n243 = local read "Data Reads (number of loops)"() -> (w337:i32)
                    n244 = local read "bins"() -> (w336:u32)
                    n245 = for {
                      N: w337 -> [_]
                      tunnel: [w391] -> w377 mode=indexing
                      tunnel: [w386] -> w342 mode=indexing
                      tunnel: w336 -> [w385]
                      # "Scalar Data is retrieved from Global \nVariable that scaler.vi is writing to,"
                      n246 = global read "AMCS_Data.vi" "AMCS_Data"() -> (w394:u16[][])
                      n247 = disable-structure shown="Disabled" {
                        frame Disabled {
                          n248 = global read "Scalar_Data_3.vi" "Scalar Data 3"() -> ()  [unwired: 1 out]
                          n249 = global read "Scalar_Data.vi" "Scalar Data"() -> ()  [unwired: 1 out]
                        }
                        frame Enabled {
                        }
                      }
                      n250 = Index Array(array=w394, index (row) #1=0 ("index (row)"), index (row) #2=2 ("index (row)")) -> (element #1=w390:u16[], element #2=w388:u16[])  [unwired: 2 in]
                      n251 = Array Subset(array=w390, index=0, length=w385) -> (w391:u16[])
                      n252 = Array Subset(array=w388, index=0, length=w385) -> (w386:u16[])
                    }
                    n253 = Transpose 2D Array(2D array=w377) -> (transposed array=w381:u16[][])
                    n254 = Transpose 2D Array(2D array=w342) -> (transposed array=w364:u16[][])
                    n255 = for {
                      tunnel: w364 -> [w384] mode=indexing
                      tunnel: [w383] -> w365 mode=indexing
                      n256 = call-poly <vilib>:"Mean.vi"("X"=w384) -> ("mean"=w383:dbl)  [unwired: 1 out]
                    }
                    n257 = for {
                      tunnel: w381 -> [w396] mode=indexing
                      tunnel: [w395] -> w382 mode=indexing
                      n258 = call-poly <vilib>:"Mean.vi"("X"=w396) -> ("mean"=w395:dbl)  [unwired: 1 out]
                    }
                    n259 = Array Subset(array=w382, index=1 ("dimension size"), length=w336) -> (w369:dbl[])
                    n260 = Array Subset(array=w365, index=1 ("dimension size"), length=w336) -> (w362:dbl[])
                    n261 = local read "background length"() -> (w349:i32)
                    n262 = local read "background start"() -> (w350:u32)
                    n263 = Array Size(array=w369) -> (size(s)=w366:i32)
                    n264 = Array Size(array=w362) -> (size(s)=w359:i32)
                    n265 = Initialize Array(1.0 ("element"), w366) -> (w368:dbl[])
                    n266 = Initialize Array(1.0 ("element"), w359) -> (w361:dbl[])
                    n267 = Multiply(x=w369, y=w368) -> (x*y=w370:dbl[])
                    "CH 0 Bin Readings" <- w370
                    n268 = Multiply(x=w362, y=w361) -> (x*y=w353:dbl[])
                    "CH 2 Bin Readings" <- w353
                    n269 = local read "Total DIAL Integration Time (Minutes)"() -> (w373:i32)
                    n270 = local read "Total Aerosol Integration Time (Minutes)"() -> (w339:dbl)
                    n271 = local read "Time Resolution Per Bin(ns)"() -> (w345:u32)
                    n272 = Array Subset(array=w370, index=w350, length=w349) -> (w379:dbl[])
                    n273 = Array Subset(array=w353, index=w350, length=w349) -> (w355:dbl[])
                    n274 = Divide(x=w339, y=w337) -> (x/y=w340:dbl)
                    n275 = call-poly <vilib>:"Mean.vi"("X"=w379) -> ("mean"=w378:dbl)  [unwired: 1 out]
                    n276 = Multiply(x=w340, y=60.0) -> (x*y=w338:dbl)
                    n277 = call-poly <vilib>:"Mean.vi"("X"=w355) -> ("mean"=w356:dbl)  [unwired: 1 out]
                    n278 = Divide(x=w373, y=w337) -> (x/y=w371:dbl)
                    n279 = local read "Index"() -> (w354:i32)
                    n280 = Subtract(x=w370, y=w378) -> (x-y=w375:dbl[])
                    n281 = Subtract(x=w353, y=w356) -> (x-y=w357:dbl[])
                    n282 = Multiply(x=w371, y=60.0) -> (x*y=w351:dbl)
                    n283 = To Double Precision Float(number=w345) -> (double precision float=w346:dbl)
                    n284 = Multiply(x=w346, y=0.15) -> (x*y=w348:dbl)
                    n285 = call "Ring Buffer CH2 rev2.vi"("Index"=w354, "Profiles to Average"=w338, "Input Array"=w357) -> ("AvgArray"=w358:dbl[])  [unwired: 7 in, 1 out]
                    n286 = call "Ring Buffer CH0 rev2.vi"("Index"=w354, "Profiles to Average"=w351, "Input Array"=w375) -> ("AvgArray"=w374:dbl[])  [unwired: 7 in, 1 out]
                    n287 = Divide(x="Smoothing Range", y=w348) -> (x/y=w343:dbl)
                    "Smoothed Bins" <- w343
                    n288 = call "Smooth Arrray.vi"("smooth size"=w343, "Raw Array"=w374) -> ("Smoothed Array"=→"CH0 (WV on) smoothed":dbl[])  [unwired: 9 in]
                    n289 = call "Smooth Arrray.vi"("smooth size"=w343, "Raw Array"=w358) -> ("Smoothed Array"=→"CH2 (molecular) smoothed":dbl[])  [unwired: 9 in]
                    n290 = disable-structure shown="Disabled" {
                      frame Disabled {
                        n291 = script code="format long;\ncounts=sum(Online);\nif counts >=0.5e6\ntime=time;\nelse\ntime=time\nend"() -> ()  [unwired: 3 in, 2 out]
                      }
                      frame Enabled {
                      }
                    }
                  }
                  frame #4 {
                    # "Toggling the Agiltron switch to the offline DBR seed laser"
                    n292 = disable-structure shown="Disabled" {
                      frame Disabled {
                        n293 = flat-sequence {
                          frame #0 {
                            # "Second one"
                            # "Command the switch to switch to position 2\ncorresponding to the offline DBR"
                            # "Hex string command \ncorrespond to offline"
                            n294 = VISA Write(VISA resource name="Switch Comm Port", write buffer="\u0001\u0012\u0000\u0001") -> ()  [unwired: 1 in, 3 out]
                          }
                        }
                      }
                      frame Enabled {
                      }
                    }
                  }
                  frame #5 {
                    # "Save the recently collected online data if 'Save Data?' is true"
                    n295 = case shown="True" "Save Data?" {
                      frame False {
                        # "'Save Data?' is false, do nothing"
                      }
                      frame True {
                        # "'Save Data?' is true, save onfline data to the Data Disk"
                        # "Write only one copy of data at this time"
                        # "Retrieve Julian Date"
                        n296 = local write "DataOpen"(TRUE ("DataOpen")) -> ()
                        n297 = local read "Readings"() -> (w415:T7)
                        n298 = local read "Time Resolution Per Bin(ns)"() -> (w421:u32)
                        n299 = Unbundle By Name(w415) -> ("WV OnLine TEC"=w408:dbl)
                        n300 = local read "Number of Accumulates"() -> (w419:u32)
                        n301 = Unbundle By Name(w415) -> ("HSRL TEC"=w401:dbl)
                        n302 = local read "Number of Bins"() -> (w420:u32)
                        n303 = local read "WV_averaged_energy"() -> (w403:dbl)
                        n304 = local read "HSRL Read (nm)"() -> (w400:dbl)
                        n305 = local read "WV Online Read (nm)"() -> (w406:dbl)
                        n306 = local read "WV Online Pulse Energy"() -> (w407:dbl)
                        n307 = local read "CH 0 Bin Readings"() -> (w442:dbl[])
                        n308 = To Double Precision Float(number=w421) -> (double precision float=w416:dbl)
                        n309 = To Double Precision Float(number=w420) -> (double precision float=w417:dbl)
                        n310 = To Double Precision Float(number=w419) -> (double precision float=w418:dbl)
                        n311 = local read "CH 2 Bin Readings"() -> (w404:dbl[])
                        n312 = call "Julian_Date_2.vi"() -> ("Julian Date"=w441:dbl)  [unwired: 11 in]
                        n313 = local read "H2ODIAL"() -> (w413:T9)
                        n314 = local read "CH 0 Bin Readings"() -> (w409:dbl[])
                        n315 = Build Array (concatenate)(w441, w406, w408, w407, w416, w417, w418, w442) -> (w436:dbl[])
                        n316 = Build Array (concatenate)(w441, w400, w401, w403, w416, w417, w418, w404) -> (w426:dbl[])
                        n317 = local read "NF_On_Ref"() -> (w424:refnum<file>)
                        n318 = local read "FF_On_Ref"() -> (w440:refnum<file>)
                        n319 = local read "NF_On_Ptr"() -> (w425:i64)
                        n320 = local read "FF_On_Ptr"() -> (w439:i64)
                        n321 = local read "HSRL"() -> (w405:T10)
                        n322 = Bundle By Name(cluster=w405, "HSRLMolecularCounts"=w404, "HSRLTEC"=w401, "HSRLWavelength"=w400) -> (→"HSRL":T10)
                        n323 = Index Array(array=w413, index="OnlinIndex") -> (element=w414:T19)
                        n324 = Bundle By Name(cluster=w414, "DIALCounts"=w409, "DIALEnergy"=w407, "DIALTEC"=w408, "DIALWavelength"=w406) -> (w410:T19)
                        n325 = Set File Position(offset (in bytes) (0)=w439, refnum=w440) -> (refnum out=w437:refnum<file>, error out=w434:errorcluster)  [unwired: 2 in]
                        n326 = Set File Position(offset (in bytes) (0)=w425, refnum=w424) -> (refnum out=w430:refnum<file>, error out=w428:errorcluster)  [unwired: 2 in]
                        n327 = Write to Binary File(file (use dialog)=w430, data=w426, error in=w428, 5:FALSE ("prepend array or string size? (T)")) -> (refnum out=w429:refnum<file>, error out=w427:errorcluster)  [unwired: 2 in, 1 out]
                        n328 = Write to Binary File(file (use dialog)=w437, data=w436, error in=w434, 5:FALSE ("prepend array or string size? (T)")) -> (refnum out=w435:refnum<file>, error out=w433:errorcluster)  [unwired: 2 in, 1 out]
                        n329 = Replace Array Subset(array=w413, new element=w410, index="OnlinIndex") -> (→"H2ODIAL":T9)
                        n330 = Get File Position(4:w427, 7:w429) -> (2:w423:i64)  [unwired: 2 out]
                        n331 = Get File Position(4:w433, 7:w435) -> (2:w432:i64)  [unwired: 2 out]
                        n332 = local write "NF_On_Ptr"(w423) -> ()
                        n333 = local write "FF_On_Ptr"(w432) -> ()
                      }
                    }
                  }
                }
              }
              frame #3 {
                # "Frame 3: Read offline data, calculate aerosol data, and plot offline and normalized relative backscatter\nFrame 4:\nFrame 5: Save the offline data and related information"
                # "Frame 0: Read the offline wavelength and lock if necessary, Switch to online DBR\nFrame 1: Read the output power from the Newport power meter\nFrame 2: Wait 'Scalar Wait Time' for buffers to clear of online contiminated data"
                # "offline"
                n334 = stacked-sequence {
                  frame #0 {
                    # "Following Locking the Offline wavelength, check and lock the HSRL 780 nm wavelength"
                    # "Every 60 data collection cycles, read the offline DBR wavelength, and if outside of wavelength tolerance, adjust DBR current until within tolerance"
                    n335 = local read "L_Count"() -> (w444:i32)
                    n336 = Quotient & Remainder(x=w444, y=60.0) -> (x-y*floor(x/y)=w445:dbl)  [unwired: 1 out]
                    n337 = Equal To 0?(x=w445) -> (x = 0?=w443:bool)
                    n338 = case shown="True" w443 {
                      frame False {
                      }
                      frame True {
                        n339 = flat-sequence {
                          frame #0 {
                            n340 = while {
                              i -> [w450]
                              stop <- w448 stop-if-true
                              # "If WL difference is within tolerance, stop looping, and illuminate 'Wavelength Lock Offline' indicator"
                              # "Frame 2: Decrement DBR if above tolerance\nFrame 3: Increment DBR if below tolerance"
                              # "Frame 0: Read the wavelength from the wavemeter\nFrame 1: Calculate the difference between desired and actual wavelength"
                              # "Continue reading and adjusting offline DBR until within locking tolerance"
                              n341 = stacked-sequence {
                                tunnel: w450 -> [w452 _ _ _ _]
                                tunnel: [_ _ w466 _ _] -> w447
                                frame #0 {
                                n342 = Equal To 0?(x=w452) -> (x = 0?=w451:bool)
                                n343 = case shown="True" w451 {
                                frame False {
                                }
                                frame True {
                                # "Set the TSOA switch to\namplify the offline wavelength"
                                n344 = Build Array(TRUE ("Boolean")) -> (w454:bool[])
                                n345 = call-poly <vilib>:"DAQmx Write.vi"("task/channels in"=refnum<k21> "BristolWM", "data"=w454) -> ()  [unwired: 11 in, 3 out]
                                n346 = Wait (ms)(milliseconds to wait=u32 3200) -> ()  [unwired: 1 out]
                                }
                                }
                                }
                                frame #1 {
                                # "Reading the wavelength from the wavemeter"
                                n347 = flat-sequence {
                                tunnel: [w459] -> w458
                                tunnel: w458 -> [w462]
                                tunnel: [w461] -> w457
                                tunnel: w457 -> [w465]
                                frame #0 {
                                n348 = local read "Bristol In"() -> (w460:i32)
                                n349 = dll-call lib="C:/Users/eol-lidar/Desktop/20171016_WVDIALLabviewSlimmed/DLLs/CLDevIface.dll" fn="CLOpenUSBSerialDevice"("commPort"=w460) -> ("return type"=w459:i32)  [unwired: 4 in, 2 out]
                                }
                                frame #1 {
                                n350 = dll-call lib="C:/Users/eol-lidar/Desktop/20171016_WVDIALLabviewSlimmed/DLLs/CLDevIface.dll" fn="CLGetLambdaReading"("devHandle"=w462) -> ("return type"=→"WV Offline Read (nm)":dbl, "devHandle"=w461:i32)  [unwired: 3 in, 2 out]
                                }
                                frame #2 {
                                n351 = dll-call lib="C:/Users/eol-lidar/Desktop/20171016_WVDIALLabviewSlimmed/DLLs/CLDevIface.dll" fn="CLCloseDevice"("commPort"=w465) -> ("return type"=w464:i32)  [unwired: 4 in, 2 out]
                                n352 = local write "Bristol Out"(w464) -> ()
                                }
                                }
                                }
                                frame #2 {
                                # "Calculating the difference between the actual and desired online wavelength"
                                n353 = local read "Offline_Tol"() -> (w468:dbl)
                                n354 = local read "WV Offline Read (nm)"() -> (w474:dbl)
                                n355 = Multiply(x=-1.0, y=w468) -> (x*y=w467:dbl)
                                n356 = Subtract(x=w474, y="WV Offline Set (nm)") -> (x-y=w470:dbl)
                                "Oflline_Diff" <- w470
                                n357 = Greater?(x=w470, y=w467) -> (0:w471:bool)
                                n358 = Less?(x=w470, y=w468) -> (x < y?=w472:bool)
                                n359 = And(x=w471, y=w472) -> (x .and. y?=w466:bool)
                                "WV Oflline Locked" <- w466
                                n360 = case shown="True" w466 {
                                frame False {
                                }
                                frame True {
                                # "Set the Wavemeter switch to\nthe HSRL wavelength"
                                n361 = Build Array(TRUE ("Boolean")) -> (w476:bool[])
                                n362 = call-poly <vilib>:"DAQmx Write.vi"("task/channels in"=refnum<k21> "HSRL_WV_switch", "data"=w476) -> ()  [unwired: 11 in, 3 out]
                                n363 = Wait (ms)(milliseconds to wait=u32 3200) -> ()  [unwired: 1 out]
                                }
                                }
                                }
                                frame #3 {
                                # "If the wavelength difference is greater that 0.0002 nm, decrement the \nDBR current by 0.01 mA"
                                n364 = local read "Oflline_Diff"() -> (w481:dbl)
                                n365 = Greater Or Equal?(x=w481, y="Offline_Tol") -> (x >= y?=w480:bool)
                                n366 = case shown="True" w480 {
                                frame False {
                                # "Wavelength difference is not greater than 0.0002 nm, do nothing"
                                }
                                frame True {
                                # "Generating a command string\nto decrement the current"
                                n367 = local read "Settings"() -> (w488:T6)
                                n368 = Unbundle By Name(w488) -> ("WV Offline TEC"=w486:dbl)
                                n369 = Subtract(x=w486, y="temp step size") -> (x-y=w485:dbl)
                                n370 = local read "Device In"() -> (w483:refnum<visa-resource-name>)
                                n371 = Bundle By Name(cluster=w488, "WV Offline TEC"=w485, "Module"=T15."WV Offline TEC") -> (w489:T6)
                                n372 = call "TL_Driver_v2.vi"("Device In"=w483, "Commands"=T12."SET", "Settings"=w489) -> ("Readings"=w490:T7)  [unwired: 9 in, 3 out]
                                n373 = local write "Settings"(w489) -> ()
                                n374 = local write "Readings"(w490) -> ()
                                }
                                }
                                }
                                frame #4 {
                                # "If WL difference is < 0.0002 nm, increment the DBR temperature"
                                n375 = local read "Oflline_Diff"() -> (w493:dbl)
                                n376 = Less Or Equal?(x=w493, y=-0.0001) -> (x <= y?=w491:bool)
                                n377 = case shown="True" w491 {
                                frame False {
                                # "WL difference is no <= to -0.0002 nm, do nothing"
                                }
                                frame True {
                                # "Generating a command string\nto decrement the current"
                                # "WL difference is less than 0.0002 nm,\nincrement the DBR current by 0.01 mA"
                                n378 = local read "Settings"() -> (w501:T6)
                                n379 = Unbundle By Name(w501) -> ("WV Offline TEC"=w499:dbl)
                                n380 = local read "temp step size"() -> (w495:dbl)
                                n381 = Add(x=w499, y=w495) -> (x+y=w498:dbl)
                                n382 = local read "Device In"() -> (w496:refnum<visa-resource-name>)
                                n383 = Bundle By Name(cluster=w501, "WV Offline TEC"=w498, "Module"=T15."WV Offline TEC") -> (w502:T6)
                                n384 = call "TL_Driver_v2.vi"("Device In"=w496, "Commands"=T12."SET", "Settings"=w502) -> ("Readings"=w500:T7)  [unwired: 9 in, 3 out]
                                n385 = local write "Settings"(w502) -> ()
                                n386 = local write "Readings"(w500) -> ()
                                }
                                }
                                }
                              }
                              n387 = Or(x=w447, y="Cancel Offline") -> (x .or. y?=w448:bool)
                            }
                          }
                          frame #1 {
                            n388 = while {
                              i -> [w506]
                              stop <- w504 stop-if-true
                              # "If WL difference is within tolerance, stop looping, and illuminate 'Wavelength Lock Offline' indicator"
                              # "Frame 2: Decrement DBR if above tolerance\nFrame 3: Increment DBR if below tolerance"
                              # "Frame 0: Read the wavelength from the wavemeter\nFrame 1: Calculate the difference between desired and actual wavelength"
                              # "Continue reading and adjusting offline DBR until within locking tolerance"
                              n389 = stacked-sequence {
                                tunnel: w506 -> [w508 _ _ _ _]
                                tunnel: [_ _ w521 _ _] -> w503
                                frame #0 {
                                n390 = Equal To 0?(x=w508) -> (x = 0?=w507:bool)
                                n391 = case shown="True" w507 {
                                frame False {
                                }
                                frame True {
                                # "Set the Wavemeter to\nthe non HSRL wavelength"
                                n392 = Build Array(TRUE ("Boolean")) -> (w509:bool[])
                                n393 = call-poly <vilib>:"DAQmx Write.vi"("task/channels in"=refnum<k21> "HSRL_WV_switch", "data"=w509) -> ()  [unwired: 11 in, 3 out]
                                }
                                }
                                }
                                frame #1 {
                                # "Reading the wavelength from the wavemeter"
                                n394 = flat-sequence {
                                tunnel: [w514] -> w513
                                tunnel: w513 -> [w517]
                                tunnel: [w516] -> w512
                                tunnel: w512 -> [w520]
                                frame #0 {
                                n395 = local read "Bristol In"() -> (w515:i32)
                                n396 = dll-call lib="C:/Users/eol-lidar/Desktop/20171016_WVDIALLabviewSlimmed/DLLs/CLDevIface.dll" fn="CLOpenUSBSerialDevice"("commPort"=w515) -> ("return type"=w514:i32)  [unwired: 4 in, 2 out]
                                }
                                frame #1 {
                                n397 = dll-call lib="C:/Users/eol-lidar/Desktop/20171016_WVDIALLabviewSlimmed/DLLs/CLDevIface.dll" fn="CLGetLambdaReading"("devHandle"=w517) -> ("return type"=→"HSRL Read (nm)":dbl, "devHandle"=w516:i32)  [unwired: 3 in, 2 out]
                                }
                                frame #2 {
                                n398 = dll-call lib="C:/Users/eol-lidar/Desktop/20171016_WVDIALLabviewSlimmed/DLLs/CLDevIface.dll" fn="CLCloseDevice"("commPort"=w520) -> ("return type"=w519:i32)  [unwired: 4 in, 2 out]
                                n399 = local write "Bristol Out"(w519) -> ()
                                }
                                }
                                }
                                frame #2 {
                                # "Calculating the difference between the actual and desired online wavelength"
                                n400 = local read "HSRL_Tol"() -> (w523:dbl)
                                n401 = local read "HSRL Read (nm)"() -> (w529:dbl)
                                n402 = Multiply(x=-1.0, y=w523) -> (x*y=w522:dbl)
                                n403 = Subtract(x=w529, y="HSRL Set (nm)") -> (x-y=w525:dbl)
                                "HSRL_Diff" <- w525
                                n404 = Greater?(x=w525, y=w522) -> (0:w526:bool)
                                n405 = Less?(x=w525, y=w523) -> (x < y?=w527:bool)
                                n406 = And(x=w526, y=w527) -> (x .and. y?=w521:bool)
                                "HSRL Locked" <- w521
                                n407 = case shown="True" w521 {
                                frame False {
                                }
                                frame True {
                                # "Set the Wavementer switch to WV Online"
                                n408 = Build Array(FALSE ("Boolean")) -> (w531:bool[])
                                n409 = Build Array(FALSE ("Boolean")) -> (w535:bool[])
                                n410 = call-poly <vilib>:"DAQmx Write.vi"("task/channels in"=refnum<k21> "BristolWM", "data"=w535) -> ("error out"=w530:errorcluster)  [unwired: 11 in, 2 out]
                                n411 = call-poly <vilib>:"DAQmx Write.vi"("task/channels in"=refnum<k21> "HSRL_WV_switch", "data"=w531, "error in"=w530) -> ()  [unwired: 10 in, 3 out]
                                n412 = Wait (ms)(milliseconds to wait=u32 3200) -> ()  [unwired: 1 out]
                                }
                                }
                                }
                                frame #3 {
                                # "If the wavelength difference is greater that 0.0002 nm, decrement the \nDBR current by 0.01 mA"
                                n413 = local read "HSRL_Diff"() -> (w540:dbl)
                                n414 = Greater Or Equal?(x=w540, y="HSRL_Tol") -> (x >= y?=w539:bool)
                                n415 = case shown="True" w539 {
                                frame False {
                                # "Wavelength difference is not greater than 0.0002 nm, do nothing"
                                }
                                frame True {
                                # "Generating a command string\nto decrement the current"
                                n416 = local read "Settings"() -> (w547:T6)
                                n417 = local read "temp step size"() -> (w541:dbl)
                                n418 = Unbundle By Name(w547) -> ("HSRL TEC"=w546:dbl)
                                n419 = Subtract(x=w546, y=w541) -> (x-y=w545:dbl)
                                n420 = local read "Device In"() -> (w543:refnum<visa-resource-name>)
                                n421 = Bundle By Name(cluster=w547, "HSRL TEC"=w545, "Module"=T15."HSRL TEC") -> (w548:T6)
                                n422 = call "TL_Driver_v2.vi"("Device In"=w543, "Commands"=T12."SET", "Settings"=w548) -> ("Readings"=w549:T7)  [unwired: 9 in, 3 out]
                                n423 = local write "Settings"(w548) -> ()
                                n424 = local write "Readings"(w549) -> ()
                                }
                                }
                                }
                                frame #4 {
                                # "If WL difference is < 0.0002 nm, increment the DBR temperature"
                                n425 = local read "HSRL_Diff"() -> (w552:dbl)
                                n426 = Less Or Equal?(x=w552, y=-0.0001) -> (x <= y?=w550:bool)
                                n427 = case shown="True" w550 {
                                frame False {
                                # "WL difference is no <= to -0.0002 nm, do nothing"
                                }
                                frame True {
                                # "Generating a command string\nto decrement the current"
                                # "WL difference is less than 0.0002 nm,\nincrement the DBR current by 0.01 mA"
                                n428 = local read "Settings"() -> (w560:T6)
                                n429 = local read "temp step size"() -> (w553:dbl)
                                n430 = Unbundle By Name(w560) -> ("HSRL TEC"=w558:dbl)
                                n431 = Add(x=w558, y=w553) -> (x+y=w557:dbl)
                                n432 = local read "Device In"() -> (w555:refnum<visa-resource-name>)
                                n433 = Bundle By Name(cluster=w560, "HSRL TEC"=w557, "Module"=T15."HSRL TEC") -> (w561:T6)
                                n434 = call "TL_Driver_v2.vi"("Device In"=w555, "Commands"=T12."SET", "Settings"=w561) -> ("Readings"=w559:T7)  [unwired: 9 in, 3 out]
                                n435 = local write "Settings"(w561) -> ()
                                n436 = local write "Readings"(w559) -> ()
                                }
                                }
                                }
                              }
                              n437 = Or(x=w503, y="Cancel HSRL") -> (x .or. y?=w504:bool)
                            }
                          }
                        }
                      }
                    }
                  }
                  frame #1 {
                    # "Reading the power meter"
                    # "Updating the pulse energy plot"
                    # "Converting to pulse energy"
                    # "Reading the offline output power, converting to pulse energy,  and updating the Pulse energy plot"
                    n438 = local read "SampleSize"() -> (w573:i32)
                    n439 = local read "Newport Device Key"() -> (w574:string)
                    n440 = local read "WV Online Pulse Energy"() -> (w579:dbl)
                    n441 = local read "WV Offline Pulse Energy"() -> (w578:dbl)
                    n442 = local read "HSRL Pulse Energy"() -> (w563:dbl)
                    n443 = local read "WV_averaged_energy"() -> (w562:dbl)
                    n444 = local read "NewportRef"() -> (w571:refnum<k24>)
                    n445 = Number To Decimal String(number=w573) -> (decimal integer string=w575:string)  [unwired: 1 in]
                    n446 = invoke class="PowerMeterCommands" method="PerformDAQ"(reference=w571, "deviceKey"=w574, "interval"="1", "sampleSize"=w575) -> ("PerformDAQ"=w576:dbl[])  [unwired: 2 in, 5 out]
                    n447 = Bundle("WV Online Pulse Energy"=w579, "WV Offline Pulse Energy"=w578, "HSRL Pulse Energy"=w563, "WV_averaged_energy"=w562) -> (w564:T18)  [unwired: 1 in]
                    n448 = local write "Pulse Energy (Micro Joule)"(w564) -> ()
                    n449 = call-poly <vilib>:"Mean.vi"("X"=w576) -> ("mean"=w572:dbl)  [unwired: 1 out]
                    n450 = Multiply(x=w572, y=1000.0) -> (x*y=w583:dbl)
                    n451 = Divide(x=w583, y=0.05) -> (x/y=w581:dbl)
                    n452 = Divide(x=w581, y=7.0) -> ()  [unwired: 1 out]
                    n453 = global read "AMCS_Data.vi" "AMCS_PowerMon"() -> (w567:u32[])
                    n454 = global read "AMCS_Data.vi" "AMCS_PowerMon"() -> (w570:u32[])
                    n455 = Index Array(array=w567, index=0) -> (element=→"HSRL Pulse Energy":u32)
                    n456 = Index Array(array=w570, index=2) -> (element=→"WV Offline Pulse Energy":u32)
                  }
                  frame #2 {
                    # "Added in the ability to interactively control the ThorLab  setting (just etalon temp for now)"
                    # "Wait 'Scalar Wait Time' for buffers to clear of online contiminated offline data"
                    n457 = disable-structure shown="Disabled" {
                      frame Disabled {
                        # "Wait 'Scalar Wait Time'"
                        n458 = local read "Scalar Wait Time"() -> (w600:u32)
                        n459 = Wait (ms)(milliseconds to wait=w600) -> ()  [unwired: 1 out]
                      }
                      frame Enabled {
                      }
                    }
                    n460 = event shown="[2] \"Settings.HSRL Etalon TEC\": Value Change" {
                      selector: _ -> [_ _ _]
                      dyn-events: _ -> [_ _ _]
                      timeout: 1 -> [_ _ _]
                      event Timeout {
                        n461 = event-data() -> ()  [unwired: 1 in, 2 out]
                      }
                      event "Settings.WV Etalon TEC": Value Change {
                        # "Generating a command string\nto update the etalon"
                        n462 = event-data() -> ()  [unwired: 1 in, 5 out]
                        n463 = local read "Settings"() -> (w590:T6)
                        n464 = Unbundle By Name(w590) -> ("WV Etalon TEC"=w592:dbl)
                        n465 = local read "Device In"() -> (w586:refnum<visa-resource-name>)
                        n466 = Bundle By Name(cluster=w590, "WV Etalon TEC"=w592, "Module"=T15."WV Etalon TEC") -> (w588:T6)
                        n467 = call "TL_Driver_v2.vi"("Device In"=w586, "Commands"=T12."SET", "Settings"=w588) -> ("Readings"=w589:T7)  [unwired: 9 in, 3 out]
                        n468 = local write "Readings"(w589) -> ()
                        n469 = local write "Settings"(w588) -> ()
                      }
                      event "Settings.HSRL Etalon TEC": Value Change {
                        # "Generating a command string\nto update the etalon"
                        n470 = event-data() -> ()  [unwired: 1 in, 5 out]
                        n471 = local read "Settings"() -> (w597:T6)
                        n472 = Unbundle By Name(w597) -> ("HSRL Etalon TEC"=w599:dbl)
                        n473 = local read "Device In"() -> (w593:refnum<visa-resource-name>)
                        n474 = Bundle By Name(cluster=w597, "HSRL Etalon TEC"=w599, "Module"=T15."HSRL Etalon TEC") -> (w595:T6)
                        n475 = call "TL_Driver_v2.vi"("Device In"=w593, "Commands"=T12."SET", "Settings"=w595) -> ("Readings"=w596:T7)  [unwired: 9 in, 3 out]
                        n476 = local write "Readings"(w596) -> ()
                        n477 = local write "Settings"(w595) -> ()
                      }
                    }
                  }
                  frame #3 {
                    w617 = 1
                    w646 = 1 ("dimension size")
                    # "Plotting the normalized relative \nbackscatter"
                    # "Calculating the normalized relative backscatter"
                    # "File path in MATLAB script is of old dial is:\nF:\\Micropulse DIAL\\Micropulse DIAL Matlab\\\nFinal Overlap Function.mat')];"
                    # "Read in latest scalar card data from \n'Scalar Data' global variable that \nscaler.vi is writing to, then wait 1 sec\nfor next batch of data"
                    # "Calculating/Plotting smoothed data,\ncross sections etc."
                    # "Pick off data with\nout header"
                    # "Calculate mean bin by bin mean"
                    # "Reading in 'Integration Period (Seconds)' of data"
                    # "Read the offline data from the scalar card, perform smoothing, calculate normalized relative backscatter, and plot"
                    # "Collects Data From Card,\nSends It To The Chart,\nAnd Saves A Copy As A\nFile If Option Selected On\nFront Panel"
                    n478 = local read "Total DIAL Integration Time (Minutes)"() -> (w662:i32)
                    n479 = local read "bins"() -> (w601:u32)
                    n480 = for {
                      N: "Data Reads (number of loops)" -> [_]
                      tunnel: [w674] -> w637 mode=indexing
                      tunnel: [w670] -> w636 mode=indexing
                      tunnel: w601 -> [w671]
                      n481 = global read "AMCS_Data.vi" "AMCS_Data"() -> (w677:u16[][])
                      n482 = disable-structure shown="Disabled" {
                        frame Disabled {
                          n483 = global read "Scalar_Data_4.vi" "Scalar Data 4"() -> ()  [unwired: 1 out]
                          n484 = global read "Scalar_Data_2.vi" "Scalar Data 2"() -> ()  [unwired: 1 out]
                        }
                        frame Enabled {
                        }
                      }
                      n485 = Index Array(array=w677, index (row) #1=1 ("index (row)"), index (row) #2=3 ("index (row)")) -> (element #1=w676:u16[], element #2=w673:u16[])  [unwired: 2 in]
                      n486 = Array Subset(array=w673, index=0, length=w671) -> (w670:u16[])
                      n487 = Array Subset(array=w676, index=0, length=w671) -> (w674:u16[])
                    }
                    n488 = Divide(x=w662, y="Data Reads (number of loops)") -> (x/y=w660:dbl)
                    n489 = local read "Total Aerosol Integration Time (Minutes)"() -> (w663:dbl)
                    n490 = Multiply(x=w660, y=60.0) -> (x*y=w650:dbl)
                    n491 = local read "background length"() -> (w641:i32)
                    n492 = local read "background start"() -> (w642:u32)
                    n493 = Transpose 2D Array(2D array=w637) -> (transposed array=w668:u16[][])
                    n494 = Transpose 2D Array(2D array=w636) -> (transposed array=w655:u16[][])
                    n495 = Divide(x=w663, y="Data Reads (number of loops)") -> (x/y=w664:dbl)
                    n496 = for {
                      N: w601 -> [_]
                      tunnel: w668 -> [w683] mode=indexing
                      tunnel: [w682] -> w669 mode=indexing
                      tunnel: w655 -> [w681] mode=indexing
                      tunnel: [w680] -> _ mode=indexing
                      tunnel: [w680] -> w652 mode=indexing
                      n497 = call-poly <vilib>:"Mean.vi"("X"=w683) -> ("mean"=w682:dbl)  [unwired: 1 out]
                      n498 = call-poly <vilib>:"Mean.vi"("X"=w681) -> ("mean"=w680:dbl)  [unwired: 1 out]
                    }
                    n499 = Multiply(x=w664, y=60.0) -> (x*y=w633:dbl)
                    n500 = Array Subset(array=w652, index=w646, length=w601) -> (w653:dbl[])
                    "CH3 Bin Readings" <- w653
                    n501 = Array Subset(array=w669, index=w646, length=w601) -> (w651:dbl[])
                    "CH1  Bin Readings" <- w651
                    n502 = Array Subset(array=w653, index=w642, length=w641) -> (w654:dbl[])
                    n503 = Array Subset(array=w651, index=w642, length=w641) -> (w667:dbl[])
                    n504 = local read "Smoothed Bins"() -> (w638:dbl)
                    n505 = call-poly <vilib>:"Mean.vi"("X"=w654) -> ("mean"=w623:dbl)  [unwired: 1 out]
                    n506 = call-poly <vilib>:"Mean.vi"("X"=w667) -> ("mean"=w628:dbl)  [unwired: 1 out]
                    n507 = local read "Index"() -> (w634:i32)
                    n508 = Subtract(x=w653, y=w623) -> (x-y=w635:dbl[])
                    n509 = Subtract(x=w651, y=w628) -> (x-y=w649:dbl[])
                    n510 = call "Ring Buffer CH1 short rev2.vi"("Index"=w634, "Profiles to Average"=w650, "Input Array"=w649) -> ("AvgArray"=w666:dbl[], "RingBufferOut"=→"CH1 RingBuffer long":dbl[][])  [unwired: 7 in]
                    n511 = call "Ring Buffer CH3 short rev2.vi"("Index"=w634, "Profiles to Average"=w633, "Input Array"=w635) -> ("AvgArray"=w644:dbl[], "RingBufferOut"=→"CH3 RingBuffer short":dbl[][])  [unwired: 7 in]
                    n512 = Reshape Array(w649, w646, w601) -> (→"CH 1 (WV off) counts display":dbl[][])
                    n513 = Reshape Array(w635, w646, w601) -> (→"CH 3 (HSRL comb) counts display":dbl[][])
                    n514 = local read "Time Resolution Per Bin(ns)"() -> (w624:u32)
                    n515 = local read "Number of Accumulates"() -> (w622:u32)
                    n516 = call "Smooth Arrray.vi"("smooth size"=w638, "Raw Array"=w666) -> ("Smoothed Array"=w602:dbl[])  [unwired: 9 in]
                    "CH1 (WV off) smooth" <- w602
                    n517 = call "Smooth Arrray.vi"("smooth size"=w638, "Raw Array"=w644) -> ("Smoothed Array"=w640:dbl[])  [unwired: 9 in]
                    "CH3 (HSRL combined) smooth" <- w640
                    n518 = local read "Temperature (C)"() -> (w659:dbl)
                    n519 = local read "Pressure (mb)"() -> (w658:dbl)
                    n520 = To Double Precision Float(number=w622) -> (double precision float=w621:dbl)
                    n521 = To Double Precision Float(number=w624) -> (double precision float=w620:dbl)
                    n522 = Reciprocal(x=w620) -> (1/x=w631:dbl)
                    n523 = script code="%accum_num=10000;     % scaler card setting number of accumulations\nt_bin = t_bin_in/1e9                 % scaler card setting time per bin\n%t_d = 37.3e-9;                % APD dead time from spec sheet\n\n% conversion from accumulated counts to count rate  (c/s)\nc_convert = 1./t_bin./accum_num;\nCR_WV = p_raw_WV.*c_convert;\nCR_HSRL = p_raw_HSRL.*c_convert;\nCR_total_WV = (p_raw_WV+b_WV).*c_convert;\nCR_total_HSRL = (p_raw_HSRL+b_HSRL).*c_convert;\nb_CR_WV =b_WV.*c_convert;\nb_CR_HSRL =b_HSRL.*c_convert;\n \n% create a range array\nsize_p =  size(p_raw_WV,2);\ngate = t_bin*3e8/2;\nr = (gate:gate:size_p*gate)./1e3; \n   \n%APD correction factor\n D_WV = 1./(1-(t_d*CR_total_WV));\n D_HSRL = 1./(1-(t_d*CR_total_HSRL));\n\n %Calculating normalize relative backscatter profile\n nrb_WV = CR_WV.*D_WV.*r.^2.*1e-6;\n nrb_HSRL = CR_HSRL.*D_HSRL.*r.^2.*1e-6;"("E"=6.0 ("Real"), "temp"=w659, "press"=w658, "p_raw_WV"=w602, "b_WV"=w628, "b_HSRL"=w623, "p_raw_HSRL"=w640, "accum_num"=w621, "t_d"="dead time", "t_bin_in"=w620) -> ("nrb_WV"=w610:cdb[], "D_WV"=w607:dbl[], "nrb_HSRL"=w609:cdb[], "D_HSRL"=w606:dbl[])  [unwired: 1 in, 1 out]
                    n524 = Divide(x=w631, y=w621) -> (x/y=w629:dbl)
                    n525 = Multiply(x=1000000000.0, y=w629) -> (x*y=w626:dbl)
                    n526 = Multiply(x=w626, y=w628) -> (x*y=w627:dbl)
                    n527 = Multiply(x=w626, y=w623) -> (x*y=w625:dbl)
                    n528 = Bundle(w627, w625) -> (→"?":cluster{dbl, dbl})  [unwired: 1 in]
                    n529 = local read "bins"() -> (w616:u32)
                    n530 = local read "Altitude Array (km)"() -> (w612:dbl[])
                    n531 = Build Array(w610, w609) -> (w614:cdb[][])
                    n532 = Build Array(w607, w606) -> (w605:dbl[][])
                    n533 = Reshape Array(w609, w617, w616) -> (→"NRB HSRL Combined":cdb[][])
                    n534 = Reshape Array(w610, w617, w616) -> (→"NRB WV Offline":cdb[][])
                    n535 = Build Array(w612, w612) -> (w611:dbl[][])
                    n536 = call "Convert to Dynamic Data7"("2D Array"=w605) -> ("Dynamic Data Type"=w604:dynamicdata)  [unwired: 3 in]
                    n537 = call "Convert to Dynamic Data3"("2D Array"=w614) -> ("Dynamic Data Type"=w613:dynamicdata)  [unwired: 3 in]
                    n538 = call "Convert to Dynamic Data4"("2D Array"=w611) -> ("Dynamic Data Type"=w608:dynamicdata)  [unwired: 3 in]
                    n539 = call "Build XY Graph2"("Y Input"=w608, "X Input"=w613) -> ("XY Graph"=→"NRB plot":cluster{"Y":dbl[], "Y":dbl[]}[])  [unwired: 3 in, 6 out]
                    n540 = call "Build XY Graph4"("Y Input"=w608, "X Input"=w604) -> ("XY Graph"=→"Correction":cluster{"Y":dbl[], "Y":dbl[]}[])  [unwired: 3 in, 6 out]
                  }
                  frame #4 {
                    # "REPLACE WITH NEW AGILTRON TASK!"
                    # "Toggle Agiltron switch to online DBR"
                    n541 = disable-structure shown="Disabled" {
                      frame Disabled {
                        # "ABSORBING"
                        n542 = flat-sequence {
                          frame #0 {
                            # "Third one"
                            # "Command the switch to switch to position 1\ncorresponding to the online DBR"
                            # "Hex string command \ncorrespond to online"
                            n543 = local read "Switch Comm Port"() -> (w687:refnum<visa-resource-name>)
                            n544 = VISA Write(VISA resource name=w687, write buffer="\u0001\u0012\u0000\u0002") -> ()  [unwired: 1 in, 3 out]
                          }
                        }
                        n545 = Build Array(FALSE ("Boolean")) -> (w686:bool[])
                        n546 = call-poly <vilib>:"DAQmx Write.vi"("task/channels in"=refnum<k21> "AgiltronSwitch", "data"=w686) -> ()  [unwired: 11 in, 3 out]
                      }
                      frame Enabled {
                      }
                    }
                  }
                  frame #5 {
                    # "If 'Save Data?' is true, save all relavant offline info"
                    n547 = local read "Save Data?"() -> (w689:bool)
                    n548 = case shown="True" w689 {
                      frame False {
                        # "'Save Data?' is false, do nothing"
                      }
                      frame True {
                        # "Write only one data file at this time"
                        # "Retrive Julian Date"
                        # "'Save Data?' is true, save offline data to the Data Disk"
                        n549 = local read "Readings"() -> (w714:T7)
                        n550 = Unbundle By Name(w714) -> ("WV Offline TEC"=w710:dbl)
                        n551 = Unbundle By Name(w714) -> ("HSRL TEC"=w715:dbl)
                        n552 = local read "HSRL Pulse Energy"() -> (w690:dbl)
                        n553 = local read "HSRL Read (nm)"() -> (w716:dbl)
                        n554 = local read "WV Offline Read (nm)"() -> (w708:dbl)
                        n555 = local read "WV Offline Pulse Energy"() -> (w709:dbl)
                        n556 = local read "Relative Humdity (%)"() -> (w737:dbl)
                        n557 = local read "CH3 Bin Readings"() -> (w706:dbl[])
                        n558 = local read "CH1  Bin Readings"() -> (w693:dbl[])
                        n559 = local read "Temperature (C)"() -> (w735:dbl)
                        n560 = local read "Pressure (mb)"() -> (w736:dbl)
                        n561 = call "Julian_Date_2.vi"() -> ("Julian Date"=w697:dbl)  [unwired: 11 in]
                        n562 = Build Array (concatenate)(w697, w708, w710, w709, w735, w736, w737, w693) -> (w721:dbl[])
                        n563 = Build Array (concatenate)(w697, w716, w715, w690, w735, w736, w737, w706) -> (w718:dbl[])
                        n564 = Array Size(array=w693) -> (size(s)=→"size(s)":i32)
                        n565 = local read "FF_Off_Ref"() -> (w723:refnum<file>)
                        n566 = local read "NF_Off_Ref"() -> (w720:refnum<file>)
                        n567 = local read "FF_Off_Ptr"() -> (w722:i64)
                        n568 = local read "NF_Off_Ptr"() -> (w719:i64)
                        n569 = local read "HSRL"() -> (w707:T10)
                        n570 = Bundle By Name(cluster=w707, "HSRLCombinedCounts"=w706, "HSRLLaserEnergy"=w690) -> (w702:T10)
                        n571 = local read "H2ODIAL"() -> (w712:T9)
                        n572 = Set File Position(offset (in bytes) (0)=w722, refnum=w723) -> (refnum out=w734:refnum<file>, error out=w732:errorcluster)  [unwired: 2 in]
                        n573 = Set File Position(offset (in bytes) (0)=w719, refnum=w720) -> (refnum out=w730:refnum<file>, error out=w728:errorcluster)  [unwired: 2 in]
                        n574 = local read "NetCDFEntry"() -> (w700:i32)
                        n575 = local read "Number of Accumulates"() -> (w696:u32)
                        n576 = local read "Time Resolution Per Bin(ns)"() -> (w695:u32)
                        n577 = Write to Binary File(file (use dialog)=w734, data=w721, error in=w732, 5:FALSE ("prepend array or string size? (T)")) -> (refnum out=w733:refnum<file>, error out=w731:errorcluster)  [unwired: 2 in, 1 out]
                        n578 = Write to Binary File(file (use dialog)=w730, data=w718, error in=w728, 5:FALSE ("prepend array or string size? (T)")) -> (refnum out=w729:refnum<file>, error out=w727:errorcluster)  [unwired: 2 in, 1 out]
                        n579 = Index Array(array=w712, index="OfflineIndex") -> (element=w711:T19)
                        n580 = Bundle By Name(cluster=w711, "DIALCounts"=w693, "DIALEnergy"=w709, "DIALTEC"=w710, "DIALWavelength"=w708) -> (w705:T19)
                        n581 = Get File Position(4:w731, 7:w733) -> (2:w724:i64)  [unwired: 2 out]
                        n582 = Get File Position(4:w727, 7:w729) -> (2:w717:i64)  [unwired: 2 out]
                        n583 = local write "FF_Off_Ptr"(w724) -> ()
                        n584 = local write "NF_Off_Ptr"(w717) -> ()
                        n585 = local write "HSRL"(w702) -> ()
                        n586 = Replace Array Subset(array=w712, new element=w705, index="OfflineIndex") -> (w703:T9)
                        n587 = local read "OfflineIndex"() -> (w699:i32)
                        n588 = local read "OnlinIndex"() -> (w698:i32)
                        n589 = local write "H2ODIAL"(w703) -> ()
                        n590 = local read "WeatherStation"() -> (w704:T11)
                        n591 = local read "NetCDFFileName"() -> (w694:string)
                        n592 = local read "NetCDFFilePath"() -> (w691:string)
                        n593 = call "UpdateNetCDFFile.vi"("FileIndex"=w700, "ShotsPerProfile"=w696, "TimePerDataBin"=w695, "TimeStamp"=w697, "OnlineIndex"=w698, "OfflineIndex"=w699, "H2ODIAL"=w703, "HSRL"=w702, "WeatherStation"=w704, "FileName"=w694, "FilePath"=w691) -> ("NewIndex"=w701:dbl)  [unwired: 15 in, 1 out]
                        n594 = local write "NetCDFEntry"(w701) -> ()
                      }
                    }
                  }
                }
              }
              frame #4 {
                n595 = First Call?() -> (First Call?: T/F=w740:bool)
                n596 = Or(x="calculate absorption cross sections", y=w740) -> (x .or. y?=w738:bool)
                n597 = case shown="True" w738 {
                  frame False {
                  }
                  frame True {
                    # "calculate absorption cross sections from HITRAN data base"
                    n598 = local read "WV Offline Set (nm)"() -> (w744:dbl)
                    n599 = local read "WV Online Read (nm)"() -> (w747:dbl)
                    n600 = local read "CH1 (WV off) smooth"() -> (w748:dbl[])
                    n601 = local read "Temperature (C)"() -> (w746:dbl)
                    n602 = local read "Pressure (mb)"() -> (w745:dbl)
                    n603 = local read "gate size"() -> (w741:dbl)
                    n604 = script code="hitran = dlmread('C:\\Users\\eol-lidar\\Desktop\\20171016_WVDIALLabviewSlimmed\\HiranData\\815nm_841nm_HITRAN_2008.csv', ',',[1 1 1676 8]);\n\n\n%hitran = dlmread('C:\\Users\\H2ODial\\Desktop\\Shared Telescope WV DIAL Code\\Libraries and VIs\\815nm_841nm_HITRAN_2008.csv', ',',[1 1 1676 8]);\n%hitran = dlmread('C:\\Users\\H2ODial\\Desktop\\Shared Telescope WV DIAL Code\\Libraries and VIs\\824nm_841nm_H2O.csv', ',',[0 1 352 7]);\n%hitran = dlmread('C:\\Users\\H2ODial\\Desktop\\Shared Telescope WV DIAL Code\\Libraries and VIs\\824nm_841nm_H2O_Spectral_Calc.csv', ',',[1 1 1209 7]);\n\n%Range vector in meters\n%range = ([75:75:size(Online,2)*75]);\ntest = size(Online,2);\nrange = ([gate_size:gate_size:test.*gate_size]); \n\nif lambda< 828\nlambda=828.195;\nelse\nlambda=lambda;\nend;\n\n%%\n\n%Voigt profile calculation\nWNmin = 1/(828+4)*1e7;  % 832.0 nm converted to wavenumber\nWNmax = 1/(828-4)*1e7;  % 824.0 nm converted to wavenumber\n\n%Find lines from WNmin to WNmax to calculate voigt profile\nline_indices = hitran(1:size(hitran,1),1)>WNmin & hitran(1:size(hitran,1),1)<WNmax;\n\nline = double(hitran(line_indices, 1:size(hitran,2)));\n\n%Calculate temperature and pressure profile\nT0 = 273+25; % surface temperature\nT0 = 273+T0_C;\nT = T0-0.0065.*range; % set to match the sounding\n\n% pressure in atmospheres\nP0  = 0.83; % surface pressure\nP0  = P0_mb/1000*0.986; %pressure in mb converted to atm\nP = P0.*(T0./T).^-5.5;   % set this value to match sounding\n\nT00 = 296;              % HITRAN reference temperature [K]\nP00 = 1;                % HITRAN reference pressure [atm]\nnu0_0 = line(:,1);      % absorption line center wavenumber from HITRAN [cm^-1]\nS0 = line(:,2);         % initial linestrength from HITRAN [cm^-1/(mol*cm^-2)]   \ngammal0 = line(:,4);    % air-broadened halfwidth at T_ref and P_ref from HITRAN [cm^-1/atm]\ngamma_s = line(:,5);    % self-broadened halfwidth at T_ref and P_ref from HITRAN [cm^-1/atm]\nE = line(:,6);          % ground state transition energy from HITRAN [cm^-1]  \nalpha = line(:,7);      % linewidth temperature dependence factor from HITRAN\ndelta = line(:,8);      % pressure shift from HiTRAN [cm^-1 atm^-1]\nnu_on = 1/(lambda)*1e7;\nnu_off = 1/(lambda_off)*1e7;\n\nfor i = 1:size(Online,2); % calculate the absorption cross section at each range\n  \n    nu0 = nu0_0+delta.*(P(i)./P00); % unclear if it should be Pi/P00  \n    gammal = gammal0.*(P(i)./P00).*((T00./T(i)).^alpha);    %Calculate Lorentz lineweidth at P(i) and T(i)\n\n    const.m = 18.015E-3./6.022E23; % mass of a single water molecule\n    const.k_B = 1.3806488e-23; % (J/K)\n    const.c = 299792458; % (m/s) (exact)\n \n    gammad = (nu0).*((2.0.*const.k_B.*T(i).*log(2.0))./(const.m.*const.c^2)).^(0.5);  %Calculate HWHM Doppler linewidth at T(i)\n     \n    % term 1 in the Voigt profile\n    y = (gammal./gammad).*((log(2.0)).^(0.5));\n    \n    % term 2 in the Voigt profile\n    x_on = ((nu_on-nu0)./gammad).*(log(2.0)).^(0.5);\n    x_off = ((nu_off-nu0)./gammad).*(log(2.0)).^(0.5);\n    \n    %setting up Voigt convolution\n    t = (-(size(line,1))/2:1:size(line,1)/2-1); %set up the integration spectral step size\n    t = repmat(t',1,length(x_on))';\n    x_on = repmat(x_on,1,length(t));\n    x_off = repmat(x_off,1,length(t));\n    y = repmat(y,1,length(t));\n    f_on = (exp(-t.^2.0))./(y.^2.0+(x_on-t).^2.0);  % combined Voigt term 1 and 2\n    f_off = (exp(-t.^2.0))./(y.^2.0+(x_off-t).^2.0);\n    %Voigt integration over all of the lines at the on and offline locations\n    z_on = trapz(t(1,:),f_on,2);\n    z_off =  trapz(t(1,:),f_off,2);\n    integral_on = z_on;\n    integral_off = z_off;\n    %Calculate linestrength at temperature T\n    S = S0.*((T00./T(i)).^(1.5)).*exp(1.439.*E.*((1./T00)-(1./T(i))));\n \n    %Calculate the Voigt profile\n    K_on = (y(:,1)./pi).*integral_on;\n    K_off = (y(:,1)./pi).*integral_off;\n    \n    %Calculate the Voigt profile absorption cross section [cm^2]\n    sigmav_on = S.*(1./gammad).*(((log(2.0))./pi).^(0.5)).*K_on; %.*far_wing_on;\n    sigmav_off = S.*(1./gammad).*(((log(2.0))./pi).^(0.5)).*K_off; %.*far_wing_off;\n    \n    %Sum contributions from all of the surrounding lines\n    sigma_on_total(i) = sum(sigmav_on);\n    sigma_off_total(i) = sum(sigmav_off);\n    \nend;"("lambda"=w747, "lambda_off"=w744, "P0_mb"=w745, "T0_C"=w746, "Online"=w748, "gate_size"=w741) -> ("sigma_on_total"=→"sigma_on_total":dbl[], "sigma_off_total"=→"sigma_off_total":dbl[])  [unwired: 1 in, 1 out]
                  }
                }
              }
              frame #5 {
                # "normalization factor\nfrom 300 to 450m"
                # "OPTICAL DEPTH PLOT"
                # "Data Processing Far Channel"
                # "Calculating the range resolved water vapor number density and plotting"
                n605 = local read "gate size"() -> (w763:dbl)
                n606 = local read "CH3 (HSRL combined) smooth"() -> (w803:dbl[])
                n607 = local read "CH2 (molecular) smoothed"() -> (w802:dbl[])
                n608 = local read "CH0 (WV on) smoothed"() -> (w782:dbl[])
                n609 = local read "CH1 (WV off) smooth"() -> (w781:dbl[])
                n610 = local read "Temperature (C)"() -> (w761:dbl)
                n611 = local read "sigma_off_total"() -> (w805:dbl[])
                n612 = local read "sigma_on_total"() -> (w804:dbl[])
                n613 = local read "Pressure (mb)"() -> (w762:dbl)
                n614 = script code="backscatter_ratio = combined./molecular;\n\n% calculate the temp and pressure profiles from surface measurement\nT0 = 273+T0_C;\n% create a range array\n range = ([0:gate_size:(size(combined,2)-1)*gate_size]); \n T = T0-0.0065.*range; \n P0  = P0_mb/1000*0.986; %pressure in mb converted to atm\n P = P0.*(T0./T).^-5.5;   \n const.k_B = 1.363806488e-23; % (J/K)\n const.k_B = 1.363806488e-23*9.89*10^-6; % (atm m^3/K)\n% backscatter coefficient in m^-1 sr^-1\nbeta_m_profile = 5.45.*10^(-32).*(550/780.2)^4.*P./(T.*const.k_B);\n\nbeta_m_array = repmat(beta_m_profile, size(backscatter_ratio,1), 1);\nbeta_bs = ((backscatter_ratio.*receiver_scale_factor)-1).*beta_m_profile"("molecular"=w802, "combined"=w803, "gate_size"=w763, "T0_C"=w761, "P0_mb"=w762, "receiver_scale_factor"="Receiver Scale Factor") -> ("beta_bs"=w749:dbl[], "beta_m_profile"=w751:dbl[])  [unwired: 1 in, 2 out]
                n615 = script code="%Time averaging in seconds.  600 Seconds =10 minutes\ntemporal_average = 600;\n%Spatial averaging in bins.  150 meters\nspatial_average = 150./gate_size;\n%Creating r and r+deltar vectors..this can also be acsomplished using the diff command\np_oni = Online(:,1:size(Online,2)-1);\np_onii = Online(:,2:size(Online,2));\np_offi = Offline(:,1:size(Offline,2)-1);\np_offii = Offline(:,2:size(Offline,2));\nInside = (p_oni.*p_offii)./(p_onii.*p_offi);\ndel_cross = 1./(2.*(sigma_on_total(1:size(Online,2)-1)-sigma_off_total(1:size(Offline,2)-1)).*gate_size*100);\ndel_cross(isinf(del_cross)) = 0;\n%Calculating Number density\nN = del_cross.*log(Inside);\n%Spatial smoothing of the profiles\nfilter1 = ones(1,4)./4;\nN_1 = N;\nN_1_avg = filter2(filter1,N_1);\nfilter1 = ones(1,10)./10;\nN_2 = N;\nN_2_avg = filter2(filter1,N_2);\nN_new = zeros(size(N,1),size(N,2));\n%Using different averaging windows for different altitudes \nN_avg=[N_1_avg(:,1:40)';N_2_avg(:,41:size(N,2))']';\nw = N_avg.*1e6.*18.015./6.022e23"("Online"=w782, "Offline"=w781, "sigma_on_total"=w804, "sigma_off_total"=w805, "gate_size"=w763) -> ("N_avg"=w765:cdb[], "w"=w766:cdb[])  [unwired: 1 in, 1 out]
                n616 = local read "Number of Bins"() -> (w771:u32)
                n617 = local read "Altitude Array (km)"() -> (w750:dbl[])
                n618 = local read "Time Resolution Per Bin(ns)"() -> (w780:u32)
                n619 = local read "Number of Bins"() -> (w759:u32)
                n620 = Logarithm Base 10(1:w749) -> (0:w756:dbl[])
                n621 = Reshape Array(w766, 1, w771) -> (→"Absolute Humdity":cdb[][])
                n622 = Build Array(w751, w749) -> (w753:dbl[][])
                n623 = Reshape Array(w756, 1, w759) -> (→"Backscatter coef":dbl[][])
                n624 = call "Convert to Dynamic Data9"("Array"=w765) -> ("Dynamic Data Type"=w769:dynamicdata)  [unwired: 3 in]
                n625 = To Double Precision Float(number=w780) -> (double precision float=w801:dbl)
                n626 = call "Convert to Dynamic Data6"("Array"=w766) -> ("Dynamic Data Type"=w767:dynamicdata)  [unwired: 3 in]
                n627 = Multiply(x=0.15, y=w801) -> (x*y=w799:dbl)
                n628 = call "Convert to Dynamic Data8"("Array"=w750) -> ("Dynamic Data Type"=w770:dynamicdata)  [unwired: 3 in]
                n629 = call "Convert to Dynamic Data5"("Array"=w750) -> ("Dynamic Data Type"=w768:dynamicdata)  [unwired: 3 in]
                n630 = call "Build XY Graph"("Y Input"=w770, "X Input"=w769) -> ("XY Graph"=→"Water Vapor Number Density":cluster{"Y":dbl[], "Y":dbl[]}[])  [unwired: 3 in, 6 out]
                n631 = call "Build XY Graph3"("Y Input"=w768, "X Input"=w767) -> ("XY Graph"=→"Absolute Humidity":cluster{"Y":dbl[], "Y":dbl[]}[])  [unwired: 3 in, 6 out]
                n632 = Divide(x=300.0, y=w799) -> (x/y=w796:dbl)
                n633 = Divide(x=450.0, y=w799) -> (x/y=w795:dbl)
                n634 = call "Convert to Dynamic Data11"("2D Array"=w753) -> ("Dynamic Data Type"=w752:dynamicdata)  [unwired: 3 in]
                n635 = call "Convert to Dynamic Data10"("Array"=w750) -> ("Dynamic Data Type"=w754:dynamicdata)  [unwired: 3 in]
                n636 = To Long Integer(number=w796) -> (32bit integer=w794:i32)
                n637 = To Long Integer(number=w795) -> (32bit integer=w793:i32)
                n638 = Decrement(x=w794) -> (x-1=w791:i32)
                n639 = Decrement(x=w793) -> (x-1=w792:i32)
                n640 = call "Build XY Graph5"("Y Input"=w754, "X Input"=w752) -> ("XY Graph"=→"aerosol profile":cluster{"Y":dbl[], "Y":dbl[]}[])  [unwired: 3 in, 6 out]
                n641 = Array Subset(array=w782, index=w791, length=w792) -> (w790:dbl[])
                n642 = Array Subset(array=w781, index=w791, length=w792) -> (w789:dbl[])
                n643 = call-poly <vilib>:"Mean.vi"("X"=w790) -> ("mean"=w788:dbl)  [unwired: 1 out]
                n644 = call-poly <vilib>:"Mean.vi"("X"=w789) -> ("mean"=w787:dbl)  [unwired: 1 out]
                n645 = Divide(x=w788, y=w787) -> (x/y=w786:dbl)
                n646 = Multiply(x=w781, y=w786) -> (x*y=w785:dbl[])
                n647 = Divide(x=w782, y=w785) -> (x/y=w784:dbl[])
                n648 = Natural Logarithm(1:w784) -> (0:w783:dbl[])
                n649 = Multiply(x=-1.0, y=w783) -> (x*y=w777:dbl[])
                n650 = call "Convert to Dynamic Data"("Array"=w777) -> ("Dynamic Data Type"=w779:dynamicdata)  [unwired: 3 in]
                n651 = call "Convert to Dynamic Data2"("Array"=w750) -> ("Dynamic Data Type"=w776:dynamicdata)  [unwired: 3 in]
                n652 = call "Build OD Plot"("Y Input"=w776, "X Input"=w779) -> ("XY Graph"=→"Optical Depth":cluster{"Y":dbl[], "Y":dbl[]}[])  [unwired: 3 in, 6 out]
              }
            }
          }
        }
        "L_Count" <- w129
      }
    }
  }
  n653 = case shown="True" w3 {
    frame False {
    }
    frame True {
      # "close data files"
      n654 = local read "NF_Off_Ref"() -> (w807:refnum<file>)
      n655 = local read "NF_On_Ref"() -> (w808:refnum<file>)
      n656 = local read "FF_Off_Ref"() -> (w809:refnum<file>)
      n657 = local read "FF_On_Ref"() -> (w810:refnum<file>)
      n658 = local read "WS_On/Off"() -> (w806:bool)
      n659 = case shown="True" w806 {
        frame False {
        }
        frame True {
          n660 = local read "WS visa"() -> (w811:refnum<visa-resource-name>)
          n661 = call "T_RH_P.vi"("VISA in"=w811, "WS_Commands"=enum16{"OpenWS", "ReadTRHP", "CloseWS"}."CloseWS") -> ()  [unwired: 11 in, 3 out]
        }
      }
      n662 = Close File(refnum=w810) -> ()  [unwired: 1 in, 2 out]
      n663 = Close File(refnum=w809) -> ()  [unwired: 1 in, 2 out]
      n664 = Close File(refnum=w808) -> ()  [unwired: 1 in, 2 out]
      n665 = Close File(refnum=w807) -> ()  [unwired: 1 in, 2 out]
    }
  }
  "FileHour" <- -1 ("FileHour")
  "DataOpen" <- FALSE
